vi "UHR-Fleezers Control (host) - 10.3.vi"() -> ()   [LabVIEW 2012]
uses:
  <vilib>/rvi/interface/nirviMethod/nirviMethod.xnode
  <vilib>/rvi/interface/nirviCloseFPGA/nirviCloseFPGA.xnode
  <vilib>/express/express analysis/Spectral/XNode/ExpressSpectralMeasurementsBlockNode.xnode
  <vilib>/rvi/interface/nirviReadWriteControl/nirviReadWriteControl.xnode
  <vilib>/Analysis/NI_AALBase.lvlib
  <vilib>/express/express analysis/Spectral/Block/exnSpectralBlock spectral measurements PSD poly.vi
  <vilib>/rvi/interface/nirviOpenFPGA/nirviOpenFPGA.xnode
  <vilib>/vision/Avi1.llb/AviRefnum.ctl
  <vilib>/Platform/TimedLoop/XDataNode/XDataNode.xnode
  <vilib>/Platform/TimedLoop/XDataNode/nitl_modes.ctl
  <vilib>/Platform/TimedLoop/XDataNode/XDNodeRunTimeDep.lvlib
  <vilib>/Platform/TimedLoop/XDataNode/wakeup.ctl
  <vilib>/Platform/TimedLoop/XDataNode/timing_clust.ctl
  <vilib>/Utility/miscctls.llb/LVPoint32TypeDef.ctl
  <vilib>/userdefined/High Color/nirio_resource_hc.ctl
  openfpgaref.8.6.ctl
  <vilib>/Utility/miscctls.llb/LVMinMaxIncTypeDef.ctl
  <vilib>/vision/NI_Vision_Development_Module.lvlib
  <vilib>/Instr/_visa.llb/VISA Configure Serial Port (Instr).vi
  <vilib>/Waveform/WDTOps.llb/WDT Append Waveforms DBL.vi
  <vilib>/express/express analysis/Spectral/Block/exnSpectralBlock spectral measurements PSD WFM.vi
  UHR-Fleezers Control (fpga) - 10.3.vi
  <vilib>/Analysis/baseanly.llb/Mean (DBL).vi
  FPGA Bitfiles/UHR-FleezersInst_FPGATarget_UHR-FleezersCont_AF27E573.lvbitx
  <vilib>/FPGAPlugInAG/PCIe-7852R/niLvFpga_Open_PCIe-7852R.vi
  <vilib>/FPGAPlugInAG/PCIe-7852R/niLvFpga_Reset_PCIe-7852R.vi
  NiFpgaLv.dll
  <vilib>/Utility/error.llb/Error Cluster From Error Code.vi
  <vilib>/rvi/errors/niLvFpgaAdjustHostInterfaceError.vi
  <vilib>/FPGAPlugInAG/PCIe-7852R/niLvFpga_ConfigureFifo_PCIe-7852R.vi
  <vilib>/rvi/errors/niLvFpgaMergeErrorWithErrorCode.vi
  <vilib>/FPGAPlugInAG/PCIe-7852R/niLvFpga_Run_PCIe-7852R.vi
  <vilib>/FPGAPlugInAG/PCIe-7852R/niLvFpga_ReadFifo_PCIe-7852R.vi
  <vilib>/FPGAPlugInAG/PCIe-7852R/niLvFpga_Close_PCIe-7852R.vi
panel:
  in  "Index":dbl=67.0 caption="Save File Index" min=1.0 step=1.0
  in  "Sample Channel Flow":bool=TRUE
  in  "Pump 3 contents":string="Left: ADig beads" caption="contents"
  in  "Pump 1 contents":string="Right: DNA beads" caption="contents"
  in  "Scripts":T1(tab)=enum."Trap Triggered Fl."
  in  "Trap Trig Fl.":bool=TRUE
  in  "Starting \nTrap Delta (MHz)":dbl=15.0
  in  "Take Force FB Data\nUpper Channel":bool
  in  "Cap 1 Samp Flow ON":bool
  in  "Cap 2 Samp Flow ON":bool=TRUE
  in  "Got DNA bead":bool
  in  "Got ADig bead":bool
  in  "Cap 2 Flow ON":bool=TRUE
  in  "Cap 1 Flow ON":bool=TRUE
  in  "Cap 2 T ON":bool=TRUE
  in  "Move Cap. 2 (ADig Left)":bool
  in  "Move Cap. 1 (DNA Right)":bool
  in  "Cal/Data Acq. Spot":bool
  in  "Dump Beads":bool
  in  "Lower Ch. Cap.":bool
  in  "Cap 1 T ON":bool=TRUE
  in  "Offset 2 Set":dbl=2.0
  in  "Offset 1 Set":dbl
  in  "Cal @ (MHz)":dbl=15.0
  in  "W/ Offset 1":bool=TRUE
  in  "Offset 1 Start (MHz)":dbl=13.0
  in  "W/ Offset 2":bool
  in  "Offset 2 Start (MHz)":dbl=16.0
  in  "Move to Delta 2 (MHz)":dbl=13.0
  in  "Attempt Limit":dbl=15.0 caption="Limit"
  out "Attempts":dbl=10.0
  in  "Wait Before Save (s)":u32=1
  in  "Fish for Tether":bool
  in  "Closest Delta (MHz)":dbl=9.25 step=0.25
  in  "Stop F (pN)":dbl=3.0
  in  "Then...":string(combo)="5"
  in  "Move to Delta 1 (MHz)":dbl=13.0
  in  "Tether Alarm?":bool=TRUE
  out "Tether":bool
  in  "TA Cancel Save?":bool
  in  "TA Green Off?":bool
  in  "Raster Set Upon Tether":u32=1
  in  "Save at end (5, 6)":bool
  out "Waiting":bool
  in  "Trap Triggering":bool
  in  "Wait to get offset (s)":u32=5
  in  "mean sampling rate (ms)":u32=100
  in  "Threshold (nm)":dbl=10.0
  in  "Fl. ON time (s)":i32=10
  out "T1 x pos data":dbl[](array[numeric])
  out "max value":dbl
  out "min value":dbl
  out "Mean T1 Position (nm) 2":dbl caption="Mean T1 for Comparison (nm)" format="%0.2f"
  in  "Dip Trap Delta 1 (MHz)":dbl=15.0
  in  "Move Trap Before?":bool
  in  "Save Data After?":bool
  in  "Green ON After?":bool
  in  "Dip Trap Delta 2 (MHz)":dbl=15.0
  in  "Move Trap After?":bool
  in  "Duration (s)":dbl=1.0
  in  "Dip for Protein":bool
  in  "Y change (mm)":dbl=3.0
  in  "Profile":bool
  out "Current Position":cluster{dbl, dbl, dbl}
  in  "APD to Watch":bool
  out "Duration (s)":dbl
  in  "Action":string(combo)="Yank"
  in  "Fl. Triggered...":bool
  in  "Fl. Delta Thresh. (kHz)":dbl=0.6
  out "Waiting":bool
  out "Fl. High":bool
  in  "N pts to average":u16=6
  in  "Yank Delay (s)":dbl=3.5
  in  "Yank to Delta Array (MHz)":dbl[](array[numeric])=[16.3, 15.85, 14.85]
  in  "N Array El":u8=3 min=1 step=1
  in  "Random Choice":bool=TRUE
  in  "Force Yank":bool
  in  "Force Reset":bool
  in  "N Steps":dbl=20.0
  in  "Step Size (nm)":dbl=0.34
  in  "Save ave factor":dbl=1.0
  in  "Take Stepping Data":bool
  out "Sigma/Mean 2":dbl=0.9156115002105881 caption="Sigma/Mean" format="%#_2g"
  out "Rate sigma (Hz) 2":dbl=91.25594618765528 caption="Sigma (Hz)" format="%0.2f"
  out "APD 2 Rate (Hz)":dbl=99.66666666666667 format="%#_3p"
  out "Primary Video Display":T2(plugin-control)
  out "Waveform Graph":dbl[](graph) caption="APD Line Scan"
  in  "Inject Pump 3":bool
  in  "Inject Pump 1":bool
  out "Messages":string="4:51 PM\tLost tether (7 s).\r4:51 PM\tFormed tether in 10 attempt(s).\r4:50 PM\tLost tether (5 s).\r4:49 PM\tFormed tether in 5 attempt(s).\r4:47 PM\tLost tether (36 s).\r4:47 PM\tFormed tether in 1 attempt(s).\r4:42 PM\tTether fishing timeout.\r4:37 PM\tTether fishing timeout.\r4:36 PM\tTether fishing timeout.\r4:32 PM\tTether fishing timeout.\r4:29 PM\tLost tether (4 s).\r4:28 PM\tFormed tether in 6 attempt(s).\r4:28 PM\tLost tether (5 s).\r4:28 PM\tFormed tether in 6 attempt(s).\r4:23 PM\tFormed tether in 1 attempt(s).\r4:23 PM\tLost tether (6 s).\r4:23 PM\tFormed tether in 1 attempt(s).\r4:14 PM\tFormed tether in 2 attempt(s).\r4:10 PM\tLost tether (548 s).\r4:01 PM\tFormed tether in 2 attempt(s).\r3:58 PM\tLost tether (6 s).\r3:58 PM\tFormed tether in 3 attempt(s).\r3:57 PM\tTether fishing timeout.\r3:42 PM\tLost tether (6 s).\r3:42 PM\tFormed tether in 6 attempt(s).\r3:39 PM\tLost tether (50 s).\r3:38 PM\tFormed tether in 10 attempt(s).\r3:37 PM\tLost tether (5 s).\r3:37 PM\tFormed tether in 6 attempt(s).\r3:34 PM\tTether fishing timeout.\r3:31 PM\tLost tether (45 s).\r3:30 PM\tFormed tether in 1 attempt(s).\r3:30 PM\tLost tether (4 s).\r3:30 PM\tFormed tether in 4 attempt(s).\r3:22 PM\tFormed tether in 6 attempt(s).\r3:18 PM\tLost tether (51 s).\r3:17 PM\tFormed tether in 3 attempt(s).\r3:17 PM\tLost tether (6 s).\r3:16 PM\tFormed tether in 1 attempt(s).\r3:06 PM\tFormed tether in 2 attempt(s).\r3:05 PM\tLost tether (3 s).\r3:05 PM\tFormed tether in 1 attempt(s).\r2:11 PM\tUHR-Fleezers ready.\r"
  in  "APD Ave N":dbl=10.0
  out "Int. Time (s)":dbl=3.0
  in  "Stop All":bool=TRUE
  out "Sigma/Mean":dbl=0.7461899027919234 format="%#_2g"
  out "Rate sigma (Hz)":dbl=246.24266792133471 caption="Sigma (Hz)" format="%0.2f"
  in  "Tab Control 6":T3(tab)
  in  "APD 2 Offset":dbl
  in  "APD 1 Offset":dbl
  out "RMS (Ang)":dbl=824.5898142565536 format="%_2g"
  in  "Bead Sep. Int. Time (s)":dbl=5.0 caption="Int. Time (s)"
  in  "Below (kHz)":dbl=0.5
  in  "Above (kHz)":dbl=2.0
  in  "Adjust Scale\nto Mean":bool
  in  "Rescale on Mean":bool
  in  "Offset (nm)":dbl
  out "Mean":dbl=107.85631162700733 caption="Mean (pN)" format="%#_3g"
  out "Force":waveform(dbl)[](graph)=[{"t0"=timestamp(9589.800000000116 s since 1904-01-01), "dt"=0.15, "Y"=[-107.59208218650274, -108.24679101361127], "attributes"=variant("NI_ChannelName"=variant(string "T1 X"))}, {"t0"=timestamp(9589.800000000116 s since 1904-01-01), "dt"=0.15, "Y"=[107.4628305657673, 108.12354274214799], "attributes"=variant("NI_ChannelName"=variant(string "T2 X"))}]
  out "APD Chart":waveform(dbl)[](graph)=[{"t0"=timestamp(9589.800000000116 s since 1904-01-01), "dt"=0.15, "Y"=[253.33333333333334, 266.6666666666667], "attributes"=variant("NI_ChannelName"=variant(string "APD 1"))}, {"t0"=timestamp(9589.800000000116 s since 1904-01-01), "dt"=0.15, "Y"=[93.33333333333334, 106.66666666666667], "attributes"=variant("NI_ChannelName"=variant(string "APD 2"))}]
  in  "Calibration":u16(ring)=2 items=["None", "Position", "Force"]
  out "T1 X":dbl=-107.919436600057 caption="T1 X (pN)" format="%0.2f"
  out "T2 X":dbl=-107.79318665395765 caption="T2 X (pN)" format="%0.2f"
  out "Bead Separation":waveform(dbl)(graph)={"t0"=timestamp(9589.800000000116 s since 1904-01-01), "dt"=0.15, "Y"=[-66.14062626515556, -66.57399525696837], "attributes"=variant("NI_ChannelName"=variant(string "T1 X"))}
  in  "Amplitude (nm)":dbl=3.0
  out "Bead Mean (nm)":dbl=-64.52066524805926 caption="Mean (nm)" format="%0.2f"
  out "Difference":dbl=0.12624994609934959 caption="Difference (pN)" format="%.2g"
  in  "Take Detection Laser\nImage":bool
  out "APD 2":T2(plugin-control) caption="APD 2 (Cy5)"
  in  "Flip Green Filter":bool
  in  "Set X Only":bool
  in  "Set Y Only":bool
  out "APD 1":T2(plugin-control) caption="APD 1 (Cy3)"
  out "Detection Laser Y":T2(plugin-control)
  out "Pointer Y (V)":dbl=4.98101801028038 format="%_3g"
  out "Pointer X (V)":dbl=3.881593676564837 format="%_3g"
  in  "Set Confocal Spot (X-Y)":bool
  out "Detection Laser X":T2(plugin-control)
  out "Saved APD":dbl[][](graph)=[[640.0, 640.0, 513.3333333333334, 520.0, 506.6666666666667, 520.0, 626.6666666666667, 680.0, 540.0, 606.6666666666667, 640.0, 513.3333333333334, 553.3333333333334, 693.3333333333334, 613.3333333333334, 513.3333333333334, 660.0, 513.3333333333334, 620.0, 506.6666666666667, 613.3333333333334, 546.6666666666667, 566.6666666666667, 753.3333333333334, 540.0, 546.6666666666667, 593.3333333333334, 646.6666666666667, 533.3333333333334, 613.3333333333334, 633.3333333333334, 653.3333333333334, 580.0, 646.6666666666667, 686.6666666666667, 660.0, 646.6666666666667, 560.0, 520.0, 600.0, 573.3333333333334, 633.3333333333334, 620.0, 600.0, 553.3333333333334, 533.3333333333334, 540.0, 546.6666666666667, 586.6666666666667, 573.3333333333334, 626.6666666666667, 506.6666666666667, 606.6666666666667, 613.3333333333334, 600.0, 526.6666666666667, 606.6666666666667, 606.6666666666667, 560.0, 613.3333333333334, 546.6666666666667, 486.6666666666667, 606.6666666666667, 573.3333333333334, 660.0, 693.3333333333334, 620.0, 586.6666666666667, 553.3333333333334, 506.6666666666667, 486.6666666666667, 593.3333333333334, 520.0, 560.0, 653.3333333333334, 633.3333333333334, 546.6666666666667, 653.3333333333334, 586.6666666666667, 566.6666666666667, 620.0, 546.6666666666667, 593.3333333333334, 580.0, 673.3333333333334, 673.3333333333334, 566.6666666666667, 620.0, 506.6666666666667, 633.3333333333334, 613.3333333333334, 546.6666666666667, 606.6666666666667, 600.0, 680.0, 586.6666666666667, 573.3333333333334, 540.0, 573.3333333333334, 633.3333333333334, 546.6666666666667, 553.3333333333334, 533.3333333333334, 633.3333333333334, 633.3333333333334, 600.0, 646.6666666666667, 640.0, 540.0, 486.6666666666667, 586.6666666666667, 566.6666666666667, 626.6666666666667, 606.6666666666667, 640.0, 546.6666666666667, 566.6666666666667, 653.3333333333334, 626.6666666666667, 586.6666666666667, 613.3333333333334, 626.6666666666667, 560.0, 700.0, 546.6666666666667, 506.6666666666667, 566.6666666666667, 640.0, 573.3333333333334, 593.3333333333334, 493.33333333333337, 613.3333333333334, 626.6666666666667, 673.3333333333334, 580.0, 633.3333333333334, 633.3333333333334, 713.3333333333334, 400.0, 560.0, 520.0, 506.6666666666667, 720.0, 553.3333333333334, 553.3333333333334, 426.6666666666667, 600.0, 540.0, 520.0, 640.0, 453.33333333333337, 533.3333333333334, 460.0, 426.6666666666667, 546.6666666666667, 580.0, 460.0, 480.0, 586.6666666666667, 473.33333333333337, 580.0, 613.3333333333334, 546.6666666666667, 500.0, 546.6666666666667, 540.0, 586.6666666666667, 560.0, 406.6666666666667, 533.3333333333334, 520.0, 573.3333333333334, 540.0, 486.6666666666667, 633.3333333333334, 486.6666666666667, 586.6666666666667, 440.0, 446.6666666666667, 553.3333333333334, 520.0, 540.0, 620.0, 506.6666666666667, 580.0, 653.3333333333334, 540.0, 566.6666666666667, 586.6666666666667, 453.33333333333337, 653.3333333333334, 553.3333333333334, 460.0, 593.3333333333334, 420.0, 553.3333333333334, 526.6666666666667, 480.0, 520.0, 606.6666666666667, 493.33333333333337, 560.0, 513.3333333333334, 426.6666666666667, 440.0, 513.3333333333334, 500.0, 633.3333333333334, 513.3333333333334, 460.0, 526.6666666666667, 466.6666666666667, 540.0, 546.6666666666667, 540.0, 486.6666666666667, 500.0, 506.6666666666667, 553.3333333333334, 400.0, 493.33333333333337, 420.0, 413.33333333333337, 540.0, 513.3333333333334, 493.33333333333337, 420.0, 533.3333333333334, 466.6666666666667, 546.6666666666667, 493.33333333333337, 480.0, 366.6666666666667, 526.6666666666667, 520.0, 406.6666666666667, 526.6666666666667, 620.0, 520.0, 500.0, 460.0, 480.0, 520.0, 446.6666666666667, 680.0, 526.6666666666667, 613.3333333333334, 700.0, 566.6666666666667, 646.6666666666667, 573.3333333333334, 593.3333333333334, 626.6666666666667, 546.6666666666667, 526.6666666666667, 773.3333333333334, 626.6666666666667, 546.6666666666667, 633.3333333333334, 553.3333333333334, 613.3333333333334, 546.6666666666667, 540.0, 593.3333333333334, 620.0, 646.6666666666667, 706.6666666666667, 506.6666666666667, 573.3333333333334, 640.0, 513.3333333333334, 473.33333333333337, 606.6666666666667, 533.3333333333334, 466.6666666666667, 506.6666666666667, 500.0, 573.3333333333334, 446.6666666666667, 646.6666666666667, 533.3333333333334, 533.3333333333334, 560.0, 500.0, 586.6666666666667, 580.0, 460.0, 486.6666666666667, 580.0, 573.3333333333334, 506.6666666666667, 533.3333333333334, 586.6666666666667, 700.0, 486.6666666666667, 480.0, 560.0, 593.3333333333334, 573.3333333333334, 680.0, 626.6666666666667, 633.3333333333334, 660.0, 640.0, 600.0, 600.0, 586.6666666666667, 760.0, 686.6666666666667, 613.3333333333334, 686.6666666666667, 593.3333333333334, 553.3333333333334, 606.6666666666667, 573.3333333333334, 460.0, 546.6666666666667, 640.0, 553.3333333333334, 600.0, 580.0, 526.6666666666667, 620.0, 573.3333333333334, 626.6666666666667, 506.6666666666667, 573.3333333333334, 413.33333333333337, 373.33333333333337, 493.33333333333337, 546.6666666666667, 513.3333333333334, 466.6666666666667, 626.6666666666667, 526.6666666666667, 486.6666666666667, 480.0, 500.0, 593.3333333333334, 453.33333333333337, 500.0, 460.0, 593.3333333333334, 540.0, 500.0, 486.6666666666667, 500.0, 533.3333333333334, 460.0, 540.0, 500.0, 580.0, 480.0, 586.6666666666667, 560.0, 513.3333333333334, 566.6666666666667, 553.3333333333334, 540.0, 593.3333333333334, 533.3333333333334, 493.33333333333337, 553.3333333333334, 466.6666666666667, 500.0, 646.6666666666667, 513.3333333333334, 540.0, 446.6666666666667, 540.0, 426.6666666666667, 540.0, 613.3333333333334, 506.6666666666667, 493.33333333333337, 486.6666666666667, 606.6666666666667, 500.0, 486.6666666666667, 526.6666666666667, 560.0, 540.0, 433.33333333333337, 540.0, 520.0, 480.0, 540.0, 473.33333333333337, 466.6666666666667, 420.0, 413.33333333333337, 560.0, 546.6666666666667, 493.33333333333337, 406.6666666666667, 480.0, 480.0, 466.6666666666667, 426.6666666666667, 486.6666666666667, 520.0, 606.6666666666667, 480.0, 493.33333333333337, 626.6666666666667, 486.6666666666667, 486.6666666666667, 440.0, 660.0, 593.3333333333334, 533.3333333333334, 520.0, 580.0, 500.0, 573.3333333333334, 500.0, 573.3333333333334, 446.6666666666667, 586.6666666666667, 586.6666666666667, 546.6666666666667, 600.0, 620.0, 540.0], [73.33333333333334, 166.66666666666669, 86.66666666666667, 113.33333333333334, 140.0, 126.66666666666667, 93.33333333333334, 93.33333333333334, 113.33333333333334, 120.0, 120.0, 146.66666666666669, 66.66666666666667, 113.33333333333334, 120.0, 113.33333333333334, 120.0, 126.66666666666667, 140.0, 133.33333333333334, 120.0, 140.0, 86.66666666666667, 160.0, 126.66666666666667, 113.33333333333334, 93.33333333333334, 133.33333333333334, 100.0, 126.66666666666667, 133.33333333333334, 86.66666666666667, 126.66666666666667, 80.0, 140.0, 113.33333333333334, 120.0, 186.66666666666669, 113.33333333333334, 93.33333333333334, 53.333333333333336, 66.66666666666667, 133.33333333333334, 140.0, 126.66666666666667, 53.333333333333336, 126.66666666666667, 133.33333333333334, 73.33333333333334, 113.33333333333334, 100.0, 66.66666666666667, 113.33333333333334, 120.0, 140.0, 100.0, 80.0, 126.66666666666667, 126.66666666666667, 133.33333333333334, 73.33333333333334, 113.33333333333334, 93.33333333333334, 126.66666666666667, 140.0, 46.66666666666667, 153.33333333333334, 113.33333333333334, 66.66666666666667, 106.66666666666667, 146.66666666666669, 100.0, 120.0, 93.33333333333334, 140.0, 126.66666666666667, 93.33333333333334, 60.0, 46.66666666666667, 133.33333333333334, 93.33333333333334, 113.33333333333334, 80.0, 73.33333333333334, 113.33333333333334, 93.33333333333334, 113.33333333333334, 146.66666666666669, 120.0, 66.66666666666667, 120.0, 106.66666666666667, 80.0, 113.33333333333334, 113.33333333333334, 100.0, 73.33333333333334, 106.66666666666667, 126.66666666666667, 80.0, 140.0, 93.33333333333334, 120.0, 113.33333333333334, 80.0, 53.333333333333336, 113.33333333333334, 80.0, 93.33333333333334, 140.0, 146.66666666666669, 93.33333333333334, 180.0, 133.33333333333334, 60.0, 140.0, 100.0, 153.33333333333334, 100.0, 86.66666666666667, 93.33333333333334, 106.66666666666667, 126.66666666666667, 60.0, 113.33333333333334, 153.33333333333334, 120.0, 140.0, 106.66666666666667, 86.66666666666667, 146.66666666666669, 113.33333333333334, 133.33333333333334, 126.66666666666667, 100.0, 126.66666666666667, 186.66666666666669, 86.66666666666667, 146.66666666666669, 73.33333333333334, 160.0, 113.33333333333334, 113.33333333333334, 80.0, 106.66666666666667, 126.66666666666667, 113.33333333333334, 93.33333333333334, 126.66666666666667, 126.66666666666667, 113.33333333333334, 93.33333333333334, 60.0, 146.66666666666669, 100.0, 106.66666666666667, 66.66666666666667, 80.0, 106.66666666666667, 93.33333333333334, 73.33333333333334, 113.33333333333334, 100.0, 86.66666666666667, 133.33333333333334, 100.0, 86.66666666666667, 100.0, 53.333333333333336, 180.0, 120.0, 133.33333333333334, 106.66666666666667, 80.0, 133.33333333333334, 86.66666666666667, 73.33333333333334, 100.0, 100.0, 126.66666666666667, 93.33333333333334, 73.33333333333334, 66.66666666666667, 113.33333333333334, 73.33333333333334, 140.0, 120.0, 133.33333333333334, 100.0, 86.66666666666667, 53.333333333333336, 100.0, 80.0, 100.0, 86.66666666666667, 106.66666666666667, 120.0, 73.33333333333334, 120.0, 60.0, 100.0, 113.33333333333334, 93.33333333333334, 126.66666666666667, 80.0, 73.33333333333334, 73.33333333333334, 100.0, 86.66666666666667, 66.66666666666667, 133.33333333333334, 93.33333333333334, 73.33333333333334, 126.66666666666667, 73.33333333333334, 106.66666666666667, 86.66666666666667, 120.0, 133.33333333333334, 80.0, 146.66666666666669, 80.0, 120.0, 86.66666666666667, 80.0, 60.0, 100.0, 93.33333333333334, 73.33333333333334, 106.66666666666667, 126.66666666666667, 80.0, 133.33333333333334, 86.66666666666667, 106.66666666666667, 120.0, 60.0, 40.0, 66.66666666666667, 86.66666666666667, 93.33333333333334, 66.66666666666667, 86.66666666666667, 100.0, 86.66666666666667, 120.0, 146.66666666666669, 80.0, 80.0, 160.0, 133.33333333333334, 93.33333333333334, 80.0, 140.0, 40.0, 113.33333333333334, 113.33333333333334, 93.33333333333334, 100.0, 106.66666666666667, 93.33333333333334, 133.33333333333334, 120.0, 120.0, 86.66666666666667, 66.66666666666667, 113.33333333333334, 66.66666666666667, 106.66666666666667, 100.0, 146.66666666666669, 120.0, 126.66666666666667, 106.66666666666667, 80.0, 133.33333333333334, 166.66666666666669, 86.66666666666667, 100.0, 133.33333333333334, 120.0, 86.66666666666667, 113.33333333333334, 40.0, 100.0, 106.66666666666667, 93.33333333333334, 86.66666666666667, 126.66666666666667, 53.333333333333336, 106.66666666666667, 106.66666666666667, 93.33333333333334, 80.0, 80.0, 120.0, 86.66666666666667, 146.66666666666669, 53.333333333333336, 86.66666666666667, 160.0, 153.33333333333334, 93.33333333333334, 93.33333333333334, 86.66666666666667, 120.0, 113.33333333333334, 93.33333333333334, 73.33333333333334, 60.0, 153.33333333333334, 60.0, 100.0, 80.0, 113.33333333333334, 106.66666666666667, 86.66666666666667, 113.33333333333334, 100.0, 86.66666666666667, 73.33333333333334, 100.0, 73.33333333333334, 80.0, 106.66666666666667, 93.33333333333334, 106.66666666666667, 106.66666666666667, 86.66666666666667, 60.0, 73.33333333333334, 93.33333333333334, 120.0, 140.0, 160.0, 60.0, 120.0, 120.0, 73.33333333333334, 73.33333333333334, 146.66666666666669, 80.0, 66.66666666666667, 100.0, 73.33333333333334, 113.33333333333334, 100.0, 66.66666666666667, 66.66666666666667, 93.33333333333334, 73.33333333333334, 146.66666666666669, 120.0, 86.66666666666667, 60.0, 86.66666666666667, 113.33333333333334, 120.0, 120.0, 73.33333333333334, 153.33333333333334, 106.66666666666667, 100.0, 80.0, 86.66666666666667, 113.33333333333334, 73.33333333333334, 113.33333333333334, 140.0, 93.33333333333334, 93.33333333333334, 60.0, 126.66666666666667, 93.33333333333334, 106.66666666666667, 113.33333333333334, 46.66666666666667, 113.33333333333334, 86.66666666666667, 100.0, 126.66666666666667, 93.33333333333334, 66.66666666666667, 160.0, 146.66666666666669, 93.33333333333334, 93.33333333333334, 93.33333333333334, 73.33333333333334, 106.66666666666667, 86.66666666666667, 66.66666666666667, 80.0, 86.66666666666667, 100.0, 120.0, 80.0, 120.0, 120.0, 133.33333333333334, 86.66666666666667, 113.33333333333334, 160.0, 93.33333333333334, 86.66666666666667, 93.33333333333334, 80.0, 120.0, 73.33333333333334, 93.33333333333334, 73.33333333333334, 73.33333333333334, 66.66666666666667, 120.0, 93.33333333333334, 60.0, 100.0, 100.0, 73.33333333333334, 73.33333333333334, 106.66666666666667, 86.66666666666667, 66.66666666666667, 126.66666666666667]] caption="Most Recent Time Trace"
  out "Trap Delta Graph":dbl[](graph)=[-106.43043807216529, -106.5454367986324, -106.51686160160939, -106.58501313534859, -106.73405579848394, -106.59345831600089, -106.55808478718131, -106.54847798904014, -106.63246708958809, -106.64841693959238, -106.4822053501463, -106.57755688373177, -106.67016724634344, -106.45433878652537, -106.47815911583766, -106.42379428925383, -106.51151845331754, -106.68746141834603, -106.50723577160747, -106.41173347001666, -106.45298074469062, -106.68357946354386, -106.41957394891901, -106.42779113376133, -106.46017439309665, -106.3331576187891, -106.35502678934324, -106.32337366489861, -106.55680288846125, -106.29647485921345, -106.4777976983645, -106.297812998571, -106.39808607771205, -106.65261139520646, -106.51296579380772, -106.66918631936434, -106.17562143548844, -84.60994919536043, 1.3310857319345684, 1.0361871672274952, 0.6560712621147459, 0.5689432704114208, 0.5054763131013246, 0.026676923553220266, 0.4416019568801436, 0.2735431213660061, 0.23024753352250904, 0.37724536348759063, 0.2421264893459717, 0.26340021780432943, 0.29841957537993546, 0.17548186500256102, 0.14535336814513755, 0.07167026524356301, 0.22596132502466781, 0.2852071568323358, 0.3257436622559723, 0.12892633791448793, 0.17014124062038827, 0.13608261272222044, 0.2165257310266071, 0.02390519326463647, 0.24374284074938912, 0.14033144222620686, 0.20160694442302618, 0.24399108515159418, 0.37280924880476496, 0.39269031828135303, 0.0020045770407064456, 0.24243253128233844, 0.5509136378777598, -0.06739948998052048, 0.3753325270901159, 0.041556923442069515, 0.5156644188755136, 0.43429902173750445, 0.6734298753615677, 0.24078809415362, 0.2226386778369127, 0.0928074556229388, 0.23452704613553288, 0.29537252172755735, 0.24028041004987544, 0.5110751644361885, 0.3115531148109213, 0.3541005104538466, 0.19808764601755413, 0.29451725645941296, 0.37483027387224876, 0.14422108697133207, 0.10937006932469684, -0.10006183935749324, 0.5174008122551468, -0.15899440920889152, 0.067222901985028, 0.4893964012215861, 0.16100705380999392, 0.040244638366899954, 0.21823030270568278, 0.2724552172281144, 0.3286154371444875, 0.09671105698981519, 0.211070673931971, 0.27403940383827663, -0.18158626168544867, 0.359992544087572, 0.17521597973752523, -0.01712139810390334, 0.34828383230753013, 0.38821465356197205, -0.47577316993658636, -0.061209978340928006, -0.04336067966990298, 0.1973437946223825, 0.14125329725782476, 0.39799396471853143, 0.5095924157430234, 0.5369250733859182, 0.5141657617439718, 0.12314529776262206, 0.12340359436175818, 0.4247246292008219, 0.34987918195615864, 0.3691260807314214, 0.18948963934016738, 0.11514675643557093, 0.3145960367967432, 0.0847238153799148, 0.5498257841297541, 0.3435810561376562, 0.28951709031660544, 0.11486034175086168, 0.19981958245548992, 0.24902605730103988, 0.08386197607169354, 0.3076486879407194, 0.5316368497813708, 0.011172428028344061, 0.16515294490283083, 0.2589832302335102, 0.06118106222967257, 0.05179602677324213, 0.14605031191417106, -0.27028691855927245, 0.3046427258477053, -0.32654161566760187, 0.11547372002670883, 0.05841771855848377, -0.09021888308668857, 0.28492200832706416, 0.14848195262761732, 0.08004379230789829, 0.11340489372509398, -0.1207310131639201, 0.1541946406564236, 0.1269929332462834, -0.25254475570349794, 0.1559630190503728, -0.16465543631295051, 0.11133039420408519, 0.1402543807831096, 0.02125799385333696, -0.16462459978957333, -0.38923305887864584, -0.02381113492727646, 0.10391530706475595, 0.23820889685935479, -0.023728686724600878, -0.04764111901766144, -0.007608743009235641, -0.2831431266449582, -0.4601669034291135, 0.1270783916843988, 0.11151315228001513, 0.07486139973609482, -0.24727183052659096, 0.19791921503036844, 0.07911640381694093, -0.06594038816975148, 0.2904115238995478, 0.2572744514721885, -0.20695214319298796, -0.011134088990943897, -0.1329170956283653, -0.17359323758311615, 0.12181978652209512, -0.11042971273973787, 0.22899157117508717, 0.3140832953715535, -0.30689327909618325, 0.03860844834068772, 0.394228107655571, 0.05293892569083136, -0.25365611830805873, 0.24686577579815186, 0.049501080171641065, -0.14974810230810087, -0.02833685388093199, 0.18652778365699527, 0.29108264069094064, -0.0008448102460272833, 0.0018380106327957058, 0.12078335855310426, 0.25940308098841486, -0.04482483301124446, 0.07376288462566721, -0.20968097306502337, -0.21601485851555285, -0.255227346307366, -0.006578989879893332, 0.2693875220630272, -0.05322628288934911, 0.013224520397867853, 0.019089251473903474, 0.1785683517670636, 0.0005106496658305038, 0.03471794306860293, -0.03881457062500418, 0.1314922052228636, 0.19291503243930383, 0.016286528257771483, 0.04613488933487331, 0.023391462208254027, -0.0867936685376553, 0.1667056535330356, 0.13551569687601753, 0.03966388491544098, -0.001509757708971271, -0.04930535048489537, -0.02488348604948106, 0.17699798141823225, 0.09067749598174343, 0.2810609960550859, -0.17953434343886976, -0.08087810161787876, 0.15531385466958078, 0.07966370440497603, 0.21169243968790535, 0.27463644895840034, 0.11358419137524867, 0.44151340468279066, 0.013676594736444725, 0.13803367875581318, 0.16762306170228025, -9.305097846396249, -8.734185730622158, -7.795085141730819, -7.1169239424821455, -6.8078194604182505, -6.012872438821646, -5.297070121155155, -4.8008820282039935, -3.80266145736694, -3.2398214424229104, -2.6995113604562464, -2.250937951595689, -1.6142815413389022, -1.1477956359922619, -0.7851258896920497, -0.5489468717661414, 0.007892963192939528, 0.4297874535410666, 0.7232126615705075, 1.0881378793787722, 0.9469945823546175, 1.1315981032380298, 1.5088200228939004, 1.9696025136662745, 2.0125320503247393, 2.0616893854058578, 2.0607414539584012, 2.6901101639116844, 2.913370534266508, 2.9915343321096253, 3.1810584698757345, 3.2694738112071233, 3.815351721905264, 3.711465789182815, 3.3319100390246166, 3.4738940838355026, 2.9938700615022165, 2.8719830063163836, 2.814001855577777, 2.4799945954145404, 2.306309702543458, 2.287683746001849, 1.884452351748454, 1.4763570637661683, 1.500909948307402, 1.3757091991201318, 0.9511484877404002, 0.7750514269276616, 0.6476631465563494, -0.070662296735875, -0.029594788212394696, -0.32400306754623637, -0.8864635561709634, -1.4877222685335405, -2.0507065584317017, -2.6968184066815972, -3.0471461188113667, -3.5358182192812335, -4.376697785171516, -4.953120166587164, -5.848565647315136, -6.053854911411889, -7.052139284154087, -7.172726882840011, -8.190341884763662, -8.57176218146154, -9.031969641304759, -9.160140089904607, -19.406396896392515, -20.72767491143481, -22.52957503831575, -24.628780001646625, -27.645919716135815, -31.524820294981247, -36.00375847806328, -40.29138452034995, -45.564980244900866, -52.03629009220346, -59.389338493635734, -67.53729872875331, -76.40368321454261, -86.00318733592643, -95.67183386111026, -98.591914485014, -103.5540396015088, -111.71602156262952, -119.7345182693686, -128.10083921857876, -133.92328842606133, -140.30486296175064, -152.13782681810846, -127.59977417259103, 1.9097381969808318, 2.146077316363836, 2.5695963953157115, 2.6372377874037967, 2.712002965976897, 2.21214115543342, 2.0827027656517636, 1.7918328994151387, 1.8334538504789635, 1.4887474407240884, 1.3183156469574928, 1.1074607806068812, 0.5449613088181862, 0.6411310292885716, 0.2865682674798876, -0.20561912550425498, -0.4283737772873612, -0.8213909015749081, -1.301367318197441, -1.4043123386109424, -2.455428847708026, -2.865387975996997, -3.4460393734956574, -4.088620933822033, -4.852423708406629, -5.363424054600309, -5.985200931385475, -6.449778687075328, -7.359018465262011, -8.014348652381976, -8.602206142039282, -9.11747831938223, -16.10276890966618, -16.652936161554457, -17.45363480985382, -18.573158822709363, -19.611725824538883, -21.567924207070938, -24.090533940752877, -27.20500645507802, -31.47067005386945, -36.72043318743074, -43.01369354998713, -50.30269462184975, -58.470394481182154, -66.68608952303441, -76.32223565208024, -85.90747526669313, -96.45584392830432, -107.64327334791787, -118.00360649269274, -128.23147312175695, -139.24390140541698, -150.1280581951645, -160.43369113902202, -169.03532569855338, -179.6526957081072, -190.15619730232487, -196.645730104612, -206.28355442560365, -205.5533003536683, -193.35735124448496, -181.88474031887915, -171.53558469680792, -161.06805576546705, -150.48071337332783, -140.05252361639847, -129.1694172743015, -118.51016094139078, -38.66402558537719, 0.4687738479286786, -0.017898865181683668, -0.38393700946650355, -0.7924297107116016, -1.2685508455729173, -1.7227958503540475, -2.5497829209829965, -3.131493827362692, -3.3162470336029233, -4.01435852437743, -4.494030889765619, -5.58945592615083, -6.219129572016236, -6.884133384184377, -7.124206108411009, -8.080705713244733, -8.622535042543017, -9.408401169796818] caption="Most Recent Time Trace"
  out "Save APD Deriv":dbl[][](graph)=[[0.0, 0.0, 0.0, 4.444444444444457, 23.33333333333337, 44.44444444444446, 30.0, 7.777777777777828, -10.0, -20.0, -11.111111111111086, 10.000000000000114, 23.33333333333337, 31.111111111111086, -22.222222222222285, 17.77777777777783, 2.2222222222221717, 64.44444444444446, 17.777777777777715, 2.2222222222222854, -54.44444444444446, -38.888888888888914, -26.666666666666742, -23.33333333333337, -35.55555555555543, -22.22222222222217, 20.000000000000114, 24.444444444444343, 30.0, 0.0, -10.0, -28.888888888888914, 8.8888888888888, 53.33333333333337, 38.888888888888914, -36.66666666666663, -86.66666666666663, -28.888888888888914, 36.66666666666663, 70.0, 12.222222222222285, -12.222222222222172, 7.777777777777715, 31.111111111111086, 30.0, -33.33333333333326, -33.33333333333337, -6.666666666666629, 16.66666666666663, 13.333333333333371, -35.55555555555566, -18.888888888888914, -14.444444444444457, 44.44444444444446, 12.222222222222172, -5.555555555555543, -45.55555555555554, 4.444444444444571, 28.888888888888914, 34.44444444444446, 16.66666666666663, 12.222222222222172, -11.111111111111086, -25.555555555555543, -47.777777777777715, -12.222222222222285, 8.888888888888914, 32.22222222222217, 63.33333333333337, -8.888888888888914, -47.77777777777783, -100.0, -40.0, 10.0, 3.3333333333332575, 1.1111111111110858, -60.0, -46.66666666666663, -55.5555555555556, 15.555555555555543, 32.222222222222285, 57.77777777777777, 33.33333333333337, 14.444444444444457, -21.111111111111086, -24.444444444444457, -36.66666666666674, 11.111111111111086, -1.1111111111110858, 14.444444444444457, -25.555555555555543, 2.2222222222221717, 45.55555555555554, 63.33333333333337, 32.222222222222285, -11.111111111111086, -27.77777777777783, -24.444444444444457, -53.333333333333314, -32.22222222222217, -7.777777777777828, 14.4444444444444, -26.666666666666686, -26.66666666666663, -10.0, 25.5555555555556, 4.444444444444457, 7.777777777777828, 3.3333333333332575, -11.111111111111143, -38.888888888888914, -50.0, -18.888888888888857, 6.666666666666686, 25.5555555555556, 11.111111111111086, -5.555555555555543, -30.0, 4.444444444444457, 35.555555555555486, 52.22222222222223, -6.666666666666686, 3.3333333333333712, 63.33333333333326, 134.4444444444445, 96.66666666666674, 11.1111111111112, -15.555555555555543, -7.777777777777828, 17.777777777777715, -20.0, -27.77777777777783, -16.66666666666663, 15.555555555555543, 35.55555555555554, -24.444444444444457, -45.55555555555554, -98.8888888888888, -37.77777777777783, -33.33333333333337, 22.22222222222217, 5.555555555555657, 25.555555555555543, -10.0, 7.777777777777715, -25.555555555555543, 51.111111111111086, 4.444444444444457, 44.44444444444446, -17.777777777777715, 62.22222222222217, 67.77777777777771, 64.44444444444446, 30.0, 5.555555555555543, 27.777777777777715, -17.777777777777715, -62.22222222222217, -91.11111111111109, -61.111111111111086, -4.444444444444457, 12.222222222222172, 10.0, -22.22222222222217, -77.77777777777771, -86.66666666666669, -48.888888888888914, 30.0, 28.888888888888857, 3.3333333333333144, -30.000000000000057, 8.888888888888914, 6.666666666666686, 27.77777777777777, -20.0, 5.555555555555543, -1.1111111111110858, 33.33333333333337, 24.444444444444457, 30.0, 10.0, -13.333333333333371, -22.22222222222217, -10.0, 1.1111111111110858, -31.111111111111143, -24.444444444444457, -19.999999999999943, 33.333333333333314, 4.444444444444457, 25.5555555555556, -20.0, -4.444444444444571, -38.88888888888897, -31.111111111111086, -33.33333333333326, -14.4444444444444, 0.0, 0.0, -25.5555555555556, 14.444444444444457, 23.333333333333314, 77.77777777777777, 4.4444444444444, 46.666666666666686, 3.3333333333333712, 62.22222222222223, -14.444444444444457, -10.0, -20.0, 22.222222222222285, 51.111111111111086], [0.0, 0.0, 0.0, -8.888888888888886, -3.3333333333333286, -3.3333333333333286, 4.444444444444443, -1.1111111111111143, -4.444444444444457, 12.222222222222214, 16.666666666666657, 20.0, -1.1111111111111143, -11.1111111111111, -14.444444444444443, -12.222222222222214, -10.000000000000014, -2.2222222222222143, 15.555555555555557, 18.8888888888889, -7.777777777777786, -27.777777777777786, -32.22222222222223, 13.333333333333343, 4.444444444444457, 6.666666666666671, -21.111111111111114, 2.2222222222222143, 11.111111111111114, 20.0, 2.2222222222222285, -2.2222222222222285, -18.888888888888886, 3.3333333333333286, -6.666666666666657, 15.555555555555557, -6.666666666666671, 16.666666666666657, -8.8888888888889, -5.555555555555557, -31.111111111111114, -15.555555555555557, -5.555555555555543, 13.333333333333343, 18.8888888888889, 17.77777777777777, -2.2222222222222285, -3.333333333333343, -14.444444444444443, -1.1111111111111143, -2.2222222222222143, 14.444444444444443, 0.0, -10.0, -18.888888888888886, 11.111111111111114, 37.77777777777777, 32.222222222222214, 16.66666666666667, -24.444444444444443, -18.888888888888886, -32.22222222222223, 2.2222222222222285, 12.222222222222214, 24.444444444444443, 10.0, 1.4210854715202004e-14, 4.444444444444457, 7.7777777777777715, 1.1111111111111143, 3.3333333333333286, -12.222222222222214, -3.333333333333343, -22.22222222222223, 1.1111111111111, -5.555555555555557, 5.555555555555557, -12.222222222222214, -17.77777777777777, -18.888888888888886, -14.444444444444443, 2.2222222222222143, 8.888888888888886, 12.222222222222214, 13.333333333333329, 11.111111111111114, 11.111111111111114, 1.1111111111111143, -15.555555555555557, -8.888888888888886, -15.555555555555543, -1.1111111111111143, -10.0, 13.333333333333329, 13.333333333333329, 5.555555555555543, -21.111111111111114, -21.1111111111111, -4.444444444444443, 7.7777777777777715, 10.0, 7.777777777777786, 3.333333333333343, -6.666666666666671, -22.22222222222223, -5.555555555555557, 5.555555555555557, 21.111111111111114, 5.555555555555557, 3.3333333333333286, 6.666666666666671, 10.0, -4.444444444444443, -17.777777777777786, -22.22222222222223, 1.1111111111111143, 11.111111111111114, 23.33333333333333, -5.555555555555557, -21.111111111111114, -40.0, -7.7777777777777715, 12.222222222222229, 34.44444444444446, 28.888888888888886, 23.33333333333333, 11.1111111111111, -12.222222222222229, -18.888888888888886, -19.999999999999986, 6.666666666666671, 15.555555555555557, 8.888888888888886, -11.111111111111114, -22.22222222222223, 5.555555555555557, 22.22222222222223, 28.8888888888889, 7.7777777777777715, -1.1111111111111143, -3.333333333333343, -17.777777777777786, -22.22222222222223, -25.555555555555557, -4.444444444444443, 1.1111111111111143, 4.444444444444443, 3.333333333333343, 5.555555555555557, 1.1111111111111143, 16.66666666666667, 5.555555555555557, 22.22222222222223, -14.444444444444457, -15.555555555555557, -25.555555555555557, -12.222222222222214, 11.111111111111114, 7.7777777777777715, 13.333333333333329, -8.888888888888886, -14.444444444444443, -13.333333333333329, 1.1111111111111143, 7.777777777777786, 0.0, 1.1111111111111, 14.444444444444443, 32.222222222222214, 5.555555555555557, -5.555555555555557, -30.0, -4.444444444444443, -15.555555555555557, -4.444444444444443, -5.555555555555557, 11.111111111111114, 10.0, 6.666666666666671, -2.2222222222222285, 18.8888888888889, 7.7777777777777715, 11.111111111111114, -20.0, -2.2222222222222143, -11.111111111111114, 6.666666666666657, -4.444444444444443, 4.444444444444443, -6.666666666666657, -4.444444444444443, 5.555555555555557, 20.0, 14.444444444444443, -4.444444444444443, -27.777777777777786, -25.555555555555557, -11.111111111111114, 11.1111111111111, 28.888888888888886, 18.888888888888886, 20.000000000000014, -6.666666666666671, -3.3333333333333286, -26.66666666666667, -20.0, -22.222222222222214, -10.0, 4.444444444444443, 0.0, 8.888888888888886, -1.1111111111111]] caption="Most Recent Time Trace"
  out "Delta Fl. 1":dbl=51.111111111111086
  out "Delta Fl. 2":dbl=-1.1111111111111
  out "All Signals":waveform(dbl)[](graph)=[{"t0"=timestamp(9589.800000000116 s since 1904-01-01), "dt"=0.15, "Y"=[380.0, 400.0], "attributes"=variant("NI_ChannelName"=variant(string "APD 1"))}, {"t0"=timestamp(9589.800000000116 s since 1904-01-01), "dt"=0.15, "Y"=[140.0, 160.0], "attributes"=variant("NI_ChannelName"=variant(string "APD 2"))}, {"t0"=timestamp(9589.800000000116 s since 1904-01-01), "dt"=0.15, "Y"=[-0.5560947071135384, -0.5488051268739088], "attributes"=variant("NI_ChannelName"=variant(string "T1 Y"))}, {"t0"=timestamp(9589.800000000116 s since 1904-01-01), "dt"=0.15, "Y"=[-0.6964523017525798, -0.7003016638635213], "attributes"=variant("NI_ChannelName"=variant(string "T1 X"))}, {"t0"=timestamp(9589.800000000116 s since 1904-01-01), "dt"=0.15, "Y"=[0.009100131229590747, 0.009068117313150425], "attributes"=variant("NI_ChannelName"=variant(string "T1 Sum"))}, {"t0"=timestamp(9589.800000000116 s since 1904-01-01), "dt"=0.15, "Y"=[-0.557341526703397, -0.5498308802934172], "attributes"=variant("NI_ChannelName"=variant(string "T2 Y"))}, {"t0"=timestamp(9589.800000000116 s since 1904-01-01), "dt"=0.15, "Y"=[-0.6977537048097585, -0.7016458986193993], "attributes"=variant("NI_ChannelName"=variant(string "T2 X"))}, {"t0"=timestamp(9589.800000000116 s since 1904-01-01), "dt"=0.15, "Y"=[0.009161107211523788, 0.00913434247871334], "attributes"=variant("NI_ChannelName"=variant(string "T2 Sum"))}, {"t0"=timestamp(9589.800000000116 s since 1904-01-01), "dt"=0.15, "Y"=[0.05199389581726632, 0.0511983167557167], "attributes"=variant("NI_ChannelName"=variant(string "T1 FB X"))}, {"t0"=timestamp(9589.800000000116 s since 1904-01-01), "dt"=0.15, "Y"=[0.016877803888058106, 0.01688229010895108], "attributes"=variant("NI_ChannelName"=variant(string "T1 FB Sum"))}, {"t0"=timestamp(9589.800000000116 s since 1904-01-01), "dt"=0.15, "Y"=[0.048074905987419425, 0.04747925277569201], "attributes"=variant("NI_ChannelName"=variant(string "T2 FB X"))}, {"t0"=timestamp(9589.800000000116 s since 1904-01-01), "dt"=0.15, "Y"=[0.016815240943632313, 0.016807855464339123], "attributes"=variant("NI_ChannelName"=variant(string "T2 FB Sum"))}, {"t0"=timestamp(9589.800000000116 s since 1904-01-01), "dt"=0.15, "Y"=[-3.8792427407756658, -3.877178718972479], "attributes"=variant("NI_ChannelName"=variant(string "PSD Y"))}, {"t0"=timestamp(9589.800000000116 s since 1904-01-01), "dt"=0.15, "Y"=[-0.32047881103365267, -0.32100188649167594], "attributes"=variant("NI_ChannelName"=variant(string "PSD X"))}, {"t0"=timestamp(9589.800000000116 s since 1904-01-01), "dt"=0.15, "Y"=[-0.025290139469588305, -0.02530741294595172], "attributes"=variant("NI_ChannelName"=variant(string "PSD Y Sum"))}]
  in  "Signals to Plot":i32(listbox)
  out "Trap Disp. Freq. (Hz)":dbl=6.666666666666667 caption="Freq. (Hz)" format="%#_6p"
  out "Display Period (s)":dbl=0.15 caption="Period (s)" format="%#_6p"
  in  "Trap Disp. Downsample":dbl=10000.0 caption="Downsample" max=20000.0
  in  "APD Disp. Scale":dbl=0.1 caption="Scale (Divide,\nfor above plot only)"
  in  "APD Disp. Downsample":dbl=15.0 caption="Integrate" min=1.0 max=30.0 step=1.0
  out "APD Display Freq. (Hz)":dbl=6.666666666666667 caption="Freq. (Hz)"
  out "APD Display Period (s)":dbl=0.15 caption="Period (s)"
  out "FFT 1":cluster{"f0":dbl, "df":dbl, "magnitude":dbl[]}[](graph)=[{"f0"=0.0, "df"=3.3333333333333335, "magnitude"=array[10000 elements]}, {"f0"=0.0, "df"=3.3333333333333335, "magnitude"=array[10000 elements]}]
  out "FFT 2":cluster{"f0":dbl, "df":dbl, "magnitude":dbl[]}[](graph)
  in  "FFT 1 Choice 1":u16(ring) items=["T1 Y", "T1 X", "T1 Sum", "T2 Y", "T2 X", "T2 Sum", "T1 FB X", "T1 FB Sum", "T2 FB X", "T2 FB Sum", "PSD Y", "PSD X", "PSD Y Sum", "none"]
  in  "FFT 2 Choice 1":u16(ring)=13 items=["T1 Y", "T1 X", "T1 Sum", "T2 Y", "T2 X", "T2 Sum", "T1 FB X", "T1 FB Sum", "T2 FB X", "T2 FB Sum", "PSD Y", "PSD X", "PSD Y Sum", "none"]
  in  "FFT 1 Choice 2":u16(ring)=1 items=["T1 Y", "T1 X", "T1 Sum", "T2 Y", "T2 X", "T2 Sum", "T1 FB X", "T1 FB Sum", "T2 FB X", "T2 FB Sum", "PSD Y", "PSD X", "PSD Y Sum", "none"]
  in  "FFT 2 Choice 2":u16(ring)=13 items=["T1 Y", "T1 X", "T1 Sum", "T2 Y", "T2 X", "T2 Sum", "T1 FB X", "T1 FB Sum", "T2 FB X", "T2 FB Sum", "PSD Y", "PSD X", "PSD Y Sum", "none"]
  in  "Compute FFT":bool
  in  "Reset FFT":bool
  in  "# Spectra to Ave.":dbl=25.0
  out "Ave. Time (s)":dbl=7.5
  out "1 Channel":waveform(dbl)(graph)={"t0"=timestamp(0 s since 1904-01-01), "dt"=1.4999999999999999e-05, "Y"=array[20000 elements], "attributes"=variant("NI_ChannelName"=variant(string "T1 Y"))}
  out "Slow mean":dbl=0.04741485510254009 format="%0.2f"
  in  "Slow mean N ave.":dbl=1.0 min=1.0 step=1.0
  out "Mean Intensity":dbl=0.04741485510254009
  out "Sigma":dbl=0.006116447585273888
  out "Sigma/Mean":dbl=0.12899855060289364
  in  "Subtract mean":bool
  in  "High Res. Display":u16(ring) items=["T1 Y", "T1 X", "T1 Sum", "T2 Y", "T2 X", "T2 Sum", "T1 FB X", "T1 FB Sum", "T2 FB X", "T2 FB Sum", "PSD Y", "PSD X", "PSD Y Sum"]
  out "APD 1 Rate (Hz)":dbl=330.0 format="%#_3p"
  in  "Tab Control":T4(tab)=enum."Trap Control (RF)"
  out "Stage Moving":bool
  in  "Read Cal":bool
  in  "Confocal Linescan":bool
  in  "Speed (nm/s)":dbl=100.0
  in  "Furthest Withdraw (MHz)":dbl=15.0
  in  "Confocal Image":bool
  in  "Round T1 X":bool caption="Round"
  in  "T1 offset_x (mV)":dbl=-63.86439785165793 format="%#_2g"
  in  "T1 kappa_x (pN/nm)":dbl=0.25444062839906995 min=0.0 step=0.001 format="%#_2g"
  out "Time (s)":dbl=8.7
  out "Total Time (s)":dbl=60.0
  in  "Start Saving":bool
  in  "Cal sets to save":u32=25 min=1 step=1
  in  "Comment (data description)":string="testing confocal setup"
  out "Calibrating Trap...":bool
  in  "Trap 2 (ON/OFF)":bool
  in  "Trap 1 (ON/OFF)":bool
  in  "Save Calibration":bool
  in  "N sets to save":u32=200 caption="N Sets"
  in  "Save N Sets":bool
  out "Save file name":path=path "E:/Data/101209/101209_067.dat"
  in  "Save ave N":dbl=500.0 caption="Averaging Factor"
  out "Saving...":bool
  in  "Stop Saving":bool
  out "Progress":u16(slide) scale=0.0..100.0
  out "Manipulating Trap":bool
  out "Buffer Status":dbl(slide) scale=0.0..1.0
  out "Overflow (data lost)":bool
  in  "Reset":bool
  out "Data Rate (Hz)":dbl=66666.66666666667 caption="Trap Data Rate (Hz)" format="%#_3p"
  out "Data Period (s)":dbl=1.4999999999999999e-05 caption="Trap Data Period (s)" format="%#_6p"
  out "Save Data Rate (Hz)":dbl=133.33333333333334 caption="Rate (Hz)" format="%#_6p"
  out "Save Data Period (s)":dbl=0.0075 caption="Period (s)" format="%#_6p"
  in  "T1 alpha_x (nm/V)":dbl=668.456221254379 step=10.0 format="%#_3g"
  in  "T2 alpha_x (nm/V)":dbl=772.4433031277968 step=10.0 format="%#_3g"
  in  "T2 kappa_x (pN/nm)":dbl=0.21976131273941338 min=0.0 step=0.001 format="%#_2g"
  in  "T2 offset_x (mV)":dbl=-64.70019248344109 format="%#_2g"
  in  "BD 1 Frequency 1 (MHz)":dbl=72.0 caption="T1 X (MHz)" min=60.0 max=90.0 step=1.0 format="%#_6p"
  in  "BD 1 Frequency 2 (MHz)":dbl=85.0 caption="T2 X (MHz)" min=60.0 max=90.0 step=1.0 format="%#_6p"
  in  "Green Laser ON/Interlacing":bool
  in  "Round T2 X":bool caption="Round"
  in  "AO1":dbl(slide)=6.126072485819795 caption="Confocal Y (V)" min=0.0 max=10.0 step=0.01 scale=0.0..10.0 scale format="%_1f"
  in  "AO2":dbl(slide)=2.5314548173467215 caption="Confocal X (V)" min=0.0 max=10.0 step=0.01 scale=0.0..10.0 scale format="%_1f"
  in  "Trap Raster Scan":bool
  out "Raster Scanning...":bool
  in  "Trap Delta (MHz)":dbl=15.0
  in  "Setpoints (V)":cluster{"Set 1":dbl, "Set 2":dbl}={"Set 1"=9.0, "Set 2"=9.0}
  in  "Green FB Setpoint (mV)":dbl=150.0
  in  "Position Label 5":string="upper flow spot (UvrD)" caption="5"
  in  "Move to Position":bool
  in  "Position":dbl=1.0 min=1.0 max=10.0 step=1.0
  in  "Set Position":bool
  in  "Saved Stage Positions":dbl[][](array[numeric])=[[1.0, 0.0, 0.0, 0.0], [2.0, 0.38896, -1.95878, -0.01812], [3.0, 1.25, -0.5, 0.0], [4.0, 0.03696, -1.95878, -0.01812], [5.0, 1.25, -2.0, 0.0], [6.0, 0.0, 0.0, 0.0], [7.0, 0.0, 0.0, 0.0], [8.0, 0.0, 0.0, 0.0], [9.0, 0.0, 0.0, 0.0], [10.0, 0.0, 0.0, 0.0]]
  in  "Move to Position 5":bool
  in  "z nudge increment (um)":dbl=0.5
  in  "+z":bool
  in  "Position 1 Label":string="Right capillary (DNA beads)" caption="1"
  in  "Set Position 1":bool
  in  "Set Position 2":bool
  in  "Set Position 3":bool
  in  "Set Position 4":bool
  in  "Move to Position 3":bool
  in  "Move to Position 4":bool
  in  "Move to Position 2":bool
  in  "Move to Position 1":bool
  in  "Position 2 Label":string="Left capillary (ADig beads)" caption="2"
  in  "Position 3 Label":string="lower flow spot (ATP)" caption="3"
  in  "Position 4 Label":string="Dump beads" caption="4"
  in  "-z":bool
  in  "Set Position 5":bool
  out "Stage Control Serial Error":errorcluster={"status"=FALSE, "code"=1073676293, "source"="VISA Read in Set Stage Position.vi->UHR-Fleezers Control (host) - 10.2.vi"}
  out "Pump 3 cont disp":string="Left: ADig beads"
  out "Pump 1 cont disp":string="Right: DNA beads "
  in  "Ch 1 Inject Rate (ul/h)":dbl=100.0
  in  "Pump write delay (ms)":dbl=300.0
  in  "All Pump Parameters":T5={"Pump 1"={"Diameter (mm)"=4.61, "Units"=4.0, "Volume"=100.0, "Rate"=100.0}, "Pump 2"={"Diameter (mm)"=4.61, "Units"=3.0, "Volume"=0.0, "Rate"=0.0}, "Pump 3"={"Diameter (mm)"=4.61, "Units"=4.0, "Volume"=100.0, "Rate"=200.0}}
  in  "Ch 2 Inject Volume (uL)":dbl=100.0
  in  "Pump pause delay (ms)":u32
  in  "Ch 3 Inject Volume (uL)":dbl=100.0
  in  "Ch 3 Inject Rate (ul/h)":dbl=200.0
  in  "Flush Center Ch Volume (uL)":dbl=15.0
  in  "Flush Center Ch Rate (ul/m)":dbl=100.0
  in  "Inject Pump 2":bool caption="Inject Pump 2\n(Flush Center)"
  in  "Total Volume\nFlushed (uL)":dbl
  in  "Tab Control 2":T6(tab)=enum."Feedback on Trap Position"
  out "Total Counts (ticks)":u32=600
  in  "Trap ON/OFF X or Y Amp?":bool=TRUE
  in  "Oscillate Set 1":bool
  in  "Trap 1 ON":bool
  in  "Number Interlace Sets":u8=3 min=1 max=3
  in  "DIO count 3 (ticks)":u32=200
  in  "DIO count 2 (ticks)":u32=200
  in  "DIO count 1 (ticks)":u32=200
  in  "BD 2 Amplitude 3 (%)":dbl min=0.0 max=50.0 step=1.0
  in  "BD 2 Amplitude 2 (%)":dbl min=0.0 max=50.0 step=1.0
  in  "BD 2 Amplitude 1 (%)":dbl min=0.0 max=50.0 step=1.0
  in  "BD 1 Amplitude 3 (%)":dbl min=0.0 max=50.0 step=1.0
  in  "BD 1 Amplitude 2 (%)":dbl=35.0 min=0.0 max=50.0 step=1.0
  in  "BD 1 Amplitude 1 (%)":dbl=10.0 min=0.0 max=50.0 step=1.0
  in  "BD 2 Frequency 3 (MHz)":dbl=26.0 min=0.0 max=40.0 step=1.0 format="%#_6p"
  in  "BD 1 Frequency 3 (MHz)":dbl=70.0 min=60.0 max=90.0 step=1.0 format="%#_6p"
  in  "BD 2 Frequency 2 (MHz)":dbl=26.0 min=0.0 max=40.0 step=1.0 format="%#_6p"
  in  "BD 2 Frequency 1 (MHz)":dbl=26.0 min=0.0 max=40.0 step=1.0 format="%#_6p"
  in  "Not-Interlacing Set":enum32{"Set 1", "Set 2", "Set 3"}(radio)
  in  "Interlace":bool=TRUE
  in  "Trap 2 ON":bool
  in  "Trap 3 ON":bool
  in  "Scan axis 2":bool=TRUE
  in  "Osc. freq. (Hz)":dbl=0.25
  in  "Osc. amp. (MHz)":dbl=2.0
  out "Coords":T7
  in  "Manipulation Scaling":cluster{"Horizontal":dbl, "Vertical":dbl}={"Horizontal"=0.075, "Vertical"=0.01}
  in  "Freq or Amp switch first":bool=TRUE
  in  "Swap F1 and F2":bool
  in  "Freq switch delay":u16
  in  "Amp switch delay":u16=5
  in  "MCL Step Increment (V_int)":dbl=3.0
  out "Time to Finish All (min)":dbl=0.13986 format="%#_2p"
  in  "Scan Speed (nm/s)":dbl=100.0
  in  "Scan Range (nm)":dbl=420.0
  in  "Step Size (nm)":dbl=1.0
  in  "MCL/AOM Scale Tweak":dbl=1.0
  in  "MCL Step Position Ratio":dbl=0.5
  in  "Move MCL Also?":bool=TRUE
  out "Final sep (nm)":dbl=1194.000000000001
  out "Initial sep (nm)":dbl=774.0
  out "Save index":dbl=67.0
  out "Final delta (MHz)":dbl=16.41463414634147
  out "Initial delta (MHz)":dbl=13.0
  out "Final freq. (MHz)":dbl=68.58536585365853
  out "Initial freq. (MHz)":dbl=72.0
  in  "Saved AOD Raster Scan Parameter Sets":T8(array[cluster])=[{"Scan Range AOD (nm) 2"=500.0, "Step Size AOD (nm) 2"=1.0, "Scan Speed AOD (nm/s) 2"=100.0, "Number of scans (AOD) 2"=1, "Label"="offset curve"}, {"Scan Range AOD (nm) 2"=420.0, "Step Size AOD (nm) 2"=1.0, "Scan Speed AOD (nm/s) 2"=100.0, "Number of scans (AOD) 2"=1, "Label"="hp raster check"}, {"Scan Range AOD (nm) 2"=6.8, "Step Size AOD (nm) 2"=0.34, "Scan Speed AOD (nm/s) 2"=0.34, "Number of scans (AOD) 2"=1, "Label"="3.4 kbp - 1 bp steps"}]
  in  "Load parameters":bool
  out "Scan Range (MHz)":dbl=-3.4146341463414633
  in  "Restart DMA? (AOD)":bool=TRUE caption="Restart DMA?"
  out "Incr. int (AOD)":i64=-7759651845
  out "Time/Scan (s) (AOD)":dbl=4.1958 format="%#_2p"
  out "Data points/scans":dbl=559440.0
  out "Data points/scan (f/b)":dbl=559440.0
  in  "Save scans":bool=TRUE
  out "AOD Scan I":u64=2 caption="Scan I"
  in  "Continuous AOD Scanning":bool caption="Continuous Scanning"
  in  "Abort AOD Scan":bool caption="Abort Scan"
  in  "Scan BD":bool=TRUE
  out "Cycles/step (AOD)":u64=666 format="%.3p"
  in  "Number of F/B Scans (AOD)":u16=1 min=1
  out "Scan steps (AOD)":u64=420
  out "Scan Increment (MHz)":dbl=-0.008149484836137144
  out "AOD Scanning":bool caption="Scanning"
  in  "Start AOD Scan":bool caption="Start Scan"
  out "N sets should be saved":dbl=27.972
  out "Progress 2":u16(slide) caption="Progress" scale=0.0..100.0
  in  "Abort save 2":bool caption="Abort save"
  in  "Trap 1 Bead Size (nm)":dbl=860.0
  in  "Trap 2 Bead Size (nm)":dbl=790.0
  out "MCL Count":dbl=782931.6080202643
  in  "All FB On/Off":bool=TRUE
  in  "AI2 to Setpoint":cluster{"Set 1":bool, "Set 2":bool}
  out "AI2 (V)":cluster{"Set 1":dbl, "Set 2":dbl}={"Set 1"=0.017090365306558428, "Set 2"=0.016785180211798457}
  in  "Reset Feedback":cluster{"Set 1":bool, "Set 2":bool}
  in  "PID Gains":T9={"Set 1"={"proportional gain (Kc)"=0, "integral gain (Kc*Ts/Ti)"=5, "derivative gain (Kc*Td/Ts)"=0}, "Set 2"={"proportional gain (Kc)"=0, "integral gain (Kc*Ts/Ti)"=5, "derivative gain (Kc*Td/Ts)"=0}}
  in  "Feedback On/Off":cluster{"Set 1":bool, "Set 2":bool}={"Set 1"=TRUE, "Set 2"=TRUE}
  in  "Unwinding offset":bool
  in  "FB Trap Pos Offset":dbl caption="Offset (nm)"
  in  "Negate Y Axis":bool=TRUE
  in  "Set SP to Reading":bool
  out "Trap X (AI1)":T10={"Trap 1"=-0.375, "Trap 2"=-0.381805419921875}
  in  "Trap Pos FB SP":fxp<+/-,16,1>=-0.123443603515625 caption="Setpoint"
  in  "Trap Pos. FB ON":bool
  in  "Reset Trap Pos. FB":bool
  out "Trap Positions":waveform(dbl)[](graph)=[{"t0"=timestamp(9589.800000000116 s since 1904-01-01), "dt"=0.15, "Y"=[0.0, 0.0], "attributes"=variant("NI_ChannelName"=variant(string "Trap 1 Pos."))}, {"t0"=timestamp(9589.800000000116 s since 1904-01-01), "dt"=0.15, "Y"=[5.5933924159035087e-11, 5.5933924159035087e-11], "attributes"=variant("NI_ChannelName"=variant(string "Trap 2 Pos."))}]
  in  "Tab Control 8":enum32{"Main Setting", "Details"}(tab)=enum."Details"
  in  "Trap Pos FB Int Count":u16=100
  in  "Trap Pos. FB Gains":T11={"proportional gain (Kc)"=10.0, "integral gain (Kc*Ts/Ti)"=10.0, "derivative gain (Kc*Td/Ts)"=0.0} {"proportional gain (Kc)" format="%.11g"; "integral gain (Kc*Ts/Ti)" format="%.11g"; "derivative gain (Kc*Td/Ts)" format="%.11g"}
  in  "Trap Pos. FB Offset Factor":i64
  in  "Trap Pos FB Negate Action":bool
  in  "Trap Pos. FB Mult Factor":i64=8388608
  in  "Trap Pos. AI1 X Pre-scale":u16
  in  "Trap Pos. FB Range":T12={"output high"=0.999969482421875, "output low"=-1.0}
  out "Trap Pos FB Int Signal":fxp<+/-,24,9>=-5.86773681640625 format="%.18g"
  out "Trap Pos FB Int-Norm Signal":fxp<+/-,16,1>=-0.058685302734375 format="%.16g"
  in  "Set SP Using...":bool
  in  "Trap Pos FB Monitor\nT1 or T2":bool
  out "Trap X AI1 (DMA)":T13={"Set 1"=-0.700286865234375, "Set 2"=-0.70166015625}
  in  "N El. to Ave.":dbl=10000.0
  out "Trap Pos FB Action":i64=-32768
  out "Action (%)":dbl(knob)=-100.0030518509476 scale=-100.0..100.0
  in  "Trap Pos. FB Out Scale 2^n":u8=25 caption="Action Scale"
  out "Mean T1 Position (nm)":dbl caption="Mean T1 (nm)" format="%0.2f"
  out "Trap 1 Position RMS (A)":dbl caption="RMS (Ang)"
  in  "Remove Action Offset":bool
  in  "factor":dbl=0.8
  in  "Tab Control 3":enum32{"Timing", "MCL Scan", "Analog Out"}(tab)
  out "APD 2 Gate Late Counter":u32
  out "APD 2 Gate Relative Phase":i16
  in  "Phase Adj. (APD 2 Gate)":i16=20
  in  "Initial Phase Adjustment (APD 2 Gate)":i16=55
  out "APD 1 Gate Late Counter":u32
  in  "- phase (APD 1 Gate)":bool
  in  "+ phase (APD 1 Gate)":bool
  out "APD 1 Gate Relative Phase":i16
  in  "Phase Adj. (APD 1 Gate)":i16=20
  in  "Initial Phase Adjustment (APD 1 Gate)":i16=60
  in  "Save APD Data\nwith Trap Data":bool=TRUE
  out "APD FIFO Elements Remaining":u32
  in  "- phase (APD Acq)":bool
  in  "+ phase (APD Acq)":bool
  out "APD Acq Late Counter":u32
  out "APD Acq Relative Phase":i16
  in  "Phase Adj. (APD Acq)":i16=20
  in  "Initial Phase Adjustment (APD Acq)":i16
  in  "Invert APD Gate":bool caption="Invert Gate"
  in  "APD Gate OFF Count":u32=450 caption="Gate OFF Count"
  in  "APD Gate ON Count":u32=150 caption="Gate ON Count"
  in  "APD Gate":enum32{"ON", "OFF", "Interlace"}(radio)=enum."Interlace"
  in  "APD Integration Time (s)":dbl=0.01 caption="Integration Time (s)"
  out "APD Acq Rate (Hz)":dbl=100.0 caption="Rate (Hz)"
  out "APD Samples/FIFO Acq.":dbl=30.0
  out "APD Elements/DMA read":u32=60
  out "APD Int. Count":u32=400000 format="%.0p"
  in  "+ phase (APD 2 Gate)":bool
  in  "- phase (APD 2 Gate)":bool
  in  "Tab Control 5":enum32{"PSD X", "PSD Y", "Other Data Channel"}(tab)
  out "Data map":dbl[][](graph)=[[-0.1333528275848164, -0.13322457942865132, -0.13338141499330441, -0.13315516332872823, -0.13349963906401516, -0.13359534704399442, -0.1336383102533325, -0.1334437596814232, -0.13351009901028432, -0.133174726924376, -0.13353618610342308, -0.13341430673495425, -0.1337791921327295, -0.13336672306878955, -0.13358485673285964, -0.13386556704797015, -0.13364109162411741, -0.1331515440816014, -0.13347705703506113, -0.13332438096152477], [-0.13330982878455255, -0.1332750495144987, -0.13319436165006812, -0.13320436012398332, -0.13337780682419856, -0.13318346406303316, -0.13354384273485564, -0.1335553857723867, -0.1333855860720205, -0.13344880369084505, -0.13331726120488946, -0.13359903256786615, -0.13374990418036614, -0.13320003077320358, -0.13320258284496916, -0.13349625923097894, -0.13341762191515427, -0.13321738360286317, -0.13365332165632604, -0.13336876386087104], [-0.13338432873053255, -0.13369836704787957, -0.13302853528383926, -0.13284664713529393, -0.13331163931728274, -0.1333869240906723, -0.1333441110818246, -0.13363613855507872, -0.13328973057954627, -0.13338978606911753, -0.13344572107757746, -0.1335788632456775, -0.13369207672074693, -0.1333552666645917, -0.133366088161167, -0.13353851024718505, -0.13344522029848654, -0.13326189706976171, -0.13331998061539002, -0.1334005748287191], [-0.133325559644922, -0.13328193405696326, -0.13298363395722104, -0.1327420972940746, -0.13319836061291315, -0.13335561564627363, -0.13332406410277234, -0.1332193936628136, -0.133421455482787, -0.13322247098645962, -0.1334396039903118, -0.13383402308145578, -0.13367469216535152, -0.13342428864571734, -0.13322726574810206, -0.13374616438110215, -0.13359839386433672, -0.13308981369306616, -0.13346933931556157, -0.13356004700673044], [-0.13318759427178156, -0.13303197461884955, -0.1329474628909061, -0.13247541089967585, -0.1329154393010578, -0.13306639647153298, -0.13294170402663102, -0.13330832394952757, -0.13324788676517313, -0.13321368995590022, -0.1332902540311242, -0.13330558882916305, -0.13358290232698766, -0.13297453395748215, -0.13345940796964523, -0.13370893335312267, -0.13345621914098815, -0.1329981434590732, -0.13351225698035923, -0.13366090449522447], [-0.1330195631246013, -0.1332342730086348, -0.13270649932352258, -0.13215920438073567, -0.13266516267281567, -0.13295697773848095, -0.13293578982905166, -0.13287245269750408, -0.13242956314631302, -0.13269915277373706, -0.13276507119029501, -0.1330605974520571, -0.13298007789861815, -0.13297345004496647, -0.13322005694115485, -0.13306352360169843, -0.13330195770575692, -0.13273863763579463, -0.13328311983926244, -0.1334693235390487], [-0.13266227273000536, -0.13265909726526673, -0.13248512915752836, -0.13206858076806094, -0.13237793289780897, -0.13264412379816848, -0.13258756757327542, -0.1320114058200433, -0.13177271172238408, -0.131641684580745, -0.1313885201234832, -0.13157327086959134, -0.13193681668173818, -0.13205110975662787, -0.13214611067498203, -0.1325055082405619, -0.13286551272419084, -0.1327044073944107, -0.13314434714805756, -0.13328319140887135], [-0.1322287995794756, -0.13244081796536053, -0.1320813927793243, -0.13167992350139204, -0.13159036903481355, -0.1309389927960272, -0.13012719192929267, -0.12950031847514665, -0.1287847279946542, -0.12849799334601392, -0.12875851379831316, -0.1291683370175165, -0.12945041921408823, -0.13011135722738026, -0.13068229553908456, -0.13178041385585593, -0.13210874887914992, -0.13240101800950432, -0.13307651459147396, -0.1332815698201827], [-0.13168864185361212, -0.13169057747645646, -0.13094174949231982, -0.1296062475621515, -0.12911771760332813, -0.1277654225075574, -0.12620502956235657, -0.12542678436739468, -0.12488401076433495, -0.12466156919740522, -0.12464721211960658, -0.12569461568122886, -0.12655494067992784, -0.12794364582857165, -0.12901026270421723, -0.13041242181451723, -0.1309906967933238, -0.13192115434221466, -0.13278733750759975, -0.13294457795155415], [-0.13140698916298538, -0.13053117104461706, -0.1298789379990306, -0.12819663899680442, -0.12676039208733167, -0.12543956236126258, -0.12399151681160528, -0.12321545134257084, -0.12266144922386354, -0.12308476056426831, -0.12333356428193396, -0.12442839177134496, -0.125361994472599, -0.1263601593064314, -0.12820727599853887, -0.1295078859250952, -0.13070166715851583, -0.13132458320754442, -0.13239984696061652, -0.13272823213845275], [-0.1316630563769322, -0.13058177067274154, -0.12934738039745952, -0.1279160589030836, -0.12698760416503796, -0.1261278846897266, -0.12563290805554983, -0.12525048180917475, -0.12499775033256465, -0.12548503096818717, -0.12562927805994936, -0.12652509628180203, -0.1268728117841831, -0.12754090298678572, -0.128892648954199, -0.1303663985392085, -0.13107103289262145, -0.13211332838117568, -0.13253399544795413, -0.13320687544530033], [-0.13216081866528823, -0.1315075999575009, -0.13100587070574482, -0.12992811693100018, -0.12997653166936626, -0.1292147140061146, -0.129640492236645, -0.12897956592947535, -0.12976715583017567, -0.1297932787035981, -0.1298023450792772, -0.13032188725883695, -0.1304761361878746, -0.13078161341726655, -0.13166629776722513, -0.13222471508906133, -0.1323213695353957, -0.1328207574902124, -0.13311501551624966, -0.1332632433913324], [-0.13281254318355107, -0.1327562901435425, -0.1326441296540774, -0.13233527591102084, -0.13266449238724481, -0.13265305237392538, -0.1332895530560203, -0.1328797037513923, -0.1337875611075738, -0.1338856032262169, -0.13396272235535894, -0.13467820635255304, -0.13459472658495253, -0.13481512721792738, -0.13510227952708725, -0.13479149504020294, -0.1342173989040399, -0.13400692912651818, -0.13384849198616516, -0.13400637529892312], [-0.13375357959243867, -0.13404569542560457, -0.13495364446143102, -0.1348249298919473, -0.13511113811042258, -0.13586064734534106, -0.1367702427345483, -0.13640277389675376, -0.137350097056054, -0.13768947654536537, -0.1377600167625419, -0.13864975659183087, -0.13855745695114235, -0.13847369645672247, -0.13797396835814926, -0.13685971442597938, -0.13588001721479026, -0.1348828617294378, -0.13459338431719314, -0.13430841037731373], [-0.13472163516252944, -0.13510778933514528, -0.13606324391762598, -0.13721477688556563, -0.13796918063942398, -0.13907970504607353, -0.13997063223219003, -0.1404952519216667, -0.14116015514376445, -0.14184210813677695, -0.14195006345681294, -0.1422200144829778, -0.14146161292344456, -0.14066503891408247, -0.13917249864709688, -0.13787213188733544, -0.13644632375244403, -0.13531181544046453, -0.13475242805372128, -0.13409655719999836], [-0.1346275621787114, -0.13581997744258686, -0.13673753910551079, -0.13825764083372993, -0.1393970856121808, -0.14055132722262284, -0.14212435341131746, -0.1429946497851761, -0.14389674915902945, -0.14437685341315143, -0.14394884392741297, -0.1437461923774046, -0.14212089804047442, -0.14062257694636499, -0.1389648070082139, -0.13735907714557666, -0.13619045970534122, -0.13491396011330425, -0.13433155550518988, -0.13385926149247016], [-0.1345463015984732, -0.13533049006777814, -0.1360079415666268, -0.13724519284297043, -0.13796266414019026, -0.13972197426375965, -0.140812875728494, -0.14160716758492864, -0.14245424606827867, -0.1426660914472218, -0.1419273669362709, -0.1411193505685126, -0.1396820763279355, -0.13849550538403904, -0.1371160534173631, -0.13616108727356172, -0.1350846968502612, -0.1345579784231545, -0.13422057092103412, -0.13391963188088524], [-0.1345140812644617, -0.13453873857919768, -0.13492439205985124, -0.13522924105885664, -0.13553263780450764, -0.13682685486563656, -0.13746523593705381, -0.13769959429766693, -0.13823681534599064, -0.13804540570103968, -0.1377168473234902, -0.137249678692798, -0.13663158321787355, -0.1358724287761378, -0.13508757455503823, -0.13481824547523152, -0.13451280366787882, -0.13405512825859384, -0.13357356099604073, -0.13361557829424386], [-0.13375329911523637, -0.1339884743615168, -0.13405049775855704, -0.13387302958751493, -0.13446815488578315, -0.13456307392704003, -0.1348368701021389, -0.1346671744649869, -0.1351616786066821, -0.13494184842817455, -0.13482617852864523, -0.13488001595602087, -0.13479250678601862, -0.13422794469954447, -0.13407231195254116, -0.13428834815292778, -0.13391074942860734, -0.1335842092801955, -0.13360705080299462, -0.13369073131918308], [-0.13342007903772915, -0.13363428924338872, -0.1336865137711592, -0.13362267437830241, -0.1340879064681812, -0.1343702460433723, -0.13427212990252296, -0.13438113623254638, -0.1342984197115018, -0.13454000136156902, -0.13410240023843895, -0.13431191302358195, -0.13372696338190082, -0.13351446601080696, -0.13369323044331194, -0.13382214512554041, -0.1335590429270594, -0.13334703606343876, -0.13344861559376253, -0.13363740432965837], [-0.13345101950898047, -0.13370694960200571, -0.13375272427901636, -0.13367615478109512, -0.133581419993757, -0.13404024017347133, -0.13403381313279544, -0.13412766960211026, -0.13408917169871215, -0.1340991529228964, -0.13394020765617004, -0.13411866463837074, -0.1338152058493298, -0.1334965001552756, -0.1336131483128123, -0.13359828229506895, -0.13336465129415692, -0.13314738412311986, -0.13348416355472054, -0.1335604277916293], [-0.13306505037644084, -0.13323849362189907, -0.13358463035347495, -0.13325024737032973, -0.1339034907224333, -0.1334823513422517, -0.13364118194855779, -0.13370487605571307, -0.13388403686022388, -0.13370936861025146, -0.13365536795624064, -0.13368173604417122, -0.13323022669565254, -0.1334299644310924, -0.13347931020293585, -0.13352842249169267, -0.13337684428363186, -0.13325924288621083, -0.13329745168878554, -0.1337439591709793], [-0.13329253323559506, -0.1331777915331699, -0.1335921549944053, -0.1328937870573285, -0.1332366580681567, -0.13343263834499086, -0.1334011301059611, -0.1333309838285126, -0.13350159936016623, -0.13320469976499644, -0.13344779732284073, -0.1334547498891746, -0.1334222219690806, -0.13318482310735769, -0.1335076304440751, -0.1337210081454326, -0.13315452452181906, -0.1334159900117032, -0.13341932871289236, -0.13354841337059192], [-0.13280291955733525, -0.13325064759222977, -0.13311404335060162, -0.13248463689492918, -0.1333237715792868, -0.1323786195149216, -0.13271644461940252, -0.13281630630206784, -0.13288259797605967, -0.13249986045502704, -0.13281665454186062, -0.13272056012529576, -0.13286471860468907, -0.13278402529871713, -0.13291014412980584, -0.13297993805663647, -0.13300434625587784, -0.1330929771016705, -0.13330992360244986, -0.13370648866336798], [-0.13245142727010079, -0.1327511055284677, -0.13268045863644556, -0.13268143112611724, -0.1325461389457877, -0.13209427203867338, -0.1321009552727226, -0.13225536226981105, -0.13186019651868192, -0.13057556692968597, -0.13114921940462385, -0.1309652877414555, -0.13152741909874535, -0.1317933488461379, -0.13157278355428226, -0.1320550574560594, -0.13258159805880432, -0.1325290720118073, -0.1330325946278319, -0.13335799111764524], [-0.132440641977841, -0.13223274943079838, -0.13289269966476258, -0.13166651817936692, -0.13145823100189755, -0.13071613425469086, -0.1305561586856538, -0.1298730961500496, -0.12931009768505008, -0.1282939344060649, -0.12877776236794292, -0.12861422530652827, -0.12939444719778675, -0.12959820237747077, -0.12982084600249316, -0.13091293127431075, -0.13161604230879553, -0.13196152998858568, -0.13235636411870588, -0.13286676513248602], [-0.1320090784600222, -0.1320251702775283, -0.1320201366202131, -0.1308841791296303, -0.13024919149293854, -0.12882972626185074, -0.12841801068211917, -0.1277257404207089, -0.12729636083194423, -0.12612102323152535, -0.1266176500993184, -0.12699800464045685, -0.1273436224975044, -0.12801691442078328, -0.1285301864636645, -0.12982378997391497, -0.13037226121792483, -0.1309877220002564, -0.13195835248531285, -0.1327283377905438], [-0.13219445798910656, -0.13188688269527568, -0.1312592281486657, -0.12974550875405527, -0.12950618274953632, -0.1282777123290045, -0.12815500917958844, -0.1276867543572287, -0.12753413346428072, -0.12700805569043083, -0.12731245292472204, -0.12733022642180977, -0.12794125592111183, -0.12787103039057496, -0.12851092699043953, -0.12941433262690494, -0.1302167567007781, -0.13097544099877062, -0.1313019129364665, -0.13256884384406073], [-0.13203935721135476, -0.1319797555557467, -0.13125504649143416, -0.1306737121404095, -0.13023153377695054, -0.12962817928808207, -0.12967599795049806, -0.12935147357664667, -0.12930920917934416, -0.12932450565660736, -0.12960389680547735, -0.12972037405457418, -0.1297802847172711, -0.12990558188238963, -0.12998660414360977, -0.13060943118902887, -0.1309291374525452, -0.13126102756068508, -0.1317875372713273, -0.13289602021495517], [-0.13237209389326543, -0.13252267873479864, -0.1322605318662779, -0.13185876549480874, -0.13161073280800273, -0.1316314093234348, -0.13175685738586845, -0.1316715289616997, -0.13176387169644788, -0.13178347463822943, -0.13222097937928162, -0.13203755361500033, -0.13189928703016512, -0.13207046955652132, -0.13193239985056698, -0.13238530821059563, -0.13213549192663696, -0.13225053431681083, -0.13249723798670127, -0.13277852346573402], [-0.13294465237215997, -0.1331343744731282, -0.13315537746712325, -0.13297264620540483, -0.13297221070219528, -0.1331608555788659, -0.1337974354021675, -0.13366029282378541, -0.13397829019364643, -0.13347118333006328, -0.13380547261304465, -0.13415791553132203, -0.13436743143778923, -0.13416465137955633, -0.1336944626800391, -0.13391189855159902, -0.13350966407890932, -0.13366670150662655, -0.13368039256028455, -0.13347009962509598], [-0.133376600865105, -0.13395481344944193, -0.1339955846830665, -0.133956967884642, -0.13444739915933085, -0.13480443484205623, -0.13553775345604469, -0.13577815788119485, -0.13626241644698478, -0.13578778100304814, -0.13600939090830583, -0.13605401743367845, -0.1363863505755896, -0.13632887707726826, -0.13590477361164166, -0.13548728900052692, -0.13504306343454786, -0.13434553140256977, -0.134204688920121, -0.13377243388378493], [-0.1336682588237614, -0.13422447217878333, -0.13491126661397695, -0.13489108653969023, -0.1356255820450017, -0.13641858768724696, -0.13726032358608364, -0.13756147425761883, -0.13826732839332784, -0.13787068229003774, -0.13819141478504252, -0.13814020164934854, -0.1383025679443424, -0.13767489897776403, -0.1370517969258808, -0.13651091961430573, -0.13533791682069152, -0.13495068828901735, -0.13448202290108713, -0.13383517463969868], [-0.13388448192593644, -0.13452246644280663, -0.1348825936438942, -0.13548641134956727, -0.13607722308562042, -0.1369913125177349, -0.13804634592340168, -0.1385997471309521, -0.1393396940160915, -0.13934838346032416, -0.13920885511607672, -0.13948125985373397, -0.13893318047380865, -0.1379397712645341, -0.13715709296524092, -0.13626258823899745, -0.1353994598816213, -0.1347628519489198, -0.1342948953293206, -0.1338826651952545], [-0.13396856227055137, -0.13388308324032946, -0.1349033619784188, -0.13485684121421254, -0.1358148424531872, -0.1365104818532411, -0.13741175304944797, -0.13811134914899487, -0.13850002869344977, -0.13841450536318534, -0.13862883436250045, -0.13852386431366803, -0.13818160725162842, -0.1369681240039362, -0.1362562280554694, -0.13548377081345972, -0.13483066956948572, -0.13443735012047295, -0.1342378731397958, -0.13377307509823724], [-0.13356343572314888, -0.1341941365836396, -0.1342048717962691, -0.13437430888148577, -0.13448523278647978, -0.13473340434566053, -0.13563618405175148, -0.13570696814363353, -0.13620209549575168, -0.13629332827180524, -0.1360534850897276, -0.13616043752292084, -0.13581500811714792, -0.13516798139559938, -0.13479299366693354, -0.1341684228711022, -0.13401951858470776, -0.13409658215468903, -0.13379318780279842, -0.13390389491094368], [-0.1333330167529305, -0.13362161369838121, -0.1338481709725886, -0.1338547076999006, -0.13402849942936956, -0.13371246447901386, -0.13406075991101218, -0.1346068155255807, -0.13448339135153925, -0.1343697655445329, -0.13433244392480195, -0.1347059206824048, -0.13430621020656403, -0.13398494532138386, -0.13408981243260248, -0.1339676492377287, -0.13363640585529052, -0.133463268599468, -0.1337636217634856, -0.13313319646196237], [-0.13339001677501267, -0.13356763117486625, -0.1335138731471422, -0.13369904065728763, -0.13356265784698806, -0.13393646575303964, -0.13379523451932357, -0.13422171713427905, -0.13424327801179983, -0.13430096809440317, -0.1340738456131889, -0.13400142245434493, -0.13425066634473476, -0.13324811503065892, -0.13383708673162248, -0.13367917914076613, -0.13306466082536614, -0.13363437140568288, -0.13351391502054588, -0.13366421283666058], [-0.13340084146025155, -0.13360379024948849, -0.1331487959310442, -0.13371310305092954, -0.13353330390356052, -0.13374704532881462, -0.1339920647140691, -0.13400128635678848, -0.13403768677352734, -0.1340789146755405, -0.1338463733795615, -0.13397139870497204, -0.13388109750858204, -0.1338416154765018, -0.13375936615743866, -0.1334771725677485, -0.13331791869274598, -0.13357071928634118, -0.13323267315952836, -0.1336530524531351], [-0.1332864922744885, -0.13355810189570258, -0.1333536633933724, -0.13342457051287818, -0.13360138120726672, -0.13342527909246157, -0.13348951207010357, -0.13395044891119165, -0.13383389597868128, -0.1338742842122126, -0.13356563240167563, -0.13390620276042048, -0.13383512262365405, -0.13344925360869556, -0.13366710661155234, -0.1334383076256932, -0.13325524216196766, -0.13304944832786095, -0.13323367495327598, -0.13339053344025073]]
  in  "Channel":i32=4
  in  "Abort MCL Scan":bool
  out "MCL Scan I":u64=2
  out "MCL Scanning":bool
  in  "Start MCL Scan":bool
  out "wait to reset values":bool
  in  "Tab Control 4":enum32{"Scan Settings", "MCL FPGA Loop Timing"}(tab)
  out "Total Time (s)":dbl=48.0
  in  "Scan lines (y)":u64=20
  in  "Fast Scan Dir":bool=TRUE
  in  "2D or 1D Scan":bool=TRUE
  out "Initial X":dbl=1.0296389660328993
  out "Initial Y":dbl=4.906247662064187
  out "Time/f+b scan (s) (MCL)":dbl=2.4 caption="Time/scan (s)"
  in  "Number of scans (MCL)":u64=1 caption="Scans"
  in  "Scan steps (MCL)":u64=40 caption="Scan steps (x)"
  in  "N APD Samp/step":dbl=3.0
  in  "Scan Range (V)\n(of steps)":dbl=3.5
  in  "Restart DMA? (MCL)":bool=TRUE caption="Restart DMA?"
  in  "Continuous MCL Scanning":bool caption="Cont. Scanning"
  in  "Center Scan":bool=TRUE
  in  "Save Data (MCL)":bool=TRUE caption="Save Data"
  out "Actual Incr. int (MCL)":i16=294 caption="Incr. int"
  out "Desired incr (int)":dbl=294.0628205128205
  out "Desired Scan Incr (V)":dbl=0.08974358974358974
  out "N sets should be saved (MCL)":dbl=160.0 caption="N sets should be saved"
  out "Data points/scans (MCL)":dbl=4800.0 caption="Data points/scans"
  out "Data points/scan (f+b)":dbl=240.0 caption="points/scan (f+b)"
  out "Cycles/step (MCL)":u64=2000 caption="Cycles/step" format="%.0p"
  out "Actual MCL Inc (V)":dbl=0.08972441785943175
  in  "Phase adjust (MCL)":i16 caption="Phase adjust"
  out "Relative Phase (MCL)":i16 caption="Relative Phase"
  in  "Initial Phase Adj. (MCL)":i16 caption="Initial Phase Adj."
  in  "Update Count (MCL)":u32=600
  in  "+ phase (MCL)":bool
  in  "- phase (MCL)":bool
  out "MCL Late Counter":u32
  in  "APD 1 AO Mult.":i16=1 min=1
  in  "APD 2 AO Mult.":i16=1 min=1
  in  "Tab Control 7":enum32{"Green FB Signals", "Slow MCL Scan"}(tab)
  out "Green FB Plot":dbl(graph)=-0.013428144169438765
  out "MCL Scan 2":cluster{"Begin (V)":dbl, dbl, dbl[]}(graph)
  out "MCL Scan":cluster{"Begin (V)":dbl, dbl, dbl[]}(graph)
  in  "Green laser mode":enum32{"Laser ON", "Laser OFF", "Interlace"}(radio)=enum."Interlace"
  in  "GI Frequency, ON count":u32=150 min=1 step=1
  in  "Invert GI":bool
  out "GI Late Counter":u32
  in  "Phase adj. (GI)":i16=5
  out "GI relative phase":i16
  in  "+ phase (GI)":bool
  in  "Initial Phase Adjustment (GI)":i16=19
  in  "GI Frequency, OFF count":u32=450 min=1 step=1
  in  "- phase (GI)":bool
  out "Green FB Signals (V)":cluster{"Y":dbl, "X":dbl, "Sum":dbl}={"Y"=-744.7045454545455, "X"=-744.7045454545455, "Sum"=-0.013428144169438765}
  out "Relative phase (Green FB)":i16
  in  "+ phase (Green FB)":bool
  in  "- phase (Green FB)":bool
  out "Green FB Count":u32=600
  in  "Phase adj. (Green FB)":i16=10
  in  "Initial Phase Adjustment (Green FB)":i16=50
  in  "Green FB On/Off":bool=TRUE
  in  "Current When FB OFF (%)":dbl=87.0 min=0.0 max=100.0 step=1.0
  in  "Green int current ON count adj":u32=150
  in  "Green FB Gains":T14={"proportional gain (Kc)"=10, "integral gain (Kc*Ts/Ti)"=5, "derivative gain (Kc*Td/Ts)"=0}
  in  "- phase (GI) 2":bool
  in  "Initial Phase Adjustment (GI) 2":i16=-100
  in  "+ phase (GI) 2":bool
  out "GI relative phase 2":i16
  in  "Phase adj. (GI) 2":i16=20
  out "GI Late Counter 2":u32
  in  "On one out of X cycles":u32=10
  in  "Trap Position FIFO Depth":u32=300000 format="%.0p"
  in  "# Samples/trap":u32=20000 format="%.0p"
  out "Trap AI Elements/DMA read":u32=320000 format="%.0p"
  out "Ave. Rate (Hz)":dbl=200000.0 format="%#_6p"
  out "FIFO El. Rem.":u32 format="%.0p"
  in  "Phase adj. (AI1)":i16=15
  out "Relative phase (AI1)":i16
  in  "+ phase (AI1)":bool
  in  "- phase (AI1)":bool
  out "Late Counter (AI1)":u32
  in  "Initial Phase Adjustment (AI1)":i16=220
  out "AI rate (Hz)":dbl=200000.0 format="%#_6p"
  in  "AI Count (ticks)":u32=200
  out "# Samples/channel":u32=40000 format="%.0p"
  in  "Trap AI FIFO Depth":u32=600000 format="%.0p"
  in  "Detector Type":string(combo)="IR-QPD + PSD + FB-QPD X position"
  in  "N Acq Sets (Traps + Fl.)":i16=3
  in  "Sets to FIFO (Traps)":T15={"Set 1"=TRUE, "Set 2"=TRUE, "Set 3"=FALSE}
  in  "FPGA Ave.":dbl=1.0 min=1.0 step=1.0
  out "Ave. Period (s)":dbl=5e-06 format="%#_6p"
  out "DMA Update Period (s)":dbl=0.3
  out "FPGA Averaging":bool
  out "Trap Sets":u32=2
  out "Counts/DMA":dbl=12000000.0 format="%#_6p"
  out "Trap Pos FIFO El Remaining":u32=306
  out "Trap Pos Elements/DMA read":u32=120000 format="%.0p"
  out "Trap AI FIFO Timeout":u16
  out "Trap Pos FIFO Timeout":u16
  in  "Video Capture Rate (Hz)":dbl=30.0
  in  "Video Index":dbl=1.0 min=1.0 step=1.0
  in  "New Video File":bool
  in  "Save Video":bool
  in  "Reset Averaging":bool
  in  "Averaging":bool
  in  "Save Image":bool
  in  "Image Index":dbl=1.0 min=1.0
  out "Path Out":path
  in  "Center Point":cluster{"X":i32, "Y":i32}={"X"=335, "Y"=271}
  in  "Zoom Factor":sgl=7.0
  out "Window Size":cluster{"Width":i32, "Height":i32}
  out "Window Position":cluster{"X Position":i32, "Y Position":i32}={"X Position"=40, "Y Position"=40}
  in  "Initial Window Size":cluster{"Width":i32, "Height":i32}={"Width"=884, "Height"=619}
  in  "Initial Window Position":cluster{"X Position":i32, "Y Position":i32}={"X Position"=796, "Y Position"=4}
  in  "Intensity Upper":dbl=88.0
  in  "Intensity Lower":dbl=66.0
  out "error out":errorcluster
  out "error out 2":errorcluster
  in  "Harvard Syringe Pump Serial Port":refnum<visa-resource-name>="ASRL5::INSTR"
  in  "Lost Tether Alarm Threshold (pN)":dbl=0.5
  in  "AOM X Cal (nm/MHz)":dbl=123.0
  in  "MCL X Cal (nm/V)":dbl=1070.0
  out "X RF Amplitude Limits (%)":T16={"Minimum"=0.0, "Maximum"=50.0, "Increment"=1.0}
  out "X RF Frequency Limits (MHz)":T16={"Minimum"=60.0, "Maximum"=90.0, "Increment"=1.0}
  out "Y RF Frequency Limits (MHz)":T16={"Minimum"=0.0, "Maximum"=40.0, "Increment"=1.0}
  out "Y RF Amplitude Limits (%)":T16={"Minimum"=0.0, "Maximum"=50.0, "Increment"=1.0}
  in  "Manip. X?":bool=TRUE
  in  "Manip. Y?":bool
  in  "Force Manip Abort":bool
  out "Read cal error":errorcluster
  in  "DAQ Delay (ms)":u32=1000
  in  "Start Scan":bool
  in  "Scan axis":bool=TRUE
  in  "Osc. amp. (V)":dbl=5.0
  in  "Osc. center (V)":dbl=5.0
  in  "Osc. freq. (Hz) 2":dbl=1.0
  in  "MCL Mode":u16(ring) items=["Manual Positioning", "Sinusoidal Wave", "Linear Scan"]
  in  "Begin (V)":dbl
  in  "End (V)":dbl=10.0
  in  "N Points":dbl=20.0
  in  "Delay to Interlace (s)":dbl
  in  "Delayed Interlace Start":bool
  in  "Read Lateness and Rel Phase":bool
  out "Vec Mean of T1 T2":dbl[](array[numeric])=[107.52745637613502, 108.18516687787962]
  in  "Cal read wait (s)":u32=5
  out "Time tether formed":timestamp=timestamp(3374779860.98425 s since 1904-01-01)
  in  "Sample Chamber Stage Serial Port":refnum<visa-resource-name>="ASRL4::INSTR"
  in  "Chemyx Syringe Pump Serial Port":refnum<visa-resource-name>="ASRL3::INSTR"
  in  "Limit Min (MHz)":dbl=10.0 caption="Min (MHz)"
  in  "Limit Max (MHz)":dbl=16.0 caption="Max (MHz)"
  in  "Limits Enable":bool=TRUE caption="Enable"
  out "AI labels":string[](array[string])=["T1 Y", "T1 X", "T1 Sum", "T2 Y", "T2 X", "T2 Sum", "T1 FB X", "T1 FB Sum", "T2 FB X", "T2 FB Sum", "PSD Y", "PSD X", "PSD Y Sum"]
  in  "Save Trap Pos. Data":bool=TRUE
  # "After"
  # "During"
  # "Trap On?"
  # "BD Flow ON?"
  # "Samp Flow ON?"
  # "Trap Trig. Fl."
  # "1"
  # "2"
  # "Trap Display:"
  # "APD Display:"
  # "DAQ"
  # "Trap Manipulation"
  # "Data Saving"
  # "Bead Calibration"
  # "Harvard Pump\n(sample channel for flow exp)"
  # "Chemyx Pump 2"
  # "Units: \n1 = ml/m\n2 = ml/h\n3 = ul/m\n4 = ul/h"
  # "Rate param is ul/h\nVolume param is ul"
  # "X"
  # "Y"
  # "Oscillate Set 1 freq. (debugging)"
  # "BD 1"
  # "BD 2"
  # "AOD Raster Scan"
  # "Approx. trap separations"
  # "X"
  # "Y"
  # "FPGA\nreading"
  # "DMA\ntransfer"
  # "APD Gates"
  # "APD 2"
  # "APD 1"
  # "X"
  # "2D"
  # "Y"
  # "1D"
  # "Green Laser Interlacing"
  # "Green FB Measurement"
  # "Digital Gate"
  # "Current Analog Control"
  # "Total AI Rates (NOT rates/trap)"
  # "(Samples/trap x Trap Sets)"
  # "(Samples/channel x\n8 if averaging (8 channels)\n4 if no averaging)"
  # "Trap 1"
  # "Trap 2"
  # "Flour./Trap 3"
  # "External Video Window"
  # "MCL Position Debugging"
  # "Temporary Control Storage\n(these used to be somewhere else, still want to keep them)"
  # "Y"
  # "X"
  # "Trap Position Difference Limits"
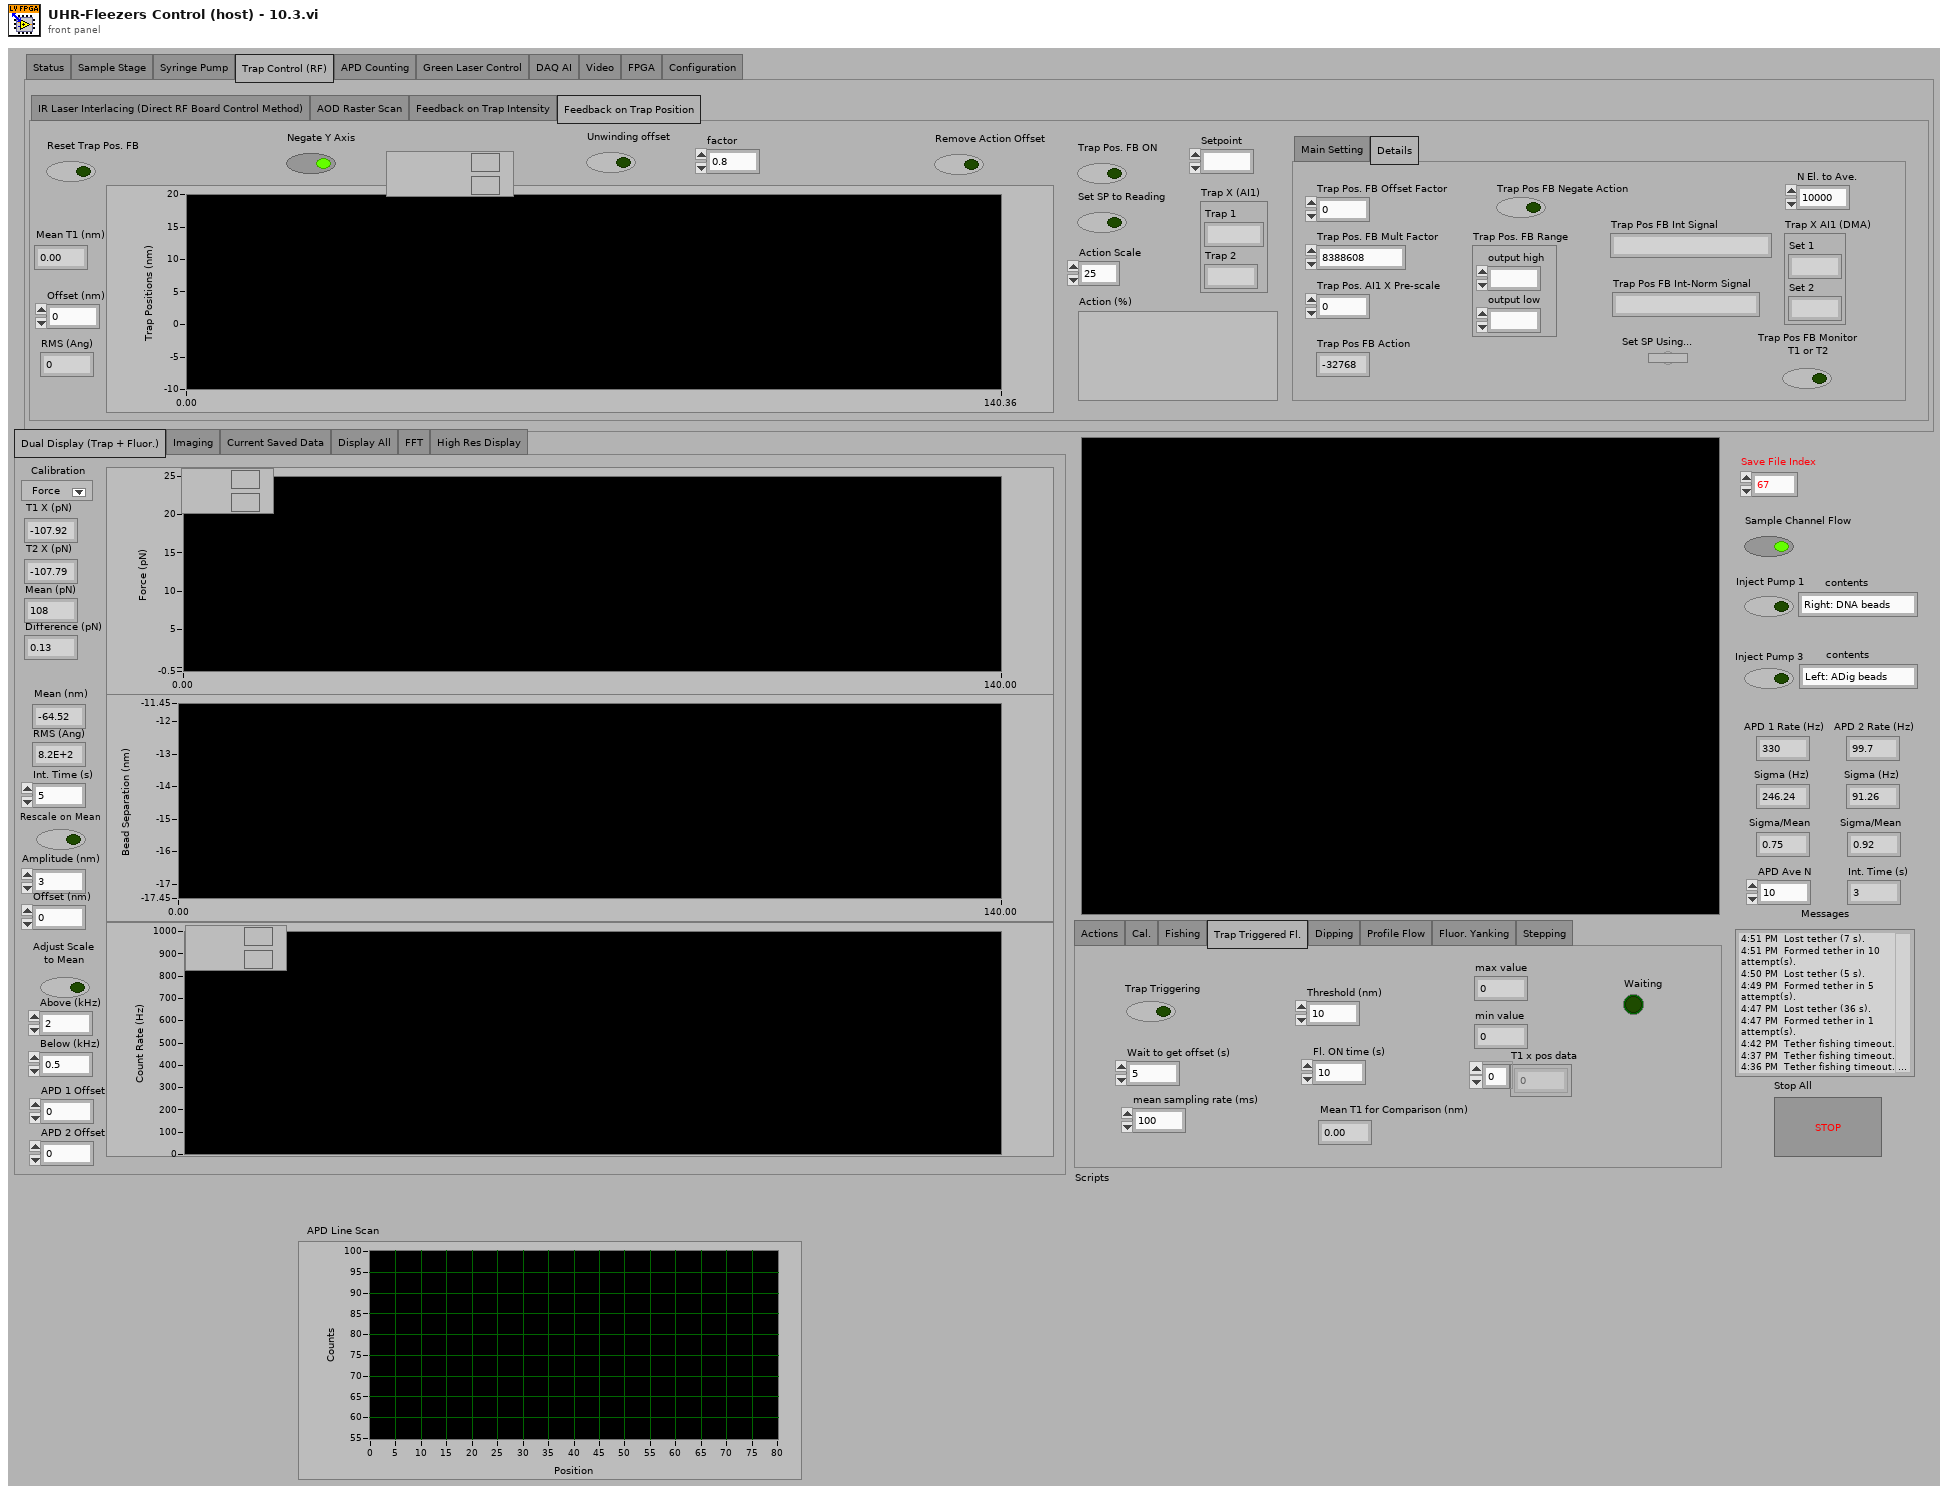
[diagram p1: front panel]
types:
  T1 = enum32{"Actions", "Cal.", "Fishing", "Trap Triggered Fl.", "Dipping", "Profile Flow", "Fluor. Yanking", "Stepping"}
  T2 = typedef "IMAQ Image.ctl" = refnum<image>
  T3 = enum32{"Dual Display (Trap + Fluor.)", "Imaging", "Current Saved Data", "Display All", "FFT", "High Res Display"}
  T4 = enum32{"Status", "Sample Stage", "Syringe Pump", "Trap Control (RF)", "APD Counting", "Green Laser Control", "DAQ AI", "Video", "FPGA", "Configuration"}
  T5 = cluster{"Pump 1":cluster{"Diameter (mm)":dbl, "Units":dbl, "Volume":dbl, "Rate":dbl}, "Pump 2":cluster{"Diameter (mm)":dbl, "Units":dbl, "Volume":dbl, "Rate":dbl}, "Pump 3":cluster{"Diameter (mm)":dbl, "Units":dbl, "Volume":dbl, "Rate":dbl}}
  T6 = enum32{"IR Laser Interlacing (Direct RF Board Control Method)", "AOD Raster Scan", "Feedback on Trap Intensity", "Feedback on Trap Position"}
  T7 = typedef "LVPoint32TypeDef.ctl" = cluster{"Horizontal":i32, "Vertical":i32}
  T8 = cluster{"Scan Range AOD (nm) 2":dbl, "Step Size AOD (nm) 2":dbl, "Scan Speed AOD (nm/s) 2":dbl, "Number of scans (AOD) 2":u16, "Label":string}[]
  T9 = cluster{"Set 1":cluster{"proportional gain (Kc)":i16, "integral gain (Kc*Ts/Ti)":i16, "derivative gain (Kc*Td/Ts)":i16}, "Set 2":cluster{"proportional gain (Kc)":i16, "integral gain (Kc*Ts/Ti)":i16, "derivative gain (Kc*Td/Ts)":i16}}
  T10 = cluster{"Trap 1":fxp<+/-,16,1>, "Trap 2":fxp<+/-,16,1>}
  T11 = cluster{"proportional gain (Kc)":fxp<+/-,16,8>, "integral gain (Kc*Ts/Ti)":fxp<+/-,16,8>, "derivative gain (Kc*Td/Ts)":fxp<+/-,16,8>}
  T12 = cluster{"output high":fxp<+/-,16,1>, "output low":fxp<+/-,16,1>}
  T13 = cluster{"Set 1":fxp<+/-,16,1>, "Set 2":fxp<+/-,16,1>}
  T14 = cluster{"proportional gain (Kc)":i16, "integral gain (Kc*Ts/Ti)":i16, "derivative gain (Kc*Td/Ts)":i16}
  T15 = cluster{"Set 1":bool, "Set 2":bool, "Set 3":bool}
  T16 = typedef "LVMinMaxIncTypeDef.ctl" = cluster{"Minimum":dbl, "Maximum":dbl, "Increment":dbl}
  T17 = typedef "Image Type" = u32
  T18 = typedef "nirio_resource_hc.ctl" = tag
  T19 = typedef "openfpgaref.8.6.ctl" = refnum<k20>
  T20 = cluster{"New Image":T2, "New Image":T2, "New Image":T2, "New Image":T2}
  T21 = typedef "XDNodeRunTimeDep.lvlib/timing_clust.ctl" = cluster{"Expected End [f-1]":u64, "Actual End [f-1]":u64, "Finished Late? [f-1]":bool, "Expected End [i-1]":u64, "Actual End [i-1]":u64, "Finished Late? [i-1]":bool, "Expected Start [i]":u64, "Actual Start [i]":u64, "Expected Start [f]":u64, "Actual Start [f]":u64, "Source Name":string, "Structure Name":string, "Period":i64, "Deadline":i64, "Offset":i64, "Start":i64, "Priority":i32, "Timeout":i32, "Mode":T22, "Wakeup Reason":T23, "Error":errorcluster, "Source Type":string, "Secondary Source Type":string, "Global End Time":u64, "Global Start Time":u64, "Frame Duration":u64, "Iteration Duration":u64, "Assigned CPU":i32, "I/O Scan Engine Mode":u32}
  T22 = typedef "XDNodeRunTimeDep.lvlib/nitl_modes.ctl" = enum32{"No Change", "Process missed periods, maintain original phase", "Discard missed periods, maintain original phase", "Process missed periods, ignore original phase", "Discard missed periods, ignore original phase"}
  T23 = typedef "XDNodeRunTimeDep.lvlib/wakeup.ctl" = enum32{"Normal", "Aborted", "Asynchronous wakeup", "Timing source error", "Timed loop error", "Timeout"}
  T24 = enum16{"big-endian, network order", "native, host order", "little-endian"}
  T25 = enum16{"open", "replace", "create", "open or create", "replace or create", "replace or create with confirmation"}
  T26 = cluster{"Scan Range AOD (nm) 2":dbl, "Step Size AOD (nm) 2":dbl, "Scan Speed AOD (nm/s) 2":dbl, "Number of scans (AOD) 2":u16, "Label":string}
  T27 = cluster{"[0]":dbl, "[1]":dbl, "[2]":dbl, "[3]":dbl, "[4]":dbl, "[5]":dbl}
  T28 = cluster{"Diameter (mm)":dbl, "Units":dbl, "Volume":dbl, "Rate":dbl}
  T29 = enum32{"Normal Display", "Dual Display (APD)", "FFT", "High Res Display"}
  T30 = cluster{"Origin Pixel":cluster{"X":sgl, "Y":sgl}, "Angle Relative to Horizontal (deg)":sgl, "Axis Reference":u32}
  T31 = typedef "Simple Grid Descriptor" = cluster{"X Step":sgl, "Y Step":sgl, "Unit":T32}
  T32 = typedef "Image Unit" = enum32{"Undefined", "Angström", "Micrometer", "Millimeter", "Centimeter", "Meter", "Kilometer", "Microinch", "Inch", "Feet", "Nautical miles", "Standard miles", "Steps"}
  T33 = cluster{"averaging mode":u16, "weighting mode":u16, "number of averages":u32}
  T34 = cluster{"dB On (F)":bool, "unwrap phase (F)":bool, "convert to degree (F)":bool}
  T35 = cluster{string, string, string, string, string, string, string, string}
  T36 = cluster{string, string, string, string, string, string, string, string, string, string, string, string}
  T37 = cluster{string, string, string, string, string, string, string, string, string, string, string, string, string}
  T38 = cluster{string, string, string, string, string, string, string, string, string, string, string, string, string, string}
  T39 = cluster{"BD 1 Frequency 1 (MHz)":dbl, "BD 1 Frequency 2 (MHz)":dbl}
  T40 = cluster{"f0":dbl, "df":dbl, "magnitude":dbl[]}[][]
  T41 = cluster{"Green FB Ch 0":i16, "Green FB Ch 1":i16, "Green FB Ch 2":i16}
  T42 = cluster{"Green FB Ch 0":dbl, "Green FB Ch 1":dbl, "Green FB Ch 2":dbl}
  T43 = cluster{"Left":i32, "Top":i32, "Width":u32, "Height":u32}
  T44 = cluster{cluster{"Left":i32, "Top":i32, "Width":u32, "Height":u32}}[]
  T45 = enum32{"setting", "request", "request control", "info", "statistics", "system settings", "I/O sub system", "HRT control", "camera descriptions", "device specific data", "event sub system settings", "event sub system results", "image memory manager"}
  T46 = typedef "AviRefnum.ctl" = refnum<k1>
  T47 = typedef "imagedata.ctl" = cluster{"image type":i32, "image depth":i32, "image":u8[], "mask":u8[], "colors":u32[], "Rectangle":cluster{"left":i16, "top":i16, "right":i16, "bottom":i16}}
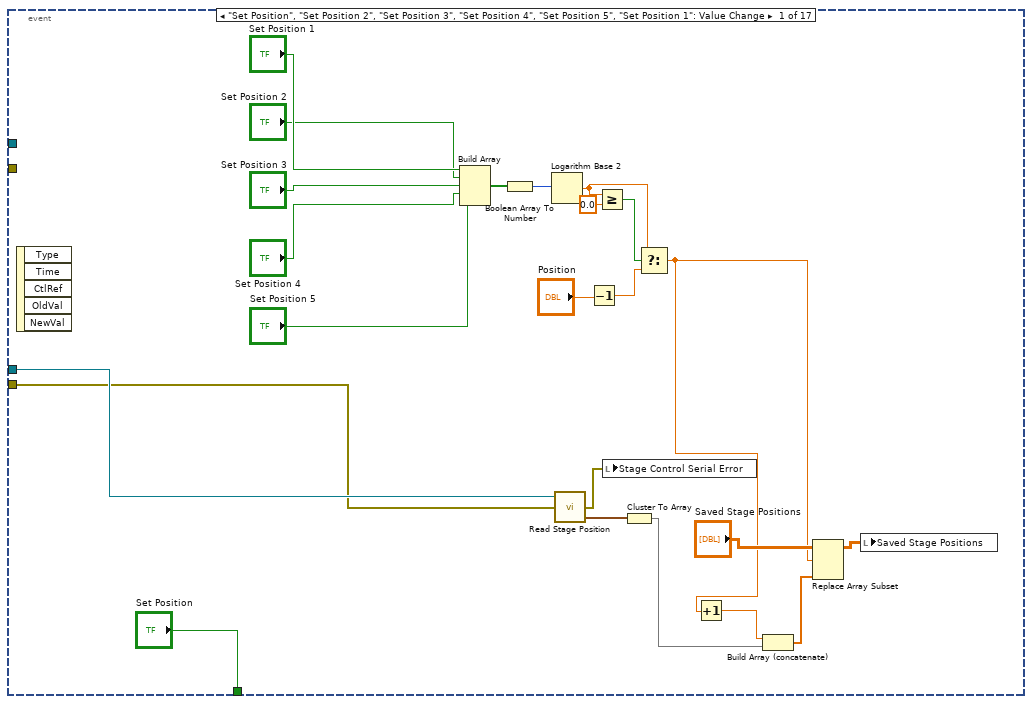
[diagram p2: hidden frame]
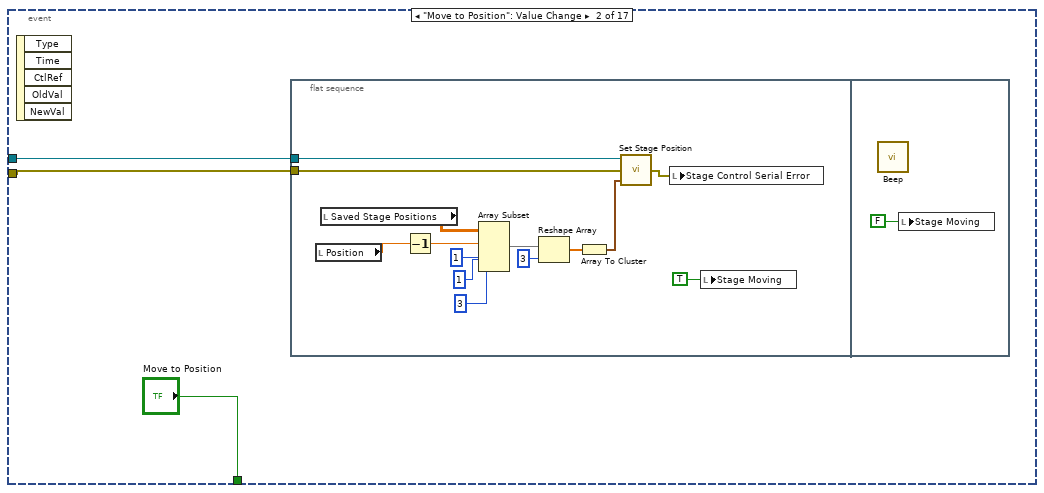
[diagram p3: hidden frame]
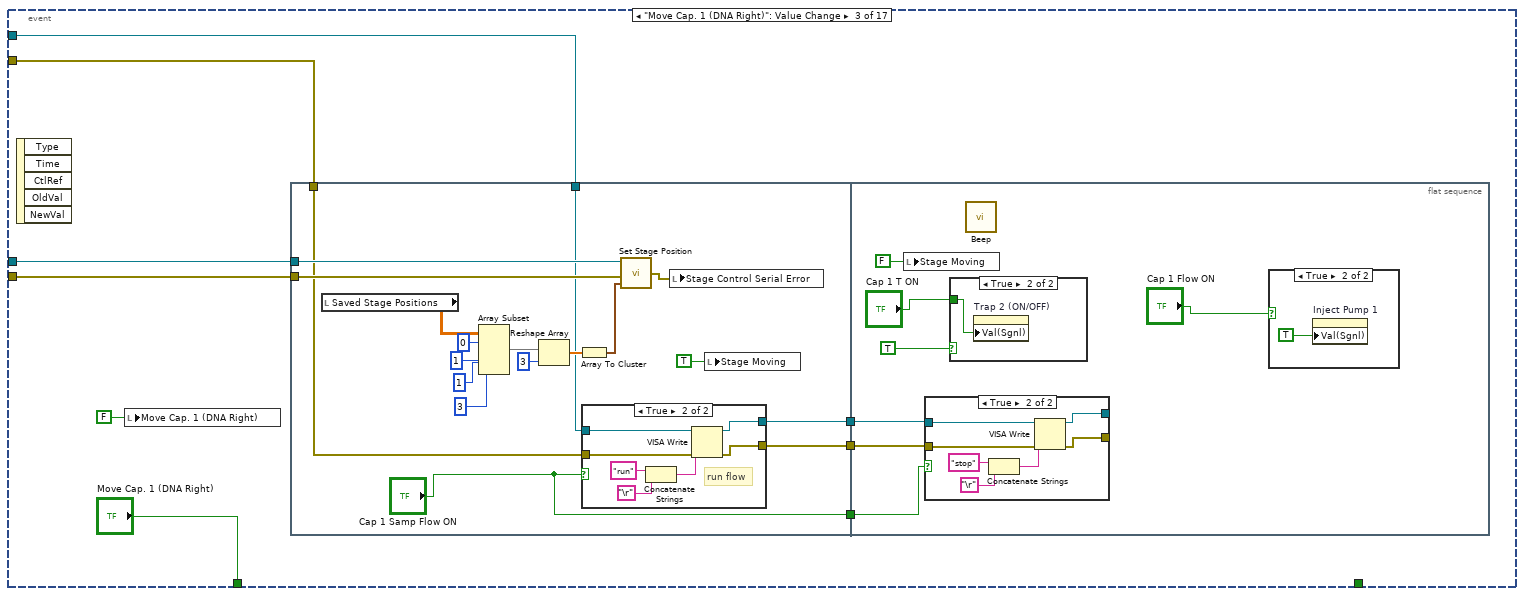
[diagram p4: hidden frame]
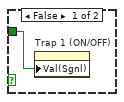
[diagram p8: hidden frame]
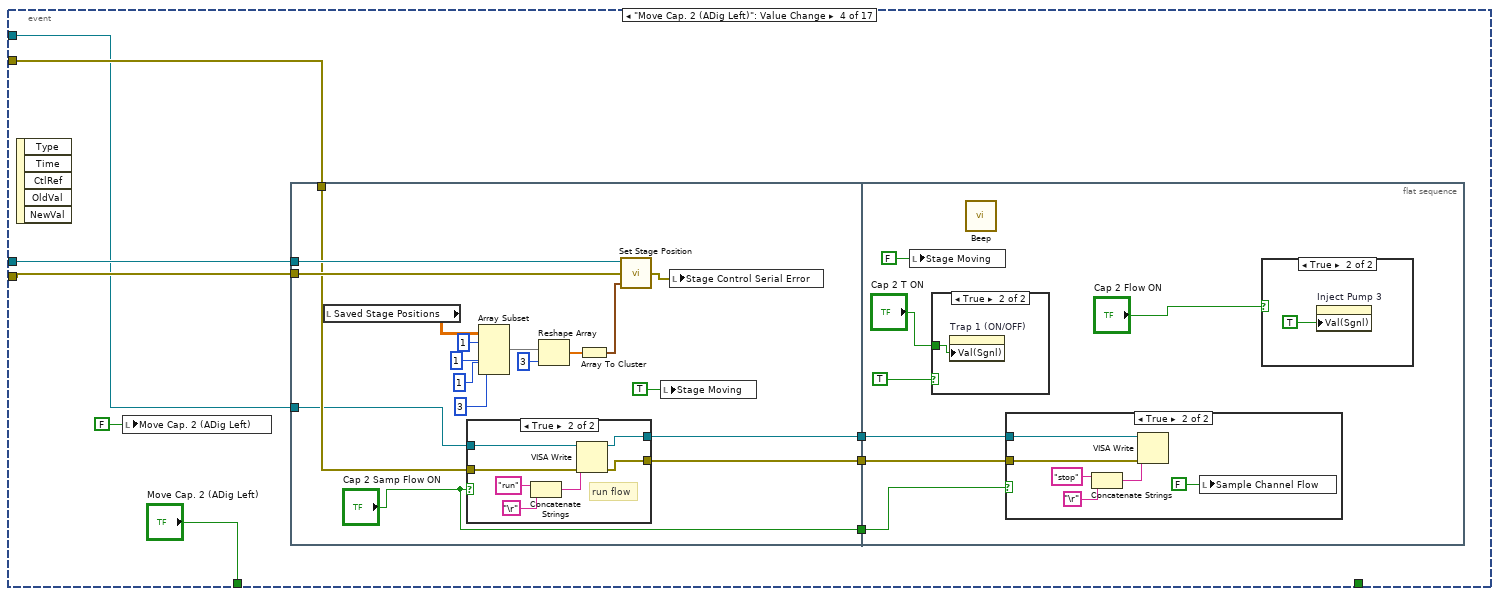
[diagram p9: hidden frame]
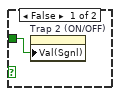
[diagram p13: hidden frame]
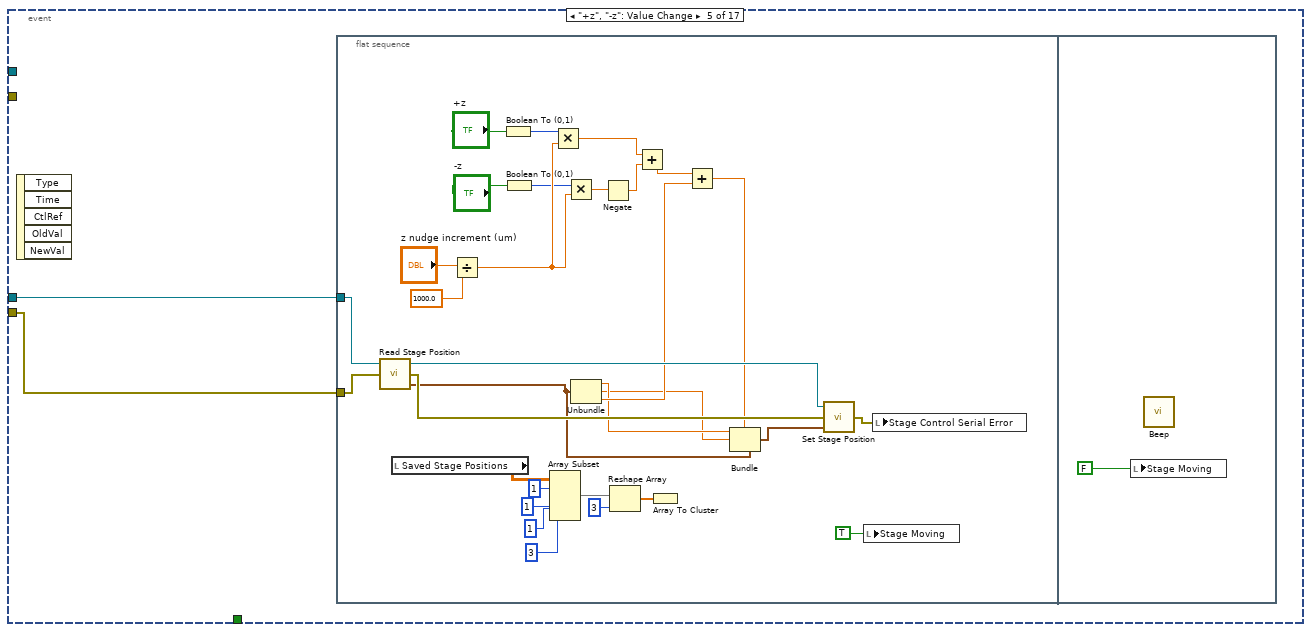
[diagram p14: hidden frame]
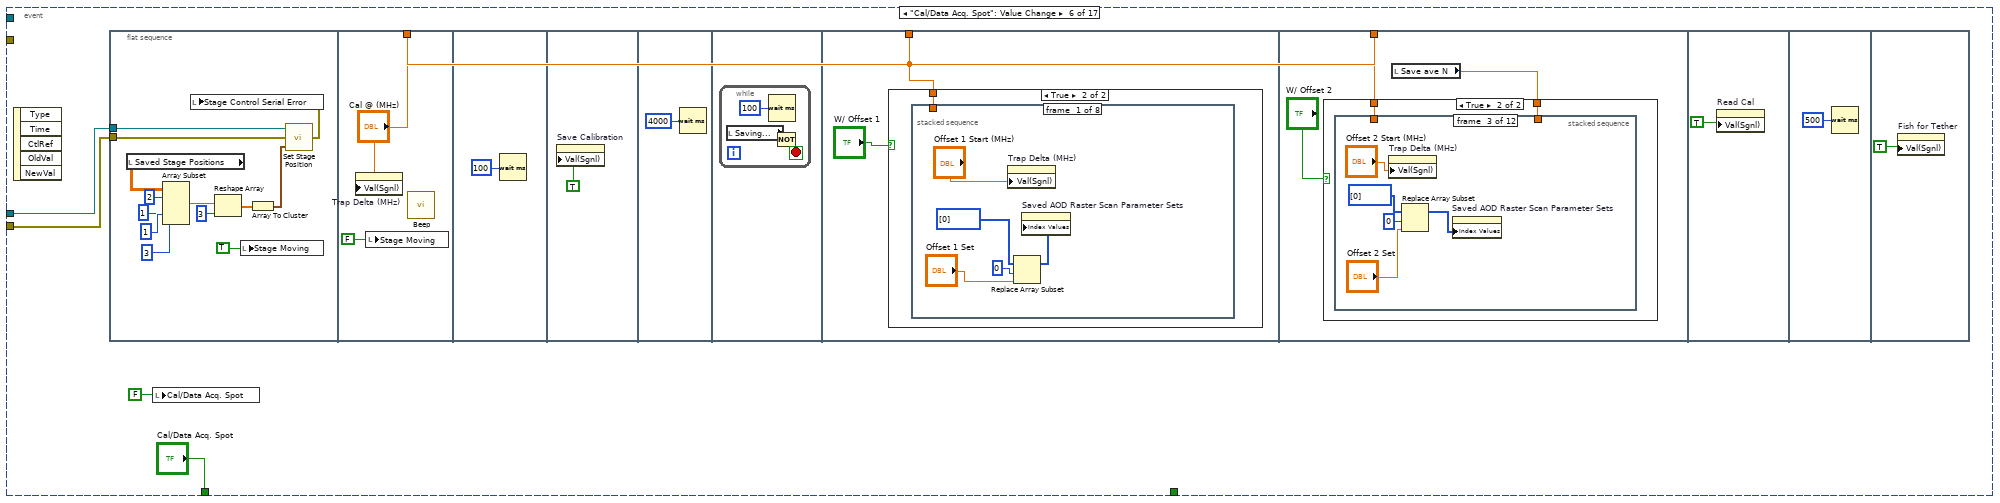
[diagram p15: hidden frame]
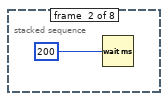
[diagram p17: hidden frame]
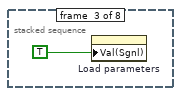
[diagram p18: hidden frame]
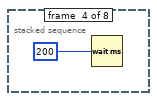
[diagram p19: hidden frame]
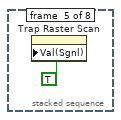
[diagram p20: hidden frame]
diagram:
  w53 = u16 20 items=["1.0"=10, "1.5"=15, "2.0"=20] ("stop bits (10: 1 bit)")
  w60 = T17 2 items=["Grayscale (U8)", "Grayscale (I16)", "Grayscale (SGL)", "Complex (CSG)", "RGB (U32)", "HSL (U32)", "RGB (U64)", "Grayscale (U16)"] ("Image Type")
  w123 = cluster{"output high":i16, "output low":i16} {"output high"=3000, "output low"=0} ("FB output range 1")
  w194 = 10.0 ("y")
  w193 = 32767.0 ("y")
  w209 = 6.0  # clock mult.
  w210 = 49152000.0  # TCXO frequ.
  n1 = Build Array("DIO count 1 (ticks)", "DIO count 2 (ticks)", "DIO count 3 (ticks)") -> (w110:u32[])
  n2 = local read "AO1"() -> (w188:dbl)
  n3 = local read "AO2"() -> (w187:dbl)
  n4 = local read "Scan Increment (MHz)"() -> (w205:dbl)
  n5 = local read "Continuous MCL Scanning"() -> (w175:bool)
  n6 = local read "Fast Scan Dir"() -> (w174:bool)
  n7 = local read "Number of scans (MCL)"() -> (w176:u64)
  n8 = property on="AI Count (ticks)" class="DigNum (strict)"("Val(Sgnl)"="AI Count (ticks)") -> ()  [unwired: 2 in, 2 out]
  n9 = Multiply(x=w188, y=w193) -> (x*y=w190:dbl)
  n10 = Multiply(x=w187, y=w193) -> (x*y=w192:dbl)
  n11 = Divide(x=w190, y=w194) -> (x/y=w189:dbl)
  n12 = Divide(x=w192, y=w194) -> (x/y=w191:dbl)
  n13 = To Word Integer(number=w189) -> (16bit integer=w186:i16)
  n14 = To Word Integer(number=w191) -> (16bit integer=w185:i16)
  n15 = Not(x=w174) -> (.not. x?=w169:bool)
  n16 = local read "Cycles/step (MCL)"() -> (w177:u64)
  n17 = Multiply(x=w205, y=1000.0) -> (x*y=w212:dbl)
  n18 = local read "Scan steps (MCL)"() -> (w178:u64)
  n19 = local write "Trap Pos FIFO Timeout"(u16 0 ("Trap Pos FIFO Timeout")) -> ()
  n20 = local read "Desired Scan Incr (V)"() -> (w180:dbl)
  n21 = Scale By Power Of 2(n=48, x=w212) -> (x*2^n=w213:dbl)
  n22 = Multiply(x=w210, y=w209) -> (x*y=w208:dbl)
  n23 = Divide(x=w213, y=w208) -> (x/y=w207:dbl)
  n24 = local read "Setpoints (V)"() -> (w227:cluster{"Set 1":dbl, "Set 2":dbl})
  n25 = To Quad Integer(1:w207) -> (0:w204:i64)
  n26 = Divide(x=40000000.0, y="AI Count (ticks)") -> (x/y=w165:dbl)
  n27 = Multiply(x=w180, y=32767.0) -> (x*y=w182:dbl)
  n28 = local read "Number Interlace Sets"() -> (w103:u8)
  n29 = Split 1D Array(array=w110, index=w103) -> (first subarray=w112:u32[])  [unwired: 1 out]
  n30 = Add Array Elements(numeric array=w112) -> (sum=w111:u32)
  n31 = local read "# Samples/channel"() -> (w197:u32)
  n32 = local read "Number of F/B Scans (AOD)"() -> (w198:u16)
  n33 = local read "Not-Interlacing Set"() -> (w102:enum32{"Set 1", "Set 2", "Set 3"})
  n34 = To Unsigned Byte Integer(number=w102) -> (unsigned 8bit integer=w108:u8)
  n35 = Index Array(array=w110, index=w108) -> (element=w109:u32)
  n36 = local read "Feedback On/Off"() -> (w230:cluster{"Set 1":bool, "Set 2":bool})
  n37 = local read "PID Gains"() -> (w222:T9)
  n38 = local read "Scan steps (AOD)"() -> (w203:u64)
  n39 = local read "All FB On/Off"() -> (w231:bool)
  n40 = local read "Cycles/step (AOD)"() -> (w202:u64)
  n41 = local write "AI rate (Hz)"(w165) -> ()
  n42 = Divide(x=w182, y=10.0) -> (x/y=w181:dbl)
  n43 = Multiply(x=w203, y=w202) -> (x*y=w201:u64)
  n44 = Multiply(x=3276.7, y=w227) -> (x*y=w226:cluster{"Set 1":dbl, "Set 2":dbl})
  n45 = xnode "Open FPGA VI Reference"("resource name"=T18 "750kHzDAQ") -> ("FPGA VI Reference Out"=w219:T19, "error out"=w218:errorcluster)  [unwired: 1 in]
  n46 = To Word Integer(number=w181) -> (16bit integer=w179:i16)
  n47 = Multiply(x=w201, y=u64 2) -> (x*y=w199:u64)
  n48 = local read "Sets to FIFO (Traps)"() -> (w234:T15)
  n49 = Divide(x=w165, y="FPGA Ave.") -> (x/y=w166:dbl)
  n50 = To Word Integer(number=w226) -> (16bit integer=w225:cluster{"Set 1":i16, "Set 2":i16})
  n51 = Unbundle By Name(w222) -> ("Set 1"=w221:T14, "Set 2"=w220:T14)
  n52 = Multiply(x=w199, y=w198) -> (x*y=w196:u64)
  n53 = local write "Ave. Rate (Hz)"(w166) -> ()
  n54 = Divide(x=w196, y=w197) -> (x/y=w195:dbl)
  n55 = Unbundle By Name(w225) -> ("Set 1"=w224:i16, "Set 2"=w223:i16)
  n56 = local read "2D or 1D Scan"() -> (w124:bool)
  n57 = local write "Data points/scans"(w196) -> ()
  n58 = local read "Scan BD"() -> (w214:bool)
  n59 = And(x=w230, y=w231) -> (x .and. y?=w229:cluster{"Set 1":bool, "Set 2":bool})
  n60 = local write "Data points/scan (f/b)"(w199) -> ()
  n61 = Reciprocal(x=w166) -> (1/x=w167:dbl)
  n62 = local read "N Acq Sets (Traps + Fl.)"() -> (w158:i16)
  n63 = local write "N sets should be saved"(w195) -> ()
  n64 = xnode "Invoke Method"("FPGA VI Reference In"=w219, "error in"=w218) -> ("FPGA VI Reference Out"=w122:T19, "error out"=w132:errorcluster)
  n65 = Unbundle By Name(w229) -> ("Set 1"=w233:bool, "Set 2"=w232:bool)
  n66 = local read "Interlace"() -> (w104:bool)
  n67 = Select(t=w111, s=w104, f=w109) -> (s? t:f=w101:u32)
  n68 = local write "Update Count (MCL)"(w101) -> ()
  n69 = local write "Total Counts (ticks)"(w101) -> ()
  n70 = local write "Ave. Period (s)"(w167) -> ()
  n71 = property on="2D or 1D Scan" class="Bool (strict)"("Val(Sgnl)"=w124) -> ()  [unwired: 2 in, 2 out]
  n72 = local read "GI Frequency, OFF count"() -> (w24:u32)
  n73 = local read "GI Frequency, ON count"() -> (w15:u32)
  n74 = local read "APD Gate OFF Count"() -> (w21:u32)
  n75 = local read "APD Gate ON Count"() -> (w17:u32)
  n76 = xnode "Read/Write Control"("FPGA VI Reference In"=w121, "error in"=w132, "ai count"="AI Count (ticks)", "Interlace ON/OFF"=w104, "Number Interlace Cycles"=w103, "AI1 Sets to FIFO"=w234, "FB On/Off Set 1"=w233, "FB On/Off Set 2"=w232, "Interlace Off Parameters"=w102, "FB Setpoint Set 1"=w224, "FB Setpoint Set 2"=w223, "FB Gains Set 1"=w221, "FB Gains Set 2"=w220, "FB output range 1"=w123, "FB output range 2"=w123, "Cycles per step"=w202, "Scan BD"=w214, "Number of scans"=w198, "Scan steps"=w203, "Scan freq.  increment"=w204, "AO1"=w186, "AO2"=w185, "Scan freq.  increment (MCL)"=w179, "Scan steps (MCL)"=w178, "Cycles per step (MCL)"=w177, "Number of scans (MCL)"=w176, "MCL count"=w101, "Cont. Scan (MCL)"=w175, "MCL Scan Axis"=w169, "1D or 2D Scan?"=w124, "N of AI1 Int Acq Sets"=w158, "Freq or Amp switch first"="Freq or Amp switch first", "Freq switch delay"="Freq switch delay", "Amp switch delay"="Amp switch delay", "Swap F1 and F2"="Swap F1 and F2", "APD to FIFO"=FALSE, "DIO count 1 (ticks)"="DIO count 1 (ticks)", "DIO count 2 (ticks)"="DIO count 2 (ticks)", "DIO count 3 (ticks)"="DIO count 3 (ticks)") -> ("FPGA VI Reference Out"=w28:T19, "error out"=w26:errorcluster)  [unwired: 1 in]
  n77 = local read "On one out of X cycles"() -> (w23:u32)
  n78 = local read "APD Integration Time (s)"() -> (w7:dbl)
  n79 = local read "DMA Update Period (s)"() -> (w6:dbl)
  n80 = Add(x=w17, y=w21) -> (x+y=w19:u32)
  n81 = Add(x=w15, y=w24) -> (x+y=w22:u32)
  n82 = local read "Green Laser ON/Interlacing"() -> (w99:bool)
  n83 = local read "Green laser mode"() -> (w100:enum32{"Laser ON", "Laser OFF", "Interlace"})
  n84 = Multiply(x=w19, y=w23) -> (x*y=w20:u32)
  n85 = Multiply(x=w23, y=w22) -> (x*y=w14:u32)
  n86 = Reciprocal(x=w7) -> (1/x=w4:dbl)
  n87 = Multiply(x=w7, y=40000000.0) -> (x*y=w3:dbl)
  n88 = Divide(x=w6, y=w7) -> (x/y=w9:dbl)
  n89 = Multiply(x="Current When FB OFF (%)", y=655.35) -> (x*y=w87:dbl)
  n90 = local read "Invert APD Gate"() -> (w13:bool)
  n91 = Multiply(x="Green FB Setpoint (mV)", y=3.2767) -> (x*y=w84:dbl)
  n92 = local read "APD Gate"() -> (w12:enum32{"ON", "OFF", "Interlace"})
  n93 = Subtract(x=w20, y=w17) -> (x-y=w18:u32)
  n94 = local write "Green FB Count"(w14) -> ()
  n95 = local write "APD Acq Rate (Hz)"(w4) -> ()
  n96 = To Unsigned Long Integer(number=w3) -> (unsigned 32bit integer=w1:u32)
  n97 = Multiply(x=2.0, y=w9) -> (x*y=w8:dbl)
  n98 = local read "Invert GI"() -> (w96:bool)
  n99 = To Unsigned Word Integer(number=w87) -> (unsigned 16bit integer=w85:u16)
  n100 = Subtract(x=w14, y=w15) -> (x-y=w16:u32)
  n101 = local write "APD Samples/FIFO Acq."(w9) -> ()
  n102 = To Word Integer(number=w84) -> (16bit integer=w82:i16)
  n103 = local write "APD Elements/DMA read"(w8) -> ()
  n104 = case shown="False" w99 {
    tunnel: w100 -> [_ w260]
    tunnel: [enum32{"Laser ON", "Laser OFF", "Interlace"}."Laser OFF" ("Green laser mode") w260] -> w95
    frame False {
    }
    frame True {
    }
  }
  n105 = local write "APD Int. Count"(w1) -> ()
  n106 = local read "Trap Pos. AI1 X Pre-scale"() -> (w39:u16)
  n107 = local read "Trap Pos FB Monitor\nT1 or T2"() -> (w46:bool)
  n108 = local read "Trap Pos FB Int Count"() -> (w32:u16)
  n109 = local read "APD 1 AO Mult."() -> (w11:i16)
  n110 = local read "Trap Pos FB Negate Action"() -> (w45:bool)
  n111 = local read "APD 2 AO Mult."() -> (w10:i16)
  n112 = local read "Trap Pos. FB Offset Factor"() -> (w44:i64)
  n113 = local read "Trap Pos. FB Mult Factor"() -> (w43:i64)
  n114 = local read "Trap Pos. FB Gains"() -> (w41:T11)
  n115 = local read "Trap Pos. FB Range"() -> (w42:T12)
  n116 = xnode "Read/Write Control"("FPGA VI Reference In"=w28, "error in"=w26, "Invert APD Gate"=w13, "APD Gate ON Count"=w17, "APD Gate OFF Count"=w18, "APD Acq Rate Count"=w1, "APD Gate Operating Mode"=w12, "APD 1 AO scale factor"=w11, "APD 2 AO scale factor"=w10, "Green interlace ON count"=w15, "Green interlace OFF count"=w16, "Green interlace ON count 2"=w15, "Green interlace OFF count 2"=w16, "Green FB Count"=w14) -> ("FPGA VI Reference Out"=w27:T19, "error out"=w25:errorcluster)
  n117 = xnode "Read/Write Control"("FPGA VI Reference In"=w27, "error in"=w25, "Invert GI 2"=w96, "Operating Mode 2"=w95, "Green FB Gains"="Green FB Gains", "Green FB Setpoint"=w82, "Green FB On/Off"="Green FB On/Off", "Current Out"=w85, "Green int current ON count adj"="Green int current ON count adj", "Operating Mode"=w95, "Invert GI"=w96, "Trap Pos FB Monitor T1 or T2"=w46, "Trap Pos FB Negate Action"=w45, "Trap Pos. FB Offset Factor"=w44, "Trap Pos. FB Mult Factor"=w43, "Trap Pos. FB Range"=w42, "Trap Pos. FB Gains"=w41, "Force feedback"=FALSE, "AI1 X Scale"=w39, "Trap Pos to FIFO"=TRUE, "Trap Pos FB Int Count"=w32) -> ("FPGA VI Reference Out"=w97:T19, "error out"=w98:errorcluster)
  n118 = xnode "Invoke Method"("FPGA VI Reference In"=w97, "error in"=w98, "Requested Depth"="Trap AI FIFO Depth") -> ("FPGA VI Reference Out"=w49:T19, "error out"=w48:errorcluster)  [unwired: 1 out]
  n119 = xnode "Invoke Method"("FPGA VI Reference In"=w49, "error in"=w48, "Requested Depth"="Trap Position FIFO Depth") -> ("FPGA VI Reference Out"=w34:T19, "error out"=w33:errorcluster)  [unwired: 1 out]
  n120 = flat-sequence {
    tunnel: w122 -> [w265]
    tunnel: [w265] -> w121
    tunnel: [w264] -> w120
    tunnel: [w263] -> w119
    tunnel: [w261] -> w117
    tunnel: [w262] -> w118
    frame #0 {
      w262 = T16 {"Minimum"=0.0, "Maximum"=40.0, "Increment"=1.0} ("Min Max Inc")
      w261 = T16 {"Minimum"=0.0, "Maximum"=50.0, "Increment"=1.0} ("Data Entry Limits")
      w264 = T16 {"Minimum"=60.0, "Maximum"=90.0, "Increment"=1.0} ("Min Max Inc")
      w263 = T16 {"Minimum"=0.0, "Maximum"=50.0, "Increment"=1.0} ("Data Entry Limits")
      n121 = property on="BD 2 Frequency 1 (MHz)" class="DigNum (strict)"("Data Range"=w262) -> ()  [unwired: 2 in, 2 out]
      n122 = property on="BD 2 Frequency 3 (MHz)" class="DigNum (strict)"("Data Range"=w262) -> ()  [unwired: 2 in, 2 out]
      n123 = property on="BD 2 Frequency 2 (MHz)" class="DigNum (strict)"("Data Range"=w262) -> ()  [unwired: 2 in, 2 out]
      n124 = property on="BD 1 Frequency 1 (MHz)" class="DigNum (strict)"("Data Range"=w264) -> ()  [unwired: 2 in, 2 out]
      n125 = property on="BD 1 Frequency 2 (MHz)" class="DigNum (strict)"("Data Range"=w264) -> ()  [unwired: 2 in, 2 out]
      n126 = property on="BD 1 Frequency 3 (MHz)" class="DigNum (strict)"("Data Range"=w264) -> ()  [unwired: 2 in, 2 out]
      n127 = property on="BD 2 Amplitude 1 (%)" class="DigNum (strict)"("Data Range"=w261) -> ()  [unwired: 2 in, 2 out]
      n128 = property on="BD 2 Amplitude 2 (%)" class="DigNum (strict)"("Data Range"=w261) -> ()  [unwired: 2 in, 2 out]
      n129 = property on="BD 2 Amplitude 3 (%)" class="DigNum (strict)"("Data Range"=w261) -> ()  [unwired: 2 in, 2 out]
      n130 = property on="BD 1 Amplitude 3 (%)" class="DigNum (strict)"("Data Range"=w263) -> ()  [unwired: 2 in, 2 out]
      n131 = property on="BD 1 Amplitude 2 (%)" class="DigNum (strict)"("Data Range"=w263) -> ()  [unwired: 2 in, 2 out]
      n132 = property on="BD 1 Amplitude 1 (%)" class="DigNum (strict)"("Data Range"=w263) -> ()  [unwired: 2 in, 2 out]
      "X RF Frequency Limits (MHz)" <- w264
      "X RF Amplitude Limits (%)" <- w263
      "Y RF Amplitude Limits (%)" <- w261
      "Y RF Frequency Limits (MHz)" <- w262
    }
  }
  n133 = xnode "Invoke Method"("FPGA VI Reference In"=w34, "error in"=w33) -> ("FPGA VI Reference Out"=w131:T19, "error out"=w130:errorcluster)  [unwired: 1 in]
  n134 = flat-sequence "Initial FPGA Loop Relative Phase Adjustment" {
    tunnel: "Initial Phase Adjustment (AI1)" -> [w276]
    tunnel: "Initial Phase Adjustment (GI)" -> [w275]
    tunnel: w131 -> [w274]
    tunnel: w130 -> [w273]
    tunnel: "Initial Phase Adj. (MCL)" -> [w272]
    tunnel: [w277] -> w140
    tunnel: [w271] -> w136
    tunnel: "Initial Phase Adjustment (APD Acq)" -> [w270]
    tunnel: "Initial Phase Adjustment (APD 1 Gate)" -> [w269]
    tunnel: "Initial Phase Adjustment (Green FB)" -> [w268]
    tunnel: "Initial Phase Adjustment (GI) 2" -> [w267]
    tunnel: "Initial Phase Adjustment (APD 2 Gate)" -> [w266]
    tunnel: w140 -> [w279]
    tunnel: [w280] -> w137
    tunnel: w136 -> [w280]
    tunnel: [w279] -> w135
    tunnel: w137 -> [w283]
    tunnel: w135 -> [w282]
    tunnel: [w285] -> w134
    tunnel: [w284] -> w133
    tunnel: [w287] -> w138
    tunnel: [w288] -> w139
    tunnel: w134 -> [w288]
    tunnel: w133 -> [w287]
    frame #0 {
      n135 = xnode "Read/Write Control"("FPGA VI Reference In"=w274, "error in"=w273, "Phase count adjustment"=w276, "Phase count adjustment (GI)"=w275, "Phase count adjustment (MCL)"=w272, "Phase Count Adjustment (APD Acq)"=w270, "Phase count adjustment (APD 1 Gate)"=w269, "Phase count adjustment (APD 2 Gate)"=w266, "Phase count adjustment (Green FB)"=w268, "Phase count adjustment (GI) 2"=w267) -> ("FPGA VI Reference Out"=w271:T19, "error out"=w277:errorcluster)
    }
    frame #1 {
      n136 = Wait (ms)(milliseconds to wait=u32 100) -> ()  [unwired: 1 out]
    }
    frame #2 {
      w281 = TRUE
      n137 = xnode "Read/Write Control"("FPGA VI Reference In"=w283, "error in"=w282, "+ phase"=w281, "+ phase (GI)"=w281, "+ phase (MCL)"=w281, "+ phase (APD Acq)"=w281, "+ phase (APD 1 Gate)"=w281, "+ phase (APD 2 Gate)"=w281, "+ phase (Green FB)"=w281, "+ phase (GI) 2"=w281) -> ("FPGA VI Reference Out"=w284:T19, "error out"=w285:errorcluster)
    }
    frame #3 {
      n138 = Wait (ms)(milliseconds to wait=u32 100) -> ()  [unwired: 1 out]
    }
  }
  n139 = local read "Phase adj. (Green FB)"() -> (w113:i16)
  n140 = local read "Phase adj. (GI) 2"() -> (w88:i16)
  n141 = local read "Phase adjust (MCL)"() -> (w170:i16)
  n142 = local read "Phase adj. (AI1)"() -> (w172:i16)
  n143 = local read "Phase adj. (GI)"() -> (w171:i16)
  n144 = xnode "Read/Write Control"("FPGA VI Reference In"=w138, "error in"=w139, "Phase count adjustment"=w172, "Phase count adjustment (GI)"=w171, "Phase count adjustment (MCL)"=w170, "Phase Count Adjustment (APD Acq)"="Phase Adj. (APD Acq)", "Phase count adjustment (APD 1 Gate)"="Phase Adj. (APD 1 Gate)", "Phase count adjustment (APD 2 Gate)"="Phase Adj. (APD 2 Gate)", "Phase count adjustment (Green FB)"=w113, "Phase count adjustment (GI) 2"=w88) -> ("FPGA VI Reference Out"=w74:T19, "error out"=w147:errorcluster)
  n145 = call "Initialize RF boards - interlace 3.vi"("error in"=w147, "FPGA VI Reference In"=w74) -> ("error out"=w145:errorcluster, "FPGA VI Reference Out"=w146:T19)
  n146 = call "set RF board frequency - interlace.vi"("Board 2 Frequency Limits"=w118, "Board 1 Frequency Limits"=w120, "error in"=w145, "FPGA VI Reference In"=w146, "Board 2 Frequency 3 (MHz)"="BD 2 Frequency 3 (MHz)", "Board 1 Frequency 3 (MHz)"="BD 1 Frequency 3 (MHz)", "Board 2 Frequency 2 (MHz)"="BD 2 Frequency 2 (MHz)", "Board 2 Frequency 1 (MHz)"="BD 2 Frequency 1 (MHz)", "Board 1 Frequency 2 (MHz)"="BD 1 Frequency 2 (MHz)", "Board 1 Frequency 1  (MHz)"="BD 1 Frequency 1 (MHz)") -> ("error out"=w249:errorcluster, "FPGA VI Reference Out"=w250:T19)
  n147 = call "set RF board amplitude - interlace.vi"("Board 2 Amplitude Limits"=w117, "Board 1 Amplitude Limits"=w119, "error in"=w249, "FPGA VI Reference In"=w250, "Board 2 Amplitude 3 (%)"="BD 2 Amplitude 3 (%)", "Board 1 Amplitude 3 (%)"="BD 1 Amplitude 3 (%)", "Board 2 Amplitude 2 (%)"="BD 2 Amplitude 2 (%)", "Board 2 Amplitude 1 (%)"="BD 2 Amplitude 1 (%)", "Board 1 Amplitude 2 (%)"="BD 1 Amplitude 2 (%)", "Board 1 Amplitude 1 (%)"="BD 1 Amplitude 1 (%)") -> ("error out"=w237:errorcluster, "FPGA VI Reference Out"=w238:T19)
  n148 = flat-sequence {
    tunnel: w238 -> [w297]
    tunnel: w237 -> [w296]
    tunnel: [w295] -> w242
    tunnel: [w294] -> w241
    tunnel: [w301] -> w240
    tunnel: w242 -> [w301]
    tunnel: [w300] -> w239
    tunnel: w241 -> [w300]
    tunnel: w240 -> [w310]
    tunnel: w239 -> [w309]
    tunnel: [w308] -> w36
    tunnel: [w307] -> w35
    frame #0 {
      n149 = local read "Trap 1 (ON/OFF)"() -> (w289:bool)
      n150 = xnode "Read/Write Control"("FPGA VI Reference In"=w297, "error in"=w296, "Direct RF Box  Communication"=FALSE) -> ("FPGA VI Reference Out"=w295:T19, "error out"=w294:errorcluster)
      n151 = local write "Saving..."(FALSE ("Saving Data")) -> ()
      n152 = local write "Stop All"(FALSE ("Stop All")) -> ()
      n153 = local write "Index"(1.0 ("Index")) -> ()
      n154 = property on="Trap 1 ON" class="Bool (strict)"("Value"=w289) -> ()  [unwired: 2 in, 2 out]
      "Manipulating Trap" <- FALSE ("Manipulating Trap")
    }
    frame #1 {
      n155 = local read "Trap 2 (ON/OFF)"() -> (w299:bool)
      n156 = Wait (ms)(milliseconds to wait=u32 10) -> ()  [unwired: 1 out]
      n157 = property on="Trap 2 ON" class="Bool (strict)"("Val(Sgnl)"=w299) -> ()  [unwired: 2 in, 2 out]
    }
    frame #2 {
      n158 = local read "Scan Range (nm)"() -> (w303:dbl)
      n159 = xnode "Read/Write Control"("FPGA VI Reference In"=w310, "error in"=w309, "FPGA Controls  RF Box"=TRUE ("Direct RF Box  Communication")) -> ("FPGA VI Reference Out"=w308:T19, "error out"=w307:errorcluster)
      n160 = call "Update messages.vi"("Message to add"="UHR-Fleezers ready.", "Old message string"="") -> ("New message string"=w306:string)
      n161 = local write "Messages"(w306) -> ()
      n162 = property on="Scan Range (nm)" class="DigNum (strict)"("Val(Sgnl)"=w303) -> ()  [unwired: 2 in, 2 out]
    }
  }
  n163 = Subtract(x="BD 1 Frequency 1 (MHz)", y="BD 1 Frequency 2 (MHz)") -> (x-y=w157:dbl)
  n164 = Subtract(x="BD 2 Frequency 1 (MHz)", y="BD 2 Frequency 2 (MHz)") -> (x-y=w156:dbl)
  n165 = Square(x=w156) -> (x^2=w154:dbl)
  n166 = Square(x=w157) -> (x^2=w155:dbl)
  n167 = Add(x=w155, y=w154) -> (x+y=w153:dbl)
  n168 = Square Root(x=w153) -> (sqrt(x)=w152:dbl)
  n169 = local write "Trap Delta (MHz)"(w152) -> ()
  n170 = call-poly "VISA Configure Serial Port"("VISA resource name"="Sample Chamber Stage Serial Port") -> ("VISA resource name out"=w69:refnum<visa-resource-name>, "error out"=w70:errorcluster)  [unwired: 5 in, 8 out]
  "Stage Control Serial Error" <- w70
  n171 = call "IMAQ Create"("Image Name"="APD 1 Image", "Image Type"=w60) -> ("New Image"=w59:T2)  [unwired: 3 in, 1 out]
  n172 = call "IMAQ Create"("Image Name"="APD 2 Image", "Image Type"=w60) -> ("New Image"=w58:T2)  [unwired: 3 in, 1 out]
  n173 = call "IMAQ Create"("Image Name"="Det. X Image", "Image Type"=w60) -> ("New Image"=w57:T2)  [unwired: 3 in, 1 out]
  n174 = call "IMAQ Create"("Image Name"="Det. Y Image", "Image Type"=w60) -> ("New Image"=w56:T2)  [unwired: 3 in, 1 out]
  n175 = call-poly "VISA Configure Serial Port"("VISA resource name"="Harvard Syringe Pump Serial Port", "baud rate (9600)"=u32 115200, "stop bits (10: 1 bit)"=w53) -> ("VISA resource name out"=w50:refnum<visa-resource-name>, "error out"=w51:errorcluster)  [unwired: 4 in, 7 out]
  n176 = Bundle("New Image"=w59, "New Image"=w58, "New Image"=w57, "New Image"=w56) -> (w55:T20)  [unwired: 1 in]
  n177 = node-c288(2 ("Processor")) -> (w78:T21)  [unwired: 3 out]
  n178 = node-c288() -> (w65:T21)  [unwired: 4 in]
  n179 = timed-loop "Control parameters (event loop)" {
    tunnel: w36 -> [w316]
    shift-right: [w315] -> _
    shift-left: errorcluster {"status"=FALSE, "code"=0, "source"=""} ("error out") -> [w314]
    tunnel: [w313] -> w215
    timing: w78 -> [_]
    timing-out: [_] -> w77
    tunnel: w50 -> [w312]
    stop <- w313 stop-if-true
    n180 = node-c288() -> ()  [unwired: 2 out]
    n181 = event shown="[47] \"Remove Action Offset\": Value Change" {
      selector: _ -> [_ _ _ _ _ _ _ _ _ _ _ _ _ _ _ _ _ _ _ _ _ _ _ _ _ _ _ _ _ _ _ _ _ _ _ _ _ _ _ _ _ _ _ _ _ _ _ _ _ _ _ _ _]
      dyn-events: _ -> [_ _ _ _ _ _ _ _ _ _ _ _ _ _ _ _ _ _ _ _ _ _ _ _ _ _ _ _ _ _ _ _ _ _ _ _ _ _ _ _ _ _ _ _ _ _ _ _ _ _ _ _ _]
      timeout: _ -> [_ _ _ _ _ _ _ _ _ _ _ _ _ _ _ _ _ _ _ _ _ _ _ _ _ _ _ _ _ _ _ _ _ _ _ _ _ _ _ _ _ _ _ _ _ _ _ _ _ _ _ _ _]
      tunnel: w316 -> [w354 _ _ _ w391 _ w413 _ _ _ _ w479 _ _ w522 w528 w533 w539 w575 w593 w600 w618 w629 w640 w651 w662 w673 w700 w794 w801 w839 _ w874 w878 w889 w893 w897 _ w905 _ _ _ _ w1031 _ w1048 w1051 w1059 w1068 w1071 w1076 _ w1092]
      tunnel: [w353 _ _ _ w381 _ w412 _ _ w444 _ w458 _ _ w521 w524 w530 w536 w574 w591 w599 w612 w623 w634 w645 w656 w667 w698 w792 w799 w837 _ w872 w876 w879 w891 w895 _ w903 _ _ _ _ w1029 _ _ _ _ _ _ _ _ _] -> w315
      tunnel: w314 -> [w352 _ _ _ w390 _ w411 _ _ w444 _ w478 _ _ w520 w523 w529 w535 w573 w592 w598 w617 w628 w639 w650 w661 w672 w699 w793 w800 w838 _ w873 w877 w888 w892 w896 _ w904 _ _ _ _ w1030 _ w1047 w1050 w1058 w1067 w1070 w1075 _ w1091]
      tunnel: [_ _ _ _ _ _ _ _ _ w443 _ _ _ _ _ _ _ _ _ _ _ _ _ _ _ _ _ _ _ _ _ _ _ _ _ _ _ _ _ _ _ _ _ _ _ _ _ _ _ _ _ _ _] -> w313
      tunnel: [_ _ _ _ _ _ _ "Round T1 X" _ _ _ _ _ _ _ _ _ _ _ _ _ _ _ _ _ _ _ _ _ _ _ _ _ _ _ _ _ _ _ _ _ _ _ _ _ _ _ _ _ _ _ _ _] -> _
      tunnel: [_ _ _ "Adjust Scale\nto Mean" _ _ _ _ _ _ _ _ _ _ _ _ _ _ _ _ _ _ _ _ _ _ _ _ _ _ _ _ _ _ _ _ _ _ _ _ _ _ _ _ _ _ _ _ _ _ _ _ _] -> _
      tunnel: [_ _ _ _ _ _ _ _ "Round T2 X" _ "Delayed Interlace Start" _ _ _ _ _ _ _ _ _ _ _ _ _ _ _ _ _ _ _ _ _ _ _ _ _ _ _ _ _ _ _ _ _ _ _ _ _ _ _ _ _ _] -> _
      tunnel: w312 -> [_ _ _ _ _ _ _ _ _ _ _ _ _ _ _ _ _ _ _ _ _ _ _ _ _ _ _ _ _ _ _ _ _ _ _ _ _ _ _ _ _ _ w1022 _ _ _ _ _ _ _ _ _ _]
      event "AI Count (ticks)", "Sets to FIFO (Traps)", "Save ave N", "FPGA Ave.", "# Samples/channel", "N sets to save": Value Change {
        # "So that if 'Save ave N' is updated, the AOD scanning code updates too."
        n182 = event-data() -> ()  [unwired: 6 out]
        n183 = local read "AI Count (ticks)"() -> (w334:u32)
        n184 = Boolean To (0,1)(Boolean="Sets to FIFO (Traps)") -> (0, 1=w344:cluster{"Set 1":i16, "Set 2":i16, "Set 3":i16})
        n185 = xnode "Read/Write Control"("FPGA VI Reference In"=w354, "error in"=w352, "ai count"=w334, "AI1 Sets to FIFO"="Sets to FIFO (Traps)", "N of AI1 Int Acq Sets"="N Acq Sets (Traps + Fl.)") -> ("error out"=w353:errorcluster)  [unwired: 1 out]
        n186 = Cluster To Array(cluster=w344) -> (array=w343:i16[])
        n187 = To Unsigned Long Integer(number=w343) -> (unsigned 32bit integer=w323:u32[])
        n188 = local read "Scan steps (AOD)"() -> (w345:u64)
        n189 = Multiply(x=w334, y="N Acq Sets (Traps + Fl.)") -> (x*y=w332:u32)
        n190 = Divide(x=40000000.0, y=w334) -> (x/y=w326:dbl)
        "AI rate (Hz)" <- w326
        "Ave. Rate (Hz)" <- w326
        n191 = Add Array Elements(numeric array=w323) -> (sum=w335:u32)
        "Trap Sets" <- w335
        n192 = Reciprocal(x=w326) -> (1/x=→"Ave. Period (s)":dbl)
        n193 = property on="Scan steps (AOD)" class="DigNum (strict)"("Val(Sgnl)"=w345) -> ()  [unwired: 2 in, 2 out]
        n194 = Divide(x=w326, y="N Acq Sets (Traps + Fl.)") -> (x/y=w349:dbl)
        "Data Rate (Hz)" <- w349
        n195 = Reciprocal(x=w349) -> (1/x=→"Data Period (s)":dbl)
        n196 = local read "Save ave N"() -> (w348:dbl)
        n197 = Divide(x=w349, y=w348) -> (x/y=w347:dbl)
        "Save Data Rate (Hz)" <- w347
        n198 = Reciprocal(x=w347) -> (1/x=→"Save Data Period (s)":dbl)
        n199 = Multiply(x=w332, y="# Samples/trap") -> (x*y=w330:u32)
        "Counts/DMA" <- w330
        n200 = property on="Trap Disp. Downsample" class="DigNum (strict)"("Maximum"="# Samples/trap") -> ()  [unwired: 2 in, 2 out]
        n201 = Multiply(x=w335, y="# Samples/trap") -> (x*y=w324:u32)
        "# Samples/channel" <- w324
        n202 = Multiply(x=w324, y=u32 8) -> (x*y=→"Trap AI Elements/DMA read":u32)
        n203 = local read "APD Int. Count"() -> (w331:u32)
        n204 = Multiply(x=w324, y=u32 3) -> (x*y=→"Trap Pos Elements/DMA read":u32)
        n205 = Divide(x=w330, y=w331) -> (x/y=w321:dbl)
        "APD Samples/FIFO Acq." <- w321
        n206 = Divide(x=w330, y=40000000.0) -> (x/y=w328:dbl)
        "DMA Update Period (s)" <- w328
        n207 = Multiply(x=2.0, y=w321) -> (x*y=→"APD Elements/DMA read":dbl)
        n208 = property on="APD Disp. Downsample" class="DigNum (strict)"("Maximum"=w321) -> ()  [unwired: 2 in, 2 out]
        n209 = local read "N sets to save"() -> (w341:u32)
        n210 = Multiply(x=w328, y=w341) -> (x*y=→"Total Time (s)":dbl)
        "FPGA Averaging" <- FALSE ("FPGA Averaging")
      }
      event "Rescale on Mean": Value Change {
        n211 = event-data() -> ()  [unwired: 7 out]
        n212 = And(x=FALSE, y="Rescale on Mean") -> (x .and. y?=w356:bool)
        n213 = local write "Rescale on Mean"(w356) -> ()
        n214 = local read "Bead Mean (nm)"() -> (w361:dbl)
        n215 = Add(x="Amplitude (nm)", y=w361) -> (x+y=w359:dbl)
        n216 = Subtract(x=w361, y="Amplitude (nm)") -> (x-y=w358:dbl)
        n217 = property on="Bead Separation" class="WFChart (strict)"("YScale.Minimum"=w358) -> ()  [unwired: 2 in, 2 out]
        n218 = property on="Bead Separation" class="WFChart (strict)"("YScale.Maximum"=w359) -> ()  [unwired: 2 in, 2 out]
      }
      event "Detector Type": Value Change {
        n219 = event-data() -> ()  [unwired: 7 out]
        n220 = local read "AI labels"() -> (w362:string[])
        n221 = property on="High Res. Display" class="Ring (strict)"("Strings []"=w362) -> ()  [unwired: 2 in, 2 out]
        n222 = Build Array (concatenate)(w362, "none") -> (w363:string[])
        n223 = property on="FFT 1 Choice 1" class="Ring (strict)"("Strings []"=w363) -> ()  [unwired: 2 in, 2 out]
        n224 = property on="FFT 1 Choice 2" class="Ring (strict)"("Strings []"=w363) -> ()  [unwired: 2 in, 2 out]
        n225 = property on="FFT 2 Choice 1" class="Ring (strict)"("Strings []"=w363) -> ()  [unwired: 2 in, 2 out]
        n226 = property on="FFT 2 Choice 2" class="Ring (strict)"("Strings []"=w363) -> ()  [unwired: 2 in, 2 out]
        n227 = Bundle("APD 1", "APD 2") -> (w366:cluster{string, string})  [unwired: 1 out]
        n228 = Cluster To Array(cluster=w366) -> (array=w364:string[])
        n229 = Build Array (concatenate)(w364, w363) -> (w368:string[])
        n230 = Array Size(array=w368) -> (size(s)=w369:i32)
        n231 = property on="Signals to Plot" class="LstBox (strict)"("Item Names"=w368) -> ()  [unwired: 2 in, 2 out]
        n232 = property on="Signals to Plot" class="LstBox (strict)"("Number of Rows"=w369) -> ()  [unwired: 2 in, 2 out]
        n233 = property on="All Signals" class="WFChart (strict)"("LegNumRows"=w369) -> ()  [unwired: 2 in, 2 out]
      }
      event "Adjust Scale\nto Mean": Value Change {
        n234 = event-data() -> ()  [unwired: 7 out]
        n235 = local read "APD 1 Rate (Hz)"() -> (w378:dbl)
        n236 = Multiply(x=1000.0, y="Above (kHz)") -> (x*y=w376:dbl)
        n237 = Multiply(x=1000.0, y="Below (kHz)") -> (x*y=w374:dbl)
        n238 = Add(x=w376, y=w378) -> (x+y=w371:dbl)
        n239 = Subtract(x=w378, y=w374) -> (x-y=w372:dbl)
        n240 = property on="APD Chart" class="WFChart (strict)"("YScale.Minimum"=w372) -> ()  [unwired: 2 in, 2 out]
        n241 = property on="APD Chart" class="WFChart (strict)"("YScale.Maximum"=w371) -> ()  [unwired: 2 in, 2 out]
      }
      event "Phase adj. (AI1)", "+ phase (AI1)", "- phase (AI1)": Value Change {
        n242 = event-data() -> ()  [unwired: 7 out]
        n243 = Negate(x="Phase adj. (AI1)") -> (-x=w388:i16)
        n244 = Select(t=w388, s="- phase (AI1)", f="Phase adj. (AI1)") -> (s? t:f=w387:i16)
        n245 = xnode "Read/Write Control"("FPGA VI Reference In"=w391, "error in"=w390, "Phase count adjustment"=w387) -> ("FPGA VI Reference Out"=w386:T19, "error out"=w385:errorcluster)
        n246 = Or(x="- phase (AI1)", y="+ phase (AI1)") -> (x .or. y?=w382:bool)
        n247 = xnode "Read/Write Control"("FPGA VI Reference In"=w386, "error in"=w385, "+ phase"=w382) -> ("error out"=w381:errorcluster)  [unwired: 1 out]
      }
      event "Signals to Plot": Double Click {
        w394 = u32 9868950 ("Color Box")
        n248 = event-data() -> ("Row"=w396:i32)  [unwired: 9 out]
        n249 = property on="All Signals" class="WFChart (strict)"("Active Plot"=w396) -> (error out=w407:errorcluster)  [unwired: 2 in, 1 out]
        n250 = property on="All Signals" class="WFChart (strict)" props=["Plot", "Visible?", "Plot", "Plot Color"](error in=w407) -> (error out=w406:errorcluster, "Plot.Visible?"=w405:bool)  [unwired: 1 in, 2 out]
        n251 = Select(t=FALSE ("Plot.Visible"), s=w405, f=TRUE ("Plot.Visible")) -> (s? t:f=w400:bool)
        n252 = property on="All Signals" class="WFChart (strict)"(error in=w406, "Plot.Visible?"=w400) -> (error out=w402:errorcluster)  [unwired: 1 in, 1 out]
        n253 = property on="All Signals" class="WFChart (strict)"(error in=w402) -> (error out=w397:errorcluster, "Plot.Plot Color"=w401:u32)  [unwired: 1 in, 1 out]
        n254 = property on="Signals to Plot" class="LstBox (strict)"(error in=w397, "Active Row"=w396) -> (error out=w395:errorcluster)  [unwired: 1 in, 1 out]
        n255 = Select(t=w401, s=w400, f=u32 0) -> (s? t:f=w398:u32)
        n256 = property on="Signals to Plot" class="LstBox (strict)"(error in=w395, "CellFontColor"=w398, "SelColor"=w394, "CellBG"=w394, "CellFontSize"=u32 20 ("Active Row:Cell Font:Size"), "CellFontBold"=TRUE ("Active Row:Cell Font:Bold")) -> ()  [unwired: 1 in, 2 out]
      }
      event "BD 1 Frequency 1 (MHz)", "BD 1 Frequency 2 (MHz)", "BD 1 Frequency 3 (MHz)", "BD 2 Frequency 1 (MHz)", "BD 2 Frequency 2 (MHz)", "BD 2 Frequency 3 (MHz)", "Trap Delta (MHz)": Value Change {
        n257 = event-data() -> ("CtlRef"=w410:refnum<vi>)  [unwired: 6 out]
        n258 = control-ref of="Trap Delta (MHz)"() -> (w409:refnum<vi>)
        n259 = Equal?(x=w409, y=w410) -> (x = y?=w408:bool)
        n260 = case shown="False" "Oscillate Set 1" {
          tunnel: w413 -> [w433 _]
          tunnel: [w432 w436] -> w412
          tunnel: w411 -> [w431 w436]
          tunnel: w408 -> [w416 _]
          frame False {
            n261 = local read "BD 1 Frequency 2 (MHz)"() -> (w420:dbl)
            n262 = local read "BD 1 Frequency 1 (MHz)"() -> (w418:dbl)
            n263 = Subtract(x=w420, y="Trap Delta (MHz)") -> (x-y=w417:dbl)
            n264 = Select(t=w417, s=w416, f=w418) -> (s? t:f=w415:dbl)
            n265 = local read "Y RF Frequency Limits (MHz)"() -> (w421:T16)
            n266 = local read "X RF Frequency Limits (MHz)"() -> (w422:T16)
            n267 = local read "BD 1 Frequency 3 (MHz)"() -> (w434:dbl)
            n268 = local write "BD 1 Frequency 1 (MHz)"(w415) -> ()
            n269 = local read "BD 2 Frequency 1 (MHz)"() -> (w425:dbl)
            n270 = local read "BD 2 Frequency 2 (MHz)"() -> (w424:dbl)
            n271 = local read "BD 2 Frequency 3 (MHz)"() -> (w435:dbl)
            n272 = call "set RF board frequency - interlace.vi"("Board 2 Frequency Limits"=w421, "Board 1 Frequency Limits"=w422, "error in"=w431, "FPGA VI Reference In"=w433, "Board 2 Frequency 3 (MHz)"=w435, "Board 1 Frequency 3 (MHz)"=w434, "Board 2 Frequency 2 (MHz)"=w424, "Board 2 Frequency 1 (MHz)"=w425, "Board 1 Frequency 2 (MHz)"=w420, "Board 1 Frequency 1  (MHz)"=w415) -> ("error out"=w432:errorcluster)  [unwired: 1 out]
            n273 = Subtract(x=w425, y=w424) -> (x-y=w429:dbl)
            n274 = Subtract(x=w415, y=w420) -> (x-y=w430:dbl)
            n275 = Square(x=w429) -> (x^2=w427:dbl)
            n276 = Square(x=w430) -> (x^2=w428:dbl)
            n277 = Add(x=w428, y=w427) -> (x+y=w426:dbl)
            n278 = Square Root(x=w426) -> (sqrt(x)=w423:dbl)
            n279 = local write "Trap Delta (MHz)"(w423) -> ()
            n280 = property on="Initial delta (MHz)" class="DigNum (strict)"("Val(Sgnl)"=w423) -> ()  [unwired: 2 in, 2 out]
          }
          frame True {
          }
        }
      }
      event "Round T1 X": Value Change {
        n281 = event-data() -> ()  [unwired: 7 out]
        n282 = local read "BD 1 Frequency 1 (MHz)"() -> (w439:dbl)
        n283 = Round To Nearest(number=w439) -> (nearest integer value=w438:dbl)
        n284 = property on="BD 1 Frequency 1 (MHz)" class="DigNum (strict)"("Val(Sgnl)"=w438) -> ()  [unwired: 2 in, 2 out]
      }
      event "Round T2 X": Value Change {
        n285 = event-data() -> ()  [unwired: 7 out]
        n286 = local read "BD 1 Frequency 2 (MHz)"() -> (w441:dbl)
        n287 = Round To Nearest(number=w441) -> (nearest integer value=w440:dbl)
        n288 = property on="BD 1 Frequency 2 (MHz)" class="DigNum (strict)"("Val(Sgnl)"=w440) -> ()  [unwired: 2 in, 2 out]
      }
      event "Stop All": Value Change {
        n289 = event-data() -> ()  [unwired: 7 out]
        n290 = local read "Stop All"() -> (w443:bool)
      }
      event "Delayed Interlace Start": Value Change {
        n291 = event-data() -> ()  [unwired: 7 out]
        n292 = flat-sequence {
          frame #0 {
            n293 = Multiply(x="Delay to Interlace (s)", y=1000.0) -> (x*y=w446:dbl)
            n294 = Wait (ms)(milliseconds to wait=w446) -> ()  [unwired: 1 out]
          }
          frame #1 {
            n295 = property on="Green laser mode" class="RadioBtnsControl (strict)"("Val(Sgnl)"=enum32{"Laser ON", "Laser OFF", "Interlace"}."Interlace" ("Value (Signaling)")) -> ()  [unwired: 2 in, 2 out]
          }
        }
      }
      event "BD 1 Amplitude 1 (%)", "BD 1 Amplitude 2 (%)", "BD 1 Amplitude 3 (%)", "BD 2 Amplitude 1 (%)", "BD 2 Amplitude 2 (%)", "BD 2 Amplitude 3 (%)", "Trap 1 ON", "Trap 2 ON", "Trap 3 ON", "Feedback On/Off", "All FB On/Off": Value Change {
        w470 = i16 1 ("f")
        n296 = event-data() -> ()  [unwired: 7 out]
        n297 = local write "Trap 1 (ON/OFF)"("Trap 1 ON") -> ()
        n298 = local write "Trap 2 (ON/OFF)"("Trap 2 ON") -> ()
        n299 = Boolean To (0,1)(Boolean="Trap 3 ON") -> (0, 1=w471:i16)
        n300 = Boolean To (0,1)(Boolean="Trap 1 ON") -> (0, 1=w472:i16)
        n301 = Boolean To (0,1)(Boolean="Trap 2 ON") -> (0, 1=w473:i16)
        n302 = Select(t=w473, s="Trap ON/OFF X or Y Amp?", f=w470) -> (s? t:f=w468:i16)
        n303 = Select(t=w472, s="Trap ON/OFF X or Y Amp?", f=w470) -> (s? t:f=w469:i16)
        n304 = Select(t=w471, s="Trap ON/OFF X or Y Amp?", f=w470) -> (s? t:f=w467:i16)
        n305 = Select(t=w470, s="Trap ON/OFF X or Y Amp?", f=w473) -> (s? t:f=w465:i16)
        n306 = Select(t=w470, s="Trap ON/OFF X or Y Amp?", f=w472) -> (s? t:f=w466:i16)
        n307 = Select(t=w470, s="Trap ON/OFF X or Y Amp?", f=w471) -> (s? t:f=w464:i16)
        n308 = And(x="All FB On/Off", y="Feedback On/Off") -> (x .and. y?=w462:cluster{"Set 1":bool, "Set 2":bool})
        n309 = local read "BD 1 Amplitude 1 (%)"() -> (w482:dbl)
        n310 = local read "BD 1 Amplitude 2 (%)"() -> (w481:dbl)
        n311 = local read "BD 1 Amplitude 3 (%)"() -> (w480:dbl)
        n312 = Unbundle By Name(w462) -> ("Set 1"=w457:bool, "Set 2"=w454:bool)
        n313 = local read "Y RF Amplitude Limits (%)"() -> (w450:T16)
        n314 = local read "X RF Amplitude Limits (%)"() -> (w451:T16)
        n315 = local read "BD 2 Amplitude 1 (%)"() -> (w483:dbl)
        n316 = local read "BD 2 Amplitude 2 (%)"() -> (w484:dbl)
        n317 = local read "BD 2 Amplitude 3 (%)"() -> (w485:dbl)
        n318 = And(x="Trap 2 ON", y=w454) -> (x .and. y?=w452:bool)
        n319 = And(x="Trap 1 ON", y=w457) -> (x .and. y?=w455:bool)
        n320 = Multiply(x=w469, y=w482) -> (x*y=w477:dbl)
        n321 = Multiply(x=w481, y=w468) -> (x*y=w475:dbl)
        n322 = Multiply(x=w480, y=w467) -> (x*y=w476:dbl)
        n323 = Multiply(x=w483, y=w466) -> (x*y=w486:dbl)
        n324 = Multiply(x=w484, y=w465) -> (x*y=w487:dbl)
        n325 = Multiply(x=w485, y=w464) -> (x*y=w488:dbl)
        n326 = call "set RF board amplitude - interlace.vi"("Board 2 Amplitude Limits"=w450, "Board 1 Amplitude Limits"=w451, "error in"=w478, "FPGA VI Reference In"=w479, "Board 2 Amplitude 3 (%)"=w488, "Board 1 Amplitude 3 (%)"=w476, "Board 2 Amplitude 2 (%)"=w487, "Board 2 Amplitude 1 (%)"=w486, "Board 1 Amplitude 2 (%)"=w475, "Board 1 Amplitude 1 (%)"=w477) -> ("error out"=w459:errorcluster, "FPGA VI Reference Out"=w460:T19)
        n327 = xnode "Read/Write Control"("FPGA VI Reference In"=w460, "error in"=w459, "FB On/Off Set 1"=w455, "FB On/Off Set 2"=w452) -> ("error out"=w458:errorcluster)  [unwired: 1 out]
      }
      event "Load parameters": Value Change {
        n328 = event-data() -> ()  [unwired: 7 out]
        n329 = property on="Saved AOD Raster Scan Parameter Sets" class="Arr (strict)"() -> ("Index Values"=w499:u32[])  [unwired: 2 in, 2 out]
        n330 = Index Array(array=w499, index=0) -> (element=w496:u32)
        n331 = local write "Load parameters"(FALSE ("Load parameters")) -> ()
        n332 = Index Array(array="Saved AOD Raster Scan Parameter Sets", index=w496) -> (element=w495:T26)
        n333 = Unbundle By Name(w495) -> ("Scan Range AOD (nm) 2"=w494:dbl, "Step Size AOD (nm) 2"=w493:dbl, "Scan Speed AOD (nm/s) 2"=w492:dbl, "Number of scans (AOD) 2"=w491:u16)
        n334 = flat-sequence {
          tunnel: w494 -> [w502]
          tunnel: w493 -> [w501]
          tunnel: w492 -> [w500]
          tunnel: w491 -> [w503]
          frame #0 {
            n335 = local write "Scan Speed (nm/s)"(w500) -> ()
            n336 = local write "Scan Range (nm)"(w502) -> ()
            n337 = local write "Step Size (nm)"(w501) -> ()
          }
          frame #1 {
            n338 = property on="Number of F/B Scans (AOD)" class="DigNum (strict)"("Val(Sgnl)"=w503) -> ()  [unwired: 2 in, 2 out]
          }
        }
      }
      event "Trap 1 (ON/OFF)", "Trap 2 (ON/OFF)": Value Change {
        n339 = event-data() -> ()  [unwired: 7 out]
        n340 = property on="Trap 2 ON" class="Bool (strict)"("Val(Sgnl)"="Trap 2 (ON/OFF)") -> ()  [unwired: 2 in, 2 out]
        n341 = property on="Trap 1 ON" class="Bool (strict)"("Val(Sgnl)"="Trap 1 (ON/OFF)") -> ()  [unwired: 2 in, 2 out]
      }
      event "DIO count 1 (ticks)", "DIO count 2 (ticks)", "DIO count 3 (ticks)", "Interlace", "Number Interlace Sets", "Not-Interlacing Set": Value Change {
        n342 = event-data() -> ()  [unwired: 7 out]
        n343 = local read "DIO count 3 (ticks)"() -> (w516:u32)
        n344 = local read "DIO count 1 (ticks)"() -> (w518:u32)
        n345 = local read "DIO count 2 (ticks)"() -> (w517:u32)
        n346 = To Unsigned Byte Integer(number="Not-Interlacing Set") -> (unsigned 8bit integer=w507:u8)
        n347 = Add(x=w507, y=u8 1) -> (x+y=w511:u8)
        n348 = xnode "Read/Write Control"("FPGA VI Reference In"=w522, "error in"=w520, "DIO count 1 (ticks)"=w518, "DIO count 2 (ticks)"=w517, "DIO count 3 (ticks)"=w516, "Interlace ON/OFF"="Interlace", "Number Interlace Cycles"="Number Interlace Sets", "Interlace Off Parameters"=w511) -> ("error out"=w521:errorcluster)  [unwired: 1 out]
        n349 = Build Array(w518, w517, w516) -> (w509:u32[])
        n350 = Split 1D Array(array=w509, index="Number Interlace Sets") -> (first subarray=w519:u32[])  [unwired: 1 out]
        n351 = Index Array(array=w509, index=w507) -> (element=w508:u32)
        n352 = Add Array Elements(numeric array=w519) -> (sum=w513:u32)
        n353 = Select(t=w513, s="Interlace", f=w508) -> (s? t:f=→"Total Counts (ticks)":u32)
      }
      event "Reset Feedback": Value Change {
        n354 = event-data() -> ()  [unwired: 7 out]
        n355 = Unbundle By Name("Reset Feedback") -> ("Set 1"=w526:bool, "Set 2"=w525:bool)
        n356 = xnode "Read/Write Control"("FPGA VI Reference In"=w528, "error in"=w523, "FB Reset Set 1"=w526, "FB Reset Set 2"=w525) -> ("error out"=w524:errorcluster)  [unwired: 1 out]
      }
      event "PID Gains": Value Change {
        n357 = event-data() -> ()  [unwired: 7 out]
        n358 = Unbundle By Name("PID Gains") -> ("Set 1"=w532:T14, "Set 2"=w531:T14)
        n359 = xnode "Read/Write Control"("FPGA VI Reference In"=w533, "error in"=w529, "FB Gains Set 1"=w532, "FB Gains Set 2"=w531) -> ("error out"=w530:errorcluster)  [unwired: 1 out]
      }
      event "AI2 to Setpoint", "Setpoints (V)": Value Change {
        n360 = event-data() -> ()  [unwired: 7 out]
        n361 = xnode "Read/Write Control"("FPGA VI Reference In"=w539, "error in"=w535) -> ("FPGA VI Reference Out"=w538:T19, "error out"=w537:errorcluster, "AI2 Y Sum Set 1"=w546:i16, "AI2 Y Sum Set 2"=w545:i16)
        n362 = Cluster To Array(cluster="AI2 to Setpoint") -> (array=w549:bool[])
        n363 = local read "AI2 (V)"() -> (w547:cluster{"Set 1":dbl, "Set 2":dbl})
        n364 = Or Array Elements(Boolean array=w549) -> (logical OR=w550:bool)
        n365 = Bundle By Name(cluster=w547, "Set 1"=w546, "Set 2"=w545) -> (w544:cluster{"Set 1":dbl, "Set 2":dbl})
        n366 = Divide(x=w544, y=3276.7) -> (x/y=w543:cluster{"Set 1":dbl, "Set 2":dbl})
        "AI2 (V)" <- w543
        n367 = case shown="True" w550 {
          tunnel: [w553 w570] -> w542
          tunnel: "AI2 to Setpoint" -> [_ w566]
          tunnel: "Setpoints (V)" -> [w554 w569]
          tunnel: w543 -> [_ w563]
          frame False {
            n368 = Multiply(x=3276.7, y=w554) -> (x*y=w555:cluster{"Set 1":dbl, "Set 2":dbl})
            n369 = To Word Integer(number=w555) -> (16bit integer=w553:cluster{"Set 1":i16, "Set 2":i16})
          }
          frame True {
            n370 = Unbundle By Name(w563) -> ("Set 1"=w562:dbl, "Set 2"=w561:dbl)
            n371 = Unbundle By Name(w569) -> ("Set 1"=w568:dbl, "Set 2"=w567:dbl)
            n372 = Unbundle By Name(w566) -> ("Set 1"=w565:bool, "Set 2"=w564:bool)
            n373 = Select(t=w562, s=w565, f=w568) -> (s? t:f=w560:dbl)
            n374 = Select(t=w561, s=w564, f=w567) -> (s? t:f=w559:dbl)
            n375 = Bundle By Name(cluster=w569, "Set 1"=w560, "Set 2"=w559) -> (w557:cluster{"Set 1":dbl, "Set 2":dbl})
            n376 = local write "Setpoints (V)"(w557) -> ()
            n377 = Multiply(x=3276.7, y=w557) -> (x*y=w558:cluster{"Set 1":dbl, "Set 2":dbl})
            n378 = To Word Integer(number=w558) -> (16bit integer=w570:cluster{"Set 1":i16, "Set 2":i16})
          }
        }
        n379 = Unbundle By Name(w542) -> ("Set 1"=w541:i16, "Set 2"=w540:i16)
        n380 = xnode "Read/Write Control"("FPGA VI Reference In"=w538, "error in"=w537, "FB Setpoint Set 1"=w541, "FB Setpoint Set 2"=w540) -> ("error out"=w536:errorcluster)  [unwired: 1 out]
      }
      event "Invert GI": Value Change {
        n381 = event-data() -> ()  [unwired: 7 out]
        n382 = xnode "Read/Write Control"("FPGA VI Reference In"=w575, "error in"=w573, "Invert GI"="Invert GI", "Invert GI 2"="Invert GI") -> ("error out"=w574:errorcluster)  [unwired: 1 out]
      }
      event "Green FB Setpoint (mV)", "Green FB Gains", "Green FB On/Off", "Current When FB OFF (%)", "Green int current ON count adj": Value Change {
        n383 = event-data() -> ()  [unwired: 7 out]
        n384 = local read "Green FB Setpoint (mV)"() -> (w582:dbl)
        n385 = local read "Current When FB OFF (%)"() -> (w585:dbl)
        n386 = Multiply(x=w582, y=3.2767) -> (x*y=w581:dbl)
        n387 = Multiply(x=w585, y=655.35) -> (x*y=w586:dbl)
        n388 = To Unsigned Word Integer(number=w586) -> (unsigned 16bit integer=w584:u16)
        n389 = local read "Green int current ON count adj"() -> (w589:u32)
        n390 = local read "Green FB Gains"() -> (w588:T14)
        n391 = local read "Green Laser ON/Interlacing"() -> (w579:bool)
        n392 = local read "Green laser mode"() -> (w578:enum32{"Laser ON", "Laser OFF", "Interlace"})
        n393 = local read "Green FB On/Off"() -> (w590:bool)
        n394 = Equal?(x=w578, y=enum32{"Laser ON", "Laser OFF", "Interlace"}."Interlace") -> (x = y?=w576:bool)
        n395 = Compound Arithmetic op=AND(w576, w590, w579) -> (w580:bool)
        n396 = xnode "Read/Write Control"("FPGA VI Reference In"=w593, "error in"=w592, "Green FB Setpoint"=w581, "Green FB On/Off"=w580, "Current Out"=w584, "Green int current ON count adj"=w589, "Green FB Gains"=w588) -> ("error out"=w591:errorcluster)  [unwired: 1 out]
      }
      event "Green laser mode", "Green Laser ON/Interlacing": Value Change {
        n397 = event-data() -> ()  [unwired: 7 out]
        n398 = case shown="True" "Green Laser ON/Interlacing" {
          tunnel: "Green laser mode" -> [_ w607]
          tunnel: [enum32{"Laser ON", "Laser OFF", "Interlace"}."Laser OFF" ("Green laser mode") w607] -> w595
          tunnel: [FALSE w603] -> w594
          frame False {
          }
          frame True {
            n399 = local read "Green FB On/Off"() -> (w604:bool)
            n400 = Equal?(x=w607, y=enum32{"Laser ON", "Laser OFF", "Interlace"}."Interlace") -> (x = y?=w605:bool)
            n401 = And(x=w605, y=w604) -> (x .and. y?=w603:bool)
          }
        }
        n402 = xnode "Read/Write Control"("FPGA VI Reference In"=w600, "error in"=w598, "Operating Mode"=w595, "Operating Mode 2"=w595, "Green FB On/Off"=w594) -> ("error out"=w599:errorcluster)  [unwired: 1 out]
      }
      event "- phase (APD 1 Gate)", "+ phase (APD 1 Gate)": Value Change {
        n403 = event-data() -> ()  [unwired: 7 out]
        n404 = local read "Phase Adj. (APD 1 Gate)"() -> (w608:i16)
        n405 = Negate(x=w608) -> (-x=w616:i16)
        n406 = Select(t=w616, s="- phase (APD 1 Gate)", f=w608) -> (s? t:f=w615:i16)
        n407 = Or(x="- phase (APD 1 Gate)", y="+ phase (APD 1 Gate)") -> (x .or. y?=w611:bool)
        n408 = xnode "Read/Write Control"("FPGA VI Reference In"=w618, "error in"=w617, "Phase count adjustment (APD 1 Gate)"=w615) -> ("FPGA VI Reference Out"=w613:T19, "error out"=w614:errorcluster)
        n409 = xnode "Read/Write Control"("FPGA VI Reference In"=w613, "error in"=w614, "+ phase (APD 1 Gate)"=w611) -> ("error out"=w612:errorcluster)  [unwired: 1 out]
      }
      event "+ phase (APD 2 Gate)", "- phase (APD 2 Gate)": Value Change {
        n410 = event-data() -> ()  [unwired: 7 out]
        n411 = local read "Phase Adj. (APD 2 Gate)"() -> (w619:i16)
        n412 = Negate(x=w619) -> (-x=w627:i16)
        n413 = Select(t=w627, s="- phase (APD 2 Gate)", f=w619) -> (s? t:f=w626:i16)
        n414 = Or(x="- phase (APD 2 Gate)", y="+ phase (APD 2 Gate)") -> (x .or. y?=w622:bool)
        n415 = xnode "Read/Write Control"("FPGA VI Reference In"=w629, "error in"=w628, "Phase count adjustment (APD 2 Gate)"=w626) -> ("FPGA VI Reference Out"=w624:T19, "error out"=w625:errorcluster)
        n416 = xnode "Read/Write Control"("FPGA VI Reference In"=w624, "error in"=w625, "+ phase (APD 2 Gate)"=w622) -> ("error out"=w623:errorcluster)  [unwired: 1 out]
      }
      event "Phase Adj. (APD Acq)", "+ phase (APD Acq)", "- phase (APD Acq)": Value Change {
        n417 = event-data() -> ()  [unwired: 7 out]
        n418 = local read "Phase Adj. (APD Acq)"() -> (w632:i16)
        n419 = Negate(x=w632) -> (-x=w638:i16)
        n420 = Select(t=w638, s="+ phase (APD Acq)", f=w632) -> (s? t:f=w637:i16)
        n421 = Or(x="+ phase (APD Acq)", y="- phase (APD Acq)") -> (x .or. y?=w633:bool)
        n422 = xnode "Read/Write Control"("FPGA VI Reference In"=w640, "error in"=w639, "Phase Count Adjustment (APD Acq)"=w637) -> ("FPGA VI Reference Out"=w635:T19, "error out"=w636:errorcluster)
        n423 = xnode "Read/Write Control"("FPGA VI Reference In"=w635, "error in"=w636, "+ phase (APD Acq)"=w633) -> ("error out"=w634:errorcluster)  [unwired: 1 out]
      }
      event "Phase adj. (GI)", "+ phase (GI)", "- phase (GI)": Value Change {
        n424 = event-data() -> ()  [unwired: 7 out]
        n425 = Negate(x="Phase adj. (GI)") -> (-x=w649:i16)
        n426 = Select(t=w649, s="+ phase (GI)", f="Phase adj. (GI)") -> (s? t:f=w648:i16)
        n427 = Or(x="+ phase (GI)", y="- phase (GI)") -> (x .or. y?=w644:bool)
        n428 = xnode "Read/Write Control"("FPGA VI Reference In"=w651, "error in"=w650, "Phase count adjustment (GI)"=w648) -> ("FPGA VI Reference Out"=w646:T19, "error out"=w647:errorcluster)
        n429 = xnode "Read/Write Control"("FPGA VI Reference In"=w646, "error in"=w647, "+ phase (GI)"=w644) -> ("error out"=w645:errorcluster)  [unwired: 1 out]
      }
      event "Phase adj. (GI) 2", "+ phase (GI) 2", "- phase (GI) 2": Value Change {
        n430 = event-data() -> ()  [unwired: 7 out]
        n431 = Negate(x="Phase adj. (GI) 2") -> (-x=w660:i16)
        n432 = Select(t=w660, s="+ phase (GI) 2", f="Phase adj. (GI) 2") -> (s? t:f=w659:i16)
        n433 = Or(x="+ phase (GI) 2", y="- phase (GI) 2") -> (x .or. y?=w655:bool)
        n434 = xnode "Read/Write Control"("FPGA VI Reference In"=w662, "error in"=w661, "Phase count adjustment (GI) 2"=w659) -> ("FPGA VI Reference Out"=w657:T19, "error out"=w658:errorcluster)
        n435 = xnode "Read/Write Control"("FPGA VI Reference In"=w657, "error in"=w658, "+ phase (GI) 2"=w655) -> ("error out"=w656:errorcluster)  [unwired: 1 out]
      }
      event "Phase adj. (Green FB)", "- phase (Green FB)", "+ phase (Green FB)": Value Change {
        n436 = event-data() -> ()  [unwired: 7 out]
        n437 = Negate(x="Phase adj. (Green FB)") -> (-x=w671:i16)
        n438 = Select(t=w671, s="+ phase (Green FB)", f="Phase adj. (Green FB)") -> (s? t:f=w670:i16)
        n439 = Or(x="+ phase (Green FB)", y="- phase (Green FB)") -> (x .or. y?=w666:bool)
        n440 = xnode "Read/Write Control"("FPGA VI Reference In"=w673, "error in"=w672, "Phase count adjustment (Green FB)"=w670) -> ("FPGA VI Reference Out"=w668:T19, "error out"=w669:errorcluster)
        n441 = xnode "Read/Write Control"("FPGA VI Reference In"=w668, "error in"=w669, "+ phase (Green FB)"=w666) -> ("error out"=w667:errorcluster)  [unwired: 1 out]
      }
      event "Invert APD Gate", "APD Gate ON Count", "APD Gate OFF Count", "APD Gate", "APD Integration Time (s)", "APD 1 AO Mult.", "APD 2 AO Mult.", "On one out of X cycles": Value Change {
        n442 = event-data() -> ()  [unwired: 7 out]
        n443 = Add(x="GI Frequency, ON count", y="GI Frequency, OFF count") -> (x+y=w677:u32)
        n444 = Add(x="APD Gate ON Count", y="APD Gate OFF Count") -> (x+y=w690:u32)
        n445 = Multiply(x="On one out of X cycles", y=w677) -> (x*y=w674:u32)
        "Green FB Count" <- w674
        n446 = Subtract(x=w674, y="GI Frequency, ON count") -> (x-y=w675:u32)
        n447 = Multiply(x=w690, y="On one out of X cycles") -> (x*y=w689:u32)
        n448 = Subtract(x=w689, y="APD Gate ON Count") -> (x-y=w688:u32)
        n449 = local read "DMA Update Period (s)"() -> (w691:dbl)
        n450 = Multiply(x="APD Integration Time (s)", y=40000000.0) -> (x*y=w696:dbl)
        n451 = Reciprocal(x="APD Integration Time (s)") -> (1/x=→"APD Acq Rate (Hz)":dbl)
        n452 = To Unsigned Long Integer(number=w696) -> (unsigned 32bit integer=w680:u32)
        "APD Int. Count" <- w680
        n453 = xnode "Read/Write Control"("FPGA VI Reference In"=w700, "error in"=w699, "Invert APD Gate"="Invert APD Gate", "APD Gate ON Count"="APD Gate ON Count", "APD Gate OFF Count"=w688, "APD Acq Rate Count"=w680, "APD Gate Operating Mode"="APD Gate", "APD 1 AO scale factor"="APD 1 AO Mult.", "APD 2 AO scale factor"="APD 2 AO Mult.", "Green interlace ON count"="GI Frequency, ON count", "Green interlace OFF count"=w675, "Green interlace ON count 2"="GI Frequency, ON count", "Green interlace OFF count 2"=w675, "Green FB Count"=w674) -> ("error out"=w698:errorcluster)  [unwired: 1 out]
        n454 = Divide(x=w691, y="APD Integration Time (s)") -> (x/y=w694:dbl)
        n455 = Multiply(x=2.0, y=w694) -> (x*y=w693:dbl)
        n456 = local write "APD Samples/FIFO Acq."(w694) -> ()
        n457 = local write "APD Elements/DMA read"(w693) -> ()
      }
      event "Number of F/B Scans (AOD)", "Scan Speed (nm/s)", "Scan BD", "Initial delta (MHz)", "Step Size (nm)", "Scan Range (nm)": Value Change {
        w762 = 123.0  # AOM cal (nm/MHz)
        n458 = event-data() -> ()  [unwired: 7 out]
        n459 = local read "BD 1 Frequency 1 (MHz)"() -> (w745:dbl)
        n460 = local read "AOM X Cal (nm/MHz)"() -> (w737:dbl)
        n461 = local read "X RF Frequency Limits (MHz)"() -> (w749:T16)
        n462 = local read "Y RF Frequency Limits (MHz)"() -> (w746:T16)
        n463 = local read "BD 2 Frequency 1 (MHz)"() -> (w751:dbl)
        n464 = Negate(x="Scan Range (nm)") -> (-x=w715:dbl)
        n465 = Divide(x=w715, y=w737) -> (x/y=w719:dbl)
        n466 = Select(t=w749, s="Scan BD", f=w746) -> (s? t:f=w748:T16)
        n467 = Select(t=w745, s="Scan BD", f=w751) -> (s? t:f=w750:dbl)
        n468 = Unbundle By Name(w748) -> ("Maximum"=w757:dbl, "Minimum"=w756:dbl)
        n469 = Add(x=w719, y=w750) -> (x+y=w754:dbl)
        n470 = Divide(x=w715, y="Step Size (nm)") -> (x/y=w734:dbl)
        n471 = Divide(x="Step Size (nm)", y=w737) -> (x/y=w743:dbl)
        n472 = Absolute Value(x=w734) -> (abs(x)=w718:dbl)
        n473 = Sign(1:w715) -> (0:w716:dbl)
        n474 = In Range and Coerce(upper limit=w757, x=w754, lower limit=w756) -> (coerced(x)=w753:dbl, In Range?=w755:bool)
        n475 = To Unsigned Quad Integer(1:w718) -> (0:w733:u64)
        "Scan steps (AOD)" <- w733
        n476 = call "IR AOM freq to word.vi"("Frequency In (MHz)"=w743) -> ("Frequency Word Out (double)"=w740:dbl)
        n477 = Multiply(x=w716, y=w740) -> (x*y=w717:dbl)
        n478 = Subtract(x=w754, y=w753) -> (x-y=w752:dbl)
        n479 = To Quad Integer(1:w717) -> (0:w739:i64)
        "Incr. int (AOD)" <- w739
        n480 = Subtract(x=w719, y=w752) -> (x-y=w738:dbl)
        "Scan Range (MHz)" <- w738
        n481 = Select(t=w719, s=w755, f=w738) -> (s? t:f=w758:dbl)
        n482 = Multiply(x=w738, y=w737) -> (x*y=w736:dbl)
        n483 = Decrement(x=w733) -> (x-1=w786:u64)
        n484 = Negate(x=w736) -> (-x=w732:dbl)
        n485 = local write "Scan Range (nm)"(w732) -> ()
        n486 = Divide(x=w758, y=w786) -> (x/y=w742:dbl)
        "Scan Increment (MHz)" <- w742
        n487 = call "IR AOM freq to word.vi"("Frequency In (MHz)"=w742) -> ("Frequency Word Out (double)"=w741:dbl)
        n488 = Divide(x="Step Size (nm)", y="Scan Speed (nm/s)") -> (x/y=w729:dbl)
        n489 = To Quad Integer(1:w741) -> ()  [unwired: 1 out]
        n490 = local read "Number Interlace Sets"() -> (w713:u8)
        n491 = local read "AI Count (ticks)"() -> (w714:u32)
        n492 = local read "Total Counts (ticks)"() -> (w712:u32)
        n493 = local read "# Samples/trap"() -> (w744:u32)
        n494 = Multiply(x=w714, y=w713) -> (x*y=w711:u32)
        n495 = Divide(x=w712, y=w711) -> (x/y=w710:dbl)
        n496 = Select(t=w745, s="Scan BD", f=w751) -> (s? t:f=w783:dbl)
        "Initial freq. (MHz)" <- w783
        n497 = Add(x=w758, y=w783) -> (x+y=→"Final freq. (MHz)":dbl)
        n498 = Divide(x=w712, y=40000000.0) -> (x/y=w728:dbl)
        n499 = Divide(x=w729, y=w728) -> (x/y=w727:dbl)
        n500 = To Unsigned Quad Integer(1:w727) -> (0:w702:u64)
        n501 = Quotient & Remainder(x=w702, y=u64 2) -> (x-y*floor(x/y)=w706:u64)  [unwired: 1 out]
        n502 = Equal?(x=w706, y=u64 0) -> (x = y?=w704:bool)
        n503 = Decrement(x=w702) -> (x-1=w703:u64)
        n504 = Select(t=w702, s=w704, f=w703) -> (s? t:f=w701:u64)
        "Cycles/step (AOD)" <- w701
        n505 = xnode "Read/Write Control"("FPGA VI Reference In"=w794, "error in"=w793, "Scan steps"=w733, "Number of scans"="Number of F/B Scans (AOD)", "Cycles per step"=w701, "Scan freq.  increment"=w739, "Scan BD"="Scan BD") -> ("error out"=w792:errorcluster)  [unwired: 1 out]
        n506 = Multiply(x=w733, y=w701) -> (x*y=w787:u64)
        n507 = Multiply(x=w787, y=u64 2) -> (x*y=w709:u64)
        n508 = Multiply(x=w710, y=w709) -> (x*y=w708:dbl)
        "Data points/scan (f/b)" <- w708
        n509 = Multiply(x=w708, y="Number of F/B Scans (AOD)") -> (x*y=w790:dbl)
        "Data points/scans" <- w790
        n510 = Divide(x=w790, y=w744) -> (x/y=→"N sets should be saved":dbl)
        n511 = Multiply(x=w787, y=w728) -> (x*y=w726:dbl)
        "Time/Scan (s) (AOD)" <- w726
        n512 = Select(t=w758, s="Scan BD", f=0.0) -> (s? t:f=w784:dbl)
        n513 = Select(t=0.0, s="Scan BD", f=w758) -> (s? t:f=w780:dbl)
        n514 = local read "BD 2 Frequency 2 (MHz)"() -> (w776:dbl)
        n515 = local read "BD 1 Frequency 2 (MHz)"() -> (w779:dbl)
        n516 = Add(x=w780, y=w751) -> (x+y=w777:dbl)
        n517 = Add(x=w745, y=w784) -> (x+y=w778:dbl)
        n518 = Multiply(x=w726, y=2.0) -> (x*y=w725:dbl)
        n519 = Multiply(x=w725, y="Number of F/B Scans (AOD)") -> (x*y=w722:dbl)
        n520 = Divide(x=w722, y=60.0) -> (x/y=→"Time to Finish All (min)":dbl)
        n521 = Add(x="Trap 2 Bead Size (nm)", y="Trap 1 Bead Size (nm)") -> (x+y=w766:dbl)
        n522 = Divide(x=w766, y=2.0) -> (x/y=w760:dbl)
        n523 = local read "Initial delta (MHz)"() -> (w763:dbl)
        n524 = Subtract(x=w777, y=w776) -> (x-y=w774:dbl)
        n525 = Subtract(x=w778, y=w779) -> (x-y=w775:dbl)
        n526 = Square(x=w774) -> (x^2=w773:dbl)
        n527 = Square(x=w775) -> (x^2=w772:dbl)
        n528 = Add(x=w772, y=w773) -> (x+y=w771:dbl)
        n529 = Square Root(x=w771) -> (sqrt(x)=w770:dbl)
        "Final delta (MHz)" <- w770
        n530 = Multiply(x=w762, y=w770) -> (x*y=w769:dbl)
        n531 = Multiply(x=w763, y=w762) -> (x*y=w761:dbl)
        n532 = Subtract(x=w761, y=w760) -> (x-y=→"Initial sep (nm)":dbl)
        n533 = Subtract(x=w769, y=w760) -> (x-y=→"Final sep (nm)":dbl)
      }
      event "Freq or Amp switch first", "Swap F1 and F2", "Freq switch delay", "Amp switch delay": Value Change {
        n534 = event-data() -> ()  [unwired: 7 out]
        n535 = local read "Freq or Amp switch first"() -> (w795:bool)
        n536 = local read "Amp switch delay"() -> (w796:u16)
        n537 = local read "Freq switch delay"() -> (w798:u16)
        n538 = local read "Swap F1 and F2"() -> (w797:bool)
        n539 = xnode "Read/Write Control"("FPGA VI Reference In"=w801, "error in"=w800, "Freq switch delay"=w798, "Swap F1 and F2"=w797, "Amp switch delay"=w796, "Freq or Amp switch first"=w795) -> ("error out"=w799:errorcluster)  [unwired: 1 out]
      }
      event "Scan steps (MCL)", "Number of scans (MCL)", "Scan Range (V)\n(of steps)", "2D or 1D Scan", "N APD Samp/step", "Fast Scan Dir", "Continuous MCL Scanning", "Scan lines (y)": Value Change {
        w803 = 32767.0 ("y")
        n540 = event-data() -> ()  [unwired: 7 out]
        n541 = Select(t="Scan lines (y)", s="2D or 1D Scan", f="Number of scans (MCL)") -> (s? t:f=w808:u64)
        n542 = Decrement(x="Scan steps (MCL)") -> (x-1=w824:u64)
        n543 = Divide(x="Scan Range (V)\n(of steps)", y=w824) -> (x/y=w823:dbl)
        "Desired Scan Incr (V)" <- w823
        n544 = local read "APD Integration Time (s)"() -> (w816:dbl)
        n545 = Multiply(x=w823, y=w803) -> (x*y=w832:dbl)
        n546 = Divide(x=w832, y=10.0) -> (x/y=w822:dbl)
        "Desired incr (int)" <- w822
        n547 = local read "Update Count (MCL)"() -> (w828:u32)
        n548 = Round Toward -Infinity(1:w822) -> (0:w831:dbl)
        n549 = To Word Integer(number=w831) -> (16bit integer=w806:i16)
        "Actual Incr. int (MCL)" <- w806
        n550 = Multiply(x=w816, y=40000000.0) -> (x*y=w829:dbl)
        n551 = Divide(x=w829, y=w828) -> (x/y=w827:dbl)
        n552 = Multiply(x=i16 10, y=w806) -> (x*y=w804:i16)
        n553 = Multiply(x="N APD Samp/step", y=w827) -> (x*y=w826:dbl)
        "Cycles/step (MCL)" <- w826
        n554 = Divide(x=w804, y=w803) -> (x/y=→"Actual MCL Inc (V)":dbl)
        n555 = Multiply(x="N APD Samp/step", y="Scan steps (MCL)") -> (x*y=w818:dbl)
        n556 = local read "APD Samples/FIFO Acq."() -> (w815:dbl)
        n557 = Multiply(x=w818, y=u64 2) -> (x*y=w817:dbl)
        "Data points/scan (f+b)" <- w817
        n558 = Multiply(x=w817, y=w808) -> (x*y=w835:dbl)
        "Data points/scans (MCL)" <- w835
        n559 = Multiply(x=w816, y=w817) -> (x*y=w809:dbl)
        "Time/f+b scan (s) (MCL)" <- w809
        n560 = Divide(x=w835, y=w815) -> (x/y=→"N sets should be saved (MCL)":dbl)
        n561 = Multiply(x=w809, y=w808) -> (x*y=→"Total Time (s)":dbl)
        n562 = Not(x="Fast Scan Dir") -> (.not. x?=w813:bool)
        n563 = xnode "Read/Write Control"("FPGA VI Reference In"=w839, "error in"=w838, "Scan steps (MCL)"="Scan steps (MCL)", "Number of scans (MCL)"=w808, "Cycles per step (MCL)"=w826, "Scan freq.  increment (MCL)"=w806, "1D or 2D Scan?"="2D or 1D Scan", "MCL Scan Axis"=w813, "Cont. Scan (MCL)"="Continuous MCL Scanning") -> ("error out"=w837:errorcluster)  [unwired: 1 out]
      }
      event "Read Cal": Value Change {
        w841 = 1000.0 ("y")
        n564 = event-data() -> ()  [unwired: 7 out]
        n565 = local read "Save file name"() -> (w866:path)
        n566 = local write "Read Cal"(FALSE ("Read Cal")) -> ()
        n567 = Strip Path(path=w866) -> (stripped path=w865:path)  [unwired: 1 out]
        n568 = Path To String(path=w865) -> (string=w864:string)
        n569 = Concatenate Strings(w864, "\\current.cal" ("string")) -> (w862:string)
        n570 = String To Path(string=w862) -> (path=w861:path)
        n571 = Open/Create/Replace File(file path (use dialog)=w861, operation (0:open)=T25."open", access (0:read/write)=enum16{"read/write", "read-only", "write-only"}."read-only") -> (refnum out=w869:refnum<file>, error out=w855:errorcluster)  [unwired: 1 in, 3 out]
        n572 = Deny Access(4:w855, 7:w869) -> (0:w854:errorcluster, 3:w860:refnum<file>)  [unwired: 1 out]
        n573 = Read from Binary File(5:0.0, 8:w854, 9:T24."big-endian, network order" ("byte order (0:big-endian, network order)"), 10:-1 ("count (1)"), 11:w860) -> (0:w853:errorcluster, 2:w851:dbl[], 3:w856:refnum<file>)  [unwired: 2 out]
        n574 = Array To Cluster(array=w851) -> (cluster=w850:T27)
        n575 = Unbundle(w850) -> ("[0]"=w849:dbl, "[1]"=w848:dbl, "[2]"=w847:dbl, "[3]"=w846:dbl, "[4]"=w845:dbl, "[5]"=w844:dbl)
        n576 = Close File(refnum=w856, error in=w853) -> (error out=→"Read cal error":errorcluster)  [unwired: 1 out]
        n577 = Multiply(x=w844, y=w841) -> (x*y=w842:dbl)
        n578 = local write "T2 kappa_x (pN/nm)"(w846) -> ()
        n579 = local write "T1 kappa_x (pN/nm)"(w847) -> ()
        n580 = local write "T1 alpha_x (nm/V)"(w849) -> ()
        n581 = local write "T2 alpha_x (nm/V)"(w848) -> ()
        n582 = Multiply(x=w845, y=w841) -> (x*y=w843:dbl)
        n583 = local write "T1 offset_x (mV)"(w843) -> ()
        n584 = local write "T2 offset_x (mV)"(w842) -> ()
      }
      event "Abort MCL Scan": Value Change {
        n585 = event-data() -> ()  [unwired: 7 out]
        n586 = local write "MCL Scanning"(FALSE ("MCL Scanning")) -> ()
        n587 = xnode "Read/Write Control"("FPGA VI Reference In"=w874, "error in"=w873, "Abort scan (MCL)"="Abort MCL Scan") -> ("error out"=w872:errorcluster)  [unwired: 1 out]
      }
      event "Update Count (MCL)": Value Change {
        n588 = event-data() -> ()  [unwired: 7 out]
        n589 = xnode "Read/Write Control"("FPGA VI Reference In"=w878, "error in"=w877, "MCL count"="Update Count (MCL)") -> ("error out"=w876:errorcluster)  [unwired: 1 out]
      }
      event "Phase adjust (MCL)", "+ phase (MCL)", "- phase (MCL)": Value Change {
        n590 = event-data() -> ()  [unwired: 7 out]
        n591 = Negate(x="Phase adjust (MCL)") -> (-x=w887:i16)
        n592 = Select(t=w887, s="- phase (MCL)", f="Phase adjust (MCL)") -> (s? t:f=w885:i16)
        n593 = Or(x="- phase (MCL)", y="+ phase (MCL)") -> (x .or. y?=w880:bool)
        n594 = xnode "Read/Write Control"("FPGA VI Reference In"=w889, "error in"=w888, "Phase count adjustment (MCL)"=w885) -> ("FPGA VI Reference Out"=w881:T19, "error out"=w882:errorcluster)
        n595 = xnode "Read/Write Control"("FPGA VI Reference In"=w881, "error in"=w882, "+ phase (MCL)"=w880) -> ("error out"=w879:errorcluster)  [unwired: 1 out]
      }
      event "Abort AOD Scan": Value Change {
        n596 = event-data() -> ()  [unwired: 7 out]
        n597 = xnode "Read/Write Control"("FPGA VI Reference In"=w893, "error in"=w892, "Abort scan"="Abort AOD Scan") -> ("error out"=w891:errorcluster)  [unwired: 1 out]
      }
      event "Continuous AOD Scanning": Value Change {
        n598 = event-data() -> ()  [unwired: 7 out]
        n599 = xnode "Read/Write Control"("FPGA VI Reference In"=w897, "error in"=w896, "Cont. Scan"="Continuous AOD Scanning") -> ("error out"=w895:errorcluster)  [unwired: 1 out]
      }
      event "Index": Value Change {
        n600 = event-data() -> ()  [unwired: 7 out]
        n601 = call "Create new save file.vi"("Insert"="", "Ext"=".dat" ("string"), "Index In"="Index") -> ("Path Out"=→"Save file name":path, "Index Out"=w898:dbl)
        "Save index" <- w898
        n602 = local write "Index"(w898) -> ()
      }
      event "AO1", "AO2": Value Change {
        w913 = 10.0 ("y")
        w912 = 32767.0 ("y")
        n603 = event-data() -> ()  [unwired: 7 out]
        n604 = local read "AO2"() -> (w911:dbl)
        n605 = local read "AO1"() -> (w908:dbl)
        n606 = Multiply(x=w908, y=w912) -> (x*y=w907:dbl)
        n607 = Multiply(x=w911, y=w912) -> (x*y=w910:dbl)
        n608 = Divide(x=w907, y=w913) -> (x/y=w906:dbl)
        n609 = Divide(x=w910, y=w913) -> (x/y=w909:dbl)
        n610 = To Word Integer(number=w906) -> (16bit integer=w914:i16)
        n611 = To Word Integer(number=w909) -> (16bit integer=w915:i16)
        n612 = xnode "Read/Write Control"("FPGA VI Reference In"=w905, "error in"=w904, "AO1"=w914, "AO2"=w915) -> ("error out"=w903:errorcluster)  [unwired: 1 out]
      }
      event "Inject Pump 1": Value Change {
        n613 = local read "Chemyx Syringe Pump Serial Port"() -> (w916:refnum<visa-resource-name>)
        n614 = event-data() -> ()  [unwired: 7 out]
        n615 = local read "Pump write delay (ms)"() -> (w917:dbl)
        n616 = case shown="True" "Inject Pump 1" {
          tunnel: w917 -> [w924 w938]
          tunnel: w916 -> [w921 w937]
          frame False {
            n617 = flat-sequence {
              tunnel: w921 -> [w925]
              tunnel: [w925] -> w922
              tunnel: w924 -> [_]
              tunnel: [w928] -> w923
              tunnel: w922 -> [w928]
              tunnel: w923 -> [w929]
              tunnel: [w929] -> w919
              tunnel: [w931] -> w920
              tunnel: w919 -> [w931]
              tunnel: w920 -> [w933]
              frame #0 {
                n618 = call "Write to pump.vi"("string"="enter pump1", "VISA resource name"=w925) -> ()  [unwired: 1 out]
              }
              frame #1 {
                n619 = Wait (ms)(milliseconds to wait="Pump pause delay (ms)") -> ()  [unwired: 1 out]
              }
              frame #2 {
                n620 = call "Write to pump.vi"("string"="stop", "VISA resource name"=w929) -> ()  [unwired: 1 out]
              }
              frame #3 {
                n621 = Wait (ms)(milliseconds to wait=u32 500) -> ()  [unwired: 1 out]
              }
              frame #4 {
                n622 = call "Write to pump.vi"("string"="stop", "VISA resource name"=w933) -> ()  [unwired: 1 out]
              }
            }
          }
          frame True {
            n623 = flat-sequence {
              tunnel: w937 -> [w947]
              tunnel: w938 -> [w942]
              tunnel: w938 -> [w949]
              tunnel: w937 -> [w950]
              tunnel: [w950] -> w935
              tunnel: [w952] -> w936
              tunnel: w935 -> [w952]
              tunnel: w936 -> [w954]
              frame #0 {
                n624 = local read "All Pump Parameters"() -> (w941:T5)
                n625 = Unbundle By Name(w941) -> ("Pump 1"=w948:T28)
                n626 = call "Set pump parameters.vi"("Pump write delay (ms)"=w942, "Volume (uL)"="Ch 2 Inject Volume (uL)", "Rate (uL/h)"="Ch 1 Inject Rate (ul/h)", "Units"=4.0, "Pump #"=1.0, "Pump Parameters In"=w948, "VISA resource name"=w947) -> ("Pump Parameters Out"=w940:T28)  [unwired: 3 in]
                n627 = Bundle By Name(cluster=w941, "Pump 1"=w940) -> (w939:T5)
                n628 = local write "All Pump Parameters"(w939) -> ()
              }
              frame #1 {
                n629 = Wait (ms)(milliseconds to wait=w949) -> ()  [unwired: 1 out]
              }
              frame #2 {
                n630 = call "Write to pump.vi"("string"="start", "VISA resource name"=w950) -> ()  [unwired: 1 out]
              }
              frame #3 {
                n631 = Wait (ms)(milliseconds to wait=u32 500) -> ()  [unwired: 1 out]
              }
              frame #4 {
                n632 = call "Write to pump.vi"("string"="start", "VISA resource name"=w954) -> ()  [unwired: 1 out]
              }
            }
          }
        }
      }
      event "Inject Pump 3": Value Change {
        n633 = event-data() -> ()  [unwired: 7 out]
        n634 = local read "Pump write delay (ms)"() -> (w957:dbl)
        n635 = case shown="False" "Inject Pump 3" {
          tunnel: w957 -> [w964 w978]
          tunnel: "Chemyx Syringe Pump Serial Port" -> [w961 w977]
          frame False {
            n636 = flat-sequence {
              tunnel: w961 -> [w965]
              tunnel: [w965] -> w962
              tunnel: w964 -> [_]
              tunnel: [w968] -> w963
              tunnel: w962 -> [w968]
              tunnel: w963 -> [w969]
              tunnel: [w969] -> w959
              tunnel: [w971] -> w960
              tunnel: w959 -> [w971]
              tunnel: w960 -> [w973]
              frame #0 {
                n637 = call "Write to pump.vi"("string"="enter pump3", "VISA resource name"=w965) -> ()  [unwired: 1 out]
              }
              frame #1 {
                n638 = local read "Pump pause delay (ms)"() -> (w967:u32)
                n639 = Wait (ms)(milliseconds to wait=w967) -> ()  [unwired: 1 out]
              }
              frame #2 {
                n640 = call "Write to pump.vi"("string"="stop", "VISA resource name"=w969) -> ()  [unwired: 1 out]
              }
              frame #3 {
                n641 = Wait (ms)(milliseconds to wait=u32 0) -> ()  [unwired: 1 out]
              }
              frame #4 {
                n642 = call "Write to pump.vi"("string"="stop", "VISA resource name"=w973) -> ()  [unwired: 1 out]
              }
            }
          }
          frame True {
            n643 = flat-sequence {
              tunnel: w977 -> [w987]
              tunnel: w978 -> [w982]
              tunnel: w978 -> [w989]
              tunnel: w977 -> [w990]
              tunnel: [w990] -> w975
              tunnel: [w993] -> w976
              tunnel: w975 -> [w993]
              tunnel: w976 -> [w994]
              frame #0 {
                n644 = local read "All Pump Parameters"() -> (w981:T5)
                n645 = Unbundle By Name(w981) -> ("Pump 3"=w988:T28)
                n646 = call "Set pump parameters.vi"("Pump write delay (ms)"=w982, "Volume (uL)"="Ch 3 Inject Volume (uL)", "Rate (uL/h)"="Ch 3 Inject Rate (ul/h)", "Units"=4.0, "Pump #"=3.0, "Pump Parameters In"=w988, "VISA resource name"=w987) -> ("Pump Parameters Out"=w980:T28)  [unwired: 3 in]
                n647 = Bundle By Name(cluster=w981, "Pump 3"=w980) -> (w979:T5)
                n648 = local write "All Pump Parameters"(w979) -> ()
              }
              frame #1 {
                n649 = Wait (ms)(milliseconds to wait=w989) -> ()  [unwired: 1 out]
              }
              frame #2 {
                n650 = call "Write to pump.vi"("string"="start", "VISA resource name"=w990) -> ()  [unwired: 1 out]
              }
              frame #3 {
                n651 = Wait (ms)(milliseconds to wait=u32 500) -> ()  [unwired: 1 out]
              }
              frame #4 {
                n652 = call "Write to pump.vi"("string"="start", "VISA resource name"=w994) -> ()  [unwired: 1 out]
              }
            }
          }
        }
      }
      event "Inject Pump 2": Value Change {
        n653 = event-data() -> ()  [unwired: 7 out]
        n654 = local read "Pump write delay (ms)"() -> (w998:dbl)
        n655 = flat-sequence {
          tunnel: w996 -> [w1011]
          tunnel: w998 -> [w1007]
          tunnel: "Inject Pump 2" -> [_]
          tunnel: w998 -> [w1013]
          tunnel: w996 -> [w1014]
          frame #0 {
            n656 = local read "All Pump Parameters"() -> (w1006:T5)
            n657 = Multiply(x=60.0, y="Flush Center Ch Rate (ul/m)") -> (x*y=w1003:dbl)
            n658 = Unbundle By Name(w1006) -> ("Pump 2"=w1012:T28)
            n659 = call "Set pump parameters.vi"("Pump write delay (ms)"=w1007, "Volume (uL)"="Flush Center Ch Volume (uL)", "Rate (uL/h)"=w1003, "Units"=3.0, "Pump #"=2.0, "Pump Parameters In"=w1012, "VISA resource name"=w1011) -> ("Pump Parameters Out"=w1005:T28)  [unwired: 3 in]
            n660 = Bundle By Name(cluster=w1006, "Pump 2"=w1005) -> (w1004:T5)
            n661 = local write "All Pump Parameters"(w1004) -> ()
            n662 = Add(x="Flush Center Ch Volume (uL)", y="Total Volume\nFlushed (uL)") -> (x+y=w1000:dbl)
            n663 = local write "Total Volume\nFlushed (uL)"(w1000) -> ()
          }
          frame #1 {
            n664 = Wait (ms)(milliseconds to wait=w1013) -> ()  [unwired: 1 out]
          }
          frame #2 {
            n665 = call "Write to pump.vi"("string"="start", "VISA resource name"=w1014) -> ()  [unwired: 1 out]
          }
        }
        n666 = local read "Chemyx Syringe Pump Serial Port"() -> (w996:refnum<visa-resource-name>)
      }
      event "Sample Channel Flow": Value Change {
        n667 = event-data() -> ()  [unwired: 7 out]
        n668 = Select(t="run" ("string"), s="Sample Channel Flow", f="stop" ("string")) -> (s? t:f=w1016:string)
        n669 = Concatenate Strings(w1016, "\r") -> (w1020:string)
        n670 = VISA Write(VISA resource name=w1022, write buffer=w1020) -> ()  [unwired: 1 in, 3 out]
      }
      event "Flip Green Filter": Value Change {
        n671 = event-data() -> ()  [unwired: 7 out]
        n672 = Not(x="Flip Green Filter") -> (.not. x?=w1023:bool)
        n673 = local write "Flip Green Filter"(w1023) -> ()
        n674 = flat-sequence {
          tunnel: w1031 -> [w1036]
          tunnel: w1030 -> [w1035]
          tunnel: [w1033] -> w1028
          tunnel: [w1032] -> w1027
          tunnel: [w1038] -> w1026
          tunnel: w1028 -> [w1038]
          tunnel: [w1037] -> w1025
          tunnel: w1027 -> [w1037]
          tunnel: w1026 -> [w1042]
          tunnel: w1025 -> [w1041]
          tunnel: [w1040] -> w1029
          frame #0 {
            n675 = xnode "Read/Write Control"("FPGA VI Reference In"=w1036, "error in"=w1035, "Green Filter Flipper"=TRUE) -> ("FPGA VI Reference Out"=w1033:T19, "error out"=w1032:errorcluster)
          }
          frame #1 {
            n676 = Wait (ms)(milliseconds to wait=u32 100) -> ()  [unwired: 1 out]
          }
          frame #2 {
            n677 = xnode "Read/Write Control"("FPGA VI Reference In"=w1042, "error in"=w1041, "Green Filter Flipper"=FALSE) -> ("error out"=w1040:errorcluster)  [unwired: 1 out]
          }
        }
      }
      event "Pump 1 contents", "Pump 3 contents": Value Change {
        n678 = event-data() -> ()  [unwired: 7 out]
        n679 = local read "Pump 1 contents"() -> (→"Pump 1 cont disp":string)
        n680 = local read "Pump 3 contents"() -> (→"Pump 3 cont disp":string)
      }
      event "Reset Trap Pos. FB": Value Change {
        n681 = event-data() -> ()  [unwired: 7 out]
        n682 = xnode "Read/Write Control"("FPGA VI Reference In"=w1048, "error in"=w1047, "Trap Pos. FB Reset"="Reset Trap Pos. FB") -> ()  [unwired: 2 out]
      }
      event "Trap Pos. FB ON": Value Change {
        n683 = event-data() -> ()  [unwired: 7 out]
        n684 = xnode "Read/Write Control"("FPGA VI Reference In"=w1051, "error in"=w1050, "Force feedback"="Trap Pos. FB ON") -> ()  [unwired: 2 out]
      }
      event "Remove Action Offset": Value Change {
        n685 = event-data() -> ()  [unwired: 7 out]
        n686 = local write "Remove Action Offset"(FALSE ("Remove Action Offset")) -> ()
        n687 = local read "Trap Pos. FB Mult Factor"() -> (w1056:i64)
        n688 = local read "Trap Pos FB Action"() -> (w1054:i64)
        n689 = local read "Trap Pos. FB Offset Factor"() -> (w1052:i64)
        n690 = Multiply(x=w1056, y=w1054) -> (x*y=w1055:i64)
        n691 = Add(x=w1055, y=w1052) -> (x+y=w1053:i64)
        n692 = xnode "Read/Write Control"("FPGA VI Reference In"=w1059, "error in"=w1058, "Trap Pos. FB Offset Factor"=w1053) -> ()  [unwired: 2 out]
        n693 = local write "Trap Pos. FB Offset Factor"(w1053) -> ()
      }
      event "Trap Pos. FB Range", "Trap Pos. FB Gains", "Trap Pos. FB Mult Factor", "Trap Pos. FB Offset Factor", "Trap Pos FB Negate Action", "Trap Pos FB Monitor\nT1 or T2": Value Change {
        n694 = event-data() -> ()  [unwired: 7 out]
        n695 = xnode "Read/Write Control"("FPGA VI Reference In"=w1068, "error in"=w1067, "Trap Pos. FB Range"="Trap Pos. FB Range", "Trap Pos. FB Gains"="Trap Pos. FB Gains", "Trap Pos. FB Mult Factor"="Trap Pos. FB Mult Factor", "Trap Pos. FB Offset Factor"="Trap Pos. FB Offset Factor", "Trap Pos FB Negate Action"="Trap Pos FB Negate Action", "Trap Pos FB Monitor T1 or T2"="Trap Pos FB Monitor\nT1 or T2", "AI1 X Scale"="Trap Pos. AI1 X Pre-scale") -> ()  [unwired: 2 out]
      }
      event "Trap Pos FB SP": Value Change {
        n696 = event-data() -> ()  [unwired: 7 out]
        n697 = xnode "Read/Write Control"("FPGA VI Reference In"=w1071, "error in"=w1070, "Trap Pos. FB SP"="Trap Pos FB SP") -> ()  [unwired: 2 out]
      }
      event "Set SP to Reading": Value Change {
        n698 = event-data() -> ()  [unwired: 7 out]
        n699 = local read "Trap Pos FB Monitor\nT1 or T2"() -> (w1080:bool)
        n700 = local read "Trap X AI1 (DMA)"() -> (w1083:T13)
        n701 = local read "Trap X (AI1)"() -> (w1086:T10)
        n702 = local write "Set SP to Reading"(FALSE ("Set SP to Reading")) -> ()
        n703 = Unbundle By Name(w1086) -> ("Trap 1"=w1085:fxp<+/-,16,1>, "Trap 2"=w1084:fxp<+/-,16,1>)
        n704 = Unbundle By Name(w1083) -> ("Set 1"=w1082:fxp<+/-,16,1>, "Set 2"=w1081:fxp<+/-,16,1>)
        n705 = Select(t=w1085, s=w1080, f=w1084) -> (s? t:f=w1079:fxp<+/-,16,1>)
        n706 = Select(t=w1082, s=w1080, f=w1081) -> (s? t:f=w1078:fxp<+/-,16,1>)
        n707 = Not(x="Set SP Using...") -> (.not. x?=w1073:bool)
        n708 = Select(t=w1079, s=w1073, f=w1078) -> (s? t:f=w1074:fxp<+/-,16,1>)
        n709 = xnode "Read/Write Control"("FPGA VI Reference In"=w1076, "error in"=w1075, "Trap Pos. FB SP"=w1074) -> ()  [unwired: 2 out]
        n710 = local write "Trap Pos FB SP"(w1074) -> ()
      }
      event "Trap Pos. FB Out Scale 2^n": Value Change {
        n711 = event-data() -> ()  [unwired: 7 out]
        n712 = Scale By Power Of 2(n="Trap Pos. FB Out Scale 2^n", x=ext 1.0) -> (x*2^n=w1087:ext)
        n713 = property on="Trap Pos. FB Mult Factor" class="DigNum (strict)"("Val(Sgnl)"=w1087) -> ()  [unwired: 2 in, 2 out]
      }
      event "Trap Pos FB Int Count": Value Change {
        n714 = event-data() -> ()  [unwired: 7 out]
        n715 = xnode "Read/Write Control"("FPGA VI Reference In"=w1092, "error in"=w1091, "Trap Pos FB Int Count"="Trap Pos FB Int Count") -> ()  [unwired: 2 out]
      }
    }
    "error out 2" <- w315
    n716 = node-c288() -> ()  [unwired: 2 out]
  }
  n717 = disable-structure shown="Disabled" {
    disable-tunnel: [w1094 _] -> w217
    disable-tunnel: w36 -> [w1093 _]
    frame Disabled {
      n718 = node-c288() -> (w1096:T21)  [unwired: 4 out]
      n719 = timed-loop "Rough control of MCL mirror stage (debugging)" {
        tunnel: w1093 -> [w1099]
        tunnel: [w1098] -> w1094
        timing: w1096 -> [_]
        timing-out: [_] -> w1095
        stop <- w1098 stop-if-true
        n720 = node-c288() -> ()  [unwired: 2 out]
        n721 = case shown="1" "MCL Mode" {
          tunnel: w1099 -> [_ w1102 w1149]
          frame 0, Default {
          }
          frame 1 {
            n722 = node-c288() -> (w1104:T21)  [unwired: 4 out]
            n723 = timed-loop "Oscillate MCL mirror" {
              timing: w1104 -> [_]
              timing-out: [_] -> w1103
              tunnel: w1102 -> [w1143]
              i -> [w1142]
              stop <- w1105 stop-if-true
              n724 = node-c288() -> (w1141:i64)  [unwired: 1 out]
              n725 = Multiply(x="AO1", y=32767.0) -> (x*y=w1137:dbl)
              n726 = Multiply(x="AO2", y=32767.0) -> (x*y=w1132:dbl)
              n727 = Divide(x=w1137, y=10.0) -> (x/y=w1138:dbl)
              n728 = Divide(x=w1132, y=10.0) -> (x/y=w1133:dbl)
              n729 = To Word Integer(number=w1138) -> (16bit integer=w1130:i16)
              n730 = To Word Integer(number=w1133) -> (16bit integer=w1129:i16)
              n731 = Divide(x=w1141, y=i64 1000) -> (x/y=w1112:dbl)
              n732 = Multiply(x=w1112, y=w1142) -> (x*y=w1123:dbl)
              n733 = Multiply(x="Osc. freq. (Hz) 2", y=6.283185307179586) -> (x*y=w1124:dbl)
              n734 = Multiply(x=w1124, y=w1123) -> (x*y=w1122:dbl)
              n735 = Sine(x=w1122) -> (sin(x)=w1121:dbl)
              n736 = Multiply(x=w1121, y="Osc. amp. (V)") -> (x*y=w1119:dbl)
              n737 = Add(x=w1119, y="Osc. center (V)") -> (x+y=w1117:dbl)
              n738 = Divide(x=w1117, y=10.0) -> (x/y=w1115:dbl)
              n739 = Multiply(x=w1115, y=32767.0) -> (x*y=w1110:dbl)
              n740 = Select(t=w1110, s="Scan axis", f=w1130) -> (s? t:f=w1128:dbl)
              n741 = Select(t=w1129, s="Scan axis", f=w1110) -> (s? t:f=w1127:dbl)
              n742 = local read "MCL Mode"() -> (w1109:u16)
              n743 = Not Equal?(x=w1109, y=u16 1) -> (x != y?=w1106:bool)
              n744 = local read "Stop All"() -> (w1107:bool)
              n745 = xnode "Read/Write Control"("FPGA VI Reference In"=w1143, "AO1"=w1128, "AO2"=w1127) -> ()  [unwired: 1 in, 2 out]
              n746 = Compound Arithmetic op=OR(w1107, w1106) -> (w1105:bool)
              n747 = node-c288() -> ()  [unwired: 2 out]
            }
            n748 = node-c288(w1103) -> ()  [unwired: 1 out]
          }
          frame 2 {
            n749 = case shown="True" "Start Scan" {
              tunnel: w1149 -> [_ w1161]
              frame False {
              }
              frame True {
                n750 = Subtract(x="End (V)", y="Begin (V)") -> (x-y=w1157:dbl)
                n751 = Decrement(x="N Points") -> (x-1=w1156:dbl)
                n752 = Divide(x=w1157, y=w1156) -> (x/y=w1154:dbl)
                n753 = for {
                  N: "N Points" -> [_]
                  tunnel: "Begin (V)" -> [w1174]
                  tunnel: w1161 -> [w1166]
                  tunnel: [w1165] -> w1160 mode=indexing
                  tunnel: w1154 -> [w1164]
                  tunnel: [w1162] -> w1153 mode=indexing
                  i -> [w1173]
                  n754 = Multiply(x=w1164, y=w1173) -> (x*y=w1172:dbl)
                  n755 = Add(x=w1174, y=w1172) -> (x+y=w1169:dbl)
                  n756 = local read "Scan axis"() -> (w1163:bool)
                  n757 = local read "AO1"() -> (w1171:dbl)
                  n758 = local read "AO2"() -> (w1170:dbl)
                  n759 = Select(t=w1169, s=w1163, f=w1171) -> (s? t:f=w1168:dbl)
                  n760 = Select(t=w1170, s=w1163, f=w1169) -> (s? t:f=w1167:dbl)
                  n761 = flat-sequence {
                    tunnel: w1168 -> [w1178]
                    tunnel: w1167 -> [w1177]
                    tunnel: w1166 -> [w1175]
                    tunnel: [w1188] -> w1165
                    tunnel: [w1187] -> w1162
                    frame #0 {
                      w1181 = 10.0 ("y")
                      w1176 = 32767.0 ("y")
                      n762 = Multiply(x=w1178, y=w1176) -> (x*y=w1184:dbl)
                      n763 = Multiply(x=w1177, y=w1176) -> (x*y=w1182:dbl)
                      n764 = Divide(x=w1184, y=w1181) -> (x/y=w1185:dbl)
                      n765 = Divide(x=w1182, y=w1181) -> (x/y=w1183:dbl)
                      n766 = To Word Integer(number=w1185) -> (16bit integer=w1179:i16)
                      n767 = To Word Integer(number=w1183) -> (16bit integer=w1180:i16)
                      n768 = xnode "Read/Write Control"("FPGA VI Reference In"=w1175, "AO1"=w1179, "AO2"=w1180) -> ()  [unwired: 1 in, 2 out]
                    }
                    frame #1 {
                      n769 = Wait (ms)(milliseconds to wait="DAQ Delay (ms)") -> ()  [unwired: 1 out]
                    }
                    frame #2 {
                      n770 = local read "Slow mean"() -> (w1188:dbl)
                      n771 = local read "Sigma"() -> (w1187:dbl)
                    }
                  }
                }
                n772 = Bundle("Begin (V)"="Begin (V)", w1154, w1160) -> (→"MCL Scan":cluster{"Begin (V)":dbl, dbl, dbl[]})  [unwired: 1 out]
                n773 = Bundle("Begin (V)"="Begin (V)", w1154, w1153) -> (→"MCL Scan 2":cluster{"Begin (V)":dbl, dbl, dbl[]})  [unwired: 1 out]
              }
            }
          }
        }
        n774 = local read "Stop All"() -> (w1098:bool)
        n775 = node-c288() -> ()  [unwired: 2 out]
      }
      n776 = node-c288(w1095) -> ()  [unwired: 1 out]
    }
    frame Enabled {
    }
  }
  n777 = timed-loop "Run Scripts, including: stage motion" {
    tunnel: w70 -> [w1193]
    tunnel: w69 -> [w1194]
    tunnel: [w1194] -> w68
    tunnel: [w1193] -> w67
    timing: w65 -> [_]
    timing-out: [_] -> w64
    tunnel: w50 -> [w1192]
    tunnel: w51 -> [w1191]
    stop <- w1195 stop-if-true
    n778 = node-c288() -> ()  [unwired: 1 in, 1 out]
    n779 = event shown="[11] \"Take Force FB Data Upper Channel\": Value Change" {
      selector: _ -> [_ _ _ _ _ _ _ _ _ _ _ _ _ _ _ _ _]
      dyn-events: _ -> [_ _ _ _ _ _ _ _ _ _ _ _ _ _ _ _ _]
      timeout: _ -> [_ _ _ _ _ _ _ _ _ _ _ _ _ _ _ _ _]
      tunnel: ["Set Position" "Move to Position" "Move Cap. 1 (DNA Right)" "Move Cap. 2 (ADig Left)" _ "Cal/Data Acq. Spot" "Dump Beads" "Dip for Protein" _ _ "Got ADig bead" "Take Force FB Data\nUpper Channel" "Got DNA bead" "Take Stepping Data" _ "Take Detection Laser\nImage" _] -> _
      tunnel: [_ _ _ _ _ _ _ _ _ _ _ _ _ _ _ _ w1733] -> w1195
      tunnel: w1193 -> [w1213 w1221 w1245 w1300 w1346 w1382 w1460 w1486 w1536 w1562 _ w1591 _ _ _ _ _]
      tunnel: w1194 -> [w1214 w1222 w1246 w1301 w1347 w1383 w1461 w1487 w1537 w1563 _ w1592 _ _ _ _ _]
      tunnel: w1192 -> [_ _ w1243 w1297 _ _ _ _ _ _ _ _ _ _ _ _ _]
      tunnel: w1191 -> [_ _ w1242 w1298 _ _ _ _ _ _ _ _ _ _ _ _ _]
      event "Set Position", "Set Position 2", "Set Position 3", "Set Position 4", "Set Position 5", "Set Position 1": Value Change {
        n780 = event-data() -> ()  [unwired: 1 in, 5 out]
        n781 = Build Array("Set Position 1", "Set Position 2", "Set Position 3", "Set Position 4", "Set Position 5") -> (w1212:bool[])
        n782 = Boolean Array To Number(Boolean array=w1212) -> (number=w1211:u32)
        n783 = Logarithm Base 2(1:w1211) -> (0:w1203:dbl)
        n784 = call "Read Stage Position.vi"("error in"=w1213, "VISA resource name in"=w1214) -> ("Current Position"=w1218:cluster{dbl, dbl, dbl}, "error out"=w1217:errorcluster)  [unwired: 2 out]
        n785 = Decrement(x="Position") -> (x-1=w1201:dbl)
        n786 = Greater Or Equal?(x=w1203, y=0.0) -> (x >= y?=w1204:bool)
        n787 = local write "Stage Control Serial Error"(w1217) -> ()
        n788 = Cluster To Array(cluster=w1218) -> (array=w1215:dbl[])
        n789 = Select(t=w1203, s=w1204, f=w1201) -> (s? t:f=w1200:dbl)
        n790 = Increment(x=w1200) -> (x+1=w1199:dbl)
        n791 = Build Array (concatenate)(w1199, w1215) -> (w1198:dbl[])
        n792 = Replace Array Subset(array="Saved Stage Positions", new element=w1198, index (row)=w1200) -> (w1216:dbl[][])  [unwired: 1 in]
        n793 = local write "Saved Stage Positions"(w1216) -> ()
      }
      event "Move to Position": Value Change {
        n794 = event-data() -> ()  [unwired: 1 in, 5 out]
        n795 = flat-sequence {
          tunnel: w1222 -> [w1225]
          tunnel: w1221 -> [w1224]
          frame #0 {
            n796 = local read "Position"() -> (w1237:dbl)
            n797 = local read "Saved Stage Positions"() -> (w1235:dbl[][])
            n798 = Decrement(x=w1237) -> (x-1=w1234:dbl)
            n799 = Array Subset(array=w1235, index (row)=w1234, length (row)=1 ("length"), index (col)=1 ("index"), length (col)=3 ("length")) -> (w1231:dbl[][])
            n800 = Reshape Array(w1231, 3 ("dimension size")) -> (w1229:dbl[])
            n801 = Array To Cluster(array=w1229) -> (cluster=w1228:cluster{"[0]":dbl, "[1]":dbl, "[2]":dbl})
            n802 = call "Set Stage Position.vi"("Position"=w1228, "error in"=w1224, "VISA resource name in"=w1225) -> ("error out"=w1227:errorcluster)  [unwired: 2 out]
            n803 = local write "Stage Control Serial Error"(w1227) -> ()
            n804 = local write "Stage Moving"(TRUE ("Stage Moving")) -> ()
          }
          frame #1 {
            n805 = call <vilib>:"Beep.vi"() -> ()  [unwired: 3 in, 9 out]
            n806 = local write "Stage Moving"(FALSE ("Stage Moving")) -> ()
          }
        }
      }
      event "Move Cap. 1 (DNA Right)": Value Change {
        n807 = event-data() -> ()  [unwired: 1 in, 5 out]
        n808 = local write "Move Cap. 1 (DNA Right)"(FALSE ("Move Cap. 1 (DNA Right)")) -> ()
        n809 = flat-sequence {
          tunnel: w1246 -> [w1254]
          tunnel: w1245 -> [w1253]
          tunnel: w1243 -> [w1252]
          tunnel: w1242 -> [w1251]
          tunnel: [w1250] -> w1241
          tunnel: [w1249] -> w1240
          tunnel: ["Cap 1 Samp Flow ON"] -> w1239
          tunnel: w1241 -> [w1277]
          tunnel: w1240 -> [w1276]
          tunnel: w1239 -> [w1275]
          frame #0 {
            n810 = local read "Saved Stage Positions"() -> (w1264:dbl[][])
            n811 = Array Subset(array=w1264, index (row)=0 ("index"), length (row)=1 ("length"), index (col)=1 ("index"), length (col)=3 ("length")) -> (w1261:dbl[][])
            n812 = Reshape Array(w1261, 3 ("dimension size")) -> (w1259:dbl[])
            n813 = Array To Cluster(array=w1259) -> (cluster=w1258:cluster{"[0]":dbl, "[1]":dbl, "[2]":dbl})
            n814 = case shown="True" "Cap 1 Samp Flow ON" {
              tunnel: w1251 -> [w1266 w1272]
              tunnel: w1252 -> [w1267 w1271]
              tunnel: [w1267 w1269] -> w1250
              tunnel: [w1266 w1268] -> w1249
              frame False {
              }
              frame True {
                # "run flow"
                n815 = Concatenate Strings("run" ("string"), "\r") -> (w1273:string)
                n816 = VISA Write(VISA resource name=w1271, write buffer=w1273, error in (no error)=w1272) -> (VISA resource name out=w1269:refnum<visa-resource-name>, error out=w1268:errorcluster)  [unwired: 1 out]
              }
            }
            n817 = call "Set Stage Position.vi"("Position"=w1258, "error in"=w1253, "VISA resource name in"=w1254) -> ("error out"=w1257:errorcluster)  [unwired: 2 out]
            n818 = local write "Stage Control Serial Error"(w1257) -> ()
            n819 = local write "Stage Moving"(TRUE ("Stage Moving")) -> ()
          }
          frame #1 {
            n820 = local write "Stage Moving"(FALSE ("Stage Moving")) -> ()
            n821 = case shown="True" w1275 {
              tunnel: w1276 -> [w1282 w1288]
              tunnel: w1277 -> [w1283 w1287]
              tunnel: [w1283 w1285] -> _
              tunnel: [w1282 w1284] -> _
              frame False {
              }
              frame True {
                n822 = Concatenate Strings("stop" ("string"), "\r") -> (w1289:string)
                n823 = VISA Write(VISA resource name=w1287, write buffer=w1289, error in (no error)=w1288) -> (VISA resource name out=w1285:refnum<visa-resource-name>, error out=w1284:errorcluster)  [unwired: 1 out]
              }
            }
            n824 = case shown="True" TRUE {
              tunnel: "Cap 1 T ON" -> [w1292 w1293]
              frame False {
                n825 = property on="Trap 1 (ON/OFF)" class="Bool (strict)"("Val(Sgnl)"=w1292) -> ()  [unwired: 2 in, 2 out]
              }
              frame True {
                n826 = property on="Trap 2 (ON/OFF)" class="Bool (strict)"("Val(Sgnl)"=w1293) -> ()  [unwired: 2 in, 2 out]
              }
            }
            n827 = call <vilib>:"Beep.vi"() -> ()  [unwired: 3 in, 9 out]
            n828 = case shown="True" "Cap 1 Flow ON" {
              frame False {
              }
              frame True {
                n829 = property on="Inject Pump 1" class="Bool (strict)"("Val(Sgnl)"=TRUE ("Value (Signaling)")) -> ()  [unwired: 2 in, 2 out]
              }
            }
          }
        }
      }
      event "Move Cap. 2 (ADig Left)": Value Change {
        n830 = event-data() -> ()  [unwired: 1 in, 5 out]
        n831 = local write "Move Cap. 2 (ADig Left)"(FALSE ("Move Cap. 2 (ADig Left)")) -> ()
        n832 = flat-sequence {
          tunnel: w1301 -> [w1309]
          tunnel: w1300 -> [w1308]
          tunnel: w1298 -> [w1307]
          tunnel: w1297 -> [w1306]
          tunnel: [w1305] -> w1296
          tunnel: [w1304] -> w1295
          tunnel: ["Cap 2 Samp Flow ON"] -> w1294
          tunnel: w1296 -> [w1332]
          tunnel: w1295 -> [w1331]
          tunnel: w1294 -> [w1330]
          frame #0 {
            n833 = local read "Saved Stage Positions"() -> (w1319:dbl[][])
            n834 = case shown="True" "Cap 2 Samp Flow ON" {
              tunnel: w1307 -> [w1321 w1327]
              tunnel: w1306 -> [w1322 w1326]
              tunnel: [w1322 w1324] -> w1305
              tunnel: [w1321 w1323] -> w1304
              frame False {
              }
              frame True {
                # "run flow"
                n835 = Concatenate Strings("run" ("string"), "\r") -> (w1328:string)
                n836 = VISA Write(VISA resource name=w1326, write buffer=w1328, error in (no error)=w1327) -> (VISA resource name out=w1324:refnum<visa-resource-name>, error out=w1323:errorcluster)  [unwired: 1 out]
              }
            }
            n837 = Array Subset(array=w1319, index (row)=1 ("index"), length (row)=1 ("length"), index (col)=1 ("index"), length (col)=3 ("length")) -> (w1316:dbl[][])
            n838 = Reshape Array(w1316, 3 ("dimension size")) -> (w1314:dbl[])
            n839 = Array To Cluster(array=w1314) -> (cluster=w1313:cluster{"[0]":dbl, "[1]":dbl, "[2]":dbl})
            n840 = call "Set Stage Position.vi"("Position"=w1313, "error in"=w1308, "VISA resource name in"=w1309) -> ("error out"=w1312:errorcluster)  [unwired: 2 out]
            n841 = local write "Stage Moving"(TRUE ("Stage Moving")) -> ()
            n842 = local write "Stage Control Serial Error"(w1312) -> ()
          }
          frame #1 {
            n843 = local write "Stage Moving"(FALSE ("Stage Moving")) -> ()
            n844 = case shown="True" TRUE {
              tunnel: "Cap 2 T ON" -> [w1344 w1345]
              frame False {
                n845 = property on="Trap 2 (ON/OFF)" class="Bool (strict)"("Val(Sgnl)"=w1344) -> ()  [unwired: 2 in, 2 out]
              }
              frame True {
                n846 = property on="Trap 1 (ON/OFF)" class="Bool (strict)"("Val(Sgnl)"=w1345) -> ()  [unwired: 2 in, 2 out]
              }
            }
            n847 = call <vilib>:"Beep.vi"() -> ()  [unwired: 3 in, 9 out]
            n848 = case shown="True" w1330 {
              tunnel: w1332 -> [_ w1339]
              tunnel: w1331 -> [_ w1338]
              frame False {
              }
              frame True {
                n849 = Concatenate Strings("stop" ("string"), "\r") -> (w1341:string)
                n850 = VISA Write(VISA resource name=w1339, write buffer=w1341, error in (no error)=w1338) -> ()  [unwired: 3 out]
                n851 = local write "Sample Channel Flow"(FALSE ("Sample Channel Flow")) -> ()
              }
            }
            n852 = case shown="True" "Cap 2 Flow ON" {
              frame False {
              }
              frame True {
                n853 = property on="Inject Pump 3" class="Bool (strict)"("Val(Sgnl)"=TRUE ("Value (Signaling)")) -> ()  [unwired: 2 in, 2 out]
              }
            }
          }
        }
      }
      event "+z", "-z": Value Change {
        n854 = event-data() -> ()  [unwired: 1 in, 5 out]
        n855 = flat-sequence {
          tunnel: w1346 -> [w1368]
          tunnel: w1347 -> [w1348]
          frame #0 {
            n856 = call "Read Stage Position.vi"("error in"=w1368, "VISA resource name in"=w1348) -> ("Current Position"=w1353:cluster{dbl, dbl, dbl}, "error out"=w1366:errorcluster, "VISA resource name out"=w1367:refnum<visa-resource-name>)  [unwired: 1 out]
            n857 = local read "Saved Stage Positions"() -> (w1377:dbl[][])
            n858 = Divide(x="z nudge increment (um)", y=1000.0) -> (x/y=w1365:dbl)
            n859 = Boolean To (0,1)(Boolean="+z") -> (0, 1=w1357:i16)
            n860 = Boolean To (0,1)(Boolean="-z") -> (0, 1=w1358:i16)
            n861 = Array Subset(array=w1377, index (row)=1 ("index"), length (row)=1 ("length"), index (col)=1 ("index"), length (col)=3 ("length")) -> (w1374:dbl[][])
            n862 = Multiply(x=w1357, y=w1365) -> (x*y=w1361:dbl)
            n863 = Multiply(x=w1358, y=w1365) -> (x*y=w1359:dbl)
            n864 = Unbundle(w1353) -> (w1351:dbl, w1350:dbl, w1354:dbl)
            n865 = Negate(x=w1359) -> (-x=w1360:dbl)
            n866 = Reshape Array(w1374, 3 ("dimension size")) -> (w1372:dbl[])
            n867 = Add(x=w1361, y=w1360) -> (x+y=w1362:dbl)
            n868 = Array To Cluster(array=w1372) -> ()  [unwired: 1 out]
            n869 = Add(x=w1362, y=w1354) -> (x+y=w1352:dbl)
            n870 = Bundle(cluster=w1353, w1351, w1350, w1352) -> (w1349:cluster{dbl, dbl, dbl})
            n871 = call "Set Stage Position.vi"("Position"=w1349, "error in"=w1366, "VISA resource name in"=w1367) -> ("error out"=w1371:errorcluster)  [unwired: 2 out]
            n872 = local write "Stage Moving"(TRUE ("Stage Moving")) -> ()
            n873 = local write "Stage Control Serial Error"(w1371) -> ()
          }
          frame #1 {
            n874 = local write "Stage Moving"(FALSE ("Stage Moving")) -> ()
            n875 = call <vilib>:"Beep.vi"() -> ()  [unwired: 3 in, 9 out]
          }
        }
      }
      event "Cal/Data Acq. Spot": Value Change {
        n876 = event-data() -> ()  [unwired: 1 in, 5 out]
        n877 = flat-sequence {
          tunnel: w1383 -> [w1386]
          tunnel: w1382 -> [w1385]
          tunnel: ["Cal @ (MHz)"] -> w1380
          tunnel: w1380 -> [w1406]
          tunnel: w1380 -> [w1427]
          frame #0 {
            n878 = local read "Saved Stage Positions"() -> (w1389:dbl[][])
            n879 = Array Subset(array=w1389, index (row)=2 ("index"), length (row)=1 ("length"), index (col)=1 ("index"), length (col)=3 ("length")) -> (w1392:dbl[][])
            n880 = Reshape Array(w1392, 3 ("dimension size")) -> (w1394:dbl[])
            n881 = local write "Stage Moving"(TRUE ("Stage Moving")) -> ()
            n882 = Array To Cluster(array=w1394) -> (cluster=w1395:cluster{"[0]":dbl, "[1]":dbl, "[2]":dbl})
            n883 = call "Set Stage Position.vi"("Position"=w1395, "error in"=w1385, "VISA resource name in"=w1386) -> ("error out"=w1396:errorcluster)  [unwired: 2 out]
            n884 = local write "Stage Control Serial Error"(w1396) -> ()
          }
          frame #1 {
            n885 = property on="Trap Delta (MHz)" class="DigNum (strict)"("Val(Sgnl)"="Cal @ (MHz)") -> ()  [unwired: 2 in, 2 out]
            n886 = local write "Stage Moving"(FALSE ("Stage Moving")) -> ()
            n887 = call <vilib>:"Beep.vi"() -> ()  [unwired: 3 in, 9 out]
          }
          frame #2 {
            n888 = Wait (ms)(milliseconds to wait=u32 100) -> ()  [unwired: 1 out]
          }
          frame #3 {
            n889 = property on="Save Calibration" class="Bool (strict)"("Val(Sgnl)"=TRUE ("Value (Signaling)")) -> ()  [unwired: 2 in, 2 out]
          }
          frame #4 {
            n890 = Wait (ms)(milliseconds to wait=u32 4000) -> ()  [unwired: 1 out]
          }
          frame #5 {
            n891 = while {
              stop <- w1403 stop-if-true
              n892 = local read "Saving..."() -> (w1404:bool)
              n893 = Wait (ms)(milliseconds to wait=u32 100) -> ()  [unwired: 1 out]
              n894 = Not(x=w1404) -> (.not. x?=w1403:bool)
            }
          }
          frame #6 {
            n895 = case shown="True" "W/ Offset 1" {
              tunnel: w1406 -> [_ w1408]
              frame False {
              }
              frame True {
                n896 = stacked-sequence {
                  tunnel: w1408 -> [_ _ _ _ _ _ _ w1425]
                  frame #0 {
                    n897 = property on="Trap Delta (MHz)" class="DigNum (strict)"("Val(Sgnl)"="Offset 1 Start (MHz)") -> ()  [unwired: 2 in, 2 out]
                    n898 = Replace Array Subset(array=u32[] [0] ("Index Values"), new element="Offset 1 Set", index=0) -> (w1409:u32[])
                    n899 = property on="Saved AOD Raster Scan Parameter Sets" class="Arr (strict)"("Index Values"=w1409) -> ()  [unwired: 2 in, 2 out]
                  }
                  frame #1 {
                    n900 = Wait (ms)(milliseconds to wait=u32 200) -> ()  [unwired: 1 out]
                  }
                  frame #2 {
                    n901 = property on="Load parameters" class="Bool (strict)"("Val(Sgnl)"=TRUE ("Value (Signaling)")) -> ()  [unwired: 2 in, 2 out]
                  }
                  frame #3 {
                    n902 = Wait (ms)(milliseconds to wait=u32 200) -> ()  [unwired: 1 out]
                  }
                  frame #4 {
                    n903 = property on="Trap Raster Scan" class="Bool (strict)"("Val(Sgnl)"=TRUE ("Value (Signaling)")) -> ()  [unwired: 2 in, 2 out]
                  }
                  frame #5 {
                    n904 = Wait (ms)(milliseconds to wait=u32 2000) -> ()  [unwired: 1 out]
                  }
                  frame #6 {
                    n905 = while {
                      stop <- w1422 stop-if-true
                      n906 = local read "Raster Scanning..."() -> (w1424:bool)
                      n907 = local read "Saving..."() -> (w1420:bool)
                      n908 = Wait (ms)(milliseconds to wait=u32 100) -> ()  [unwired: 1 out]
                      n909 = Not(x=w1420) -> (.not. x?=w1419:bool)
                      n910 = Not(x=w1424) -> (.not. x?=w1421:bool)
                      n911 = And(x=w1421, y=w1419) -> (x .and. y?=w1422:bool)
                    }
                  }
                  frame #7 {
                    n912 = property on="Trap Delta (MHz)" class="DigNum (strict)"("Val(Sgnl)"=w1425) -> ()  [unwired: 2 in, 2 out]
                  }
                }
              }
            }
          }
          frame #7 {
            n913 = local read "Save ave N"() -> (w1426:dbl)
            n914 = case shown="True" "W/ Offset 2" {
              tunnel: w1427 -> [_ w1433]
              tunnel: w1426 -> [_ w1432]
              frame False {
                n915 = Multiply(x="Cal read wait (s)", y=u32 1000 ("milliseconds to wait")) -> (x*y=w1430:u32)
                n916 = Wait (ms)(milliseconds to wait=w1430) -> ()  [unwired: 1 out]
              }
              frame True {
                n917 = stacked-sequence {
                  tunnel: w1433 -> [_ _ _ _ _ _ _ _ _ w1454 _ _]
                  tunnel: w1432 -> [_ _ _ _ _ _ _ _ _ w1452 _ _]
                  frame #0 {
                    n918 = property on="Save ave N" class="DigNum (strict)"("Val(Sgnl)"=1.0 ("Value (Signaling)")) -> ()  [unwired: 2 in, 2 out]
                  }
                  frame #1 {
                    n919 = Wait (ms)(milliseconds to wait=u32 500) -> ()  [unwired: 1 out]
                  }
                  frame #2 {
                    n920 = property on="Trap Delta (MHz)" class="DigNum (strict)"("Val(Sgnl)"="Offset 2 Start (MHz)") -> ()  [unwired: 2 in, 2 out]
                    n921 = Replace Array Subset(array=u32[] [0] ("Index Values"), new element="Offset 2 Set", index=0) -> (w1438:u32[])
                    n922 = property on="Saved AOD Raster Scan Parameter Sets" class="Arr (strict)"("Index Values"=w1438) -> ()  [unwired: 2 in, 2 out]
                  }
                  frame #3 {
                    n923 = Wait (ms)(milliseconds to wait=u32 500) -> ()  [unwired: 1 out]
                  }
                  frame #4 {
                    n924 = property on="Load parameters" class="Bool (strict)"("Val(Sgnl)"=TRUE ("Value (Signaling)")) -> ()  [unwired: 2 in, 2 out]
                  }
                  frame #5 {
                    n925 = Wait (ms)(milliseconds to wait=u32 500) -> ()  [unwired: 1 out]
                  }
                  frame #6 {
                    n926 = property on="Trap Raster Scan" class="Bool (strict)"("Val(Sgnl)"=TRUE ("Value (Signaling)")) -> ()  [unwired: 2 in, 2 out]
                  }
                  frame #7 {
                    n927 = Wait (ms)(milliseconds to wait=u32 2000) -> ()  [unwired: 1 out]
                  }
                  frame #8 {
                    n928 = while {
                      stop <- w1447 stop-if-true
                      n929 = local read "Raster Scanning..."() -> (w1450:bool)
                      n930 = local read "Saving..."() -> (w1448:bool)
                      n931 = Wait (ms)(milliseconds to wait=u32 100) -> ()  [unwired: 1 out]
                      n932 = Not(x=w1448) -> (.not. x?=w1446:bool)
                      n933 = Not(x=w1450) -> (.not. x?=w1449:bool)
                      n934 = And(x=w1449, y=w1446) -> (x .and. y?=w1447:bool)
                    }
                  }
                  frame #9 {
                    n935 = property on="Trap Delta (MHz)" class="DigNum (strict)"("Val(Sgnl)"=w1454) -> ()  [unwired: 2 in, 2 out]
                    n936 = property on="Saved AOD Raster Scan Parameter Sets" class="Arr (strict)"("Index Values"=u32[] [0]) -> ()  [unwired: 2 in, 2 out]
                    n937 = property on="Save ave N" class="DigNum (strict)"("Val(Sgnl)"=w1452) -> ()  [unwired: 2 in, 2 out]
                  }
                  frame #10 {
                    n938 = Wait (ms)(milliseconds to wait=u32 500) -> ()  [unwired: 1 out]
                  }
                  frame #11 {
                    n939 = property on="Load parameters" class="Bool (strict)"("Val(Sgnl)"=TRUE ("Value (Signaling)")) -> ()  [unwired: 2 in, 2 out]
                  }
                }
              }
            }
          }
          frame #8 {
            n940 = property on="Read Cal" class="Bool (strict)"("Val(Sgnl)"=TRUE ("Value (Signaling)")) -> ()  [unwired: 2 in, 2 out]
          }
          frame #9 {
            n941 = Wait (ms)(milliseconds to wait=u32 500) -> ()  [unwired: 1 out]
          }
          frame #10 {
            n942 = property on="Fish for Tether" class="Bool (strict)"("Val(Sgnl)"=TRUE ("Value (Signaling)")) -> ()  [unwired: 2 in, 2 out]
          }
        }
        n943 = local write "Cal/Data Acq. Spot"(FALSE ("Cal/Data Acq. Spot")) -> ()
      }
      event "Dump Beads": Value Change {
        n944 = event-data() -> ()  [unwired: 1 in, 5 out]
        n945 = flat-sequence {
          tunnel: w1461 -> [w1467]
          tunnel: w1460 -> [w1466]
          frame #0 {
            w1463 = FALSE ("Fl. Triggered...")
            w1464 = TRUE ("Stage Moving")
            n946 = local read "Saving..."() -> (w1465:bool)
            n947 = local write "Fl. Triggered..."(w1463) -> ()
            n948 = local write "Stage Moving"(w1464) -> ()
            n949 = local write "Tether"(w1463) -> ()
            n950 = property on="Green Laser ON/Interlacing" class="Bool (strict)"("Val(Sgnl)"=w1463) -> ()  [unwired: 2 in, 2 out]
            n951 = property on="Trap Pos. FB ON" class="Bool (strict)"("Val(Sgnl)"=w1463) -> ()  [unwired: 2 in, 2 out]
            n952 = property on="Trap Triggering" class="Bool (strict)"("Val(Sgnl)"=w1463) -> ()  [unwired: 2 in, 2 out]
            n953 = local write "Stop Saving"(w1465) -> ()
            n954 = property on="Sample Channel Flow" class="Bool (strict)"("Val(Sgnl)"=w1464) -> ()  [unwired: 2 in, 2 out]
          }
          frame #1 {
            n955 = local read "Saved Stage Positions"() -> (w1468:dbl[][])
            n956 = Array Subset(array=w1468, index (row)=3 ("index"), length (row)=1 ("length"), index (col)=1 ("index"), length (col)=3 ("length")) -> (w1473:dbl[][])
            n957 = Reshape Array(w1473, 3 ("dimension size")) -> (w1471:dbl[])
            n958 = Array To Cluster(array=w1471) -> (cluster=w1470:cluster{"[0]":dbl, "[1]":dbl, "[2]":dbl})
            n959 = call "Set Stage Position.vi"("Position"=w1470, "error in"=w1466, "VISA resource name in"=w1467) -> ()  [unwired: 3 out]
          }
          frame #2 {
            w1477 = FALSE ("Value (Signaling)")
            n960 = property on="Trap 1 (ON/OFF)" class="Bool (strict)"("Val(Sgnl)"=w1477) -> ()  [unwired: 2 in, 2 out]
            n961 = property on="Trap 2 (ON/OFF)" class="Bool (strict)"("Val(Sgnl)"=w1477) -> ()  [unwired: 2 in, 2 out]
            n962 = call <vilib>:"Beep.vi"() -> ()  [unwired: 3 in, 9 out]
          }
          frame #3 {
            n963 = property on="Move Cap. 2 (ADig Left)" class="Bool (strict)"("Val(Sgnl)"=TRUE ("Value (Signaling)")) -> ()  [unwired: 2 in, 2 out]
            n964 = property on="Tab Control" class="TabCtl (strict)"("Val(Sgnl)"=T4."Status" ("Value (Signaling)")) -> ()  [unwired: 2 in, 2 out]
          }
        }
      }
      event "Dip for Protein": Value Change {
        n965 = event-data() -> ()  [unwired: 1 in, 5 out]
        n966 = flat-sequence {
          tunnel: w1486 -> [w1490]
          tunnel: w1487 -> [w1491]
          tunnel: [w1491] -> w1481
          tunnel: [w1490] -> w1480
          tunnel: [w1494] -> w1484
          tunnel: [w1493] -> w1482
          tunnel: w1481 -> [w1497]
          tunnel: w1480 -> [w1496]
          tunnel: [w1507] -> w1485
          tunnel: w1484 -> [w1507]
          tunnel: [w1506] -> w1483
          tunnel: w1482 -> [w1506]
          tunnel: w1485 -> [w1512]
          tunnel: w1483 -> [w1511]
          frame #0 {
            n967 = case shown="True" "Move Trap Before?" {
              frame False {
              }
              frame True {
                n968 = property on="Trap Delta (MHz)" class="DigNum (strict)"("Val(Sgnl)"="Dip Trap Delta 1 (MHz)") -> ()  [unwired: 2 in, 2 out]
              }
            }
          }
          frame #1 {
            n969 = local read "Saved Stage Positions"() -> (w1495:dbl[][])
            n970 = Array Subset(array=w1495, index (row)=4 ("index"), length (row)=1 ("length"), index (col)=1 ("index"), length (col)=3 ("length")) -> (w1502:dbl[][])
            n971 = Reshape Array(w1502, 3 ("dimension size")) -> (w1500:dbl[])
            n972 = Array To Cluster(array=w1500) -> (cluster=w1499:cluster{"[0]":dbl, "[1]":dbl, "[2]":dbl})
            n973 = call "Set Stage Position.vi"("Position"=w1499, "error in"=w1496, "VISA resource name in"=w1497) -> ("error out"=w1493:errorcluster, "VISA resource name out"=w1494:refnum<visa-resource-name>)  [unwired: 1 out]
          }
          frame #2 {
            n974 = Multiply(x="Duration (s)", y=1000.0) -> (x*y=w1508:dbl)
            n975 = Wait (ms)(milliseconds to wait=w1508) -> ()  [unwired: 1 out]
          }
          frame #3 {
            n976 = local read "Saved Stage Positions"() -> (w1513:dbl[][])
            n977 = Array Subset(array=w1513, index (row)=2 ("index"), length (row)=1 ("length"), index (col)=1 ("index"), length (col)=3 ("length")) -> (w1518:dbl[][])
            n978 = Reshape Array(w1518, 3 ("dimension size")) -> (w1516:dbl[])
            n979 = Array To Cluster(array=w1516) -> (cluster=w1515:cluster{"[0]":dbl, "[1]":dbl, "[2]":dbl})
            n980 = call "Set Stage Position.vi"("Position"=w1515, "error in"=w1511, "VISA resource name in"=w1512) -> ()  [unwired: 3 out]
          }
          frame #4 {
            n981 = case shown="True" "Move Trap After?" {
              frame False {
              }
              frame True {
                n982 = property on="Trap Delta (MHz)" class="DigNum (strict)"("Val(Sgnl)"="Dip Trap Delta 2 (MHz)") -> ()  [unwired: 2 in, 2 out]
              }
            }
          }
          frame #5 {
            n983 = case shown="True" "Green ON After?" {
              frame False {
              }
              frame True {
                n984 = property on="Green Laser ON/Interlacing" class="Bool (strict)"("Val(Sgnl)"=TRUE ("Value (Signaling)")) -> ()  [unwired: 2 in, 2 out]
              }
            }
          }
          frame #6 {
            n985 = Wait (ms)(milliseconds to wait=u32 500) -> ()  [unwired: 1 out]
          }
          frame #7 {
            n986 = case shown="True" "Save Data After?" {
              frame False {
              }
              frame True {
                n987 = property on="Start Saving" class="Bool (strict)"("Val(Sgnl)"=TRUE ("Value (Signaling)")) -> ()  [unwired: 2 in, 2 out]
              }
            }
          }
        }
      }
      event "Profile": Value Change {
        n988 = event-data() -> ()  [unwired: 1 in, 5 out]
        n989 = flat-sequence {
          tunnel: w1537 -> [w1540]
          tunnel: w1536 -> [w1548]
          tunnel: [w1542] -> w1535
          tunnel: [w1541] -> w1534
          tunnel: [w1539] -> w1532
          tunnel: [w1538] -> w1529
          tunnel: w1535 -> [w1555]
          tunnel: w1534 -> [w1554]
          tunnel: [w1552] -> w1533
          tunnel: w1532 -> [w1553]
          tunnel: [w1551] -> w1531
          tunnel: [w1550] -> w1530
          tunnel: w1529 -> [w1550]
          tunnel: w1533 -> [w1559]
          tunnel: w1531 -> [w1558]
          tunnel: w1530 -> [w1557]
          frame #0 {
            n990 = call "Read Stage Position.vi"("error in"=w1548, "VISA resource name in"=w1540) -> ("Current Position"=w1538:cluster{dbl, dbl, dbl}, "error out"=w1541:errorcluster, "VISA resource name out"=w1539:refnum<visa-resource-name>)  [unwired: 1 out]
            "Current Position" <- w1538
            n991 = local write "Stage Control Serial Error"(w1541) -> ()
            n992 = Unbundle(w1538) -> (w1545:dbl, w1547:dbl, w1543:dbl)
            n993 = Add(x=w1547, y="Y change (mm)") -> (x+y=w1544:dbl)
            n994 = Bundle(w1545, w1544, w1543) -> (w1542:cluster{dbl, dbl, dbl})  [unwired: 1 in]
          }
          frame #1 {
            # "move to new position and start saving"
            n995 = local write "Stage Moving"(TRUE ("Stage Moving")) -> ()
            n996 = local write "Start Saving"(TRUE ("Start Saving")) -> ()
            n997 = call "Set Stage Position.vi"("Position"=w1555, "error in"=w1554, "VISA resource name in"=w1553) -> ("error out"=w1551:errorcluster, "VISA resource name out"=w1552:refnum<visa-resource-name>)  [unwired: 1 out]
          }
          frame #2 {
            # "go back to start"
            n998 = call "Set Stage Position.vi"("Position"=w1557, "error in"=w1558, "VISA resource name in"=w1559) -> ()  [unwired: 3 out]
          }
          frame #3 {
            # "stop saving"
            n999 = local write "Stop Saving"(TRUE ("Stop Saving")) -> ()
            n1000 = local write "Stage Moving"(FALSE ("Stage Moving")) -> ()
          }
        }
      }
      event "Move to Position 1", "Move to Position 2", "Move to Position 3", "Move to Position 4", "Move to Position 5", "Lower Ch. Cap.": Value Change {
        n1001 = event-data() -> ()  [unwired: 1 in, 5 out]
        n1002 = Or(x="Move to Position 5", y="Lower Ch. Cap.") -> (x .or. y?=w1565:bool)
        n1003 = Build Array("Move to Position 1", "Move to Position 2", "Move to Position 3", "Move to Position 4", w1565) -> (w1568:bool[])
        n1004 = Boolean Array To Number(Boolean array=w1568) -> (number=w1567:u32)
        n1005 = Logarithm Base 2(1:w1567) -> (0:w1566:dbl)
        n1006 = flat-sequence {
          tunnel: w1566 -> [w1577]
          tunnel: w1563 -> [w1575]
          tunnel: w1562 -> [w1574]
          frame #0 {
            n1007 = local read "Saved Stage Positions"() -> (w1585:dbl[][])
            n1008 = Array Subset(array=w1585, index (row)=w1577, length (row)=1 ("length"), index (col)=1 ("index"), length (col)=3 ("length")) -> (w1582:dbl[][])
            n1009 = Reshape Array(w1582, 3 ("dimension size")) -> (w1580:dbl[])
            n1010 = Array To Cluster(array=w1580) -> (cluster=w1579:cluster{"[0]":dbl, "[1]":dbl, "[2]":dbl})
            n1011 = call "Set Stage Position.vi"("Position"=w1579, "error in"=w1574, "VISA resource name in"=w1575) -> ("error out"=w1578:errorcluster)  [unwired: 2 out]
            n1012 = local write "Stage Moving"(TRUE ("Stage Moving")) -> ()
            n1013 = local write "Stage Control Serial Error"(w1578) -> ()
          }
          frame #1 {
            n1014 = local write "Stage Moving"(FALSE ("Stage Moving")) -> ()
            n1015 = call <vilib>:"Beep.vi"() -> ()  [unwired: 3 in, 9 out]
          }
        }
      }
      event "Got ADig bead": Value Change {
        n1016 = event-data() -> ()  [unwired: 1 in, 5 out]
        n1017 = property on="Move Cap. 1 (DNA Right)" class="Bool (strict)"("Val(Sgnl)"=TRUE ("Value (Signaling)")) -> ()  [unwired: 2 in, 2 out]
        n1018 = property on="Inject Pump 3" class="Bool (strict)"("Val(Sgnl)"=FALSE ("Value (Signaling)")) -> ()  [unwired: 2 in, 2 out]
      }
      event "Take Force FB Data\nUpper Channel": Value Change {
        n1019 = event-data() -> ()  [unwired: 1 in, 5 out]
        n1020 = flat-sequence {
          tunnel: w1592 -> [w1598]
          tunnel: w1591 -> [w1597]
          frame #0 {
            n1021 = local read "Saved Stage Positions"() -> (w1601:dbl[][])
            n1022 = local write "Stage Moving"(TRUE ("Stage Moving")) -> ()
            n1023 = Array Subset(array=w1601, index (row)=4 ("index"), length (row)=1 ("length"), index (col)=1 ("index"), length (col)=3 ("length")) -> (w1606:dbl[][])
            n1024 = Reshape Array(w1606, 3 ("dimension size")) -> (w1604:dbl[])
            n1025 = Array To Cluster(array=w1604) -> (cluster=w1599:cluster{"[0]":dbl, "[1]":dbl, "[2]":dbl})
            n1026 = call "Set Stage Position.vi"("Position"=w1599, "error in"=w1597, "VISA resource name in"=w1598) -> ("error out"=w1596:errorcluster)  [unwired: 2 out]
            n1027 = property on="Trap Pos. FB Offset Factor" class="DigNum (strict)"("Val(Sgnl)"=i64 0 ("Value (Signaling)")) -> ()  [unwired: 2 in, 2 out]
            n1028 = local write "Stage Control Serial Error"(w1596) -> ()
            n1029 = local write "FB Trap Pos Offset"(0.0 ("FB Trap Pos Offset")) -> ()
          }
          frame #1 {
            n1030 = call <vilib>:"Beep.vi"() -> ()  [unwired: 3 in, 9 out]
            n1031 = property on="Trap Delta (MHz)" class="DigNum (strict)"("Val(Sgnl)"="Starting \nTrap Delta (MHz)") -> ()  [unwired: 2 in, 2 out]
            n1032 = local write "Stage Moving"(FALSE ("Stage Moving")) -> ()
            n1033 = Wait (ms)(milliseconds to wait=u32 1000) -> ()  [unwired: 1 out]
          }
          frame #2 {
            n1034 = property on="Set SP to Reading" class="Bool (strict)"("Val(Sgnl)"=TRUE ("Value (Signaling)")) -> ()  [unwired: 2 in, 2 out]
            n1035 = Wait (ms)(milliseconds to wait=u32 500) -> ()  [unwired: 1 out]
          }
          frame #3 {
            n1036 = local read "Mean T1 Position (nm)"() -> (w1615:dbl)
            n1037 = property on="Trap Pos. FB ON" class="Bool (strict)"("Val(Sgnl)"=TRUE ("Value (Signaling)")) -> ()  [unwired: 2 in, 2 out]
            n1038 = Wait (ms)(milliseconds to wait=u32 250) -> ()  [unwired: 1 out]
            n1039 = Negate(x=w1615) -> (-x=w1614:dbl)
            n1040 = local write "FB Trap Pos Offset"(w1614) -> ()
          }
          frame #4 {
            n1041 = property on="Remove Action Offset" class="Bool (strict)"("Val(Sgnl)"=TRUE ("Value (Signaling)")) -> ()  [unwired: 2 in, 2 out]
            n1042 = Wait (ms)(milliseconds to wait=u32 250) -> ()  [unwired: 1 out]
          }
          frame #5 {
            n1043 = local read "Trap Pos. FB Mult Factor"() -> (w1620:i64)
            n1044 = local read "Trap Pos. FB Offset Factor"() -> (w1628:i64)
            n1045 = Multiply(x=32768, y="factor") -> (x*y=w1625:dbl)
            n1046 = Multiply(x=w1625, y=w1620) -> (x*y=w1621:dbl)
            n1047 = Subtract(x=w1628, y=w1621) -> (x-y=w1624:dbl)
            n1048 = To Quad Integer(1:w1624) -> (0:w1623:i64)
            n1049 = property on="Trap Pos. FB Offset Factor" class="DigNum (strict)"("Val(Sgnl)"=w1623) -> ()  [unwired: 2 in, 2 out]
            n1050 = Wait (ms)(milliseconds to wait=u32 250) -> ()  [unwired: 1 out]
          }
          frame #6 {
            n1051 = case shown="True" "Trap Trig Fl." {
              frame False {
                n1052 = property on="Green Laser ON/Interlacing" class="Bool (strict)"("Val(Sgnl)"=TRUE ("Value (Signaling)")) -> ()  [unwired: 2 in, 2 out]
              }
              frame True {
                n1053 = property on="Trap Triggering" class="Bool (strict)"("Val(Sgnl)"=TRUE ("Value (Signaling)")) -> ()  [unwired: 2 in, 2 out]
              }
            }
            n1054 = Wait (ms)(milliseconds to wait=u32 500) -> ()  [unwired: 1 out]
          }
          frame #7 {
            n1055 = property on="Start Saving" class="Bool (strict)"("Val(Sgnl)"=TRUE ("Value (Signaling)")) -> ()  [unwired: 2 in, 2 out]
            n1056 = property on="Tab Control" class="TabCtl (strict)"("Val(Sgnl)"=T4."Trap Control (RF)" ("Value (Signaling)")) -> ()  [unwired: 2 in, 2 out]
            n1057 = property on="Tab Control 2" class="TabCtl (strict)"("Val(Sgnl)"=T6."Feedback on Trap Position" ("Value (Signaling)")) -> ()  [unwired: 2 in, 2 out]
          }
        }
      }
      event "Got DNA bead": Value Change {
        n1058 = event-data() -> ()  [unwired: 1 in, 5 out]
        n1059 = property on="Cal/Data Acq. Spot" class="Bool (strict)"("Val(Sgnl)"=TRUE ("Value (Signaling)")) -> ()  [unwired: 2 in, 2 out]
        n1060 = property on="Inject Pump 1" class="Bool (strict)"("Val(Sgnl)"=FALSE ("Value (Signaling)")) -> ()  [unwired: 2 in, 2 out]
      }
      event "Take Stepping Data": Value Change {
        n1061 = event-data() -> ()  [unwired: 1 in, 5 out]
        n1062 = local read "Save ave N"() -> (w1647:dbl)
        n1063 = flat-sequence {
          tunnel: w1647 -> [w1649]
          tunnel: [w1649] -> w1642
          tunnel: [w1651] -> w1643
          tunnel: w1642 -> [w1651]
          tunnel: [w1653] -> w1644
          tunnel: w1643 -> [w1653]
          tunnel: [w1656] -> w1645
          tunnel: w1644 -> [w1656]
          tunnel: [w1658] -> w1646
          tunnel: w1645 -> [w1658]
          tunnel: [w1660] -> w1640
          tunnel: w1646 -> [w1660]
          tunnel: w1640 -> [w1663]
          tunnel: [w1663] -> w1639
          tunnel: w1639 -> [w1664]
          tunnel: [w1664] -> w1641
          tunnel: w1641 -> [w1670]
          frame #0 {
            n1064 = property on="Save ave N" class="DigNum (strict)"("Val(Sgnl)"="Save ave factor") -> ()  [unwired: 2 in, 2 out]
          }
          frame #1 {
            n1065 = Wait (ms)(milliseconds to wait=u32 100) -> ()  [unwired: 1 out]
          }
          frame #2 {
            n1066 = local read "Offset 2 Start (MHz)"() -> (w1655:dbl)
            n1067 = property on="Saved AOD Raster Scan Parameter Sets" class="Arr (strict)"("Index Values"=u32[] [2]) -> ()  [unwired: 2 in, 2 out]
            n1068 = property on="Trap Delta (MHz)" class="DigNum (strict)"("Val(Sgnl)"=w1655) -> ()  [unwired: 2 in, 2 out]
          }
          frame #3 {
            n1069 = property on="Load parameters" class="Bool (strict)"("Val(Sgnl)"=TRUE ("Value (Signaling)")) -> ()  [unwired: 2 in, 2 out]
          }
          frame #4 {
            n1070 = Wait (ms)(milliseconds to wait=u32 100) -> ()  [unwired: 1 out]
          }
          frame #5 {
            n1071 = property on="Trap Raster Scan" class="Bool (strict)"("Val(Sgnl)"=TRUE ("Value (Signaling)")) -> ()  [unwired: 2 in, 2 out]
          }
          frame #6 {
            n1072 = Wait (ms)(milliseconds to wait=u32 1000) -> ()  [unwired: 1 out]
          }
          frame #7 {
            n1073 = while {
              stop <- w1667 stop-if-true
              n1074 = local read "Raster Scanning..."() -> (w1669:bool)
              n1075 = local read "Saving..."() -> (w1668:bool)
              n1076 = Not(x=w1668) -> (.not. x?=w1665:bool)
              n1077 = Not(x=w1669) -> (.not. x?=w1666:bool)
              n1078 = And(x=w1666, y=w1665) -> (x .and. y?=w1667:bool)
            }
          }
          frame #8 {
            n1079 = property on="Save ave N" class="DigNum (strict)"("Val(Sgnl)"=w1670) -> ()  [unwired: 2 in, 2 out]
          }
        }
      }
      event "Step Size (nm)": Value Change {
        n1080 = event-data() -> ()  [unwired: 1 in, 5 out]
        n1081 = flat-sequence {
          frame #0 {
            n1082 = property on="Saved AOD Raster Scan Parameter Sets" class="Arr (strict)"("Index Values"=u32[] [1]) -> ()  [unwired: 2 in, 2 out]
          }
          frame #1 {
            n1083 = Multiply(x="N Steps", y="Step Size (nm)") -> (x*y=w1672:dbl)
            n1084 = property on="Scan Speed AOD (nm/s) 2" class="DigNum (strict)"("Value"="Step Size (nm)") -> ()  [unwired: 2 in, 2 out]
            n1085 = property on="Step Size AOD (nm) 2" class="DigNum (strict)"("Value"="Step Size (nm)") -> ()  [unwired: 2 in, 2 out]
            n1086 = property on="Scan Range AOD (nm) 2" class="DigNum (strict)"("Value"=w1672) -> ()  [unwired: 2 in, 2 out]
          }
        }
      }
      event "Take Detection Laser\nImage": Value Change {
        n1087 = event-data() -> ()  [unwired: 1 in, 5 out]
        n1088 = flat-sequence {
          tunnel: [w1700] -> w1690
          tunnel: [w1699] -> w1683
          tunnel: [w1698] -> w1675
          tunnel: [w1703] -> w1691
          tunnel: w1690 -> [w1703]
          tunnel: [w1702] -> w1684
          tunnel: w1683 -> [w1702]
          tunnel: [w1701] -> w1676
          tunnel: w1675 -> [w1701]
          tunnel: [w1707] -> w1692
          tunnel: w1691 -> [w1707]
          tunnel: [w1706] -> w1685
          tunnel: w1684 -> [w1706]
          tunnel: [w1705] -> w1677
          tunnel: w1676 -> [w1705]
          tunnel: [w1713] -> w1693
          tunnel: w1692 -> [w1713]
          tunnel: [w1712] -> w1686
          tunnel: w1685 -> [w1712]
          tunnel: [w1711] -> w1678
          tunnel: w1677 -> [w1711]
          tunnel: [w1717] -> w1694
          tunnel: w1693 -> [w1717]
          tunnel: [w1716] -> w1687
          tunnel: w1686 -> [w1716]
          tunnel: [w1715] -> w1679
          tunnel: w1678 -> [w1715]
          tunnel: [w1721] -> w1695
          tunnel: w1694 -> [w1721]
          tunnel: [w1720] -> w1688
          tunnel: w1687 -> [w1720]
          tunnel: [w1719] -> w1680
          tunnel: w1679 -> [w1719]
          tunnel: [w1725] -> w1696
          tunnel: w1695 -> [w1725]
          tunnel: [w1724] -> w1689
          tunnel: w1688 -> [w1724]
          tunnel: [w1723] -> w1681
          tunnel: w1680 -> [w1723]
          tunnel: w1696 -> [w1731]
          tunnel: w1689 -> [w1730]
          tunnel: [w1728] -> w1682
          tunnel: w1681 -> [w1728]
          tunnel: w1682 -> [w1732]
          frame #0 {
            n1089 = local read "Green Laser ON/Interlacing"() -> (w1700:bool)
            n1090 = local read "Green laser mode"() -> (w1699:enum32{"Laser ON", "Laser OFF", "Interlace"})
            n1091 = local read "Green FB On/Off"() -> (w1698:bool)
          }
          frame #1 {
            n1092 = property on="Green FB On/Off" class="Bool (strict)"("Val(Sgnl)"=FALSE ("Value (Signaling)")) -> ()  [unwired: 2 in, 2 out]
          }
          frame #2 {
            n1093 = property on="Green Laser ON/Interlacing" class="Bool (strict)"("Val(Sgnl)"=TRUE ("Value (Signaling)")) -> ()  [unwired: 2 in, 2 out]
            n1094 = property on="Flip Green Filter" class="Bool (strict)"("Val(Sgnl)"=TRUE ("Value (Signaling)")) -> ()  [unwired: 2 in, 2 out]
            n1095 = property on="Green laser mode" class="RadioBtnsControl (strict)"("Val(Sgnl)"=enum32{"Laser ON", "Laser OFF", "Interlace"}."Laser ON" ("Value (Signaling)")) -> ()  [unwired: 2 in, 2 out]
          }
          frame #3 {
            n1096 = Wait (ms)(milliseconds to wait=u32 500) -> ()  [unwired: 1 out]
          }
          frame #4 {
            n1097 = property on="Confocal Image" class="Bool (strict)"("Val(Sgnl)"=TRUE ("Value (Signaling)")) -> ()  [unwired: 2 in, 2 out]
          }
          frame #5 {
            n1098 = Wait (ms)(milliseconds to wait=u32 2000) -> ()  [unwired: 1 out]
          }
          frame #6 {
            n1099 = while {
              stop <- w1726 stop-if-true
              n1100 = local read "Saving..."() -> (w1727:bool)
              n1101 = Not(x=w1727) -> (.not. x?=w1726:bool)
            }
          }
          frame #7 {
            n1102 = property on="Flip Green Filter" class="Bool (strict)"("Val(Sgnl)"=TRUE ("Value (Signaling)")) -> ()  [unwired: 2 in, 2 out]
            n1103 = property on="Green Laser ON/Interlacing" class="Bool (strict)"("Val(Sgnl)"=w1731) -> ()  [unwired: 2 in, 2 out]
            n1104 = property on="Green laser mode" class="RadioBtnsControl (strict)"("Val(Sgnl)"=w1730) -> ()  [unwired: 2 in, 2 out]
          }
          frame #8 {
            n1105 = property on="Green FB On/Off" class="Bool (strict)"("Val(Sgnl)"=w1732) -> ()  [unwired: 2 in, 2 out]
          }
        }
      }
      event "Stop All": Value Change {
        n1106 = event-data() -> ()  [unwired: 1 in, 5 out]
        n1107 = local read "Stop All"() -> (w1733:bool)
      }
    }
    n1108 = node-c288() -> ()  [unwired: 1 in, 1 out]
  }
  n1109 = node-c288(i64 1 ("Period"), 1 ("Processor")) -> (w161:T21)  [unwired: 2 out]
  n1110 = node-c288() -> (w80:T21)  [unwired: 4 out]
  n1111 = node-c288(3 ("Processor")) -> (w76:T21)  [unwired: 3 out]
  n1112 = timed-loop "Acquire Data" {
    tunnel: w36 -> [w1989]
    tunnel: w35 -> [w1988]
    tunnel: [w2019] -> w257
    tunnel: [w2013] -> w255
    timing: w161 -> [_]
    timing-out: [_] -> w160
    tunnel: w55 -> [w1814]
    stop <- "Stop All" stop-if-true
    w1799 = "NI_ChannelName" ("name")
    n1113 = node-c288() -> ()  [unwired: 2 out]
    n1114 = First Call?() -> (First Call?: T/F=w1764:bool)
    n1115 = Or(x="Reset", y=w1764) -> (x .or. y?=w1765:bool)
    n1116 = case "Reset data stream" shown="True" w1765 {
      tunnel: w1989 -> [w2852 w2860]
      tunnel: w1988 -> [w2851 w2859]
      tunnel: [w2852 w2854] -> w1984
      tunnel: [w2851 w2853] -> w1983
      frame False {
      }
      frame True {
        w2857 = TRUE ("AI to FIFO")
        n1117 = local write "Overflow (data lost)"(FALSE ("Overflow (data lost)")) -> ()
        n1118 = call "reset FPGA DMA.vi"("error in"=w2859, "FPGA VI Reference In"=w2860) -> ("error out"=w2855:errorcluster, "FPGA VI Reference Out"=w2856:T19)
        n1119 = xnode "Read/Write Control"("FPGA VI Reference In"=w2856, "error in"=w2855, "AI to FIFO"=w2857, "APD to FIFO"=w2857) -> ("FPGA VI Reference Out"=w2854:T19, "error out"=w2853:errorcluster)
      }
    }
    n1120 = Or(x="Start AOD Scan", y="Trap Raster Scan") -> (x .or. y?=w1934:bool)
    n1121 = case "Start AOM raster scan" shown="True" w1934 {
      tunnel: w1984 -> [w2702 w2712]
      tunnel: w1983 -> [w2701 w2711]
      tunnel: [w2702 w2705] -> w1982
      tunnel: [w2701 w2704] -> w1981
      frame False {
      }
      frame True {
        n1122 = case shown="True" "Restart DMA? (AOD)" {
          tunnel: [w2750 w2752] -> w2706
          tunnel: [w2749 w2751] -> w2707
          tunnel: w2712 -> [w2750 w2754]
          tunnel: w2711 -> [w2749 w2753]
          frame False {
          }
          frame True {
            n1123 = local write "Overflow (data lost)"(FALSE ("Overflow (data lost)")) -> ()
            n1124 = call "reset FPGA DMA.vi"("error in"=w2753, "FPGA VI Reference In"=w2754) -> ("error out"=w2751:errorcluster, "FPGA VI Reference Out"=w2752:T19)
          }
        }
        n1125 = local write "Trap Raster Scan"(FALSE ("Trap Raster Scan")) -> ()
        n1126 = case shown="True" "Move MCL Also?" {
          tunnel: w2707 -> [w2715 w2744]
          tunnel: w2706 -> [w2716 w2745]
          tunnel: [w2714 w2748] -> w2705
          tunnel: [w2713 w2747] -> w2704
          frame False {
            w2717 = TRUE ("AI to FIFO")
            n1127 = xnode "Read/Write Control"("FPGA VI Reference In"=w2716, "error in"=w2715, "AI to FIFO"=w2717, "APD to FIFO"=w2717, "Start scan"=w2717) -> ("FPGA VI Reference Out"=w2714:T19, "error out"=w2713:errorcluster)
          }
          frame True {
            w2741 = FALSE ("1D or 2D Scan?")
            w2746 = TRUE ("AI to FIFO")
            # "Count for MCL loop"
            # "N total cycles"
            # "N steps"
            # "V_int"
            n1128 = local read "Scan Range (nm)"() -> (w2723:dbl)
            n1129 = local read "Number of F/B Scans (AOD)"() -> (w2740:u16)
            n1130 = Sign(1:w2723) -> (0:w2722:dbl)
            n1131 = Compound Arithmetic op=MULTIPLY(w2723, "MCL Step Position Ratio", "MCL/AOM Scale Tweak") -> (w2727:dbl)
            n1132 = Negate(x=w2722) -> (-x=w2719:dbl)
            n1133 = Multiply(x=w2719, y="MCL Step Increment (V_int)") -> (x*y=w2721:dbl)
            n1134 = Divide(x=w2727, y="MCL X Cal (nm/V)") -> (x/y=w2733:dbl)
            n1135 = Multiply(x=32767.0 ("y"), y=w2733) -> (x*y=w2739:dbl)
            n1136 = local read "Total Counts (ticks)"() -> (w2724:u32)
            n1137 = local read "Cycles/step (AOD)"() -> (w2735:u64)
            n1138 = local read "Scan steps (AOD)"() -> (w2736:u64)
            n1139 = Divide(x=w2739, y=10.0) -> (x/y=w2732:dbl)
            n1140 = Divide(x=w2732, y="MCL Step Increment (V_int)") -> (x/y=w2730:dbl)
            n1141 = Absolute Value(x=w2730) -> (abs(x)=w2718:dbl)
            n1142 = Compound Arithmetic op=MULTIPLY(w2736, w2735, w2724) -> (w2731:u64)
            n1143 = local write "wait to reset values"(w2746) -> ()
            n1144 = local write "MCL Scanning"(w2746) -> ()
            n1145 = Divide(x=w2731, y=w2718) -> (x/y=w2728:dbl)
            "MCL Count" <- w2728
            n1146 = xnode "Read/Write Control"("FPGA VI Reference In"=w2745, "error in"=w2744, "Scan steps (MCL)"=w2718, "Number of scans (MCL)"=w2740, "Cycles per step (MCL)"=u64 1, "Scan freq.  increment (MCL)"=w2721, "1D or 2D Scan?"=w2741, "MCL Scan Axis"=w2741, "Cont. Scan (MCL)"=w2741, "MCL count"=w2728) -> ("FPGA VI Reference Out"=w2743:T19, "error out"=w2742:errorcluster)
            n1147 = xnode "Read/Write Control"("FPGA VI Reference In"=w2743, "error in"=w2742, "AI to FIFO"=w2746, "APD to FIFO"=w2746, "Start scan"=w2746, "Start scan (MCL)"=w2746) -> ("FPGA VI Reference Out"=w2748:T19, "error out"=w2747:errorcluster)
          }
        }
        "Raster Scanning..." <- TRUE ("Scanning...")
      }
    }
    n1148 = And(x="Save scans", y=w1934) -> (x .and. y?=w1980:bool)
    n1149 = Compound Arithmetic op=OR("Start MCL Scan", "Confocal Image", "Confocal Linescan") -> (w1932:bool)
    n1150 = And(x="Save Data (MCL)", y=w1932) -> (x .and. y?=w1979:bool)
    n1151 = case "Start MCL raster scan" shown="True" w1932 {
      tunnel: w1982 -> [w2320 w2335]
      tunnel: w1981 -> [w2319 w2334]
      tunnel: [w2320 w2330] -> w1812
      tunnel: [w2319 w2329] -> w1811
      tunnel: [FALSE w2328] -> w1965
      tunnel: "Start MCL Scan" -> [_ w2323]
      tunnel: "Confocal Image" -> [_ w2322]
      tunnel: "Confocal Linescan" -> [_ _]
      frame False {
      }
      frame True {
        w2328 = TRUE
        n1152 = case shown="True" "Restart DMA? (MCL)" {
          tunnel: [w2380 w2382] -> w2333
          tunnel: [w2379 w2381] -> w2332
          tunnel: w2335 -> [w2380 w2385]
          tunnel: w2334 -> [w2379 w2384]
          frame False {
          }
          frame True {
            n1153 = call "reset FPGA DMA.vi"("error in"=w2384, "FPGA VI Reference In"=w2385) -> ("error out"=w2381:errorcluster, "FPGA VI Reference Out"=w2382:T19)
            n1154 = local write "Overflow (data lost)"(FALSE ("Overflow (data lost)")) -> ()
          }
        }
        n1155 = case shown="False" w2323 {
          selector: w2323 -> [_ w2339]
          tunnel: w2322 -> [w2338 _]
          tunnel: [w2338 w2339] -> w2321
          frame False {
            n1156 = property on="2D or 1D Scan" class="Bool (strict)"("Val(Sgnl)"=w2338) -> ()  [unwired: 2 in, 2 out]
            n1157 = property on="Confocal Image" class="Bool (strict)"("Value"=FALSE ("Start Confocal Map")) -> ()  [unwired: 2 in, 2 out]
          }
          frame True {
          }
        }
        n1158 = local write "MCL Scanning"(w2328) -> ()
        n1159 = local read "AO1"() -> (w2325:dbl)
        n1160 = local read "AO2"() -> (w2324:dbl)
        n1161 = case shown="True" "Center Scan" {
          tunnel: w2333 -> [w2346 w2378]
          tunnel: w2332 -> [w2345 w2377]
          tunnel: [w2344 w2376] -> w2330
          tunnel: [w2343 w2375] -> w2329
          tunnel: [w2341 w2362] -> w2327
          tunnel: [w2340 w2361] -> w2326
          tunnel: w2325 -> [w2341 w2367]
          tunnel: w2324 -> [w2340 w2370]
          tunnel: w2321 -> [_ _]
          frame False {
            w2342 = TRUE ("AI to FIFO")
            n1162 = xnode "Read/Write Control"("FPGA VI Reference In"=w2346, "error in"=w2345, "AI to FIFO"=w2342, "APD to FIFO"=w2342, "Start scan (MCL)"=w2342) -> ("FPGA VI Reference Out"=w2344:T19, "error out"=w2343:errorcluster)
          }
          frame True {
            w2374 = TRUE ("AI to FIFO")
            n1163 = local read "Scan steps (MCL)"() -> (w2353:u64)
            n1164 = local read "Scan lines (y)"() -> (w2349:u64)
            n1165 = local read "Fast Scan Dir"() -> (w2360:bool)
            n1166 = local read "Actual MCL Inc (V)"() -> (w2350:dbl)
            n1167 = Decrement(x=w2349) -> (x-1=w2348:u64)
            n1168 = Decrement(x=w2353) -> (x-1=w2352:u64)
            n1169 = Multiply(x=w2350, y=w2348) -> (x*y=w2347:dbl)
            n1170 = Divide(x=w2347, y=2.0) -> (x/y=w2357:dbl)
            n1171 = Multiply(x=w2350, y=w2352) -> (x*y=w2351:dbl)
            n1172 = Divide(x=w2351, y=2.0) -> (x/y=w2356:dbl)
            n1173 = Select(t=w2356, s=w2360, f=w2357) -> (s? t:f=w2355:dbl)
            n1174 = Select(t=w2357, s=w2360, f=w2356) -> (s? t:f=w2359:dbl)
            n1175 = Subtract(x=w2367, y=w2359) -> (x-y=w2358:dbl)
            n1176 = Subtract(x=w2370, y=w2355) -> (x-y=w2354:dbl)
            n1177 = local read "2D or 1D Scan"() -> (w2372:bool)
            n1178 = Not(x=w2360) -> (.not. x?=w2366:bool)
            n1179 = Not(x=w2372) -> (.not. x?=w2368:bool)
            n1180 = And(x=w2360, y=w2368) -> (x .and. y?=w2369:bool)
            n1181 = And(x=w2368, y=w2366) -> (x .and. y?=w2371:bool)
            n1182 = Select(t=w2370, s=w2371, f=w2354) -> (s? t:f=w2361:dbl)
            n1183 = Select(t=w2367, s=w2369, f=w2358) -> (s? t:f=w2362:dbl)
            n1184 = call "Volt to I16.vi"("Voltage In"=w2362) -> ("I16 Voltage Out"=w2365:i16)
            n1185 = call "Volt to I16.vi"("Voltage In"=w2361) -> ("I16 Voltage Out"=w2364:i16)
            n1186 = xnode "Read/Write Control"("FPGA VI Reference In"=w2378, "error in"=w2377, "AI to FIFO"=w2374, "APD to FIFO"=w2374, "Start scan (MCL)"=w2374, "AO1"=w2365, "AO2"=w2364) -> ("FPGA VI Reference Out"=w2376:T19, "error out"=w2375:errorcluster)
          }
        }
        "Initial Y" <- w2327
        "Initial X" <- w2326
        "wait to reset values" <- w2328
      }
    }
    n1187 = local read "Trap Pos Elements/DMA read"() -> (w1808:u32)
    n1188 = local read "Trap AI Elements/DMA read"() -> (w1893:u32)
    n1189 = local read "APD Elements/DMA read"() -> (w1853:u32)
    n1190 = xnode "Get APD Data"("FPGA VI Reference In"=w1812, "error in"=w1811, "Number of Elements"=w1853, "Timeout (ms)"=-1) -> ("Data"=w1852:u32[], "Elements Remaining"=→"APD FIFO Elements Remaining":u32)  [unwired: 2 out]
    n1191 = xnode "Invoke Method"("FPGA VI Reference In"=w1812, "error in"=w1811, "Number of Elements"=w1808, "Timeout (ms)"=-1) -> ("Data"=w1771:u16[], "Elements Remaining"=→"Trap Pos FIFO El Remaining":u32)  [unwired: 2 out]
    n1192 = xnode "Get Trap Data"("FPGA VI Reference In"=w1812, "error in"=w1811, "Number of Elements"=w1893, "Timeout (ms)"=-1 ("Timeout")) -> ("FPGA VI Reference Out"=w1882:T19, "error out"=w1881:errorcluster, "Data"=w1772:i16[], "Elements Remaining"=w2028:u32)
    "FIFO El. Rem." <- w2028
    n1193 = local read "Trap AI FIFO Depth"() -> (w2030:u32)
    n1194 = Subtract(x=w2030, y=w1893) -> (x-y=w2029:u32)
    n1195 = Decimate 1D Array(w1771) -> (w1768:u16[], w1770:u16[], w1769:u16[])
    n1196 = Divide(x=w2028, y=w2029) -> (x/y=w2027:dbl)
    "Buffer Status" <- w2027
    n1197 = To Unsigned Long Integer(number=w1768) -> (unsigned 32bit integer=w1767:u32[])
    n1198 = Join Numbers(hi=w1770, lo=w1769) -> ((hi.lo)=w1766:u32[])
    n1199 = Equal?(x=w2027, y=1.0) -> (x = y?=w2025:bool)
    n1200 = Join Numbers(hi=w1767, lo=w1766) -> ((hi.lo)=w1760:u64[])
    n1201 = call "IR AOM word to freq - vec.vi"("Frequency Word In (double vec)"=w1760) -> ("Frequency Out"=w1807:dbl[])
    n1202 = case "Alert buffer overflow" shown="True" w2025 {
      frame False {
      }
      frame True {
        n1203 = call <vilib>:"Beep.vi"() -> ()  [unwired: 3 in, 9 out]
        "Overflow (data lost)" <- TRUE ("Overflow (data lost)")
      }
    }
    n1204 = Decimate 1D Array(w1807) -> (w1806:dbl[], w1805:dbl[])
    n1205 = Build Array(w1806, w1805) -> (w1804:dbl[][])
    n1206 = local read "Trap Sets"() -> (w1892:u32)
    n1207 = case "Deinterlace trap data, average down PSD" shown="2" w1892 {
      tunnel: w1772 -> [w2415 w2480]
      tunnel: [w2412 w2477] -> w1885
      tunnel: [w2415 w2479] -> w1763
      tunnel: "Detector Type" -> [w2414 w2475]
      tunnel: [w2413 w2478] -> w1884
      tunnel: [w2411 w2476] -> w2000
      frame 1, Default {
        n1208 = Divide(x=w2415, y=3276.7) -> (x/y=w2416:dbl[])
        n1209 = Decimate 1D Array(w2416) -> (w2425:dbl[], w2424:dbl[], w2423:dbl[], w2422:dbl[], w2421:dbl[], w2420:dbl[], w2419:dbl[], w2418:dbl[])
        n1210 = case shown="\"IR-QPD + PSD + FB-QPD position\"" w2414 {
          tunnel: w2425 -> [w2449 w2474]
          tunnel: w2424 -> [w2448 w2473]
          tunnel: w2423 -> [w2433 w2451]
          tunnel: w2422 -> [w2434 w2461]
          tunnel: w2421 -> [w2447 w2472]
          tunnel: w2420 -> [w2446 w2471]
          tunnel: w2419 -> [w2430 w2452]
          tunnel: w2418 -> [w2429 w2450]
          tunnel: [w2428 w2458] -> w2413
          tunnel: [w2427 w2457] -> w2412
          tunnel: [w2426 w2456] -> w2411
          frame "IR-QPD + PSD + FB-QPD", Default {
            w2426 = 0  # Channel pattern
            n1211 = Divide(x=w2449, y=w2434) -> (x/y=w2436:dbl[])
            n1212 = Divide(x=w2448, y=w2434) -> (x/y=w2435:dbl[])
            n1213 = Divide(x=w2447, y=w2430) -> (x/y=w2432:dbl[])
            n1214 = Divide(x=w2446, y=w2429) -> (x/y=w2431:dbl[])
            n1215 = Build Array(w2436, w2435, w2434, w2433, w2432, w2431, w2430, w2429) -> (w2427:dbl[][])
            n1216 = Bundle("T1 Y", "T1 X", "T1 Sum", "FB Sum", "PSD Y", "PSD X", "PSD Y Sum", "PSD X Sum") -> (w2445:T35)  [unwired: 1 out]
            n1217 = Cluster To Array(cluster=w2445) -> (array=w2428:string[])
          }
          frame "IR-QPD + PSD + FB-QPD position" {
            w2456 = 3  # Channel pattern
            n1218 = Negate(x=w2452) -> (-x=w2453:dbl[])
            n1219 = Divide(x=w2474, y=w2461) -> (x/y=w2463:dbl[])
            n1220 = Divide(x=w2473, y=w2461) -> (x/y=w2462:dbl[])
            n1221 = Divide(x=w2472, y=w2452) -> (x/y=w2460:dbl[])
            n1222 = Divide(x=w2471, y=w2453) -> (x/y=w2459:dbl[])
            n1223 = Build Array(w2463, w2462, w2461, w2450, w2451, w2460, w2459, w2452) -> (w2457:dbl[][])
            n1224 = Bundle("T1 Y", "T1 X", "T1 Sum", "FB X", "FB Sum", "PSD Y", "PSD X", "PSD Y Sum") -> (w2470:T35)  [unwired: 1 out]
            n1225 = Cluster To Array(cluster=w2470) -> (array=w2458:string[])
          }
        }
      }
      frame 2 {
        n1226 = case shown="\"IR-QPD + PSD + FB-QPD X position\"" w2475 {
          tunnel: w2480 -> [w2542 w2609 w2680]
          tunnel: [w2481 w2600 w2611] -> w2479
          tunnel: [w2508 w2591 w2658] -> w2478
          tunnel: [w2507 w2554 w2625] -> w2477
          tunnel: [w2501 w2589 w2656] -> w2476
          frame "IR-QPD + PSD + FB-QPD", Default {
            w2501 = 1  # Channel pattern
            # "time average x2 the 4th signal and the 4 psd signals (detection laser)"
            # "deinterlace 3 signals from qpd"
            n1227 = Decimate 1D Array(w2542) -> (w2541:i16[], w2540:i16[], w2506:i16[], w2539:i16[], w2529:i16[], w2527:i16[], w2526:i16[], w2524:i16[])
            n1228 = Decimate 1D Array(w2506) -> (w2505:i16[], w2504:i16[])
            n1229 = Decimate 1D Array(w2541) -> (w2538:i16[], w2510:i16[])
            n1230 = Decimate 1D Array(w2540) -> (w2537:i16[], w2535:i16[])
            n1231 = Decimate 1D Array(w2539) -> (w2536:i16[], w2534:i16[])
            n1232 = call "downsample 1D array - double.vi"("Ave N"=2.0, "Array In"=w2529) -> ("Array Out"=w2528:dbl[])  [unwired: 1 out]
            n1233 = call "downsample 1D array - double.vi"("Ave N"=2.0, "Array In"=w2527) -> ("Array Out"=w2509:dbl[])  [unwired: 1 out]
            n1234 = call "downsample 1D array - double.vi"("Ave N"=2.0, "Array In"=w2526) -> ("Array Out"=w2525:dbl[])  [unwired: 1 out]
            n1235 = call "downsample 1D array - double.vi"("Ave N"=2.0, "Array In"=w2524) -> ("Array Out"=w2523:dbl[])  [unwired: 1 out]
            n1236 = Interleave 1D Arrays(w2538, w2537, w2536, w2510, w2535, w2534, w2505, w2504, w2528, w2509, w2525, w2523) -> (w2522:dbl[])
            n1237 = Divide(x=w2522, y=3276.7) -> (x/y=w2521:dbl[])
            n1238 = Decimate 1D Array(w2521) -> (w2520:dbl[], w2519:dbl[], w2518:dbl[], w2517:dbl[], w2516:dbl[], w2515:dbl[], w2503:dbl[], w2502:dbl[], w2514:dbl[], w2513:dbl[], w2512:dbl[], w2511:dbl[])
            n1239 = Divide(x=w2520, y=w2518) -> (x/y=w2488:dbl[])
            n1240 = Divide(x=w2519, y=w2518) -> (x/y=w2487:dbl[])
            n1241 = Divide(x=w2517, y=w2515) -> (x/y=w2486:dbl[])
            n1242 = Divide(x=w2516, y=w2515) -> (x/y=w2485:dbl[])
            n1243 = Divide(x=w2514, y=w2512) -> (x/y=w2484:dbl[])
            n1244 = Divide(x=w2513, y=w2511) -> (x/y=w2483:dbl[])
            n1245 = Build Array(w2488, w2487, w2518, w2486, w2485, w2515, w2503, w2502, w2484, w2483, w2512, w2511) -> (w2507:dbl[][])
            n1246 = Bundle("T1 Y", "T1 X", "T1 Sum", "T2 Y", "T2 X", "T2 Sum", "T1 FB Sum", "T2 FB Sum", "PSD Y", "PSD X", "PSD Y Sum", "PSD X Sum") -> (w2489:T36)  [unwired: 1 out]
            n1247 = To Word Integer(number=w2522) -> (16bit integer=w2481:i16[])
            n1248 = Cluster To Array(cluster=w2489) -> (array=w2508:string[])
          }
          frame "IR-QPD + PSD + FB-QPD X position" {
            w2589 = 2  # Channel pattern
            # "time average x2 the 3 psd signals (detection laser)"
            # "deinterlace 3 signals from qpds"
            n1249 = Decimate 1D Array(w2609) -> (w2608:i16[], w2607:i16[], w2590:i16[], w2606:i16[], w2552:i16[], w2549:i16[], w2546:i16[], w2577:i16[])
            n1250 = Decimate 1D Array(w2590) -> (w2575:i16[], w2573:i16[])
            n1251 = Decimate 1D Array(w2608) -> (w2605:i16[], w2592:i16[])
            n1252 = Decimate 1D Array(w2607) -> (w2604:i16[], w2602:i16[])
            n1253 = Decimate 1D Array(w2606) -> (w2603:i16[], w2601:i16[])
            n1254 = Decimate 1D Array(w2577) -> (w2576:i16[], w2574:i16[])
            n1255 = call "downsample 1D array - I16.vi"("Ave N"=2.0, "Array In"=w2552) -> ("Array Out"=w2550:i16[])  [unwired: 1 in]
            n1256 = call "downsample 1D array - I16.vi"("Ave N"=2.0, "Array In"=w2546) -> ("Array Out"=w2544:i16[])  [unwired: 1 in]
            n1257 = call "downsample 1D array - I16.vi"("Ave N"=2.0, "Array In"=w2549) -> ("Array Out"=w2547:i16[])  [unwired: 1 in]
            n1258 = Interleave 1D Arrays(w2605, w2604, w2603, w2592, w2602, w2601, w2576, w2575, w2574, w2573, w2550, w2547, w2544) -> (w2600:i16[])
            n1259 = Divide(x=w2600, y=3276.7) -> (x/y=w2599:dbl[])
            n1260 = Decimate 1D Array(w2599) -> (w2598:dbl[], w2597:dbl[], w2596:dbl[], w2595:dbl[], w2594:dbl[], w2593:dbl[], w2565:dbl[], w2563:dbl[], w2562:dbl[], w2560:dbl[], w2559:dbl[], w2558:dbl[], w2555:dbl[])
            n1261 = Negate(x=w2555) -> (-x=w2553:dbl[])
            n1262 = Divide(x=w2559, y=w2555) -> (x/y=w2557:dbl[])
            n1263 = Divide(x=w2558, y=w2553) -> (x/y=w2556:dbl[])
            n1264 = Divide(x=w2598, y=w2596) -> (x/y=w2581:dbl[])
            n1265 = Divide(x=w2597, y=w2596) -> (x/y=w2580:dbl[])
            n1266 = Divide(x=w2595, y=w2593) -> (x/y=w2579:dbl[])
            n1267 = Divide(x=w2594, y=w2593) -> (x/y=w2578:dbl[])
            n1268 = Divide(x=w2565, y=w2563) -> (x/y=w2564:dbl[])
            n1269 = Divide(x=w2562, y=w2560) -> (x/y=w2561:dbl[])
            n1270 = Build Array(w2581, w2580, w2596, w2579, w2578, w2593, w2564, w2563, w2561, w2560, w2557, w2556, w2555) -> (w2554:dbl[][])
            n1271 = Bundle("T1 Y", "T1 X", "T1 Sum", "T2 Y", "T2 X", "T2 Sum", "T1 FB X", "T1 FB Sum", "T2 FB X", "T2 FB Sum", "PSD Y", "PSD X", "PSD Y Sum") -> (w2582:T37)  [unwired: 1 out]
            n1272 = Cluster To Array(cluster=w2582) -> (array=w2591:string[])
          }
          frame "IR-QPD + PSD + FB-QPD XY positions" {
            w2656 = 4  # Channel pattern
            # "time average x2 the 3 psd signals (detection laser)"
            # "deinterlace 3 signals from qpds"
            n1273 = Decimate 1D Array(w2680) -> (w2679:i16[], w2678:i16[], w2657:i16[], w2677:i16[], w2623:i16[], w2669:i16[], w2668:i16[], w2645:i16[])
            n1274 = Decimate 1D Array "Feedback Sum"(w2657) -> (w2641:i16[], w2639:i16[])
            n1275 = Decimate 1D Array "QPD Y"(w2679) -> (w2676:i16[], w2659:i16[])
            n1276 = Decimate 1D Array "QPD X"(w2678) -> (w2675:i16[], w2673:i16[])
            n1277 = Decimate 1D Array "Feedback Y"(w2623) -> (w2622:i16[], w2621:i16[])
            n1278 = Decimate 1D Array "QPD Sum"(w2677) -> (w2674:i16[], w2672:i16[])
            n1279 = Decimate 1D Array "Feedback X"(w2645) -> (w2642:i16[], w2640:i16[])
            n1280 = call "downsample 1D array - double.vi"("Ave N"=2.0, "Array In"=w2669) -> ("Array Out"=w2644:dbl[])  [unwired: 1 out]
            n1281 = call "downsample 1D array - double.vi"("Ave N"=2.0, "Array In"=w2668) -> ("Array Out"=w2643:dbl[])  [unwired: 1 out]
            n1282 = Interleave 1D Arrays(w2676, w2675, w2674, w2659, w2673, w2672, w2622, w2642, w2641, w2621, w2640, w2639, w2644, w2643) -> (w2667:dbl[])
            n1283 = Divide(x=w2667, y=3276.7) -> (x/y=w2666:dbl[])
            n1284 = Decimate 1D Array(w2666) -> (w2665:dbl[], w2664:dbl[], w2663:dbl[], w2662:dbl[], w2661:dbl[], w2660:dbl[], w2618:dbl[], w2632:dbl[], w2616:dbl[], w2617:dbl[], w2630:dbl[], w2614:dbl[], w2628:dbl[], w2626:dbl[])
            n1285 = Negate(x=w2626) -> (-x=w2624:dbl[])
            n1286 = Divide(x=w2628, y=w2624) -> (x/y=w2627:dbl[])
            n1287 = Divide(x=w2617, y=w2614) -> (x/y=w2613:dbl[])
            n1288 = Divide(x=w2618, y=w2616) -> (x/y=w2615:dbl[])
            n1289 = Divide(x=w2665, y=w2663) -> (x/y=w2649:dbl[])
            n1290 = Divide(x=w2664, y=w2663) -> (x/y=w2648:dbl[])
            n1291 = Divide(x=w2662, y=w2660) -> (x/y=w2647:dbl[])
            n1292 = Divide(x=w2661, y=w2660) -> (x/y=w2646:dbl[])
            n1293 = Divide(x=w2632, y=w2616) -> (x/y=w2631:dbl[])
            n1294 = Divide(x=w2630, y=w2614) -> (x/y=w2629:dbl[])
            n1295 = Build Array(w2649, w2648, w2663, w2647, w2646, w2660, w2615, w2631, w2616, w2613, w2629, w2614, w2627, w2626) -> (w2625:dbl[][])
            n1296 = Bundle("T1 Y", "T1 X", "T1 Sum", "T2 Y", "T2 X", "T2 Sum", "T1 FB Y", "T1 FB X", "T1 FB Sum", "T2 FB Y", "T2 FB X", "T2 FB Sum", "PSD X", "PSD Y Sum") -> (w2612:T38)  [unwired: 1 out]
            n1297 = To Word Integer(number=w2667) -> (16bit integer=w2611:i16[])
            n1298 = Cluster To Array(cluster=w2612) -> (array=w2658:string[])
          }
        }
      }
    }
    "AI labels" <- w1884
    n1299 = Decimate 1D Array(w1852) -> (w1880:u32[], w1816:u32[])
    n1300 = local read "DMA Update Period (s)"() -> (w1894:dbl)
    n1301 = local read "BD 1 Frequency 2 (MHz)"() -> (w1755:dbl)
    n1302 = local read "BD 1 Frequency 1 (MHz)"() -> (w1756:dbl)
    n1303 = Build Array(w1880, w1816) -> (w1962:u32[][])
    n1304 = local read "Data Period (s)"() -> (w1865:dbl)
    n1305 = Decimate 1D Array(w1763) -> (w1787:i16[], w1786:i16[], w1784:i16[], w1783:i16[])  [unwired: 9 out]
    n1306 = To Double Precision Float(number=w1962) -> (double precision float=w1963:dbl[][])
    n1307 = local read "APD Integration Time (s)"() -> (w1829:dbl)
    n1308 = Divide(x=w1787, y=w1786) -> (x/y=w1788:dbl[])
    n1309 = Divide(x=w1784, y=w1783) -> (x/y=w1785:dbl[])
    n1310 = feedback #1(0.0) -> (w1801:dbl)
    n1311 = Add(x=w1894, y=w1801) -> (x+y=w2002:dbl)
    n1312 = feedback-in #1(w2002) -> ()
    n1313 = local read "AOM X Cal (nm/MHz)"() -> (w1753:dbl)
    n1314 = To Time Stamp(1:w1801) -> (0:w1800:timestamp)
    n1315 = Split 1D Array(array=w1788, index="N El. to Ave.") -> (second subarray=w1791:dbl[])  [unwired: 1 out]
    n1316 = Split 1D Array(array=w1785, index="N El. to Ave.") -> (second subarray=w1790:dbl[])  [unwired: 1 out]
    n1317 = local read "Trap X AI1 (DMA)"() -> (w1789:T13)
    n1318 = Multiply(x=w1865, y="Trap Disp. Downsample") -> (x*y=w1802:dbl)
    "Display Period (s)" <- w1802
    n1319 = Bundle("BD 1 Frequency 1 (MHz)"=w1756, "BD 1 Frequency 2 (MHz)"=w1755) -> (w1757:T39)  [unwired: 1 out]
    n1320 = for "Trap AI" {
      tunnel: [w2410] -> w1996 mode=indexing
      tunnel: w1800 -> [w2400]
      tunnel: "Trap Disp. Downsample" -> [w2408]
      tunnel: w1885 -> [w2406] mode=indexing
      tunnel: w1865 -> [w2405]
      tunnel: w1884 -> [w2404] mode=indexing
      tunnel: w1799 -> [w2403]
      tunnel: [w2402] -> w1840 mode=indexing
      tunnel: w1802 -> [w2401]
      workers-P: _ -> [_]
      n1321 = Bundle By Name("Y"=w2406, "dt"=w2405) -> (w2407:waveform(dbl))  [unwired: 1 out]
      n1322 = Set Waveform Attribute(5:w2404, 6:w2403, 7:w2407) -> (3:w2402:waveform(dbl))  [unwired: 1 in, 2 out]
      n1323 = call "downsample 1D array - double.vi"("Ave N"=w2408, "Array In"=w2406) -> ("Array Out"=w2409:dbl[])  [unwired: 1 out]
      n1324 = Bundle By Name(cluster=w2402, "t0"=w2400, "Y"=w2409, "dt"=w2401) -> (w2410:waveform(dbl))
    }
    n1325 = call-poly <vilib>:"Mean.vi"("X"=w1790) -> ("mean"=w1778:dbl)  [unwired: 1 out]
    n1326 = call-poly <vilib>:"Mean.vi"("X"=w1791) -> ("mean"=w1779:dbl)  [unwired: 1 out]
    n1327 = Cluster To Array(cluster=w1757) -> (array=w1754:dbl[])
    n1328 = Reciprocal(x=w1802) -> (1/x=→"Trap Disp. Freq. (Hz)":dbl)
    n1329 = local read "Data points/scans (MCL)"() -> (w1974:dbl)
    n1330 = To Fixed-Point(number=w1778) -> (fixed-point=w1776:fxp<+/-,16,1>)  [unwired: 1 in]
    n1331 = To Fixed-Point(number=w1779) -> (fixed-point=w1777:fxp<+/-,16,1>)  [unwired: 1 in]
    n1332 = Bundle("Trap 1 Pos.", "Trap 2 Pos.") -> (w1798:cluster{string, string})  [unwired: 1 out]
    n1333 = Bundle By Name(cluster=w1789, "Set 1"=w1777, "Set 2"=w1776) -> (→"Trap X AI1 (DMA)":T13)
    n1334 = Cluster To Array(cluster=w1798) -> (array=w1795:string[])
    n1335 = Bundle("APD 1", "APD 2") -> (w1995:cluster{string, string})  [unwired: 1 out]
    n1336 = Select(t=-1.0, s="Negate Y Axis", f=1.0) -> (s? t:f=w1736:dbl)
    n1337 = for "Trap Position" {
      tunnel: w1804 -> [w2050] mode=indexing
      tunnel: "Trap Disp. Downsample" -> [w2049]
      tunnel: w1802 -> [w2047]
      tunnel: w1800 -> [w2046]
      tunnel: w1799 -> [w2044]
      tunnel: w1795 -> [w2043] mode=indexing
      tunnel: [w2042] -> w1752 mode=indexing
      tunnel: w1754 -> [w2040] mode=indexing
      tunnel: w1753 -> [w2038]
      tunnel: w1736 -> [w2037]
      n1338 = call "downsample 1D array - double.vi"("Ave N"=w2049, "Array In"=w2050) -> ("Array Out"=w2048:dbl[])  [unwired: 1 out]
      n1339 = Subtract(x=w2048, y=w2040) -> (x-y=w2041:dbl[])
      n1340 = Multiply(x=w2038, y=w2041) -> (x*y=w2039:dbl[])
      n1341 = Multiply(x=w2037, y=w2039) -> (x*y=w2035:dbl[])
      n1342 = Subtract(x=w2035, y="FB Trap Pos Offset") -> (x-y=w2036:dbl[])
      n1343 = Bundle By Name("Y"=w2036, "dt"=w2047, "t0"=w2046) -> (w2045:waveform(dbl))  [unwired: 1 out]
      n1344 = Set Waveform Attribute(5:w2043, 6:w2044, 7:w2045) -> (3:w2042:waveform(dbl))  [unwired: 1 in, 2 out]
    }
    "Trap Positions" <- w1752
    n1345 = Cluster To Array(cluster=w1995) -> (array=w1992:string[])
    n1346 = for "APD" {
      tunnel: w1963 -> [w2389] mode=indexing
      tunnel: w1829 -> [w2397]
      tunnel: [w2393] -> w1836 mode=indexing
      tunnel: "APD Disp. Scale" -> [w2394]
      tunnel: w1799 -> [w2392]
      tunnel: w1992 -> [w2391] mode=indexing
      tunnel: "APD Disp. Downsample" -> [w2387]
      tunnel: [w2390] -> w1991
      workers-P: _ -> [_]
      tunnel: w1800 -> [w2386]
      n1347 = call "integrate 1D array interval - double.vi"("Ave N"=w2387, "Array In"=w2389) -> ("Array Out"=w2388:dbl[])  [unwired: 1 out]
      n1348 = Multiply(x=w2397, y=w2387) -> (x*y=w2390:dbl)
      n1349 = Divide(x=w2388, y=w2394) -> (x/y=w2395:dbl[])
      n1350 = Bundle By Name("t0"=w2386, "Y"=w2395, "dt"=w2390) -> (w2396:waveform(dbl))  [unwired: 1 out]
      n1351 = Set Waveform Attribute(5:w2391, 6:w2392, 7:w2396) -> (3:w2393:waveform(dbl))  [unwired: 1 in, 2 out]
    }
    "APD Display Period (s)" <- w1991
    n1352 = Reciprocal(x=w1991) -> (1/x=→"APD Display Freq. (Hz)":dbl)
    n1353 = local read "Display Period (s)"() -> (w1864:dbl)
    n1354 = Increment(x=w1974) -> (x+1=w1975:dbl)
    n1355 = Index Array(array=w1752, index=0) -> (element=w1750:waveform(dbl))
    n1356 = To Double Precision Float(number=w1880) -> (double precision float=w1879:dbl[])
    n1357 = feedback #2(w1975) -> (w1978:dbl)
    n1358 = Select(t=0, s=w1965, f=w1978) -> (s? t:f=w1971:dbl)
    n1359 = Array Size(array=w1879) -> (size(s)=w1977:i32)
    n1360 = Add(x=w1977, y=w1971) -> (x+y=w1972:dbl)
    n1361 = Unbundle By Name(w1750) -> ("Y"=w1748:dbl[])
    "T1 x pos data" <- w1748
    n1362 = feedback #3(w1880) -> (w1961:u32[])
    n1363 = Build Array (concatenate)(w1961, w1880) -> (w1958:u32[])
    n1364 = feedback #4(w1816) -> (w1835:u32[])
    n1365 = Divide(x="Bead Sep. Int. Time (s)", y=w1864) -> (x/y=w1746:dbl)
    n1366 = Build Array (concatenate)(w1835, w1816) -> (w1834:u32[])
    n1367 = Greater?(x=w1972, y=w1974) -> (0:w1973:bool)
    n1368 = feedback #5(w1748) -> (w1749:dbl[])
    n1369 = Build Array (concatenate)(w1748, w1749) -> (w1747:dbl[])
    n1370 = Select(t=w1971, s=w1973, f=w1972) -> (s? t:f=w1970:dbl)
    n1371 = feedback-in #2(w1970) -> ()
    n1372 = Array Size(array=w1958) -> (size(s)=w1955:i32)
    n1373 = Array Size(array=w1880) -> (size(s)=w1957:i32)
    n1374 = local read "MCL Scanning"() -> (w1968:bool)
    n1375 = local read "APD Integration Time (s)"() -> (w1843:dbl)
    n1376 = Build Array (concatenate)(w1836, w1996) -> (w1838:waveform(dbl)[])
    "All Signals" <- w1838
    n1377 = Split 1D Array(array=w1747, index=w1746) -> (first subarray=w1740:dbl[])  [unwired: 1 out]
    n1378 = feedback-in #5(w1740) -> ()
    n1379 = Multiply(x=w1957, y="APD Ave N") -> (x*y=w1956:dbl)
    n1380 = Greater?(x=w1955, y=w1956) -> (0:w1959:bool)
    n1381 = Not(x=w1973) -> (.not. x?=w1967:bool)
    n1382 = To Double Precision Float(number=w1816) -> (double precision float=w1815:dbl[])
    n1383 = call-poly <vilib>:"Mean.vi"("X"=w1740) -> ("mean"=w1739:dbl)  [unwired: 1 out]
    "Mean T1 Position (nm)" <- w1739
    n1384 = Subtract(x=w1740, y=w1739) -> (x-y=w1745:dbl[])
    n1385 = Square(x=w1745) -> (x^2=w1744:dbl[])
    n1386 = And(x=w1967, y=w1968) -> (x .and. y?=w1969:bool)
    n1387 = call-poly <vilib>:"Mean.vi"("X"=w1744) -> ("mean"=w1743:dbl)  [unwired: 1 out]
    n1388 = case shown="True" w1959 {
      tunnel: w1958 -> [w2170 w2177]
      tunnel: [w2170 w2175] -> w1899
      tunnel: w1956 -> [_ w2172]
      tunnel: w1955 -> [_ w2176]
      tunnel: w1834 -> [w2169 w2174]
      tunnel: [w2169 w2171] -> w1831
      frame False {
      }
      frame True {
        n1389 = Subtract(x=w2176, y=w2172) -> (x-y=w2173:dbl)
        n1390 = Array Subset(array=w2177, index=w2173, length=w2172) -> (w2175:u32[])
        n1391 = Array Subset(array=w2174, index=w2173, length=w2172) -> (w2171:u32[])
      }
    }
    n1392 = feedback-in #3(w1899) -> ()
    n1393 = feedback-in #4(w1831) -> ()
    n1394 = Or(x=w1969, y=w1965) -> (x .or. y?=w1966:bool)
    n1395 = Square Root(x=w1743) -> (sqrt(x)=w1742:dbl)
    n1396 = Equal?(x="Tab Control 6", y=T29."High Res Display") -> (x = y?=w1888:bool)
    n1397 = Multiply(x="APD Disp. Scale", y=w1836) -> (x*y=w1845:waveform(dbl)[])
    n1398 = Multiply(x="APD Disp. Downsample", y=w1843) -> (x*y=w1841:dbl)
    n1399 = Multiply(x=10.0, y=w1742) -> (x*y=→"Trap 1 Position RMS (A)":dbl)
    n1400 = Divide(x=w1845, y=w1841) -> (x/y=w1813:waveform(dbl)[])
    n1401 = Index Array(array=w1813, index=0) -> (element=w1823:waveform(dbl))
    n1402 = case "For computing FFTs for display" shown="True" "Compute FFT" {
      tunnel: w1840 -> [_ w2783]
      frame False {
      }
      frame True {
        n1403 = Build Array("FFT 1 Choice 1", "FFT 1 Choice 2", "FFT 2 Choice 1", "FFT 2 Choice 2") -> (w2776:u16[])
        n1404 = Array Size(array=w2783) -> (size(s)=w2782:i32)
        n1405 = feedback-in #6(w2776) -> ()
        n1406 = feedback #6(u16[] [100, 100, 100, 100]) -> (w2777:u16[])
        n1407 = feedback-in #7("# Spectra to Ave.") -> ()
        n1408 = feedback #7("# Spectra to Ave.") -> (w2774:dbl)
        n1409 = Not Equal?(x="# Spectra to Ave.", y=w2774) -> (x != y?=w2773:bool)
        n1410 = Not Equal?(x=w2776, y=w2777) -> (x != y?=w2775:bool)
        n1411 = feedback #8(1.0) -> (w2760:dbl)
        n1412 = Compound Arithmetic op=OR("Reset FFT", w2775, w2773) -> (w2758:bool)
        n1413 = Select(t=1.0, s=w2758, f=w2760) -> (s? t:f=w2762:dbl)
        n1414 = Greater?(x=w2762, y="# Spectra to Ave.") -> (0:w2781:bool)
        n1415 = Increment(x=w2762) -> (x+1=w2761:dbl)
        n1416 = feedback-in #8(w2761) -> ()
        n1417 = local read "DMA Update Period (s)"() -> (w2756:dbl)
        n1418 = Multiply(x="# Spectra to Ave.", y=w2756) -> (x*y=→"Ave. Time (s)":dbl)
        n1419 = Build Array(cluster{"f0":dbl, "df":dbl, "magnitude":dbl[]} {"f0"=0.0, "df"=0.0, "magnitude"=[]} ("PSD")) -> (w2765:cluster{"f0":dbl, "df":dbl, "magnitude":dbl[]}[])
        n1420 = Build Array(w2765, w2765, w2765, w2765) -> (w2767:T40)
        n1421 = feedback #9(w2767) -> (w2772:T40)
        n1422 = for {
          N: 4 -> [_]
          tunnel: w2776 -> [w2805] mode=indexing
          tunnel: w2783 -> [w2806]
          tunnel: w2782 -> [w2808]
          tunnel: w2758 -> [w2801]
          tunnel: w2781 -> [w2800]
          tunnel: "# Spectra to Ave." -> [w2799]
          tunnel: [w2798] -> w2771 mode=indexing
          tunnel: w2772 -> [w2803] mode=indexing
          tunnel: [w2802] -> w2759 mode=indexing
          tunnel: w2762 -> [w2797]
          n1423 = Less?(x=w2805, y=w2808) -> (x < y?=w2807:bool)
          n1424 = Index Array(array=w2806, index=w2805) -> (element=w2804:waveform(dbl))
          n1425 = case shown="True" w2807 {
            tunnel: w2804 -> [_ w2825]
            tunnel: w2803 -> [w2810 w2823]
            tunnel: [w2810 w2811] -> w2802
            tunnel: w2801 -> [_ w2822]
            tunnel: w2800 -> [_ w2815]
            tunnel: w2799 -> [_ w2814]
            tunnel: [cluster{"f0":dbl, "df":dbl, "magnitude":dbl[]} {"f0"=0.0, "df"=0.0, "magnitude"=[]} ("PSD") w2816] -> w2798
            tunnel: w2797 -> [_ w2813]
            frame False {
            }
            frame True {
              n1426 = call <vilib>:"Std Deviation and Variance.vi"("X"=w2825) -> ("mean"=w2826:dbl)  [unwired: 1 in, 2 out]
              n1427 = Subtract(x=w2825, y=w2826) -> (x-y=w2824:waveform(dbl))
              n1428 = xnode "Spectral Measurements"("Signals"=w2824) -> ("PSD"=w2818:cluster{"f0":dbl, "df":dbl, "magnitude":dbl[]})  [unwired: 1 in, 1 out]
              n1429 = case shown="False" w2822 {
                tunnel: w2823 -> [w2835 _]
                tunnel: [w2831 w2840] -> w2811
                tunnel: w2818 -> [w2834 w2841]
                tunnel: w2815 -> [w2833 _]
                frame False {
                  n1430 = Build Array (concatenate)(w2835, w2834) -> (w2832:cluster{"f0":dbl, "df":dbl, "magnitude":dbl[]}[])
                  n1431 = case shown="True" w2833 {
                    tunnel: w2832 -> [w2836 w2839]
                    tunnel: [w2836 w2837] -> w2831
                    frame False {
                    }
                    frame True {
                      n1432 = Delete From Array(array=w2839, index=0) -> (array with subset deleted=w2837:cluster{"f0":dbl, "df":dbl, "magnitude":dbl[]}[])  [unwired: 1 in, 1 out]
                    }
                  }
                }
                frame True {
                  n1433 = Build Array(w2841) -> (w2840:cluster{"f0":dbl, "df":dbl, "magnitude":dbl[]}[])
                }
              }
              n1434 = for {
                tunnel: w2811 -> [w2830] mode=indexing
                tunnel: [w2829] -> w2821 mode=indexing
                workers-P: _ -> [_]
                n1435 = Unbundle By Name(w2830) -> ("magnitude"=w2829:dbl[])
              }
              n1436 = Transpose 2D Array(2D array=w2821) -> (transposed array=w2820:dbl[][])
              n1437 = for {
                tunnel: w2820 -> [w2828] mode=indexing
                tunnel: [w2827] -> w2819 mode=indexing
                workers-P: _ -> [_]
                n1438 = Add Array Elements(numeric array=w2828) -> (sum=w2827:dbl)
              }
              n1439 = Select(t=w2814, s=w2815, f=w2813) -> (s? t:f=w2812:dbl)
              n1440 = Divide(x=w2819, y=w2812) -> (x/y=w2817:dbl[])
              n1441 = Bundle By Name(cluster=w2818, "magnitude"=w2817) -> (w2816:cluster{"f0":dbl, "df":dbl, "magnitude":dbl[]})
            }
          }
        }
        n1442 = case shown="True" w2758 {
          tunnel: w2759 -> [w2790 w2796]
          tunnel: [w2790 w2791] -> w2757
          frame False {
          }
          frame True {
            n1443 = Array Subset(array=w2796, index (row)=0 ("index"), length (row)=4 ("length"), index (col)=0 ("index"), length (col)=1 ("length")) -> (w2791:T40)
          }
        }
        n1444 = feedback-in #9(w2757) -> ()
        n1445 = Split 1D Array(array=w2771, index=2) -> (first subarray=→"FFT 1":cluster{"f0":dbl, "df":dbl, "magnitude":dbl[]}[], second subarray=→"FFT 2":cluster{"f0":dbl, "df":dbl, "magnitude":dbl[]}[])
      }
    }
    n1446 = Index Array(array=w1813, index=1) -> (element=w1821:waveform(dbl))
    n1447 = case "For displaying the high resolution display (no downsampling)" shown="True" w1888 {
      tunnel: w1840 -> [_ w2070]
      frame False {
      }
      frame True {
        n1448 = Index Array(array=w2070, index="High Res. Display") -> (element=w2071:waveform(dbl))
        n1449 = call <vilib>:"Std Deviation and Variance.vi"("X"=w2071) -> ("mean"=w2078:dbl, "standard deviation"=w2083:dbl)  [unwired: 1 in, 1 out]
        "Mean Intensity" <- w2078
        "Sigma" <- w2083
        n1450 = Subtract(x=w2071, y=w2078) -> (x-y=w2077:waveform(dbl))
        n1451 = Select(t=w2077, s="Subtract mean", f=w2071) -> (s? t:f=→"1 Channel":waveform(dbl))
        n1452 = Divide(x=w2083, y=w2078) -> (x/y=→"Sigma/Mean":dbl)
        n1453 = feedback #10(1) -> (w2072:i32)
        n1454 = Greater Or Equal?(x=w2072, y="Slow mean N ave.") -> (x >= y?=w2085:bool)
        n1455 = Increment(x=w2072) -> (x+1=w2087:i32)
        n1456 = Select(t=1, s=w2085, f=w2087) -> (s? t:f=w2074:i32)
        n1457 = feedback-in #10(w2074) -> ()
        n1458 = feedback #11() -> (w2075:waveform(dbl))  [unwired: 1 out]
        n1459 = case shown="Default" w2072 {
          tunnel: [w2090 w2093] -> w2076
          tunnel: w2075 -> [w2092 _]
          tunnel: w2071 -> [w2091 w2093]
          frame Default {
            n1460 = call-poly <vilib>:"Append Waveforms.vi"("waveform B"=w2091, "waveform A"=w2092) -> ("waveform out"=w2090:waveform(dbl))  [unwired: 1 in, 8 out]
          }
          frame 1 {
          }
        }
        n1461 = feedback-in #11(w2076) -> ()
        n1462 = case shown="True" w2085 {
          tunnel: w2076 -> [_ w2089]
          frame False {
          }
          frame True {
            n1463 = call-poly <vilib>:"Mean.vi"("X"=w2089) -> ("mean"=→"Slow mean":dbl)  [unwired: 1 out]
          }
        }
      }
    }
    n1464 = case "For plotting results of scanning MCL" shown="True" w1966 {
      tunnel: w1965 -> [_ w2210]
      tunnel: w1879 -> [_ w2306]
      tunnel: w1974 -> [_ _]
      tunnel: w1840 -> [_ w2280]
      tunnel: w1815 -> [_ w2211]
      tunnel: w1814 -> [_ w2184]
      frame False {
      }
      frame True {
        w2191 = u32 0 items=["Horizontal", "Vertical", "Central", "1st Diagonal", "2nd Diagonal"] ("Type of Symmetry")
        w2219 = u32 0 items=["Horizontal", "Vertical", "Central", "1st Diagonal", "2nd Diagonal"] ("Type of Symmetry")
        w2222 = u32 0 items=["Horizontal", "Vertical", "Central", "1st Diagonal", "2nd Diagonal"] ("Type of Symmetry")
        w2251 = u32 0 items=["Horizontal", "Vertical", "Central", "1st Diagonal", "2nd Diagonal"] ("Type of Symmetry")
        n1465 = Index Array(array=w2280, index=10) -> (element=w2286:waveform(dbl))
        n1466 = Index Array(array=w2280, index=11) -> (element=w2283:waveform(dbl))
        n1467 = local read "Cycles/step (MCL)"() -> (w2236:u64)
        n1468 = Index Array(array=w2280, index="Channel") -> (element=w2282:waveform(dbl))
        n1469 = Unbundle(w2184) -> ("New Image"=w2183:T2, "New Image"=w2182:T2, "New Image"=w2181:T2, "New Image"=w2180:T2)
        n1470 = Unbundle By Name(w2286) -> ("Y"=w2238:dbl[])
        n1471 = Unbundle By Name(w2283) -> ("Y"=w2240:dbl[])
        n1472 = Unbundle By Name(w2282) -> ("Y"=w2245:dbl[])
        n1473 = call "downsample 1D array - double.vi"("Ave N"=w2236, "Array In"=w2238) -> ("Array Out"=w2237:dbl[])  [unwired: 1 out]
        n1474 = call "downsample 1D array - double.vi"("Ave N"=w2236, "Array In"=w2240) -> ("Array Out"=w2239:dbl[])  [unwired: 1 out]
        n1475 = call "downsample 1D array - double.vi"("Ave N"=w2236, "Array In"=w2245) -> ("Array Out"=w2244:dbl[])  [unwired: 1 out]
        n1476 = feedback #12(w2306) -> (w2307:dbl[])
        n1477 = Build Array (concatenate)(w2307, w2306) -> (w2288:dbl[])
        n1478 = feedback #13(w2211) -> (w2213:dbl[])
        n1479 = Build Array (concatenate)(w2213, w2211) -> (w2212:dbl[])
        n1480 = local read "Scan steps (MCL)"() -> (w2193:u64)
        n1481 = Select(t=w2306, s=w2210, f=w2288) -> (s? t:f=w2292:dbl[])
        n1482 = feedback-in #12(w2292) -> ()
        n1483 = Select(t=w2211, s=w2210, f=w2212) -> (s? t:f=w2194:dbl[])
        n1484 = feedback-in #13(w2194) -> ()
        n1485 = local read "Scan lines (y)"() -> (w2179:u64)
        n1486 = local read "N APD Samp/step"() -> (w2195:dbl)
        n1487 = feedback #14(w2237) -> (w2294:dbl[])
        n1488 = Build Array (concatenate)(w2294, w2237) -> (w2285:dbl[])
        n1489 = feedback #15(w2244) -> (w2304:dbl[])
        n1490 = Build Array (concatenate)(w2304, w2244) -> (w2303:dbl[])
        n1491 = feedback #16(w2239) -> (w2296:dbl[])
        n1492 = Build Array (concatenate)(w2296, w2239) -> (w2297:dbl[])
        n1493 = Select(t=w2237, s=w2210, f=w2285) -> (s? t:f=w2241:dbl[])
        n1494 = feedback-in #14(w2241) -> ()
        n1495 = Select(t=w2244, s=w2210, f=w2303) -> (s? t:f=w2243:dbl[])
        n1496 = feedback-in #15(w2243) -> ()
        n1497 = Select(t=w2239, s=w2210, f=w2297) -> (s? t:f=w2242:dbl[])
        n1498 = feedback-in #16(w2242) -> ()
        n1499 = Multiply(x=w2193, y=u64 2) -> (x*y=w2178:u64)
        n1500 = call "integrate 1D array interval - double.vi"("Ave N"=w2195, "Array In"=w2194) -> ("Array Out"=w2206:dbl[])  [unwired: 1 out]
        n1501 = call "integrate 1D array interval - double.vi"("Ave N"=w2195, "Array In"=w2292) -> ("Array Out"=w2291:dbl[])  [unwired: 1 out]
        n1502 = Array Size(array=w2206) -> (size(s)=w2207:i32)
        n1503 = Array Size(array=w2291) -> (size(s)=w2293:i32)
        n1504 = Multiply(x=w2179, y=w2178) -> (x*y=w2209:u64)
        n1505 = Multiply(x=w2179, y=w2178) -> (x*y=w2301:u64)
        n1506 = call-poly <vilib>:"Mean.vi"("X"=w2241) -> ("mean"=w2225:dbl)  [unwired: 1 out]
        n1507 = Subtract(x=w2209, y=w2207) -> (x-y=w2200:u64)
        n1508 = call-poly <vilib>:"Mean.vi"("X"=w2243) -> ("mean"=w2230:dbl)  [unwired: 1 out]
        n1509 = call-poly <vilib>:"Mean.vi"("X"=w2242) -> ("mean"=w2228:dbl)  [unwired: 1 out]
        n1510 = call-poly <vilib>:"Mean.vi"("X"=w2206) -> ("mean"=w2197:dbl)  [unwired: 1 out]
        n1511 = Subtract(x=w2301, y=w2293) -> (x-y=w2235:u64)
        n1512 = call-poly <vilib>:"Mean.vi"("X"=w2291) -> ("mean"=w2232:dbl)  [unwired: 1 out]
        n1513 = Initialize Array(1.0 ("element"), w2200) -> (w2196:dbl[])
        n1514 = Initialize Array(1.0 ("element"), w2235) -> (w2226:dbl[])
        n1515 = Multiply(x=w2196, y=w2197) -> (x*y=w2198:dbl[])
        n1516 = Multiply(x=w2226, y=w2228) -> (x*y=w2229:dbl[])
        n1517 = Multiply(x=w2226, y=w2230) -> (x*y=w2231:dbl[])
        n1518 = Multiply(x=w2226, y=w2225) -> (x*y=w2227:dbl[])
        n1519 = Multiply(x=w2226, y=w2232) -> (x*y=w2233:dbl[])
        n1520 = Build Array (concatenate)(w2241, w2227) -> (w2295:dbl[])
        n1521 = Build Array (concatenate)(w2243, w2231) -> (w2299:dbl[])
        n1522 = Build Array (concatenate)(w2242, w2229) -> (w2298:dbl[])
        n1523 = Build Array (concatenate)(w2206, w2198) -> (w2208:dbl[])
        n1524 = Build Array (concatenate)(w2291, w2233) -> (w2300:dbl[])
        n1525 = Reshape Array(w2295, w2179, w2178) -> (w2261:dbl[][])
        n1526 = Reshape Array(w2208, w2179, w2178) -> (w2204:dbl[][])
        n1527 = Reshape Array(w2299, w2179, w2178) -> (w2253:dbl[][])
        n1528 = Reshape Array(w2298, w2179, w2178) -> (w2268:dbl[][])
        n1529 = Reshape Array(w2300, w2179, w2178) -> (w2278:dbl[][])
        n1530 = Array Subset(array=w2268, index (col)=0 ("index"), length (col)=w2193) -> (w2273:dbl[][])  [unwired: 2 in]
        n1531 = Array Subset(array=w2268, index (col)=w2193) -> (w2271:dbl[][])  [unwired: 3 in]
        n1532 = Array Subset(array=w2253, index (col)=0 ("index"), length (col)=w2193) -> (w2259:dbl[][])  [unwired: 2 in]
        n1533 = Array Subset(array=w2253, index (col)=w2193) -> (w2257:dbl[][])  [unwired: 3 in]
        n1534 = Array Subset(array=w2204, index (col)=0 ("index"), length (col)=w2193) -> (w2203:dbl[][])  [unwired: 2 in]
        n1535 = Array Subset(array=w2204, index (col)=w2193) -> (w2201:dbl[][])  [unwired: 3 in]
        n1536 = Array Subset(array=w2278, index (col)=0 ("index"), length (col)=w2193) -> (w2277:dbl[][])  [unwired: 2 in]
        n1537 = Array Subset(array=w2278, index (col)=w2193) -> (w2275:dbl[][])  [unwired: 3 in]
        n1538 = Array Subset(array=w2261, index (col)=0 ("index"), length (col)=w2193) -> (w2266:dbl[][])  [unwired: 2 in]
        n1539 = Array Subset(array=w2261, index (col)=w2193) -> (w2264:dbl[][])  [unwired: 3 in]
        n1540 = for {
          tunnel: w2273 -> [w2315] mode=indexing
          tunnel: [w2314] -> w2272 mode=indexing
          workers-P: _ -> [_]
          n1541 = Reverse 1D Array(array=w2315) -> (reversed array=w2314:dbl[])
        }
        n1542 = for {
          tunnel: w2259 -> [w2311] mode=indexing
          tunnel: [w2310] -> w2258 mode=indexing
          workers-P: _ -> [_]
          n1543 = Reverse 1D Array(array=w2311) -> (reversed array=w2310:dbl[])
        }
        n1544 = for {
          tunnel: w2203 -> [w2309] mode=indexing
          tunnel: [w2308] -> w2202 mode=indexing
          workers-P: _ -> [_]
          n1545 = Reverse 1D Array(array=w2309) -> (reversed array=w2308:dbl[])
        }
        n1546 = for {
          tunnel: w2277 -> [w2317] mode=indexing
          tunnel: [w2316] -> w2276 mode=indexing
          workers-P: _ -> [_]
          n1547 = Reverse 1D Array(array=w2317) -> (reversed array=w2316:dbl[])
        }
        n1548 = for {
          tunnel: w2266 -> [w2313] mode=indexing
          tunnel: [w2312] -> w2265 mode=indexing
          workers-P: _ -> [_]
          n1549 = Reverse 1D Array(array=w2313) -> (reversed array=w2312:dbl[])
        }
        n1550 = Index Array(array=w2278, index (row)=0) -> (element=→"Waveform Graph":dbl[])  [unwired: 1 in]
        n1551 = Add(x=w2272, y=w2271) -> (x+y=w2270:dbl[][])
        n1552 = Add(x=w2258, y=w2257) -> (x+y=w2256:dbl[][])
        n1553 = Add(x=w2202, y=w2201) -> (x+y=w2186:dbl[][])
        n1554 = Add(x=w2276, y=w2275) -> (x+y=w2250:dbl[][])
        n1555 = Add(x=w2265, y=w2264) -> (x+y=w2263:dbl[][])
        n1556 = Divide(x=w2256, y=2) -> (x/y=w2254:dbl[][])
        n1557 = Divide(x=w2270, y=2) -> (x/y=w2215:dbl[][])
        n1558 = Divide(x=w2263, y=2) -> (x/y=w2217:dbl[][])
        n1559 = To Single Precision Float(number=w2250) -> (single precision float=w2249:sgl[][])
        n1560 = Transpose 2D Array(2D array=w2254) -> (transposed array=→"Data map":dbl[][])
        n1561 = To Single Precision Float(number=w2186) -> (single precision float=w2190:sgl[][])
        n1562 = To Single Precision Float(number=w2215) -> (single precision float=w2221:sgl[][])
        n1563 = To Single Precision Float(number=w2217) -> (single precision float=w2218:sgl[][])
        n1564 = call "IMAQ ArrayToImage"("Image Pixels (Float)"=w2249, "Image"=w2183) -> ("Image Out"=w2252:T2)  [unwired: 8 in, 1 out]
        n1565 = call "IMAQ ArrayToImage"("Image Pixels (Float)"=w2190, "Image"=w2182) -> ("Image Out"=w2192:T2)  [unwired: 8 in, 1 out]
        n1566 = call "IMAQ ArrayToImage"("Image Pixels (Float)"=w2221, "Image"=w2181) -> ("Image Out"=w2223:T2)  [unwired: 8 in, 1 out]
        n1567 = call "IMAQ ArrayToImage"("Image Pixels (Float)"=w2218, "Image"=w2180) -> ("Image Out"=w2220:T2)  [unwired: 8 in, 1 out]
        n1568 = call "IMAQ Symmetry"("Type of Symmetry"=w2251, "Image Src"=w2252) -> ("Image Dst Out"=w2247:T2)  [unwired: 3 in, 1 out]
        n1569 = call "IMAQ Symmetry"("Type of Symmetry"=w2191, "Image Src"=w2192) -> ("Image Dst Out"=w2188:T2)  [unwired: 3 in, 1 out]
        n1570 = call "IMAQ Symmetry"("Type of Symmetry"=w2222, "Image Src"=w2223) -> ("Image Dst Out"=→"Detection Laser X":T2)  [unwired: 3 in, 1 out]
        n1571 = call "IMAQ Symmetry"("Type of Symmetry"=w2219, "Image Src"=w2220) -> ("Image Dst Out"=→"Detection Laser Y":T2)  [unwired: 3 in, 1 out]
        n1572 = call "IMAQ Set Simple Calibration"("Calibration Axis Info"=T30 {"Origin Pixel"={"X"=0.0, "Y"=0.0}, "Angle Relative to Horizontal (deg)"=0.0, "Axis Reference"=0}, "Grid Descriptor"=T31 {"X Step"=0.3, "Y Step"=0.3, "Unit"=enum."Undefined"}, "Image"=w2247) -> ("Calibrated Image"=→"APD 1":T2)  [unwired: 7 in, 1 out]
        n1573 = call "IMAQ Set Simple Calibration"("Calibration Axis Info"=T30 {"Origin Pixel"={"X"=0.0, "Y"=0.0}, "Angle Relative to Horizontal (deg)"=0.0, "Axis Reference"=0}, "Grid Descriptor"=T31 {"X Step"=0.3, "Y Step"=0.3, "Unit"=enum."Undefined"}, "Image"=w2188) -> ("Calibrated Image"=→"APD 2":T2)  [unwired: 7 in, 1 out]
      }
    }
    n1574 = Subtract(x=w1821, y="APD 2 Offset") -> (x-y=w1818:waveform(dbl))
    n1575 = Subtract(x=w1823, y="APD 1 Offset") -> (x-y=w1819:waveform(dbl))
    n1576 = Index Array(array=w1838, index=3) -> (element=w1910:waveform(dbl))
    n1577 = Index Array(array=w1838, index=6) -> (element=w1907:waveform(dbl))
    n1578 = Build Array(w1819, w1818) -> (→"APD Chart":waveform(dbl)[])
    n1579 = Array Size(array=w1899) -> (size(s)=w1954:i32)
    n1580 = call <vilib>:"Std Deviation and Variance.vi"("X"=w1831) -> ("standard deviation"=w1830:dbl)  [unwired: 1 in, 2 out]
    n1581 = Add Array Elements(numeric array=w1831) -> (sum=w1833:u32)
    n1582 = Add Array Elements(numeric array=w1899) -> (sum=w1964:u32)
    n1583 = call <vilib>:"Std Deviation and Variance.vi"("X"=w1899) -> ("standard deviation"=w1898:dbl)  [unwired: 1 in, 2 out]
    n1584 = Divide(x="T1 offset_x (mV)", y=1000.0) -> (x/y=w1911:dbl)
    n1585 = Divide(x=w1830, y=w1829) -> (x/y=w1826:dbl)
    "Rate sigma (Hz) 2" <- w1826
    n1586 = Multiply(x=w1829, y=w1954) -> (x*y=w1832:dbl)
    "Int. Time (s)" <- w1832
    n1587 = Divide(x=w1833, y=w1832) -> (x/y=w1827:dbl)
    "APD 2 Rate (Hz)" <- w1827
    n1588 = Divide(x=w1964, y=w1832) -> (x/y=w1896:dbl)
    "APD 1 Rate (Hz)" <- w1896
    n1589 = Divide(x=w1898, y=w1829) -> (x/y=w1897:dbl)
    "Rate sigma (Hz)" <- w1897
    n1590 = Divide(x=w1826, y=w1827) -> (x/y=→"Sigma/Mean 2":dbl)
    n1591 = Divide(x=w1897, y=w1896) -> (x/y=→"Sigma/Mean":dbl)
    n1592 = Divide(x="T2 offset_x (mV)", y=1000.0) -> (x/y=w1909:dbl)
    n1593 = case shown="0, Default" "Calibration" {
      tunnel: "T1 alpha_x (nm/V)" -> [_ w2146 w2167]
      tunnel: "T1 kappa_x (pN/nm)" -> [_ _ w2157]
      tunnel: "T2 alpha_x (nm/V)" -> [_ w2145 w2165]
      tunnel: "T2 kappa_x (pN/nm)" -> [_ _ w2158]
      tunnel: w1910 -> [w2128 w2143 w2163]
      tunnel: w1907 -> [w2127 w2141 w2161]
      tunnel: [w2128 w2140 w2160] -> w1940
      tunnel: [w2127 w2139 w2159] -> w1939
      tunnel: ["T1 X (V)" ("Label.Text") "T1 X (nm)" ("Label.Text") "T1 X (pN)" ("Label.Text")] -> w1928
      tunnel: ["T2 X (V)" ("Label.Text") "T2 X (nm)" ("Label.Text") "T2 X (pN)" ("Label.Text")] -> w1927
      tunnel: ["Position (V)" ("Label.Text") "Position (nm)" ("Label.Text") "Force (pN)" ("Label.Text")] -> w1929
      tunnel: w1909 -> [_ w2131 w2150]
      tunnel: w1911 -> [_ w2134 w2152]
      tunnel: ["Mean (V)" ("Label.Text") "Mean (nm)" ("Label.Text") "Mean (pN)" ("Label.Text")] -> w1924
      tunnel: ["Difference (V)" ("Label.Text") "Difference (nm)" ("Label.Text") "Difference (pN)" ("Label.Text")] -> w1846
      frame 0, Default {
      }
      frame 1 {
        n1594 = Unbundle By Name(w2143) -> ("Y"=w2147:dbl[])
        n1595 = Unbundle By Name(w2141) -> ("Y"=w2132:dbl[])
        n1596 = Subtract(x=w2147, y=w2134) -> (x-y=w2135:dbl[])
        n1597 = Subtract(x=w2132, y=w2131) -> (x-y=w2133:dbl[])
        n1598 = Multiply(x=w2133, y=w2145) -> (x*y=w2142:dbl[])
        n1599 = Multiply(x=w2146, y=w2135) -> (x*y=w2144:dbl[])
        n1600 = Bundle By Name(cluster=w2141, "Y"=w2142) -> (w2139:waveform(dbl))
        n1601 = Bundle By Name(cluster=w2143, "Y"=w2144) -> (w2140:waveform(dbl))
      }
      frame 2 {
        n1602 = Unbundle By Name(w2163) -> ("Y"=w2168:dbl[])
        n1603 = Unbundle By Name(w2161) -> ("Y"=w2166:dbl[])
        n1604 = Subtract(x=w2166, y=w2150) -> (x-y=w2151:dbl[])
        n1605 = Subtract(x=w2168, y=w2152) -> (x-y=w2153:dbl[])
        n1606 = Compound Arithmetic op=MULTIPLY(w2151, w2165, w2158) -> (w2162:dbl[])
        n1607 = Compound Arithmetic op=MULTIPLY(w2157, w2167, w2153) -> (w2164:dbl[])
        n1608 = Bundle By Name(cluster=w2161, "Y"=w2162) -> (w2159:waveform(dbl))
        n1609 = Bundle By Name(cluster=w2163, "Y"=w2164) -> (w2160:waveform(dbl))
      }
    }
    n1610 = feedback-in #17("Calibration") -> ()
    n1611 = feedback #17(u16 1 ("Calibration")) -> (w1931:u16)
    n1612 = Not Equal?(x=w1931, y="Calibration") -> (x != y?=w1886:bool)
    n1613 = Unbundle By Name(w1910) -> ("Y"=w1913:dbl[])
    n1614 = Unbundle By Name(w1907) -> ("Y"=w1916:dbl[])
    n1615 = Subtract(x=w1913, y=w1911) -> (x-y=w1914:dbl[])
    n1616 = Subtract(x=w1916, y=w1909) -> (x-y=w1915:dbl[])
    n1617 = Multiply(x=w1915, y="T2 alpha_x (nm/V)") -> (x*y=w1906:dbl[])
    n1618 = Multiply(x="T1 alpha_x (nm/V)", y=w1914) -> (x*y=w1905:dbl[])
    n1619 = Multiply(x=w1939, y=-1.0) -> (x*y=w1918:waveform(dbl))
    n1620 = case shown="True" "Read Lateness and Rel Phase" {
      tunnel: w1882 -> [w2094 w2116]
      tunnel: w1881 -> [w2095 w2115]
      tunnel: [w2094 w2114] -> w1902
      tunnel: [w2095 w2113] -> w1901
      frame False {
      }
      frame True {
        n1621 = xnode "Read/Write Control"("FPGA VI Reference In"=w2116, "error in"=w2115) -> ("FPGA VI Reference Out"=w2114:T19, "error out"=w2113:errorcluster, "GI Relative phase"=→"GI relative phase":i16, "Relative phase"=→"Relative phase (AI1)":i16, "AI Late Counter"=→"Late Counter (AI1)":u16, "GI Late Counter"=→"GI Late Counter":u16, "MCL Late Counter"=→"MCL Late Counter":u16, "MCL Relative Phase"=→"Relative Phase (MCL)":i16, "APD Acq Relative Phase"=→"APD Acq Relative Phase":i16, "APD 1 Gate Relative Phase"=→"APD 1 Gate Relative Phase":i16, "APD 2 Gate Relative Phase"=→"APD 2 Gate Relative Phase":i16, "APD Acq Late Counter"=→"APD Acq Late Counter":u16, "APD 1 Gate Late Counter"=→"APD 1 Gate Late Counter":u16, "APD 2 Gate Late Counter"=→"APD 2 Gate Late Counter":u16, "Green FB Relative Phase"=→"Relative phase (Green FB)":i16, "GI Relative phase 2"=→"GI relative phase 2":i16, "GI Late Counter 2"=→"GI Late Counter 2":u16, "Trap Pos FIFO Timeout"=→"Trap Pos FIFO Timeout":u16, "Trap AI FIFO Timeout"=→"Trap AI FIFO Timeout":u16)
      }
    }
    n1622 = Subtract(x=w1906, y=w1905) -> (x-y=w1904:dbl[])
    n1623 = Unbundle By Name(w1939) -> ("Y"=w1871:dbl[])
    n1624 = Unbundle By Name(w1940) -> ("Y"=w1872:dbl[])
    n1625 = Build Array(w1940, w1918) -> (→"Force":waveform(dbl)[])
    n1626 = Subtract(x=w1904, y="Offset (nm)") -> (x-y=w1869:dbl[])
    n1627 = call-poly <vilib>:"Mean.vi"("X"=w1871) -> ("mean"=w1850:dbl)  [unwired: 1 out]
    "T2 X" <- w1850
    n1628 = Absolute Value(x=w1872) -> (abs(x)=w1873:dbl[])
    n1629 = Absolute Value(x=w1871) -> (abs(x)=w1874:dbl[])
    n1630 = call-poly <vilib>:"Mean.vi"("X"=w1872) -> ("mean"=w1851:dbl)  [unwired: 1 out]
    "T1 X" <- w1851
    n1631 = Add(x=w1873, y=w1874) -> (x+y=w1875:dbl[])
    n1632 = Bundle By Name(cluster=w1910, "Y"=w1869) -> (w1837:waveform(dbl))
    "Bead Separation" <- w1837
    n1633 = Divide(x=w1875, y=2.0) -> (x/y=→"Vec Mean of T1 T2":dbl[])
    n1634 = case shown="True" w1886 {
      tunnel: w1929 -> [_ w2121]
      tunnel: w1928 -> [_ w2120]
      tunnel: w1927 -> [_ w2119]
      tunnel: w1924 -> [_ w2118]
      tunnel: w1846 -> [_ w2117]
      frame False {
      }
      frame True {
        n1635 = property on="Force" class="WFChart (strict)"("YScale.NameLbl.Text"=w2121) -> ()  [unwired: 2 in, 2 out]
        n1636 = property on="T2 X" class="DigNum (strict)"("Caption.Text"=w2119) -> ()  [unwired: 2 in, 2 out]
        n1637 = property on="T1 X" class="DigNum (strict)"("Caption.Text"=w2120) -> ()  [unwired: 2 in, 2 out]
        n1638 = property on="Mean" class="DigNum (strict)"("Caption.Text"=w2118) -> ()  [unwired: 2 in, 2 out]
        n1639 = property on="Difference" class="DigNum (strict)"("Caption.Text"=w2117) -> ()  [unwired: 2 in, 2 out]
      }
    }
    n1640 = local read "Tether"() -> (w1878:bool)
    n1641 = Absolute Value(x=w1851) -> (abs(x)=w1848:dbl)
    n1642 = Absolute Value(x=w1850) -> (abs(x)=w1847:dbl)
    n1643 = Add(x=w1848, y=w1847) -> (x+y=w1926:dbl)
    n1644 = Subtract(x=w1848, y=w1847) -> (x-y=→"Difference":dbl)
    n1645 = feedback #18(w1869) -> (w1868:dbl[])
    n1646 = Divide(x=w1926, y=2.0) -> (x/y=w1877:dbl)
    "Mean" <- w1877
    n1647 = case shown="True" w1878 {
      tunnel: w1877 -> [_ w2053]
      frame False {
      }
      frame True {
        n1648 = Greater?(x="Lost Tether Alarm Threshold (pN)", y=w2053) -> (0:w2051:bool)
        n1649 = case shown="True" w2051 {
          frame False {
          }
          frame True {
            w2054 = FALSE ("Value (Signaling)")
            n1650 = flat-sequence {
              frame #0 {
                # "stop only if saving"
                n1651 = local read "Saving..."() -> (w2066:bool)
                n1652 = And(x=w2066, y="TA Cancel Save?") -> (x .and. y?=w2065:bool)
                n1653 = local write "Stop Saving"(w2065) -> ()
              }
              frame #1 {
                n1654 = case shown="True" "TA Green Off?" {
                  frame False {
                  }
                  frame True {
                    w2069 = FALSE ("Fl. Triggered...")
                    n1655 = local write "Fl. Triggered..."(w2069) -> ()
                    n1656 = property on="Green Laser ON/Interlacing" class="Bool (strict)"("Val(Sgnl)"=w2069) -> ()  [unwired: 2 in, 2 out]
                  }
                }
              }
            }
            n1657 = local read "Time tether formed"() -> (w2060:timestamp)
            n1658 = Get Date/Time In Seconds() -> (seconds since 1Jan1904=w2061:timestamp)
            n1659 = Subtract(x=w2061, y=w2060) -> (x-y=w2059:dbl)
            n1660 = Number To Decimal String(number=w2059) -> (decimal integer string=w2056:string)  [unwired: 1 out]
            n1661 = local read "Messages"() -> (w2063:string)
            n1662 = call <vilib>:"Beep.vi"() -> ()  [unwired: 3 in, 9 out]
            n1663 = Concatenate Strings("Lost tether (" ("Message to add"), w2056, " s)." ("string")) -> (w2058:string)
            n1664 = local write "Tether"(FALSE ("Tether")) -> ()
            n1665 = call "Update messages.vi"("Message to add"=w2058, "Old message string"=w2063) -> ("New message string"=w2062:string)
            n1666 = local write "Messages"(w2062) -> ()
            n1667 = property on="Trap Pos. FB ON" class="Bool (strict)"("Val(Sgnl)"=w2054) -> ()  [unwired: 2 in, 2 out]
            n1668 = property on="Trap Triggering" class="Bool (strict)"("Val(Sgnl)"=w2054) -> ()  [unwired: 2 in, 2 out]
          }
        }
      }
    }
    n1669 = Build Array (concatenate)(w1869, w1868) -> (w1867:dbl[])
    n1670 = Split 1D Array(array=w1867, index=w1746) -> (first subarray=w1863:dbl[])  [unwired: 1 out]
    n1671 = feedback-in #18(w1863) -> ()
    n1672 = call-poly <vilib>:"Mean.vi"("X"=w1863) -> ("mean"=w1862:dbl)  [unwired: 1 out]
    "Bead Mean (nm)" <- w1862
    n1673 = Subtract(x=w1863, y=w1862) -> (x-y=w1861:dbl[])
    n1674 = Square(x=w1861) -> (x^2=w1860:dbl[])
    n1675 = call-poly <vilib>:"Mean.vi"("X"=w1860) -> ("mean"=w1859:dbl)  [unwired: 1 out]
    n1676 = Square Root(x=w1859) -> (sqrt(x)=w1858:dbl)
    n1677 = Multiply(x=10.0, y=w1858) -> (x*y=→"RMS (Ang)":dbl)
    n1678 = xnode "Read/Write Control"("FPGA VI Reference In"=w1902, "error in"=w1901) -> ("FPGA VI Reference Out"=w2020:T19, "error out"=w2014:errorcluster, "AI2 Y Sum Set 1"=w2010:i16, "AI2 Y Sum Set 2"=w2009:i16, "AI1 X Set 1"=w1781:fxp<+/-,16,1>, "AI1 X Set 2"=w1780:fxp<+/-,16,1>, "Trap Pos FB Int Signal"=→"Trap Pos FB Int Signal":fxp<+/-,24,9>, "Trap Pos FB Int-Norm Signal"=→"Trap Pos FB Int-Norm Signal":fxp<+/-,16,1>, "Trap Pos FB Action"=w1774:i64, "Scanning"=→"AOD Scanning":bool, "Scan I"=→"AOD Scan I":u64, "Scanning MCL"=w2012:bool, "Scan I (MCL)"=→"MCL Scan I":u64, "Green FB Signals"=w1949:T41)  [unwired: 1 out]
    "MCL Scanning" <- w2012
    "Trap Pos FB Action" <- w1774
    n1679 = local read "AI2 (V)"() -> (w2011:cluster{"Set 1":dbl, "Set 2":dbl})
    n1680 = Bundle By Name(cluster=w2011, "Set 1"=w2010, "Set 2"=w2009) -> (w2007:cluster{"Set 1":dbl, "Set 2":dbl})
    n1681 = Divide(x=w1774, y=327.67) -> (x/y=→"Action (%)":dbl)
    n1682 = local read "Trap X (AI1)"() -> (w1794:T10)
    n1683 = Divide(x=w2007, y=3276.7) -> (x/y=w2006:cluster{"Set 1":dbl, "Set 2":dbl})
    n1684 = local write "AI2 (V)"(w2006) -> ()
    n1685 = Bundle(cluster=w1794, "Trap 1"=w1781, "Trap 2"=w1780) -> (→"Trap X (AI1)":T10)
    n1686 = Divide(x=w1949, y=3276.7) -> (x/y=w1945:T42)
    n1687 = Unbundle By Name(w1945) -> ("Green FB Ch 0"=w1948:dbl, "Green FB Ch 1"=w1947:dbl, "Green FB Ch 2"=w1946:dbl)
    n1688 = Divide(x=w1948, y=w1946) -> (x/y=w1944:dbl)
    n1689 = Divide(x=w1947, y=w1946) -> (x/y=w1943:dbl)
    n1690 = flat-sequence "To save data" {
      tunnel: [w2889] -> w2032
      tunnel: [w2890] -> w2031
      tunnel: w1980 -> [w2883]
      tunnel: w1865 -> [w2887]
      tunnel: ["Save Calibration"] -> w2003
      tunnel: w2000 -> [w2886]
      tunnel: [w2879] -> w1999
      tunnel: [w2876] -> w1998
      tunnel: [w2873] -> w1997
      tunnel: w1979 -> [w2875]
      tunnel: w1884 -> [w2869]
      tunnel: [w2869] -> w1883
      tunnel: ["Start Saving"] -> w1839
      tunnel: [w2863] -> w1762
      tunnel: [w2862] -> w1761
      tunnel: w2032 -> [w3124]
      tunnel: w2031 -> [w3123]
      tunnel: w1763 -> [w3122]
      tunnel: w2003 -> [w3121]
      tunnel: w1999 -> [w3119]
      tunnel: w1998 -> [w3118]
      tunnel: w1997 -> [w3117]
      tunnel: w1852 -> [w3116]
      tunnel: w1894 -> [w3115]
      tunnel: w1883 -> [w3114]
      tunnel: w1839 -> [w3113]
      tunnel: w1837 -> [w3112]
      tunnel: w1813 -> [w3111]
      tunnel: w1762 -> [w3110]
      tunnel: w1761 -> [w3109]
      tunnel: w1760 -> [w3108]
      frame #0 {
        n1691 = Or(x="Save N Sets", y="Start Saving") -> (x .or. y?=w2870:bool)
        n1692 = To Double Precision Float(number=w2886) -> (double precision float=w2880:dbl)
        n1693 = Build Array(w2870, "Save Calibration", w2883, w2875) -> (w2885:bool[])
        n1694 = Compound Arithmetic op=OR("Save Calibration", w2883, w2870, w2875) -> (w2888:bool)
        n1695 = Boolean Array To Number(Boolean array=w2885) -> (number=w2882:u32)
        n1696 = feedback #19(FALSE ("Save APD Data\nwith Trap Data")) -> (w2864:bool)
        n1697 = feedback #20(refnum<k0> refnum) -> (w2891:refnum<file>)
        n1698 = feedback #21(refnum<k0> refnum) -> (w2866:refnum<file>)
        n1699 = feedback #22(FALSE ("Save APD Data\nwith Trap Data")) -> (w2874:bool)
        n1700 = feedback #23(refnum<k0> refnum) -> (w2877:refnum<file>)
        n1701 = feedback #24(0) -> (w2893:i32)
        n1702 = feedback #25() -> (w2881:u32)  [unwired: 1 out]
        n1703 = case shown="True" w2888 {
          tunnel: [w2900 1] -> w2889
          tunnel: w2893 -> [w2902 _]
          tunnel: [w2901 w2920] -> w2890
          tunnel: w2891 -> [w2901 _]
          tunnel: w2887 -> [_ w2940]
          tunnel: w2880 -> [_ w2938]
          tunnel: w2882 -> [_ w2941]
          tunnel: [w2899 w2919] -> w2879
          tunnel: w2881 -> [w2899 _]
          tunnel: [w2898 w2917] -> w2876
          tunnel: w2877 -> [w2898 _]
          tunnel: [w2897 w2916] -> w2873
          tunnel: w2874 -> [w2897 _]
          tunnel: "Start Saving" -> [_ w2914]
          tunnel: w2869 -> [_ w2913]
          tunnel: [w2896 w2904] -> w2862
          tunnel: w2866 -> [w2896 _]
          tunnel: [w2895 w2903] -> w2863
          tunnel: w2864 -> [w2895 _]
          frame False {
            n1704 = Increment(x=w2902) -> (x+1=w2900:i32)
          }
          frame True {
            w2910 = FALSE ("Start Saving")
            w2915 = 9.0  # File Version
            w2923 = FALSE ("prepend array or string size? (T)")
            w2921 = T24."big-endian, network order" ("byte order (0:big-endian, network order)")
            n1705 = local read "BD 1 Frequency 1 (MHz)"() -> (w2937:dbl)
            n1706 = local read "BD 2 Frequency 1 (MHz)"() -> (w2936:dbl)
            n1707 = local read "BD 1 Frequency 2 (MHz)"() -> (w2935:dbl)
            n1708 = local read "BD 2 Frequency 2 (MHz)"() -> (w2934:dbl)
            n1709 = local read "BD 1 Frequency 3 (MHz)"() -> (w2933:dbl)
            n1710 = local read "BD 2 Frequency 3 (MHz)"() -> (w2932:dbl)
            n1711 = Array Size(array=w2913) -> (size(s)=w2912:i32)
            n1712 = To Double Precision Float(number=w2912) -> (double precision float=w2911:dbl)
            n1713 = local write "Save Calibration"(w2910) -> ()
            n1714 = local write "Start Saving"(w2910) -> ()
            n1715 = Build Array("Save APD Data\nwith Trap Data", "Save Trap Pos. Data") -> (w2907:bool[])
            n1716 = Boolean Array To Number(Boolean array=w2907) -> (number=w2906:u32)
            n1717 = Build Array(w2937, w2936, w2935, w2934, w2933, w2932) -> (w2931:dbl[])
            n1718 = case shown="4" w2941 {
              tunnel: w2940 -> [w3012 w3032 w3048 w3086]
              tunnel: w2911 -> [w3017 w3039 w3068 w3105]
              tunnel: w2938 -> [w3016 w3038 w3067 w3104]
              tunnel: [w3013 w3034 w3059 w3096] -> w2929
              tunnel: [w3004 "Cal sets to save" w3049 w3087] -> w2919
              tunnel: w2931 -> [w3014 w3035 w3061 w3098]
              tunnel: "Save APD Data\nwith Trap Data" -> [w3011 _ w3045 w3084]
              tunnel: [w3011 w3026 w3045 w3084] -> w2916
              tunnel: w2915 -> [w3007 w3027 w3043 w3082]
              tunnel: w2914 -> [w3006 _ _ _]
              tunnel: [w2997 w3026 w3042 w3072] -> w2903
              tunnel: "Save Trap Pos. Data" -> [w2997 _ w3042 w3072]
              tunnel: w2906 -> [w2996 _ w3041 w3071]
              frame 1, Default {
                # "timeseries"
                n1719 = case shown="True" "Profile" {
                  tunnel: [w3020 w3024] -> w3001
                  tunnel: [w3020 w3023] -> w3000
                  tunnel: [w3020 w3022] -> w2999
                  tunnel: [w3020 w3021] -> w2998
                  frame False {
                    w3020 = 0.0 ("f")
                  }
                  frame True {
                    n1720 = local read "Current Position"() -> (w3025:cluster{dbl, dbl, dbl})
                    n1721 = local read "Y change (mm)"() -> (w3021:dbl)
                    n1722 = Unbundle(w3025) -> (w3024:dbl, w3023:dbl, w3022:dbl)
                  }
                }
                n1723 = local read "Save ave N"() -> (w3019:dbl)
                n1724 = Multiply(x=w3019, y=w3012) -> (x*y=w3018:dbl)
                n1725 = To Double Precision Float(number=w2996) -> (double precision float=w3010:dbl)
                n1726 = Build Array(w3007, w3012, w3018, w3017, w3016, 0.0 ("f")) -> (w3015:dbl[])
                n1727 = Build Array(w3010, w3001, w3000, w2999, w2998) -> (w3008:dbl[])
                n1728 = Select(t=u32 4000000000, s=w3006, f="N sets to save") -> (s? t:f=w3004:u32)
                n1729 = Build Array (concatenate)(w3015, w3014, w3008) -> (w3013:dbl[])
              }
              frame 2 {
                w3029 = 0.0 ("f")
                w3026 = FALSE ("Save APD Data\nwith Trap Data")
                # "calibration"
                n1730 = Boolean To (0,1)(Boolean=w3026) -> (0, 1=w3031:i16)
                n1731 = To Double Precision Float(number=w3031) -> (double precision float=w3030:dbl)
                n1732 = Build Array(w3030, w3029, w3029, w3029, w3029) -> (w3028:dbl[])
                n1733 = Build Array(w3027, w3032, w3032, w3039, w3038, 1.0 ("t")) -> (w3036:dbl[])
                n1734 = Build Array (concatenate)(w3036, w3035, w3028) -> (w3034:dbl[])
                "Calibrating Trap..." <- TRUE ("Calibrating...")
              }
              frame 4 {
                w3046 = 0.0 ("f")
                # "scan dir (x/y = 0/1)"
                # "cycles/step"
                # "n scans (f/b)"
                # "steps"
                # "freq. range"
                # "AOD raster scan"
                n1735 = local read "Number of F/B Scans (AOD)"() -> (w3053:u16)
                n1736 = local read "Cycles/step (AOD)"() -> (w3055:u64)
                n1737 = local read "Scan Range (MHz)"() -> (w3058:dbl)
                n1738 = local read "Scan steps (AOD)"() -> (w3057:u64)
                n1739 = local read "Scan BD"() -> (w3065:bool)
                n1740 = local read "Save ave N"() -> (w3070:dbl)
                n1741 = Boolean To (0,1)(Boolean=w3065) -> (0, 1=w3064:i16)
                n1742 = To Double Precision Float(number=w3053) -> (double precision float=w3052:dbl)
                n1743 = To Double Precision Float(number=w3057) -> (double precision float=w3056:dbl)
                n1744 = To Double Precision Float(number=w3055) -> (double precision float=w3054:dbl)
                n1745 = To Double Precision Float(number=w3064) -> (double precision float=w3063:dbl)
                n1746 = Multiply(x=w3070, y=w3048) -> (x*y=w3069:dbl)
                n1747 = To Double Precision Float(number=w3041) -> (double precision float=w3047:dbl)
                n1748 = Build Array(w3047, w3046, w3046, w3046, w3046) -> (w3044:dbl[])
                n1749 = local read "N sets should be saved"() -> (w3050:dbl)
                n1750 = Build Array(w3063, w3058, w3056, w3054, w3052) -> (w3060:dbl[])
                n1751 = Build Array(w3043, w3048, w3069, w3068, w3067, 2.0 ("t")) -> (w3062:dbl[])
                n1752 = Round Toward +Infinity(x=w3050) -> (ceil(x): smallest int >= x=w3051:dbl)
                n1753 = Build Array (concatenate)(w3062, w3061, w3044, w3060) -> (w3059:dbl[])
                n1754 = To Unsigned Long Integer(number=w3051) -> (unsigned 32bit integer=w3049:u32)
              }
              frame 8 {
                w3079 = 0.0 ("f")
                # "MCL raster scan"
                n1755 = local read "Number of scans (MCL)"() -> (w3074:u64)
                n1756 = local read "Scan lines (y)"() -> (w3073:u64)
                n1757 = local read "2D or 1D Scan"() -> (w3076:bool)
                n1758 = local read "Scan Range (V)\n(of steps)"() -> (w3095:dbl)
                n1759 = local read "Fast Scan Dir"() -> (w3102:bool)
                n1760 = local read "Cycles/step (MCL)"() -> (w3092:u64)
                n1761 = local read "Scan steps (MCL)"() -> (w3094:u64)
                n1762 = Select(t=w3073, s=w3076, f=w3074) -> (s? t:f=w3075:u64)
                n1763 = Boolean To (0,1)(Boolean=w3076) -> (0, 1=w3078:i16)
                n1764 = local read "Save ave N"() -> (w3107:dbl)
                n1765 = local read "Initial X"() -> (w3081:dbl)
                n1766 = local read "Initial Y"() -> (w3080:dbl)
                n1767 = To Double Precision Float(number=w3078) -> (double precision float=w3077:dbl)
                n1768 = Boolean To (0,1)(Boolean=w3102) -> (0, 1=w3101:i16)
                n1769 = To Double Precision Float(number=w3075) -> (double precision float=w3090:dbl)
                n1770 = To Double Precision Float(number=w3094) -> (double precision float=w3093:dbl)
                n1771 = To Double Precision Float(number=w3092) -> (double precision float=w3091:dbl)
                n1772 = To Double Precision Float(number=w3101) -> (double precision float=w3100:dbl)
                n1773 = Multiply(x=w3107, y=w3086) -> (x*y=w3106:dbl)
                n1774 = To Double Precision Float(number=w3071) -> (double precision float=w3085:dbl)
                n1775 = local read "N sets should be saved (MCL)"() -> (w3088:dbl)
                n1776 = Build Array(w3085, w3077, w3079, w3079, w3079) -> (w3083:dbl[])
                n1777 = Build Array(w3100, w3095, w3093, w3091, w3090, w3081, w3080) -> (w3097:dbl[])
                n1778 = Build Array(w3082, w3086, w3106, w3105, w3104, 3.0 ("t")) -> (w3099:dbl[])
                n1779 = Round Toward +Infinity(x=w3088) -> (ceil(x): smallest int >= x=w3089:dbl)
                n1780 = Build Array (concatenate)(w3099, w3098, w3083, w3097) -> (w3096:dbl[])
                n1781 = To Unsigned Long Integer(number=w3089) -> (unsigned 32bit integer=w3087:u32)
              }
            }
            n1782 = local read "Index"() -> (w2946:dbl)
            n1783 = call "Create new save file.vi"("Insert"="", "Ext"=".dat", "Index In"=w2946) -> ("Path Out"=w2905:path, "Index Out"=w2918:dbl)
            n1784 = local write "Save file name"(w2905) -> ()
            n1785 = local write "Index"(w2918) -> ()
            n1786 = local write "Save index"(w2918) -> ()
            n1787 = Array Size(array=w2929) -> (size(s)=w2930:i32)
            n1788 = Open/Create/Replace File(file path (use dialog)=w2905, operation (0:open)=T25."create", access (0:read/write)=enum16{"read/write", "read-only", "write-only"}."write-only") -> (refnum out=w2943:refnum<file>)  [unwired: 1 in, 4 out]
            n1789 = local write "Saving..."(TRUE ("Saving...")) -> ()
            n1790 = To Double Precision Float(number=w2930) -> (double precision float=w2928:dbl)
            n1791 = String Length(string="Comment (data description)") -> (length=w2926:i32)
            n1792 = To Double Precision Float(number=w2926) -> (double precision float=w2925:dbl)
            n1793 = Deny Access(7:w2943) -> (3:w2942:refnum<file>)  [unwired: 1 in, 2 out]
            n1794 = Build Array (concatenate)(w2928, w2929, w2925) -> (w2927:dbl[])
            n1795 = case "If fluorescence data to be saved" shown="True" w2916 {
              tunnel: w2905 -> [_ w2995]
              tunnel: [refnum<k0> refnum w2975] -> w2917
              frame False {
              }
              frame True {
                w2974 = 0.0
                n1796 = local read "APD Integration Time (s)"() -> (w2980:dbl)
                n1797 = local read "N APD Samp/step"() -> (w2973:dbl)
                n1798 = Path To String(path=w2995) -> (string=w2994:string)
                n1799 = String Length(string=w2994) -> (length=w2993:i32)
                n1800 = Subtract(x=w2993, y=4) -> (x-y=w2991:i32)
                n1801 = String Subset(string=w2994, length (rest)=w2991) -> (substring=w2990:string)  [unwired: 1 out]
                n1802 = Build Array(w2980, w2973, w2974, w2974, w2974, w2974, w2974, w2974) -> (w2977:dbl[])
                n1803 = Concatenate Strings(w2990, "_fl.dat" ("string")) -> (w2988:string)
                n1804 = Array Size(array=w2977) -> (size(s)=w2979:i32)
                n1805 = String To Path(string=w2988) -> (path=w2984:path)
                n1806 = Open/Create/Replace File(file path (use dialog)=w2984, operation (0:open)=T25."create", access (0:read/write)=enum16{"read/write", "read-only", "write-only"}."write-only") -> (refnum out=w2985:refnum<file>)  [unwired: 1 in, 4 out]
                n1807 = Deny Access(7:w2985) -> (3:w2981:refnum<file>)  [unwired: 1 in, 2 out]
                n1808 = To Double Precision Float(number=w2979) -> (double precision float=w2978:dbl)
                n1809 = Build Array (concatenate)(w2978, w2977) -> (w2976:dbl[])
                n1810 = Write to Binary File(file (use dialog)=w2981, data=w2976, 5:FALSE ("prepend array or string size? (T)"), 9:T24."big-endian, network order" ("byte order (0:big-endian, network order)")) -> (refnum out=w2975:refnum<file>)  [unwired: 1 in, 3 out]
              }
            }
            n1811 = case shown="True" w2903 {
              tunnel: w2905 -> [_ w2957]
              tunnel: [refnum<k0> refnum w2956] -> w2904
              frame False {
              }
              frame True {
                w2952 = 0.0 ("element")
                n1812 = Path To String(path=w2957) -> (string=w2971:string)
                n1813 = Build Array(w2952, w2952, w2952, w2952, w2952, w2952, w2952, w2952) -> (w2953:dbl[])
                n1814 = String Length(string=w2971) -> (length=w2970:i32)
                n1815 = Subtract(x=w2970, y=4) -> (x-y=w2968:i32)
                n1816 = Array Size(array=w2953) -> (size(s)=w2955:i32)
                n1817 = String Subset(string=w2971, length (rest)=w2968) -> (substring=w2967:string)  [unwired: 1 out]
                n1818 = To Double Precision Float(number=w2955) -> (double precision float=w2954:dbl)
                n1819 = Concatenate Strings(w2967, "_pos.dat" ("string")) -> (w2965:string)
                n1820 = Build Array (concatenate)(w2954, w2953) -> (w2951:dbl[])
                n1821 = String To Path(string=w2965) -> (path=w2961:path)
                n1822 = Open/Create/Replace File(file path (use dialog)=w2961, operation (0:open)=T25."create", access (0:read/write)=enum16{"read/write", "read-only", "write-only"}."write-only") -> (refnum out=w2962:refnum<file>)  [unwired: 1 in, 4 out]
                n1823 = Deny Access(7:w2962) -> (3:w2958:refnum<file>)  [unwired: 1 in, 2 out]
                n1824 = Write to Binary File(file (use dialog)=w2958, data=w2951, 5:FALSE ("prepend array or string size? (T)"), 9:T24."big-endian, network order" ("byte order (0:big-endian, network order)")) -> (refnum out=w2956:refnum<file>)  [unwired: 1 in, 3 out]
              }
            }
            n1825 = Write to Binary File(file (use dialog)=w2942, data=w2927, 5:w2923, 9:w2921) -> (refnum out=w2924:refnum<file>)  [unwired: 1 in, 3 out]
            n1826 = Write to Binary File(file (use dialog)=w2924, data="Comment (data description)", 5:w2923, 9:w2921) -> (refnum out=w2920:refnum<file>)  [unwired: 1 in, 3 out]
          }
        }
        n1827 = feedback-in #19(w2863) -> ()
        n1828 = feedback-in #20(w2890) -> ()
        n1829 = feedback-in #21(w2862) -> ()
        n1830 = feedback-in #22(w2873) -> ()
        n1831 = feedback-in #23(w2876) -> ()
        n1832 = feedback-in #24(w2889) -> ()
        n1833 = feedback-in #25(w2879) -> ()
      }
      frame #1 {
        n1834 = local read "Saving..."() -> (w3120:bool)
        n1835 = case shown="True" w3120 {
          tunnel: w3124 -> [_ w3134]
          tunnel: w3123 -> [_ w3148]
          tunnel: w3122 -> [_ w3144]
          tunnel: w3121 -> [_ w3143]
          tunnel: w3119 -> [_ w3142]
          tunnel: w3118 -> [_ w3137]
          tunnel: w3117 -> [_ w3136]
          tunnel: w3116 -> [_ w3135]
          tunnel: w3115 -> [_ w3133]
          tunnel: w3114 -> [_ w3131]
          tunnel: w3113 -> [_ w3130]
          tunnel: w3112 -> [_ w3129]
          tunnel: w3111 -> [_ w3128]
          tunnel: w3110 -> [_ w3127]
          tunnel: w3109 -> [_ w3126]
          tunnel: w3108 -> [_ w3125]
          frame False {
          }
          frame True {
            n1836 = Multiply(x=w3134, y=w3133) -> (x*y=→"Time (s)":dbl)
            n1837 = Less Or Equal?(x=w3134, y=w3142) -> (x <= y?=w3146:bool)
            n1838 = Or(x="Stop Saving", y="Abort save 2") -> (x .or. y?=w3138:bool)
            n1839 = Not(x=w3138) -> (.not. x?=w3147:bool)
            n1840 = And(x=w3146, y=w3147) -> (x .and. y?=w3145:bool)
            n1841 = case shown="True" w3145 {
              tunnel: w3148 -> [w3155 w3223]
              tunnel: [0.0 w3226] -> w3141
              tunnel: w3134 -> [_ w3224]
              tunnel: w3142 -> [_ w3225]
              tunnel: w3144 -> [_ w3220]
              tunnel: w3143 -> [_ _]
              tunnel: w3137 -> [w3153 w3213]
              tunnel: w3136 -> [w3152 w3214]
              tunnel: w3135 -> [_ w3212]
              tunnel: w3131 -> [_ w3211]
              tunnel: w3130 -> [_ w3165]
              tunnel: w3129 -> [_ w3204]
              tunnel: w3128 -> [_ w3182]
              tunnel: w3127 -> [w3149 w3163]
              tunnel: w3126 -> [w3150 w3162]
              tunnel: w3125 -> [_ w3159]
              frame False {
                w3151 = FALSE
                n1842 = Close File(refnum=w3155) -> ()  [unwired: 1 in, 2 out]
                n1843 = case shown="True" w3152 {
                  tunnel: w3153 -> [_ w3157]
                  frame False {
                  }
                  frame True {
                    n1844 = Close File(refnum=w3157) -> ()  [unwired: 1 in, 2 out]
                  }
                }
                n1845 = case shown="True" w3149 {
                  tunnel: w3150 -> [_ w3156]
                  frame False {
                  }
                  frame True {
                    n1846 = Close File(refnum=w3156) -> ()  [unwired: 1 in, 2 out]
                  }
                }
                n1847 = local write "Raster Scanning..."(w3151) -> ()
                n1848 = local write "Calibrating Trap..."(w3151) -> ()
                n1849 = call <vilib>:"Beep.vi"() -> ()  [unwired: 3 in, 9 out]
                n1850 = local write "Stop Saving"(w3151) -> ()
                "Saving..." <- w3151
              }
              frame True {
                n1851 = local read "Calibrating Trap..."() -> (w3215:bool)
                n1852 = case "Write fl. data" shown="True" w3214 {
                  tunnel: w3213 -> [_ w3249]
                  tunnel: w3212 -> [_ w3248]
                  frame False {
                  }
                  frame True {
                    n1853 = Write to Binary File(file (use dialog)=w3249, data=w3248, 5:FALSE ("prepend array or string size? (T)"), 9:T24."big-endian, network order" ("byte order (0:big-endian, network order)")) -> ()  [unwired: 1 in, 4 out]
                  }
                }
                n1854 = Greater?(x="Save ave N", y=1.0) -> (0:w3218:bool)
                n1855 = Not(x=w3215) -> (.not. x?=w3217:bool)
                n1856 = And(x=w3217, y=w3218) -> (x .and. y?=w3160:bool)
                n1857 = case shown="True" w3160 {
                  tunnel: w3159 -> [w3229 w3240]
                  tunnel: [w3229 w3232] -> w3158
                  tunnel: "Save ave N" -> [_ w3233]
                  frame False {
                  }
                  frame True {
                    w3230 = 2 ("dimension size")
                    n1858 = Array Size(array=w3240) -> (size(s)=w3234:i32)
                    n1859 = Divide(x=w3234, y=w3230) -> (x/y=w3238:dbl)
                    n1860 = Reshape Array(w3240, w3238, w3230) -> (w3239:u64[][])
                    n1861 = Transpose 2D Array(2D array=w3239) -> (transposed array=w3237:u64[][])
                    n1862 = for {
                      tunnel: w3237 -> [w3242] mode=indexing
                      tunnel: [w3241] -> w3231 mode=indexing
                      tunnel: w3233 -> [w3243]
                      workers-P: _ -> [_]
                      n1863 = call "downsample 1D array - U64.vi"("Ave N"=w3243, "Array In"=w3242) -> ("Array Out"=w3241:u64[])  [unwired: 1 in]
                    }
                    n1864 = Transpose 2D Array(2D array=w3231) -> (transposed array=w3236:u64[][])
                    n1865 = Divide(x=w3234, y=w3233) -> (x/y=w3235:dbl)
                    n1866 = Reshape Array(w3236, w3235) -> (w3232:u64[])
                  }
                }
                n1867 = case shown="True" w3160 {
                  tunnel: w3220 -> [w3252 w3264]
                  tunnel: [w3252 w3256] -> w3216
                  tunnel: "Save ave N" -> [_ w3257]
                  tunnel: w3211 -> [_ w3255]
                  frame False {
                  }
                  frame True {
                    n1868 = Array Size(array=w3264) -> (size(s)=w3258:i32)
                    n1869 = Array Size(array=w3255) -> (size(s)=w3254:i32)
                    n1870 = Divide(x=w3258, y=w3254) -> (x/y=w3262:dbl)
                    n1871 = Reshape Array(w3264, w3262, w3254) -> (w3263:i16[][])
                    n1872 = Transpose 2D Array(2D array=w3263) -> (transposed array=w3261:i16[][])
                    n1873 = for {
                      tunnel: w3261 -> [w3267] mode=indexing
                      tunnel: [w3266] -> w3253 mode=indexing
                      tunnel: w3257 -> [w3265]
                      workers-P: _ -> [_]
                      n1874 = call "downsample 1D array - I16.vi"("Ave N"=w3265, "Array In"=w3267) -> ("Array Out"=w3266:i16[])  [unwired: 1 out]
                    }
                    n1875 = Transpose 2D Array(2D array=w3253) -> (transposed array=w3260:i16[][])
                    n1876 = Divide(x=w3258, y=w3257) -> (x/y=w3259:dbl)
                    n1877 = Reshape Array(w3260, w3259) -> (w3256:i16[])
                  }
                }
                n1878 = Index Array(array=w3182, index=1) -> (element=w3185:waveform(dbl))
                n1879 = Index Array(array=w3182, index=0) -> (element=w3187:waveform(dbl))
                n1880 = Unbundle By Name(w3185) -> ("Y"=w3189:dbl[])
                n1881 = Unbundle By Name(w3187) -> ("Y"=w3197:dbl[])
                n1882 = case "Write trap pos. data" shown="True" w3163 {
                  tunnel: w3162 -> [_ w3245]
                  tunnel: w3158 -> [_ w3244]
                  frame False {
                  }
                  frame True {
                    n1883 = Write to Binary File(file (use dialog)=w3245, data=w3244, 5:FALSE ("prepend array or string size? (T)"), 9:T24."big-endian, network order" ("byte order (0:big-endian, network order)")) -> ()  [unwired: 1 in, 4 out]
                  }
                }
                n1884 = Write to Binary File(file (use dialog)=w3223, data=w3216, 5:FALSE ("prepend array or string size? (T)"), 9:T24."big-endian, network order" ("byte order (0:big-endian, network order)")) -> ()  [unwired: 1 in, 4 out]
                n1885 = feedback #26(w3189) -> (w3191:dbl[])
                n1886 = Build Array (concatenate)(w3191, w3189) -> (w3190:dbl[])
                n1887 = Select(t=w3189, s=w3165, f=w3190) -> (s? t:f=w3175:dbl[])
                n1888 = feedback-in #26(w3175) -> ()
                n1889 = feedback #27(w3197) -> (w3210:dbl[])
                n1890 = Build Array (concatenate)(w3210, w3197) -> (w3209:dbl[])
                n1891 = Select(t=w3197, s=w3165, f=w3209) -> (s? t:f=w3184:dbl[])
                n1892 = feedback-in #27(w3184) -> ()
                n1893 = Divide(x=w3224, y=w3225) -> (x/y=w3227:dbl)
                n1894 = Multiply(x=w3227, y=100.0) -> (x*y=w3226:dbl)
                n1895 = Build Array(w3184, w3175) -> (→"Saved APD":dbl[][])
                n1896 = Array Size(array=w3184) -> (size(s)=w3202:i32)
                n1897 = Unbundle By Name(w3204) -> ("Y"=w3208:dbl[])
                n1898 = Subtract(x=w3202, y="N pts to average") -> (x-y=w3178:i32)
                n1899 = Multiply(x="N pts to average", y=u16 2) -> (x*y=w3179:u16)
                n1900 = Subtract(x=w3202, y=w3179) -> (x-y=w3177:i32)
                n1901 = feedback #28(w3208) -> (w3207:dbl[])
                n1902 = Build Array (concatenate)(w3207, w3208) -> (w3206:dbl[])
                n1903 = Select(t=w3208, s=w3165, f=w3206) -> (s? t:f=w3205:dbl[])
                "Trap Delta Graph" <- w3205
                n1904 = feedback-in #28(w3205) -> ()
                n1905 = Array Subset(array=w3184, index=w3178, length="N pts to average") -> (w3201:dbl[])
                n1906 = Array Subset(array=w3184, index=w3177, length="N pts to average") -> (w3200:dbl[])
                n1907 = Array Subset(array=w3175, index=w3178, length="N pts to average") -> (w3181:dbl[])
                n1908 = Array Subset(array=w3175, index=w3177, length="N pts to average") -> (w3180:dbl[])
                n1909 = call-poly <vilib>:"Mean.vi"("X"=w3201) -> ("mean"=w3199:dbl)  [unwired: 1 out]
                n1910 = call-poly <vilib>:"Mean.vi"("X"=w3181) -> ("mean"=w3174:dbl)  [unwired: 1 out]
                n1911 = call-poly <vilib>:"Mean.vi"("X"=w3200) -> ("mean"=w3198:dbl)  [unwired: 1 out]
                n1912 = call-poly <vilib>:"Mean.vi"("X"=w3180) -> ("mean"=w3173:dbl)  [unwired: 1 out]
                n1913 = Subtract(x=w3174, y=w3173) -> (x-y=w3164:dbl)
                "Delta Fl. 2" <- w3164
                n1914 = Subtract(x=w3199, y=w3198) -> (x-y=w3196:dbl)
                "Delta Fl. 1" <- w3196
                n1915 = Initialize Array(w3196, 1 ("dimension size")) -> (w3193:dbl[])
                n1916 = Initialize Array(w3164, 1 ("dimension size")) -> (w3170:dbl[])
                n1917 = feedback #29(w3193) -> (w3194:dbl[])
                n1918 = Build Array (concatenate)(w3194, w3193) -> (w3192:dbl[])
                n1919 = feedback #30(w3170) -> (w3171:dbl[])
                n1920 = Build Array (concatenate)(w3171, w3170) -> (w3169:dbl[])
                n1921 = Select(t=w3193, s=w3165, f=w3192) -> (s? t:f=w3168:dbl[])
                n1922 = feedback-in #29(w3168) -> ()
                n1923 = Select(t=w3170, s=w3165, f=w3169) -> (s? t:f=w3167:dbl[])
                n1924 = feedback-in #30(w3167) -> ()
                n1925 = Build Array(w3168, w3167) -> (→"Save APD Deriv":dbl[][])
              }
            }
            "Progress" <- w3141
            "Progress 2" <- w3141
          }
        }
      }
    }
    n1926 = Bundle By Name(cluster=w1945, "Green FB Ch 0"=w1944, "Green FB Ch 1"=w1943) -> (w1923:T42)
    "Green FB Signals (V)" <- w1923
    n1927 = Unbundle By Name(w1923) -> ("Green FB Ch 2"=→"Green FB Plot":dbl)
    n1928 = local read "wait to reset values"() -> (w2015:bool)
    n1929 = Not(x=w2012) -> (.not. x?=w2016:bool)
    n1930 = And(x=w2016, y=w2015) -> (x .and. y?=w2017:bool)
    n1931 = case "Part of MCL raster scanning: returns to initial positions after scan done" shown="True" w2017 {
      tunnel: w2020 -> [w2683 w2690]
      tunnel: [w2683 w2689] -> w2019
      tunnel: w2014 -> [w2682 w2688]
      tunnel: [w2682 w2687] -> w2013
      frame False {
      }
      frame True {
        w2698 = 10.0 ("y")
        w2697 = 32767.0 ("y")
        # "to return scan values\nafter a synchronous \nAOM scan"
        n1932 = local read "AO2"() -> (w2691:dbl)
        n1933 = local read "AO1"() -> (w2692:dbl)
        n1934 = local write "wait to reset values"(FALSE ("wait to reset values")) -> ()
        n1935 = Multiply(x=w2692, y=w2697) -> (x*y=w2694:dbl)
        n1936 = Multiply(x=w2691, y=w2697) -> (x*y=w2696:dbl)
        n1937 = Divide(x=w2694, y=w2698) -> (x/y=w2693:dbl)
        n1938 = Divide(x=w2696, y=w2698) -> (x/y=w2695:dbl)
        n1939 = To Word Integer(number=w2693) -> (16bit integer=w2699:i16)
        n1940 = To Word Integer(number=w2695) -> (16bit integer=w2700:i16)
        n1941 = local read "Total Counts (ticks)"() -> (w2684:u32)
        n1942 = xnode "Read/Write Control"("FPGA VI Reference In"=w2690, "error in"=w2688, "AO1"=w2699, "AO2"=w2700, "MCL count"=w2684) -> ("FPGA VI Reference Out"=w2689:T19, "error out"=w2687:errorcluster)
        n1943 = local read "Scan Range (V)\n(of steps)"() -> (w2685:dbl)
        n1944 = property on="Scan Range (V)\n(of steps)" class="DigNum (strict)"("Val(Sgnl)"=w2685) -> ()  [unwired: 2 in, 2 out]
      }
    }
    n1945 = node-c288() -> ()  [unwired: 2 out]
  }
  n1946 = timed-loop "Mouse control: trap position (AOM deflection), set confocal spot from image" {
    tunnel: [w3269] -> w168
    tunnel: w36 -> [w3268]
    timing: w80 -> [_]
    timing-out: [_] -> w79
    stop <- w3269 stop-if-true
    n1947 = node-c288() -> ()  [unwired: 2 out]
    n1948 = event shown="[0] \"Pane\": Mouse Down" {
      selector: _ -> [_ _]
      dyn-events: _ -> [_ _]
      timeout: _ -> [_ _]
      tunnel: w3268 -> [w3272 _]
      event Mouse Down {
        n1949 = event-data() -> ("Time"=w3274:u32, "Coords"=w3273:T7, "Button"=w3275:u16)  [unwired: 6 out]
        n1950 = case shown="1" w3275 {
          tunnel: w3274 -> [_ _ w3378]
          tunnel: w3273 -> [_ w3312 w3376]
          tunnel: w3272 -> [_ _ w3374]
          frame 0, Default {
          }
          frame 1 {
            n1951 = property on="APD 2" class="ImageControl"() -> ("Displayed Image Position"=w3282:cluster{"Left":i32, "Top":i32})  [unwired: 2 in, 2 out]
            n1952 = property on="APD 1" class="ImageControl"() -> ("Displayed Image Position"=w3311:cluster{"Left":i32, "Top":i32})  [unwired: 2 in, 2 out]
            n1953 = property on="Detection Laser X" class="ImageControl"() -> ("Displayed Image Position"=w3308:cluster{"Left":i32, "Top":i32})  [unwired: 2 in, 2 out]
            n1954 = property on="Detection Laser Y" class="ImageControl"() -> ("Displayed Image Position"=w3307:cluster{"Left":i32, "Top":i32})  [unwired: 2 in, 2 out]
            n1955 = property on="APD 2" class="ImageControl"() -> ("Displayed Image Size"=w3281:cluster{"Width":u32, "Height":u32})  [unwired: 2 in, 2 out]
            n1956 = property on="APD 1" class="ImageControl"() -> ("Displayed Image Size"=w3309:cluster{"Width":u32, "Height":u32})  [unwired: 2 in, 2 out]
            n1957 = property on="Detection Laser X" class="ImageControl"() -> ("Displayed Image Size"=w3310:cluster{"Width":u32, "Height":u32})  [unwired: 2 in, 2 out]
            n1958 = property on="Detection Laser Y" class="ImageControl"() -> ("Displayed Image Size"=w3306:cluster{"Width":u32, "Height":u32})  [unwired: 2 in, 2 out]
            n1959 = Unbundle By Name(w3281) -> ("Width"=w3278:u32, "Height"=w3277:u32)
            n1960 = Unbundle By Name(w3282) -> ("Left"=w3280:i32, "Top"=w3279:i32)
            n1961 = Unbundle By Name(w3309) -> ("Width"=w3303:u32, "Height"=w3302:u32)
            n1962 = Unbundle By Name(w3310) -> ("Width"=w3299:u32, "Height"=w3298:u32)
            n1963 = Unbundle By Name(w3306) -> ("Width"=w3295:u32, "Height"=w3294:u32)
            n1964 = Unbundle By Name(w3311) -> ("Left"=w3305:i32, "Top"=w3304:i32)
            n1965 = Unbundle By Name(w3308) -> ("Left"=w3301:i32, "Top"=w3300:i32)
            n1966 = Unbundle By Name(w3307) -> ("Left"=w3297:i32, "Top"=w3296:i32)
            n1967 = Bundle("Left"=w3280, "Top"=w3279, "Width"=w3278, "Height"=w3277) -> (w3276:T43)  [unwired: 1 in]
            n1968 = Bundle("Left"=w3305, "Top"=w3304, "Width"=w3303, "Height"=w3302) -> (w3293:T43)  [unwired: 1 in]
            n1969 = Bundle("Left"=w3301, "Top"=w3300, "Width"=w3299, "Height"=w3298) -> (w3292:T43)  [unwired: 1 in]
            n1970 = Bundle("Left"=w3297, "Top"=w3296, "Width"=w3295, "Height"=w3294) -> (w3291:T43)  [unwired: 1 in]
            n1971 = Build Cluster Array(w3276, w3293, w3292, w3291) -> (w3290:T44)
            n1972 = for {
              tunnel: w3312 -> [w3323]
              tunnel: w3290 -> [w3324] mode=indexing
              shift-right: [w3321] -> w3288
              shift-left: TRUE -> [w3322]
              shift-right: [w3320] -> w3286
              shift-left: _ -> [w3316]
              shift-right: [w3319] -> w3285
              shift-left: _ -> [w3315]
              shift-right: [w3318] -> w3284
              shift-left: _ -> [w3314]
              shift-right: [w3317] -> w3283
              shift-left: _ -> [w3313]
              n1973 = case shown="True" w3322 {
                selector: w3322 -> [w3329 _]
                tunnel: w3324 -> [_ w3338]
                tunnel: w3323 -> [_ w3336]
                tunnel: [w3329 w3334] -> w3321
                tunnel: [w3328 w3333] -> w3320
                tunnel: [w3327 w3332] -> w3319
                tunnel: [w3326 w3331] -> w3318
                tunnel: [w3325 w3330] -> w3317
                tunnel: w3316 -> [w3328 _]
                tunnel: w3315 -> [w3327 _]
                tunnel: w3314 -> [w3326 _]
                tunnel: w3313 -> [w3325 _]
                frame False {
                }
                frame True {
                  n1974 = Unbundle(w3338) -> (w3337:T43)
                  n1975 = call "isclickinwindow.vi"("Image Param"=w3337, "Point32"=w3336) -> ("4 Y"=w3330:i32, "3 Height"=w3331:i32, "2 X"=w3332:i32, "1 Width"=w3333:i32, "In image?"=w3335:bool)  [unwired: 1 in]
                  n1976 = Not(x=w3335) -> (.not. x?=w3334:bool)
                }
              }
            }
            n1977 = Not(x=w3288) -> (.not. x?=w3287:bool)
            n1978 = case shown="True" w3287 {
              tunnel: w3285 -> [_ w3351]
              tunnel: w3283 -> [_ w3350]
              tunnel: w3286 -> [_ w3349]
              tunnel: w3284 -> [_ w3348]
              frame False {
              }
              frame True {
                w3344 = FALSE ("Get Point")
                n1979 = local read "Scan lines (y)"() -> (w3353:u64)
                n1980 = local read "Actual MCL Inc (V)"() -> (w3345:dbl)
                n1981 = local read "Scan steps (MCL)"() -> (w3352:u64)
                n1982 = Divide "Y Pix/step"(x=w3348, y=w3353) -> (x/y=w3360:dbl)
                n1983 = Divide "Y V/pix"(x=w3345, y=w3360) -> (x/y=w3359:dbl)
                n1984 = Divide "Y half step offset"(x=w3345, y=2.0) -> (x/y=w3361:dbl)
                n1985 = Divide "X pix/step"(x=w3349, y=w3352) -> (x/y=w3358:dbl)
                n1986 = Negate(x=w3361) -> (-x=w3362:dbl)
                n1987 = local read "Initial Y"() -> (w3368:dbl)
                n1988 = Multiply(x=w3350, y=w3359) -> (x*y=w3369:dbl)
                n1989 = Divide "X half step offset"(x=w3345, y=2.0) -> (x/y=w3355:dbl)
                n1990 = Divide "X V/pix"(x=w3345, y=w3358) -> (x/y=w3357:dbl)
                n1991 = Multiply(x=w3345, y=w3352) -> (x*y=w3364:dbl)
                n1992 = Compound Arithmetic op=ADD(w3362, w3369, w3368) -> (w3346:dbl)
                "Pointer Y (V)" <- w3346
                n1993 = Multiply(x=w3357, y=w3351) -> (x*y=w3366:dbl)
                n1994 = Negate(x=w3355) -> (-x=w3354:dbl)
                n1995 = local read "Initial X"() -> (w3367:dbl)
                n1996 = Negate(x=w3366) -> (-x=w3365:dbl)
                n1997 = Compound Arithmetic op=ADD(w3354, w3364, w3367, w3365) -> (w3347:dbl)
                "Pointer X (V)" <- w3347
                n1998 = Or(x="Set X Only", y="Set Confocal Spot (X-Y)") -> (x .or. y?=w3340:bool)
                n1999 = Or(x="Set Confocal Spot (X-Y)", y="Set Y Only") -> (x .or. y?=w3339:bool)
                n2000 = case shown="True" w3340 {
                  tunnel: w3347 -> [_ w3370]
                  frame False {
                  }
                  frame True {
                    n2001 = property on="AO2" class="Slide (strict)"("Val(Sgnl)"=w3370) -> ()  [unwired: 2 in, 2 out]
                  }
                }
                n2002 = case shown="True" w3339 {
                  tunnel: w3346 -> [_ w3371]
                  frame False {
                  }
                  frame True {
                    n2003 = property on="AO1" class="Slide (strict)"("Val(Sgnl)"=w3371) -> ()  [unwired: 2 in, 2 out]
                  }
                }
                n2004 = local write "Set Confocal Spot (X-Y)"(w3344) -> ()
                n2005 = local write "Set X Only"(w3344) -> ()
                n2006 = local write "Set Y Only"(w3344) -> ()
              }
            }
          }
          frame 3 {
            n2007 = local read "BD 2 Frequency 1 (MHz)"() -> (w3372:dbl)
            n2008 = local read "BD 1 Frequency 1 (MHz)"() -> (w3373:dbl)
            n2009 = local write "Manipulating Trap"(TRUE ("Manipulating Trap")) -> ()
            n2010 = local write "Coords"(T7 {"Horizontal"=0, "Vertical"=0} ("Coords")) -> ()
            n2011 = while {
              tunnel: w3378 -> [w3383]
              tunnel: w3376 -> [w3382]
              tunnel: w3374 -> [w3381]
              tunnel: w3373 -> [w3380]
              tunnel: w3372 -> [w3379]
              stop <- w3384 stop-if-true
              n2012 = event shown="[0] \"Pane\": Mouse Move" {
                selector: _ -> [_ _]
                dyn-events: _ -> [_ _]
                timeout: _ -> [_ _]
                tunnel: ["Force Manip Abort" w3448] -> w3384
                tunnel: w3383 -> [w3391 _]
                tunnel: w3382 -> [w3389 _]
                tunnel: w3381 -> [w3388 _]
                tunnel: w3380 -> [w3387 _]
                tunnel: w3379 -> [w3386 _]
                event Mouse Move {
                  n2013 = event-data() -> ("Time"=w3392:u32, "Coords"=w3393:T7)  [unwired: 3 out]
                  n2014 = Less?(x=w3392, y=w3391) -> (x < y?=w3390:bool)
                  n2015 = case "Makes sure old motion events prior to mouse click aren't used" shown="False" w3390 {
                    tunnel: w3393 -> [w3435 _]
                    tunnel: w3389 -> [w3436 _]
                    tunnel: w3388 -> [w3413 _]
                    tunnel: w3387 -> [w3409 _]
                    tunnel: w3386 -> [w3408 _]
                    frame False {
                      n2016 = Subtract(x=w3435, y=w3436) -> (x-y=w3434:T7)
                      "Coords" <- w3434
                      n2017 = local read "Y RF Frequency Limits (MHz)"() -> (w3394:T16)
                      n2018 = To Double Precision Float(number=w3434) -> (double precision float=w3433:cluster{"Horizontal":dbl, "Vertical":dbl})
                      n2019 = Multiply(x=cluster{"Horizontal":dbl, "Vertical":dbl} {"Horizontal"=-1.0, "Vertical"=1.0}, y="Manipulation Scaling") -> (x*y=w3429:cluster{"Horizontal":dbl, "Vertical":dbl})
                      n2020 = local read "X RF Frequency Limits (MHz)"() -> (w3395:T16)
                      n2021 = Multiply(x=w3433, y=w3429) -> (x*y=w3431:cluster{"Horizontal":dbl, "Vertical":dbl})
                      n2022 = Unbundle By Name(w3431) -> ("Horizontal"=w3426:dbl, "Vertical"=w3430:dbl)
                      n2023 = Unbundle By Name(w3394) -> ("Maximum"=w3397:dbl, "Minimum"=w3396:dbl)
                      n2024 = Boolean To (0,1)(Boolean="Manip. X?") -> (0, 1=w3424:i16)
                      n2025 = Boolean To (0,1)(Boolean="Manip. Y?") -> (0, 1=w3421:i16)
                      n2026 = local read "BD 1 Frequency 2 (MHz)"() -> (w3411:dbl)
                      n2027 = Multiply(x=w3430, y=w3421) -> (x*y=w3423:dbl)
                      n2028 = Multiply(x=w3424, y=w3426) -> (x*y=w3427:dbl)
                      n2029 = local read "BD 2 Frequency 2 (MHz)"() -> (w3410:dbl)
                      n2030 = Unbundle By Name(w3395) -> ("Maximum"=w3399:dbl, "Minimum"=w3398:dbl)
                      n2031 = Add(x=w3408, y=w3423) -> (x+y=w3401:dbl)
                      n2032 = Add(x=w3409, y=w3427) -> (x+y=w3403:dbl)
                      n2033 = In Range and Coerce(upper limit=w3399, x=w3403, lower limit=w3398) -> (coerced(x)=w3402:dbl)  [unwired: 1 out]
                      n2034 = In Range and Coerce(upper limit=w3397, x=w3401, lower limit=w3396) -> (coerced(x)=w3400:dbl)  [unwired: 1 out]
                      n2035 = Subtract(x=w3402, y=w3411) -> (x-y=w3420:dbl)
                      n2036 = Subtract(x=w3400, y=w3410) -> (x-y=w3419:dbl)
                      n2037 = Square(x=w3420) -> (x^2=w3418:dbl)
                      n2038 = Square(x=w3419) -> (x^2=w3417:dbl)
                      n2039 = Add(x=w3418, y=w3417) -> (x+y=w3416:dbl)
                      n2040 = Square Root(x=w3416) -> (sqrt(x)=w3412:dbl)
                      n2041 = In Range and Coerce(upper limit="Limit Max (MHz)", x=w3412, lower limit="Limit Min (MHz)") -> (In Range?=w3405:bool)  [unwired: 1 out]
                      n2042 = Not(x="Limits Enable") -> (.not. x?=w3404:bool)
                      n2043 = Or(x=w3405, y=w3404) -> (x .or. y?=w3406:bool)
                      n2044 = case shown="True" w3406 {
                        tunnel: w3413 -> [_ w3446]
                        tunnel: w3412 -> [_ w3437]
                        tunnel: w3402 -> [_ w3444]
                        tunnel: w3411 -> [_ w3443]
                        tunnel: w3400 -> [_ w3442]
                        tunnel: w3410 -> [_ w3441]
                        tunnel: w3395 -> [_ w3439]
                        tunnel: w3394 -> [_ w3438]
                        frame False {
                        }
                        frame True {
                          n2045 = local read "BD 1 Frequency 3 (MHz)"() -> (w3445:dbl)
                          n2046 = local read "BD 2 Frequency 3 (MHz)"() -> (w3440:dbl)
                          n2047 = local write "Trap Delta (MHz)"(w3437) -> ()
                          n2048 = call "set RF board frequency - interlace.vi"("Board 2 Frequency Limits"=w3438, "Board 1 Frequency Limits"=w3439, "FPGA VI Reference In"=w3446, "Board 2 Frequency 3 (MHz)"=w3440, "Board 1 Frequency 3 (MHz)"=w3445, "Board 2 Frequency 2 (MHz)"=w3441, "Board 2 Frequency 1 (MHz)"=w3442, "Board 1 Frequency 2 (MHz)"=w3443, "Board 1 Frequency 1  (MHz)"=w3444) -> ()  [unwired: 1 in, 2 out]
                          n2049 = local write "BD 2 Frequency 1 (MHz)"(w3442) -> ()
                          n2050 = local write "BD 1 Frequency 1 (MHz)"(w3444) -> ()
                        }
                      }
                    }
                    frame True {
                    }
                  }
                }
                event Mouse Up {
                  n2051 = event-data() -> ("Button"=w3447:u16)  [unwired: 8 out]
                  n2052 = case shown="3" w3447 {
                    tunnel: [FALSE TRUE] -> w3448
                    frame 0, Default {
                    }
                    frame 3 {
                      n2053 = local read "Trap Delta (MHz)"() -> (w3450:dbl)
                      n2054 = property on="Initial delta (MHz)" class="DigNum (strict)"("Val(Sgnl)"=w3450) -> ()  [unwired: 2 in, 2 out]
                      n2055 = local write "Manipulating Trap"(FALSE ("Manipulating Trap")) -> ()
                    }
                  }
                }
              }
            }
          }
        }
      }
      event Mouse Move {
        n2056 = event-data() -> ()  [unwired: 6 out]
      }
    }
    n2057 = local read "Stop All"() -> (w3269:bool)
    n2058 = node-c288() -> ()  [unwired: 2 out]
  }
  n2059 = timed-loop "Oscillate AOD (debugging)" {
    tunnel: w36 -> [w3454]
    tunnel: [w3453] -> w81
    timing: w76 -> [_]
    timing-out: [_] -> w75
    stop <- w3453 stop-if-true
    n2060 = node-c288() -> ()  [unwired: 2 out]
    n2061 = event shown="[2] \"Trap Triggering\": Value Change" {
      selector: _ -> [_ _ _ _]
      dyn-events: _ -> [_ _ _ _]
      timeout: _ -> [_ _ _ _]
      tunnel: w3454 -> [w3461 _ _ _]
      tunnel: [FALSE ("Stop All") _ _ w3766] -> w3453
      event "Oscillate Set 1", "Fish for Tether": Value Change {
        n2062 = event-data() -> ()  [unwired: 6 out]
        n2063 = local read "Oscillate Set 1"() -> (w3460:bool)
        n2064 = Or(x=w3460, y="Fish for Tether") -> (x .or. y?=w3458:bool)
        n2065 = case shown="True" w3458 {
          tunnel: w3461 -> [_ w3463]
          tunnel: "Fish for Tether" -> [_ w3462]
          frame False {
          }
          frame True {
            n2066 = case shown="True" w3462 {
              frame False {
              }
              frame True {
                n2067 = local write "Scan axis 2"(TRUE) -> ()
                n2068 = local write "Tether"(FALSE ("Tether")) -> ()
              }
            }
            n2069 = node-c288() -> (w3465:T21)  [unwired: 4 out]
            n2070 = timed-loop "Oscillate AOD" {
              timing: w3465 -> [_]
              timing-out: [_] -> w3464
              tunnel: w3463 -> [w3475]
              tunnel: w3462 -> [w3474]
              i -> [w3477]
              stop <- w3473 stop-if-true
              n2071 = node-c288() -> (w3476:i64)  [unwired: 1 out]
              n2072 = flat-sequence {
                tunnel: w3477 -> [w3504]
                tunnel: w3476 -> [w3503]
                tunnel: w3475 -> [w3482]
                tunnel: w3474 -> [w3485]
                tunnel: [w3485] -> w3472
                tunnel: [w3484] -> w3471
                tunnel: [w3481] -> w3470
                tunnel: [w3478] -> w3468
                tunnel: w3472 -> [w3540]
                tunnel: w3471 -> [w3538]
                tunnel: w3470 -> [w3537]
                tunnel: [w3536] -> w3469
                tunnel: w3468 -> [w3535]
                tunnel: [w3603] -> w3473
                tunnel: w3469 -> [w3602]
                frame #0 {
                  n2073 = Divide(x=w3503, y=i64 1000) -> (x/y=w3498:dbl)
                  n2074 = Multiply(x=w3498, y=w3504) -> (x*y=w3500:dbl)
                  n2075 = local read "BD 1 Frequency 2 (MHz)"() -> (w3483:dbl)
                  n2076 = Multiply(x="Osc. freq. (Hz)", y=6.283185307179586) -> (x*y=w3501:dbl)
                  n2077 = Multiply(x=w3501, y=w3500) -> (x*y=w3480:dbl)
                  n2078 = local read "BD 1 Frequency 1 (MHz)"() -> (w3488:dbl)
                  n2079 = case shown="True" w3485 {
                    tunnel: w3480 -> [w3510 w3515]
                    tunnel: w3488 -> [_ w3526]
                    tunnel: w3483 -> [_ w3527]
                    tunnel: [w3507 w3521] -> w3486
                    tunnel: [FALSE w3518] -> w3481
                    tunnel: [0.0 w3511] -> w3478
                    frame False {
                      n2080 = Sine(x=w3510) -> (sin(x)=w3508:dbl)
                      n2081 = Multiply(x=w3508, y="Osc. amp. (MHz)") -> (x*y=w3507:dbl)
                    }
                    frame True {
                      n2082 = Cosine(x=w3515) -> (cos(x)=w3530:dbl)
                      n2083 = Subtract(x=w3527, y=w3526) -> (x-y=w3525:dbl)
                      n2084 = Decrement(x=w3530) -> (x-1=w3529:dbl)
                      n2085 = Subtract(x=w3525, y="Closest Delta (MHz)") -> (x-y=w3522:dbl)
                      n2086 = Divide(x=w3529, y=-2.0) -> (x/y=w3523:dbl)
                      n2087 = Multiply(x=w3523, y=w3522) -> (x*y=w3521:dbl)
                      n2088 = local read "Vec Mean of T1 T2"() -> (w3517:dbl[])
                      n2089 = Greater?(x=w3517, y="Stop F (pN)") -> (0:w3519:bool[])
                      n2090 = Or Array Elements(Boolean array=w3519) -> (logical OR=w3518:bool)
                      n2091 = Divide(x=w3515, y=6.283185307179586) -> (x/y=w3514:dbl)
                      n2092 = Round Toward +Infinity(x=w3514) -> (ceil(x): smallest int >= x=w3511:dbl)
                      "Attempts" <- w3511
                      n2093 = Greater?(x=w3511, y="Attempt Limit") -> (0:w3513:bool)
                      n2094 = case shown="True" w3513 {
                        frame False {
                        }
                        frame True {
                          n2095 = local write "Fish for Tether"(FALSE ("Fish for Tether")) -> ()
                          n2096 = call <vilib>:"Beep.vi"() -> ()  [unwired: 3 in, 9 out]
                          n2097 = local read "Messages"() -> (w3532:string)
                          n2098 = call "Update messages.vi"("Message to add"="Tether fishing timeout." ("Messages"), "Old message string"=w3532) -> ("New message string"=→"Messages":string)
                        }
                      }
                    }
                  }
                  n2099 = local read "BD 2 Frequency 1 (MHz)"() -> (w3487:dbl)
                  n2100 = Select(t=w3488, s="Scan axis 2", f=w3487) -> (s? t:f=w3491:dbl)
                  n2101 = Add(x=w3486, y=w3491) -> (x+y=w3484:dbl)
                  n2102 = Select(t=w3484, s="Scan axis 2", f=w3488) -> (s? t:f=w3494:dbl)
                  n2103 = Select(t=w3487, s="Scan axis 2", f=w3484) -> (s? t:f=w3493:dbl)
                  n2104 = local read "Y RF Frequency Limits (MHz)"() -> (w3489:T16)
                  n2105 = local read "X RF Frequency Limits (MHz)"() -> (w3490:T16)
                  n2106 = local read "BD 1 Frequency 3 (MHz)"() -> (w3497:dbl)
                  n2107 = local read "BD 2 Frequency 2 (MHz)"() -> (w3496:dbl)
                  n2108 = local read "BD 2 Frequency 3 (MHz)"() -> (w3495:dbl)
                  n2109 = call "set RF board frequency - interlace.vi"("Board 2 Frequency Limits"=w3489, "Board 1 Frequency Limits"=w3490, "FPGA VI Reference In"=w3482, "Board 2 Frequency 3 (MHz)"=w3495, "Board 1 Frequency 3 (MHz)"=w3497, "Board 2 Frequency 2 (MHz)"=w3496, "Board 2 Frequency 1 (MHz)"=w3493, "Board 1 Frequency 2 (MHz)"=w3483, "Board 1 Frequency 1  (MHz)"=w3494) -> ()  [unwired: 1 in, 2 out]
                }
                frame #1 {
                  n2110 = And(x=w3540, y=w3537) -> (x .and. y?=w3539:bool)
                  n2111 = case "Only if were fishing and now formed tether" shown="True" w3539 {
                    tunnel: w3538 -> [w3542 w3555]
                    tunnel: [w3541 w3554] -> w3536
                    tunnel: w3535 -> [_ w3550]
                    frame False {
                      n2112 = local read "Fish for Tether"() -> (w3541:bool)
                      n2113 = case shown="False" w3541 {
                        tunnel: w3542 -> [w3543 _]
                        frame False {
                          n2114 = property on="BD 1 Frequency 1 (MHz)" class="DigNum (strict)"("Val(Sgnl)"=w3543) -> ()  [unwired: 2 in, 2 out]
                        }
                        frame True {
                        }
                      }
                    }
                    frame True {
                      w3554 = FALSE ("Fish for Tether")
                      n2115 = call <vilib>:"Beep.vi"() -> ()  [unwired: 3 in, 9 out]
                      n2116 = Number To Decimal String(number=w3550, width (-)=i16 1) -> (decimal integer string=w3548:string)
                      n2117 = case shown="\"2\", \"3\", \"4\", \"5\", \"6\"" "Then..." {
                        selector: "Then..." -> [_ w3558]
                        tunnel: w3555 -> [w3557 _]
                        frame "1", Default {
                          n2118 = property on="BD 1 Frequency 1 (MHz)" class="DigNum (strict)"("Val(Sgnl)"=w3557) -> ()  [unwired: 2 in, 2 out]
                        }
                        frame "2", "3", "4", "5", "6" {
                          n2119 = flat-sequence {
                            tunnel: w3558 -> [w3560]
                            frame #0 {
                              n2120 = property on="Trap Delta (MHz)" class="DigNum (strict)"("Val(Sgnl)"="Move to Delta 1 (MHz)") -> ()  [unwired: 2 in, 2 out]
                            }
                            frame #1 {
                              n2121 = case shown="\"5\", \"6\"" w3560 {
                                selector: w3560 -> [w3563 w3573 _]
                                frame "3", "4" {
                                n2122 = flat-sequence {
                                tunnel: w3563 -> [w3564]
                                tunnel: [w3564] -> w3561
                                tunnel: [w3566] -> w3562
                                tunnel: w3561 -> [w3566]
                                tunnel: w3562 -> [w3570]
                                frame #0 {
                                n2123 = property on="Green Laser ON/Interlacing" class="Bool (strict)"("Val(Sgnl)"=TRUE ("Value (Signaling)")) -> ()  [unwired: 2 in, 2 out]
                                }
                                frame #1 {
                                n2124 = Multiply(x="Wait Before Save (s)", y=u32 1000 ("x")) -> (x*y=w3568:u32)
                                n2125 = Wait (ms)(milliseconds to wait=w3568) -> ()  [unwired: 1 out]
                                }
                                frame #2 {
                                n2126 = property on="Start Saving" class="Bool (strict)"("Value"=TRUE ("Start Saving")) -> ()  [unwired: 2 in, 2 out]
                                n2127 = case shown="\"4\"" w3570 {
                                frame Default {
                                }
                                frame "4" {
                                n2128 = property on="Fl. Triggered..." class="Bool (strict)"("Val(Sgnl)"=TRUE ("Value (Signaling)")) -> ()  [unwired: 2 in, 2 out]
                                }
                                }
                                }
                                }
                                }
                                frame "5", "6" {
                                n2129 = stacked-sequence {
                                tunnel: w3573 -> [_ _ _ _ _ _ _ _ w3590 _ _]
                                frame #0 {
                                n2130 = Replace Array Subset(array=u32[] [0] ("Index Values"), new element="Raster Set Upon Tether", index=0) -> (w3574:u32[])
                                n2131 = property on="Saved AOD Raster Scan Parameter Sets" class="Arr (strict)"("Index Values"=w3574) -> ()  [unwired: 2 in, 2 out]
                                }
                                frame #1 {
                                n2132 = Wait (ms)(milliseconds to wait=u32 500) -> ()  [unwired: 1 out]
                                }
                                frame #2 {
                                n2133 = property on="Load parameters" class="Bool (strict)"("Val(Sgnl)"=TRUE ("Value (Signaling)")) -> ()  [unwired: 2 in, 2 out]
                                }
                                frame #3 {
                                n2134 = Wait (ms)(milliseconds to wait=u32 500) -> ()  [unwired: 1 out]
                                }
                                frame #4 {
                                n2135 = property on="Trap Raster Scan" class="Bool (strict)"("Val(Sgnl)"=TRUE ("Value (Signaling)")) -> ()  [unwired: 2 in, 2 out]
                                }
                                frame #5 {
                                n2136 = Wait (ms)(milliseconds to wait=u32 2000) -> ()  [unwired: 1 out]
                                }
                                frame #6 {
                                n2137 = while {
                                stop <- w3585 stop-if-true
                                n2138 = local read "Raster Scanning..."() -> (w3584:bool)
                                n2139 = local read "Saving..."() -> (w3587:bool)
                                n2140 = Wait (ms)(milliseconds to wait=u32 100) -> ()  [unwired: 1 out]
                                n2141 = Not(x=w3587) -> (.not. x?=w3586:bool)
                                n2142 = Not(x=w3584) -> (.not. x?=w3583:bool)
                                n2143 = And(x=w3586, y=w3583) -> (x .and. y?=w3585:bool)
                                }
                                }
                                frame #7 {
                                n2144 = property on="Trap Delta (MHz)" class="DigNum (strict)"("Val(Sgnl)"="Move to Delta 2 (MHz)") -> ()  [unwired: 2 in, 2 out]
                                }
                                frame #8 {
                                n2145 = local read "Tether"() -> (w3591:bool)
                                n2146 = case shown="True" w3591 {
                                tunnel: w3590 -> [_ w3592]
                                frame False {
                                }
                                frame True {
                                n2147 = flat-sequence {
                                tunnel: w3592 -> [w3594]
                                frame #0 {
                                n2148 = Wait (ms)(milliseconds to wait=u32 500) -> ()  [unwired: 1 out]
                                }
                                frame #1 {
                                n2149 = case shown="\"6\"" w3594 {
                                frame Default {
                                }
                                frame "6" {
                                n2150 = property on="Green Laser ON/Interlacing" class="Bool (strict)"("Val(Sgnl)"=TRUE ("Green Laser ON/Interlacing")) -> ()  [unwired: 2 in, 2 out]
                                }
                                }
                                }
                                frame #2 {
                                n2151 = Wait (ms)(milliseconds to wait=u32 500) -> ()  [unwired: 1 out]
                                }
                                frame #3 {
                                n2152 = local write "Start Saving"("Save at end (5, 6)") -> ()
                                }
                                }
                                }
                                }
                                }
                                frame #9 {
                                n2153 = local read "Bead Sep. Int. Time (s)"() -> (w3600:dbl)
                                n2154 = Multiply(x=w3600, y=1000.0) -> (x*y=w3599:dbl)
                                n2155 = Wait (ms)(milliseconds to wait=w3599) -> ()  [unwired: 1 out]
                                }
                                frame #10 {
                                n2156 = property on="Rescale on Mean" class="Bool (strict)"("Val(Sgnl)"=TRUE ("Value (Signaling)")) -> ()  [unwired: 2 in, 2 out]
                                }
                                }
                                }
                                frame "2", Default {
                                }
                              }
                            }
                          }
                        }
                      }
                      n2157 = Concatenate Strings("Formed tether in ", w3548, " attempt(s)." ("string")) -> (w3545:string)
                      n2158 = local read "Messages"() -> (w3552:string)
                      n2159 = local write "Fish for Tether"(w3554) -> ()
                      n2160 = call "Update messages.vi"("Message to add"=w3545, "Old message string"=w3552) -> ("New message string"=w3551:string)
                      n2161 = local write "Messages"(w3551) -> ()
                      n2162 = Get Date/Time In Seconds() -> (seconds since 1Jan1904=→"Time tether formed":timestamp)
                      "Tether" <- "Tether Alarm?"
                    }
                  }
                }
                frame #2 {
                  n2163 = local read "Oscillate Set 1"() -> (w3607:bool)
                  n2164 = local read "Stop All"() -> (w3605:bool)
                  n2165 = Or(x=w3607, y=w3602) -> (x .or. y?=w3604:bool)
                  n2166 = Not(x=w3604) -> (.not. x?=w3606:bool)
                  n2167 = Compound Arithmetic op=OR(w3605, w3606) -> (w3603:bool)
                }
              }
              n2168 = node-c288() -> ()  [unwired: 2 out]
            }
            n2169 = node-c288(w3464) -> ()  [unwired: 1 out]
          }
        }
      }
      event "Fl. Triggered...": Value Change {
        n2170 = event-data() -> ()  [unwired: 7 out]
        n2171 = case shown="True" "Fl. Triggered..." {
          frame False {
          }
          frame True {
            n2172 = node-c288() -> (w3617:T21)  [unwired: 4 out]
            n2173 = timed-loop {
              timing: w3617 -> [_]
              timing-out: [_] -> w3616
              tunnel: "Action" -> [w3621]
              shift-right: [w3618] -> _
              shift-left: u8 255 -> [w3620]
              stop <- w3622 stop-if-true
              n2174 = node-c288() -> ()  [unwired: 2 out]
              n2175 = flat-sequence {
                tunnel: w3621 -> [w3634]
                tunnel: w3620 -> [w3631]
                tunnel: [w3630] -> w3619
                tunnel: [w3720] -> w3622
                tunnel: w3619 -> [w3719]
                tunnel: [w3719] -> w3618
                frame #0 {
                  n2176 = local read "Delta Fl. 2"() -> (w3625:dbl)
                  n2177 = local read "Delta Fl. 1"() -> (w3626:dbl)
                  n2178 = Select(t=w3626, s="APD to Watch", f=w3625) -> (s? t:f=w3624:dbl)
                  n2179 = Multiply(x="Fl. Delta Thresh. (kHz)", y=1000.0) -> (x*y=w3633:dbl)
                  n2180 = Greater?(x=w3624, y=w3633) -> (0:w3628:bool)
                  n2181 = Or(x="Force Yank", y=w3628) -> (x .or. y?=w3629:bool)
                  n2182 = case shown="True" w3629 {
                    tunnel: w3634 -> [_ w3644]
                    tunnel: w3631 -> [w3636 w3640]
                    tunnel: [w3636 w3637] -> w3630
                    frame False {
                    }
                    frame True {
                      n2183 = flat-sequence {
                        tunnel: w3641 -> [w3650]
                        tunnel: [w3650] -> w3645
                        tunnel: w3644 -> [w3649]
                        tunnel: [w3649] -> w3643
                        tunnel: [w3648] -> w3642
                        tunnel: w3640 -> [w3647]
                        tunnel: [w3646] -> w3639
                        tunnel: w3645 -> [w3675]
                        tunnel: w3643 -> [w3674]
                        tunnel: w3642 -> [w3673]
                        tunnel: w3639 -> [w3672]
                        tunnel: [w3672] -> w3638
                        tunnel: w3638 -> [w3717]
                        tunnel: [w3717] -> w3637
                        frame #0 {
                          n2184 = call <vilib>:"Beep.vi"() -> ()  [unwired: 3 in, 9 out]
                          n2185 = local write "Waiting"(FALSE ("Waiting")) -> ()
                          n2186 = Increment(x=w3647) -> (x+1=w3646:u8)
                          n2187 = case shown="\"Yank\"" w3649 {
                            tunnel: w3646 -> [_ _ w3656]
                            frame "Image" {
                              n2188 = property on="Confocal Image" class="Bool (strict)"("Val(Sgnl)"=TRUE ("Value (Signaling)")) -> ()  [unwired: 2 in, 2 out]
                            }
                            frame "Alarm", Default {
                            }
                            frame "Yank" {
                              n2189 = flat-sequence {
                                tunnel: w3656 -> [w3659]
                                tunnel: [w3658] -> w3655
                                tunnel: ["N Array El"] -> w3654
                                tunnel: w3655 -> [w3669]
                                tunnel: w3654 -> [w3665]
                                frame #0 {
                                n2190 = Multiply(x="Yank Delay (s)", y=1000.0) -> (x*y=w3662:dbl)
                                n2191 = Quotient & Remainder(x=w3659, y="N Array El") -> (x-y*floor(x/y)=w3658:u8)  [unwired: 1 out]
                                n2192 = Wait (ms)(milliseconds to wait=w3662) -> ()  [unwired: 1 out]
                                }
                                frame #1 {
                                n2193 = Random Number (0-1)() -> (number: 0 to 1=w3666:dbl)
                                n2194 = Multiply(x=w3665, y=w3666) -> (x*y=w3664:dbl)
                                n2195 = Round Toward -Infinity(1:w3664) -> (0:w3663:dbl)
                                n2196 = Select(t=w3663, s="Random Choice", f=w3669) -> (s? t:f=w3667:dbl)
                                n2197 = Index Array(array="Yank to Delta Array (MHz)", index=w3667) -> (element=w3670:dbl)
                                n2198 = property on="Trap Delta (MHz)" class="DigNum (strict)"("Val(Sgnl)"=w3670) -> ()  [unwired: 2 in, 2 out]
                                }
                              }
                            }
                          }
                          n2199 = local read "Time (s)"() -> (w3648:dbl)
                          "Fl. High" <- TRUE ("Yanking")
                        }
                        frame #1 {
                          n2200 = node-c288() -> (w3677:T21)  [unwired: 4 out]
                          n2201 = timed-loop {
                            timing: w3677 -> [_]
                            timing-out: [_] -> w3676
                            tunnel: w3675 -> [w3693]
                            tunnel: w3674 -> [w3691]
                            tunnel: w3673 -> [w3690]
                            stop <- w3692 stop-if-true
                            n2202 = node-c288() -> ()  [unwired: 2 out]
                            n2203 = local read "Fl. Delta Thresh. (kHz)"() -> (w3685:dbl)
                            n2204 = local read "Fl. Triggered..."() -> (w3694:bool)
                            n2205 = local read "Delta Fl. 1"() -> (w3681:dbl)
                            n2206 = local read "Delta Fl. 2"() -> (w3679:dbl)
                            n2207 = local read "Stop All"() -> (w3688:bool)
                            n2208 = local read "APD to Watch"() -> (w3680:bool)
                            n2209 = Select(t=w3681, s=w3680, f=w3679) -> (s? t:f=w3678:dbl)
                            n2210 = Not(x=w3694) -> (.not. x?=w3689:bool)
                            n2211 = Multiply(x=w3685, y=1000.0) -> (x*y=w3684:dbl)
                            n2212 = Negate(x=w3684) -> (-x=w3683:dbl)
                            n2213 = Less?(x=w3678, y=w3683) -> (x < y?=w3687:bool)
                            n2214 = Compound Arithmetic op=OR(w3687, w3688, w3689, "Force Reset") -> (w3692:bool)
                            n2215 = case shown="True" w3692 {
                              tunnel: w3693 -> [_ w3705]
                              tunnel: w3691 -> [_ w3704]
                              tunnel: w3690 -> [_ w3702]
                              frame False {
                              }
                              frame True {
                                n2216 = case shown="\"Yank\"" w3704 {
                                tunnel: w3705 -> [_ w3706]
                                frame "Image", Default {
                                }
                                frame "Yank" {
                                n2217 = flat-sequence {
                                tunnel: [w3711] -> w3707
                                tunnel: w3706 -> [w3711]
                                tunnel: w3707 -> [w3712]
                                frame #0 {
                                n2218 = local read "Yank Delay (s)"() -> (w3710:dbl)
                                n2219 = Multiply(x=w3710, y=1000.0) -> (x*y=w3708:dbl)
                                n2220 = Wait (ms)(milliseconds to wait=w3708) -> ()  [unwired: 1 out]
                                }
                                frame #1 {
                                n2221 = property on="Trap Delta (MHz)" class="DigNum (strict)"("Val(Sgnl)"=w3712) -> ()  [unwired: 2 in, 2 out]
                                }
                                }
                                }
                                }
                                n2222 = local read "Time (s)"() -> (w3703:dbl)
                                n2223 = Subtract(x=w3703, y=w3702) -> (x-y=w3699:dbl)
                                "Duration (s)" <- w3699
                                n2224 = Number To Decimal String(number=w3699, width (-)=i16 0) -> (decimal integer string=w3697:string)
                                n2225 = Concatenate Strings(w3697, " s fluorescence event." ("string")) -> (w3695:string)
                                n2226 = local read "Messages"() -> (w3701:string)
                                n2227 = call "Update messages.vi"("Message to add"=w3695, "Old message string"=w3701) -> ("New message string"=w3700:string)
                                n2228 = call <vilib>:"Beep.vi"() -> ()  [unwired: 3 in, 9 out]
                                n2229 = local write "Messages"(w3700) -> ()
                              }
                            }
                            n2230 = node-c288() -> ()  [unwired: 2 out]
                          }
                          n2231 = node-c288(w3676) -> ()  [unwired: 1 out]
                        }
                        frame #2 {
                          n2232 = local write "Fl. High"(FALSE ("Yanking")) -> ()
                        }
                      }
                      n2233 = local read "Trap Delta (MHz)"() -> (w3641:dbl)
                    }
                  }
                }
                frame #1 {
                  n2234 = local read "Stop All"() -> (w3723:bool)
                  n2235 = local read "Fl. Triggered..."() -> (w3721:bool)
                  n2236 = Not(x=w3721) -> (.not. x?=w3722:bool)
                  n2237 = Or(x=w3722, y=w3723) -> (x .or. y?=w3720:bool)
                  n2238 = Not(x=w3720) -> (.not. x?=→"Waiting":bool)
                }
              }
              n2239 = node-c288() -> ()  [unwired: 2 out]
            }
            n2240 = node-c288(w3616) -> ()  [unwired: 1 out]
          }
        }
      }
      event "Trap Triggering": Value Change {
        n2241 = event-data() -> ()  [unwired: 7 out]
        n2242 = case shown="True" "Trap Triggering" {
          frame False {
          }
          frame True {
            n2243 = while {
              stop <- w3730 stop-if-true
              n2244 = flat-sequence {
                tunnel: [w3736] -> w3730
                frame #0 {
                  n2245 = Multiply(x="Wait to get offset (s)", y=u32 1000) -> (x*y=w3732:u32)
                  n2246 = Wait (ms)(milliseconds to wait=w3732) -> ()  [unwired: 1 out]
                }
                frame #1 {
                  n2247 = local read "Mean T1 Position (nm)"() -> (w3738:dbl)
                  "Mean T1 Position (nm) 2" <- w3738
                  n2248 = while {
                    tunnel: w3738 -> [w3765]
                    tunnel: [w3756] -> w3737
                    tunnel: [FALSE ("Waiting")] -> w3734
                    stop <- w3761 stop-if-true
                    n2249 = local read "T1 x pos data"() -> (w3758:dbl[])
                    n2250 = local read "Trap Triggering"() -> (w3759:bool)
                    n2251 = Subtract(x=w3758, y=w3765) -> (x-y=w3763:dbl[])
                    n2252 = Wait (ms)(milliseconds to wait="mean sampling rate (ms)") -> ()  [unwired: 1 out]
                    n2253 = Negate(x=w3763) -> (-x=w3755:dbl[])
                    n2254 = Array Max & Min(array=w3755) -> (max value=→"max value":dbl, min value=→"min value":dbl)  [unwired: 2 out]
                    n2255 = Not(x=w3759) -> (.not. x?=w3760:bool)
                    n2256 = Greater?(x=w3755, y="Threshold (nm)") -> (0:w3757:bool[])
                    n2257 = Or Array Elements(Boolean array=w3757) -> (logical OR=w3756:bool)
                    n2258 = Or(x=w3756, y=w3760) -> (x .or. y?=w3761:bool)
                  }
                  "Waiting" <- w3734
                  n2259 = local write "Waiting"(TRUE ("Waiting")) -> ()
                  n2260 = case shown="True" w3737 {
                    tunnel: [TRUE w3740] -> w3736
                    frame False {
                    }
                    frame True {
                      n2261 = flat-sequence {
                        tunnel: [w3741] -> _
                        tunnel: [w3741] -> w3740
                        frame #0 {
                          n2262 = while {
                            tunnel: [w3743] -> w3741
                            i -> [w3749]
                            stop <- w3746 stop-if-true
                            n2263 = Increment(x=w3749) -> (x+1=w3748:i32)
                            n2264 = Wait (ms)(milliseconds to wait=u32 1000) -> ()  [unwired: 1 out]
                            n2265 = Greater Or Equal?(x=w3748, y="Fl. ON time (s)") -> (x >= y?=w3744:bool)
                            n2266 = local read "Trap Triggering"() -> (w3745:bool)
                            n2267 = Not(x=w3745) -> (.not. x?=w3743:bool)
                            n2268 = Or(x=w3743, y=w3744) -> (x .or. y?=w3746:bool)
                            n2269 = case shown="True" w3744 {
                              frame False {
                              }
                              frame True {
                                n2270 = property on="Green Laser ON/Interlacing" class="Bool (strict)"("Val(Sgnl)"=FALSE ("Value (Signaling)")) -> ()  [unwired: 2 in, 2 out]
                              }
                            }
                          }
                          n2271 = property on="Green Laser ON/Interlacing" class="Bool (strict)"("Val(Sgnl)"=TRUE ("Value (Signaling)")) -> ()  [unwired: 2 in, 2 out]
                          n2272 = call <vilib>:"Beep.vi"() -> ()  [unwired: 12 in]
                        }
                      }
                    }
                  }
                }
              }
            }
          }
        }
      }
      event "Stop All": Value Change {
        n2273 = event-data() -> ()  [unwired: 7 out]
        n2274 = local read "Stop All"() -> (w3766:bool)
      }
    }
    n2275 = node-c288() -> ()  [unwired: 2 out]
  }
  n2276 = flat-sequence "Video" {
    tunnel: [w3775] -> w66
    tunnel: w66 -> [w3816]
    frame #0 {
      n2277 = while {
        stop <- w3768 continue-if-true
        n2278 = call "Close Video Capture.vi"() -> ("error code OUT"=w3770:i32)
        n2279 = Equal?(x=w3770, y=0) -> (x = y?=w3768:bool)
      }
      n2280 = local write "Stop All"(FALSE ("Stop All")) -> ()
    }
    frame #1 {
      n2281 = call "DMR_Init.vi"() -> ()  [unwired: 3 out]
    }
    frame #2 {
      # "Setting the destination format to Mono8 makes sure that the image can be displayed in the intensity plot."
      n2282 = call "DMR_GetDevice.vi"("search string IN"="DE019116701") -> ("device handle OUT"=w3793:i32)  [unwired: 4 in, 2 out]
      n2283 = call "DMR_OpenDevice.vi"("device handle IN"=w3793) -> ("driver handle OUT"=w3776:i32)  [unwired: 4 out]
      n2284 = call "DMR_FindList.vi"("flags IN"=u32 0 ("flags"), "list name IN"="" ("String"), "list type IN"=T45."camera descriptions", "driver handle IN"=w3776) -> ("list handle OUT"=w3779:i32)  [unwired: 2 out]
      n2285 = call "DMR_FindList.vi"("flags IN"=u32 0 ("flags"), "list name IN"="Base", "list type IN"=T45."setting", "driver handle IN"=w3776) -> ("list handle OUT"=w3777:i32)  [unwired: 2 out]
      n2286 = call "OBJ_GetHandle.vi"("object name IN"="VideoStandard", "list handle IN"=w3779) -> ("object handle OUT"=w3773:i32)  [unwired: 3 out]
      n2287 = call "OBJ_GetHandle.vi"("object name IN"="PixelFormat", "list handle IN"=w3777) -> ("object handle OUT"=w3787:i32)  [unwired: 3 out]
      n2288 = call "OBJ_SetS.vi"("value index IN"=0, "value IN"="NTSC M", "object handle IN"=w3773) -> ()  [unwired: 2 out]
      n2289 = call "OBJ_SetS.vi"("value index IN"=0, "value IN"="Mono8" ("value"), "object handle IN"=w3787) -> ()  [unwired: 2 out]
      n2290 = call "OBJ_GetHandle.vi"("object name IN"="VideoChannel", "list handle IN"=w3777) -> ("object handle OUT"=w3783:i32)  [unwired: 3 out]
      n2291 = while {
        tunnel: [w3798] -> w3775
        tunnel: w3776 -> [w3795]
        stop <- w3796 continue-if-true
        n2292 = call "DMR_ImageRequestSingle.vi"("request control IN"=0, "driver handle IN"=w3795) -> ("error code OUT"=w3797:i32, "driver handle OUT"=w3798:i32)  [unwired: 2 out]
        n2293 = Equal To 0?(x=w3797) -> (x = 0?=w3796:bool)
      }
      n2294 = call "OBJ_SetI.vi"("value index IN"=0, "value IN"=3 ("Video channel"), "object handle IN"=w3783) -> ()  [unwired: 2 out]
    }
    frame #3 {
      w3804 = T17 0 items=["Grayscale (U8)", "Grayscale (I16)", "Grayscale (SGL)", "Complex (CSG)", "RGB (U32)", "HSL (U32)", "RGB (U64)"] ("Image Type")
      w3812 = T17 0 items=["Grayscale (U8)", "Grayscale (I16)", "Grayscale (SGL)", "Complex (CSG)", "RGB (U32)", "HSL (U32)", "RGB (U64)"] ("Image Type")
      n2295 = for "Create Greyscale map" {
        N: 256 -> [_]
        tunnel: [w3818] -> w3801 mode=indexing
        workers-P: _ -> [_]
        i -> [w3821]
        n2296 = To Unsigned Byte Integer(number=w3821) -> (unsigned 8bit integer=w3817:u8)
        n2297 = Join Numbers(hi=w3817, lo=w3817) -> ((hi.lo)=w3820:u16)
        n2298 = Join Numbers(hi=w3817, lo=w3817) -> ((hi.lo)=w3819:u16)
        n2299 = Join Numbers(hi=w3820, lo=w3819) -> ((hi.lo)=w3818:u32)
      }
      n2300 = call "IMAQ Create"("Image Name"="Scaled video", "Image Type"=w3804) -> ("New Image"=w3803:T2)  [unwired: 2 in, 2 out]
      n2301 = call "IMAQ Create"("Image Name"="Main video", "Image Type"=w3812) -> ("New Image"=w3813:T2)  [unwired: 2 in, 2 out]
      n2302 = node-c288(0 ("Processor")) -> (w3811:T21)  [unwired: 3 out]
      n2303 = Initialize Array(u32 0 ("Window Number (0...15)"), 480 ("dimension size"), 640 ("dimension size")) -> (w3806:u32[][])
      n2304 = timed-loop {
        tunnel: w3816 -> [w3838]
        tunnel: [w3837] -> w3815
        tunnel: w3813 -> [w3836]
        timing: w3811 -> [_]
        timing-out: [_] -> w3810
        tunnel: w3806 -> [w3825]
        tunnel: w3803 -> [w3823]
        tunnel: w3801 -> [w3822]
        stop <- w3824 stop-if-true
        # "This block performs the \nactual image capture."
        n2305 = node-c288() -> ()  [unwired: 2 out]
        n2306 = local read "Stop All"() -> (w3824:bool)
        n2307 = Reciprocal(x="Video Capture Rate (Hz)") -> (1/x=w3828:dbl)
        n2308 = Multiply(x=w3828, y=1000.0) -> (x*y=w3826:dbl)
        n2309 = call "DMR_ImageRequestWaitFor.vi"("queue number IN"=0, "timeout(ms) IN"=500, "driver handle IN"=w3838) -> ("error code OUT"=w3842:i32, "request number OUT"=w3839:i32, "driver handle OUT"=w3840:i32)
        n2310 = feedback #31(T46 refnum ("Avi Refnum")) -> (w3830:T46)
        n2311 = case shown="True" "New Video File" {
          tunnel: [T46 refnum ("Avi Refnum") w3859] -> w3832
          tunnel: [FALSE TRUE] -> w3833
          tunnel: w3830 -> [_ w3855]
          frame False {
          }
          frame True {
            n2312 = call "Create new save file.vi"("Ext"=".avi" ("string"), "Index In"="Video Index") -> ("Path Out"=w3851:path, "Index Out"=w3852:dbl)  [unwired: 1 in]
            "Path Out" <- w3851
            n2313 = Not Equal?(x=w3855, y=T46 refnum ("Avi Refnum")) -> (x != y?=w3856:bool)
            n2314 = Increment(x=w3852) -> (x+1=w3861:dbl)
            n2315 = case shown="True" w3856 {
              tunnel: w3855 -> [_ w3862]
              frame False {
              }
              frame True {
                n2316 = call "IMAQ AVI Close"("Avi Refnum"=w3862) -> ()  [unwired: 1 in, 10 out]
              }
            }
            n2317 = local write "Video Index"(w3861) -> ()
            n2318 = call "IMAQ AVI Create"("Frames Per Second"=u32 30, "AVI Path"=w3851) -> ("Avi Refnum"=w3859:T46)  [unwired: 5 in, 4 out]
          }
        }
        n2319 = Equal To 0?(x=w3842) -> (x = 0?=w3841:bool)
        n2320 = Select(t=w3832, s=w3833, f=w3830) -> (s? t:f=w3831:T46)
        n2321 = feedback-in #31(w3831) -> ()
        n2322 = case shown="True" w3841 {
          tunnel: w3840 -> [w3863 w3888]
          tunnel: w3839 -> [_ w3887]
          tunnel: [w3863 w3884] -> w3837
          tunnel: w3836 -> [_ w3868]
          tunnel: w3825 -> [_ w3872]
          tunnel: w3831 -> [_ w3870]
          tunnel: w3823 -> [_ w3865]
          tunnel: w3822 -> [_ w3864]
          frame False {
          }
          frame True {
            w3878 = u32 0 ("X-offset IN")
            n2323 = call "DMR_GetImageRequestBufferData.vi"("driver handle IN"=w3888, "request number IN"=w3887) -> ("width OUT"=w3877:i32, "height OUT"=w3876:i32, "driver handle OUT"=w3883:i32, "request number OUT"=w3882:i32, "bytes per pixel OUT"=w3879:i32)  [unwired: 13 out]
            n2324 = call "DMR_GetImageRequestBufferImageData.vi"("driver handle IN"=w3883, "request number IN"=w3882, "bytes per pixel IN"=w3879, "X-offset IN"=w3878, "Y-offset IN"=w3878, "height IN"=w3876, "width IN"=w3877) -> ("driver handle OUT"=w3881:u32, "request number OUT"=w3880:u32, "image OUT"=w3873:u32[][])  [unwired: 10 out]
            n2325 = call "DMR_ImageRequestUnlock.vi"("request number IN"=w3880, "driver handle IN"=w3881) -> ("driver handle OUT"=w3886:i32)  [unwired: 1 in, 2 out]
            n2326 = case shown="True" "Averaging" {
              tunnel: w3873 -> [w3924 w3929]
              tunnel: [w3924 w3928] -> w3869
              tunnel: w3872 -> [_ w3926]
              frame False {
              }
              frame True {
                (unwired) 1
                w3934 = 1
                n2327 = feedback #32(w3926) -> (w3925:u32[][])
                n2328 = Add(x=w3929, y=w3925) -> (x+y=w3930:u32[][])
                n2329 = Select(t=w3926, s="Reset Averaging", f=w3930) -> (s? t:f=w3932:u32[][])
                n2330 = feedback-in #32(w3932) -> ()
                n2331 = feedback #33(w3934) -> (w3927:i32)
                n2332 = Divide(x=w3930, y=w3927) -> (x/y=w3931:dbl[][])
                n2333 = Increment(x=w3927) -> (x+1=w3935:i32)
                n2334 = To Unsigned Long Integer(number=w3931) -> (unsigned 32bit integer=w3928:u32[][])
                n2335 = Select(t=w3934, s="Reset Averaging", f=w3935) -> (s? t:f=w3933:i32)
                n2336 = feedback-in #33(w3933) -> ()
              }
            }
            n2337 = call "DMR_ImageRequestSingle.vi"("request control IN"=0, "driver handle IN"=w3886) -> ("driver handle OUT"=w3884:i32)  [unwired: 3 out]
            n2338 = disable-structure shown="Disabled" {
              disable-tunnel: w3869 -> [w3901 _]
              disable-tunnel: w3865 -> [w3900 _]
              frame Disabled {
                n2339 = To Double Precision Float(number=w3901) -> (double precision float=w3899:dbl[][])
                n2340 = In Range and Coerce(upper limit="Intensity Upper", x=w3899, lower limit="Intensity Lower") -> (coerced(x)=w3898:dbl[][])  [unwired: 1 out]
                n2341 = Subtract(x="Intensity Upper", y="Intensity Lower") -> (x-y=w3895:dbl)
                n2342 = Subtract(x=w3898, y="Intensity Lower") -> (x-y=w3896:dbl[][])
                n2343 = Divide(x=w3896, y=w3895) -> (x/y=w3897:dbl[][])
                n2344 = Multiply(x=255.0, y=w3897) -> (x*y=w3893:dbl[][])
                n2345 = To Unsigned Byte Integer(number=w3893) -> (unsigned 8bit integer=w3902:u8[][])
                n2346 = call "IMAQ ArrayToImage"("Image Pixels (U8)"=w3902, "Image"=w3900) -> ("Image Out"=w3889:T2)  [unwired: 4 in, 5 out]
                n2347 = First Call?() -> (First Call?: T/F=w3890:bool)
                n2348 = case shown="True" w3890 {
                  tunnel: w3889 -> [w3903 w3914]
                  frame False {
                    n2349 = flat-sequence {
                      tunnel: w3903 -> [w3909]
                      frame #0 {
                        w3906 = FALSE ("Get/Set Status? (Set)")
                        w3905 = 0 ("Window Number (0...15)")
                        n2350 = call "IMAQ WindSize"("Get/Set Status? (Set)"=w3906, "Window Number"=w3905) -> ("Width & Height out"=→"Window Size":cluster{"Width":i32, "Height":i32})  [unwired: 4 in, 2 out]
                        n2351 = call "IMAQ WindMove"("Window Number (0...15)"=w3905, "Get/Set Status? (Set)"=w3906) -> ("Coordinates (screen)"=→"Window Position":cluster{"X Position":i32, "Y Position":i32})  [unwired: 3 in, 1 out]
                        n2352 = call "IMAQ WindDraw"("Resize to Image Size? (Y)"=FALSE, "Window Number (0...15)"=w3905, "Image"=w3909) -> ()  [unwired: 7 in, 2 out]
                      }
                      frame #1 {
                        n2353 = call "IMAQ WindZoom 2"("Center Point"="Center Point", "Zoom to Fit? (False)"=FALSE, "Zoom Factor"="Zoom Factor") -> ()  [unwired: 5 in, 4 out]
                      }
                    }
                  }
                  frame True {
                    n2354 = flat-sequence {
                      tunnel: w3914 -> [w3917]
                      tunnel: [w3915] -> w3913
                      tunnel: w3913 -> [w3919]
                      frame #0 {
                        w3916 = TRUE ("Resize to Image Size? (Y)")
                        w3915 = 0 ("Window Number (0...15)")
                        n2355 = call "IMAQ WindNonTearing"("Window Number"=w3915, "NonTearing? (True)"=w3916) -> ()  [unwired: 8 in, 2 out]
                        n2356 = call "IMAQ WindDraw"("Resize to Image Size? (Y)"=w3916, "Window Number (0...15)"=w3915, "Image"=w3917) -> ()  [unwired: 7 in, 2 out]
                      }
                      frame #1 {
                        n2357 = call "IMAQ WindSize"("Scrollbars? (N)"=FALSE, "Width & Height"="Initial Window Size", "Window Number"=w3919) -> ()  [unwired: 3 in, 3 out]
                        n2358 = call "IMAQ WindMove"("Window Number (0...15)"=w3919, "Coordinates (screen)"="Initial Window Position") -> ()  [unwired: 3 in, 2 out]
                      }
                    }
                  }
                }
              }
              frame Enabled {
              }
            }
            n2359 = To Unsigned Byte Integer(number=w3869) -> (unsigned 8bit integer=w3867:u8[][])
            n2360 = call "IMAQ ArrayToImage"("Image Pixels (U8)"=w3867, "Image"=w3868) -> ("Image Out"=w3866:T2)  [unwired: 4 in, 5 out]
            "Primary Video Display" <- w3866
            n2361 = case shown="True" "Save Video" {
              tunnel: w3870 -> [_ w3923]
              tunnel: w3866 -> [_ w3922]
              frame False {
              }
              frame True {
                n2362 = call "IMAQ AVI Write Frame"("Image"=w3922, "Avi Refnum"=w3923) -> ()  [unwired: 2 in, 8 out]
              }
            }
            n2363 = case shown="True" "Save Image" {
              tunnel: w3867 -> [_ w3938]
              tunnel: w3864 -> [_ w3937]
              frame False {
              }
              frame True {
                n2364 = call <vilib>:"Flatten Pixmap.vi"("colors"=w3937, "8-bit pixmap"=w3938) -> ("image data"=w3944:T47)  [unwired: 4 in, 5 out]
                n2365 = call "Create new save file.vi"("Insert"="video_frame_" ("string"), "Ext"=".bmp" ("string"), "Index In"="Image Index") -> ("Path Out"=w3940:path, "Index Out"=w3945:dbl)
                n2366 = Increment(x=w3945) -> (x+1=w3939:dbl)
                n2367 = local write "Image Index"(w3939) -> ()
                n2368 = call <vilib>:"Write BMP File.vi"("image data"=w3944, "path to BMP file"=w3940) -> ()  [unwired: 1 in, 9 out]
              }
            }
          }
        }
        n2369 = node-c288(w3826) -> ()  [unwired: 1 out]
      }
      n2370 = node-c288(w3810) -> ()  [unwired: 1 out]
      n2371 = call "DMR_CloseDevice.vi"("driver handle IN"=w3815) -> ()  [unwired: 1 in, 4 out]
    }
    frame #4 {
      n2372 = call "DMR_Close.vi"() -> ()  [unwired: 1 out]
    }
  }
  n2373 = node-c288(w77) -> ()  [unwired: 1 out]
  n2374 = node-c288(w64) -> ()  [unwired: 1 out]
  n2375 = VISA Close(VISA resource name=w68, error in (no error)=w67) -> (error out=w116:errorcluster)
  n2376 = node-c288(w79) -> ()  [unwired: 1 out]
  n2377 = call <vilib>:"Simple Error Handler.vi"("error in (no error)"=w116) -> ()  [unwired: 1 in, 8 out]
  n2378 = node-c288(w75) -> ()  [unwired: 1 out]
  n2379 = node-c288(w160) -> ()  [unwired: 1 out]
  n2380 = flat-sequence {
    tunnel: w255 -> [w3953]
    tunnel: w257 -> [w3954]
    tunnel: [w3952] -> w236
    tunnel: [w3951] -> w235
    tunnel: w217 -> [_]
    tunnel: w215 -> [_]
    tunnel: w168 -> [_]
    tunnel: w81 -> [_]
    tunnel: w236 -> [w3955]
    tunnel: w235 -> [w3956]
    frame #0 {
      w3950 = FALSE ("AI to FIFO")
      n2381 = xnode "Read/Write Control"("FPGA VI Reference In"=w3954, "error in"=w3953, "AI to FIFO"=w3950, "APD to FIFO"=w3950) -> ("FPGA VI Reference Out"=w3952:T19, "error out"=w3951:errorcluster)
    }
    frame #1 {
      n2382 = xnode "Close FPGA VI Reference"("FPGA VI Reference In"=w3955, "error in"=w3956) -> ("error out"=→"error out":errorcluster)
    }
  }
